vi "TLB main task ver 1.00 (incomplete).vi"() -> ()   [LabVIEW 2018]
uses:
  TLB Type Definitions/Intruction Type Definitions.ctl
  TLB Type Definitions/State Type Definitions, for 0.26g versions and later 3.ctl
  <vilib>/Studica/Studica Toolkit/NavX/TypeDefs/Flags/Z900_navX_Flags_OpStatusTypeDef.ctl
  <vilib>/Studica/Studica Toolkit/NavX/TypeDefs/Flags/Z900_navX_Flags_CalibrationStatusTypeDef.ctl
  TLB Type Definitions/Vision cluster.ctl
  TLB Type Definitions/PING CLUSTER.ctl
  TLB Type Definitions/Encoder cluster.ctl
  TLB Type Definitions/Stepper cluster.ctl
  TLB Type Definitions/Yaw Cluster.ctl
  TLB Type Definitions/IR Sensor Type Def.ctl
  TLB Type Definitions/Line Sensor Cluster.ctl
  TLB Type Definitions/Time cluster.ctl
  TLB Type Definitions/Box Colour Detection Cluster (0.26d and above).ctl
  Underlying VI's/FGV's/Box FGV/Box Colour FGV Colours.ctl
  <vilib>/Studica/Studica Toolkit/Background/DIO Channel.ctl
  TLB Type Definitions/Y Stepper cluster.ctl
  TLB Type Definitions/Motor Speed Cluster.ctl
  Labview Training Phase 2/Enum Controls/States for Action Engine.ctl
  Underlying VI's/NavX VI/navX type def.ctl
  <vilib>/Studica/Studica Toolkit/Background/I2C Channel.ctl
  Underlying VI's/I2C Master VI/Arduino_Interfacing.ctl
  Underlying VI's/Motor Control VI with PID/MOTOR CONTROL WITH PID AE DATA MODE TYPE DEF.ctl
  Underlying VI's/Motor Control VI with PID/MOTOR CONTROL WITH PID AE DIRECTION TYPE DEF.ctl
  Experimental VI's/Archived VI's/MOTOR CONTROL NO PID Type Def.ctl
  <vilib>/myRIO/Common/Instrument Driver Framework/myRIO v1.0/AI/typedefs/AI Channels List.ctl
  <vilib>/myRIO/Common/Instrument Driver Framework/myRIO v1.0/AI/typedefs/AI Channels Enum.ctl
  Underlying VI's/Line Sensor AE/Line Sensor AE Type Def.ctl
  Underlying VI's/I2C Master VI/I2C MASTER Type Def.ctl
  Underlying VI's/Elasped Timer/Elapsed timer control.ctl
  Underlying VI's/IMAQ Create Reference AE/IMAQ Reference AE.ctl
  Underlying VI's/FGV's/Box FGV/Box Colour FGV States.ctl
  Underlying VI's/I2C Master VI/I2C_MASTER_WRITE_NEW Type Def.ctl
  Underlying VI's/Modified webcam FGV/Webcam AE.ctl
  <vilib>/userdefined/High Color/IMAQdx.ctl
  <vilib>/Studica/Studica Toolkit/NavX/NavX.lvlib
  <vilib>/NI_Real-Time Target Support.lvlib
panel:
  out "Distance to move":dbl
  out "Same colour?":bool
  out "Box Colour Detection":T1
  out "Errors detected":bool
  out "Robot ready":bool
  out "Time cluster":T3
  out "Table IR obstruct":bool
  out "Front IR obstruct":bool
  out "CPU 1 Usage":dbl
  out "CPU 0 Usage":dbl
  out "Line sensors":T4
  out "IR Sensors":T5
  out "NAVX Values":T6
  out "Stepper position values":T7
  out "Encoder values":T8
  out "Ultrasonic sensors":T9
  out "Selected Task":T10=enum."Start Task 9"
  out "Object recognition mode":enum16{"Ball", "Soap", "Gel", "Pipe", "None"}(ring)
  out "Image Processing Error":errorcluster
  out "Object Detection":T11
  out "Status":T14 {"OP Status" items=["INITIALIZING", "SELFTEST_IN_PROGRESS", "ERROR", "IMU_AUTOCAL_IN_PROGRESS", "NORMAL"]; "Calibration Status" items=["IMU_CAL_STATE_MASK"=3, "IMU_CAL_STATE_INPROGRESS"=0, "IMU_CAL_STATE_ACCUMULATE"=1, "IMU_CAL_STATE_COMPLETE"=2]}
  out "General Errors":errorcluster
  in  "Red LED":bool
  out "Front Ultrasonic obstruct":bool
  out "Speed & distance":T15
  out "Task selection":u8
  out "NavX Readings":T16
  out "Arduino Data":T17
  out "TASK ENABLE":bool
  out "Rising Edge":bool
  in  "Green LED":bool
  out "State Logic":T18=enum."Startup"
  out "elements":T10[](array[typedef])
  in  "STOP TASK":bool
  in  "OK Button":bool
  in  "STOP":bool
  out "Queue Errors":errorcluster
  out "Action Queue Items":i32
  out "State Logic Queue Items":i32
  out "Action Queues items":string[](array[string])=["Hardware reset", "Software reset", ""]
  out "Action State":string
  # "VISION"
  # "TLB FRAMEWORK STATUS"
  # "System Health Status Update"
  # "Test Programme written by Calvin Loke    Dated: 28 Aug 2019\nTest Programme revised by Dr Alex See   Dated 30 Aug 2019\n\nRevision date: 20/03/2020\nProgramme version:   TLB Native Dynamic Events ver 0.19a"
  # "0: Task 1\n1: Task 2\n2: Task 3\n3: Task 4\n4: Task 5\n5: Task 6\n6: Task 7\n7: Task 8 Ball\n8: Task 8 Soap\n9: Task 8 Gel\n10: Task 8 Pipe\n11: Task 9 Blue\n12: Task 9 Black\n13: Task 9 Green\n14: Task 9 Red\n15: Task 9 Yellow"
  # "Ball: Right\nSoap: Left\nGel: Reverse\nPipe: Forward"
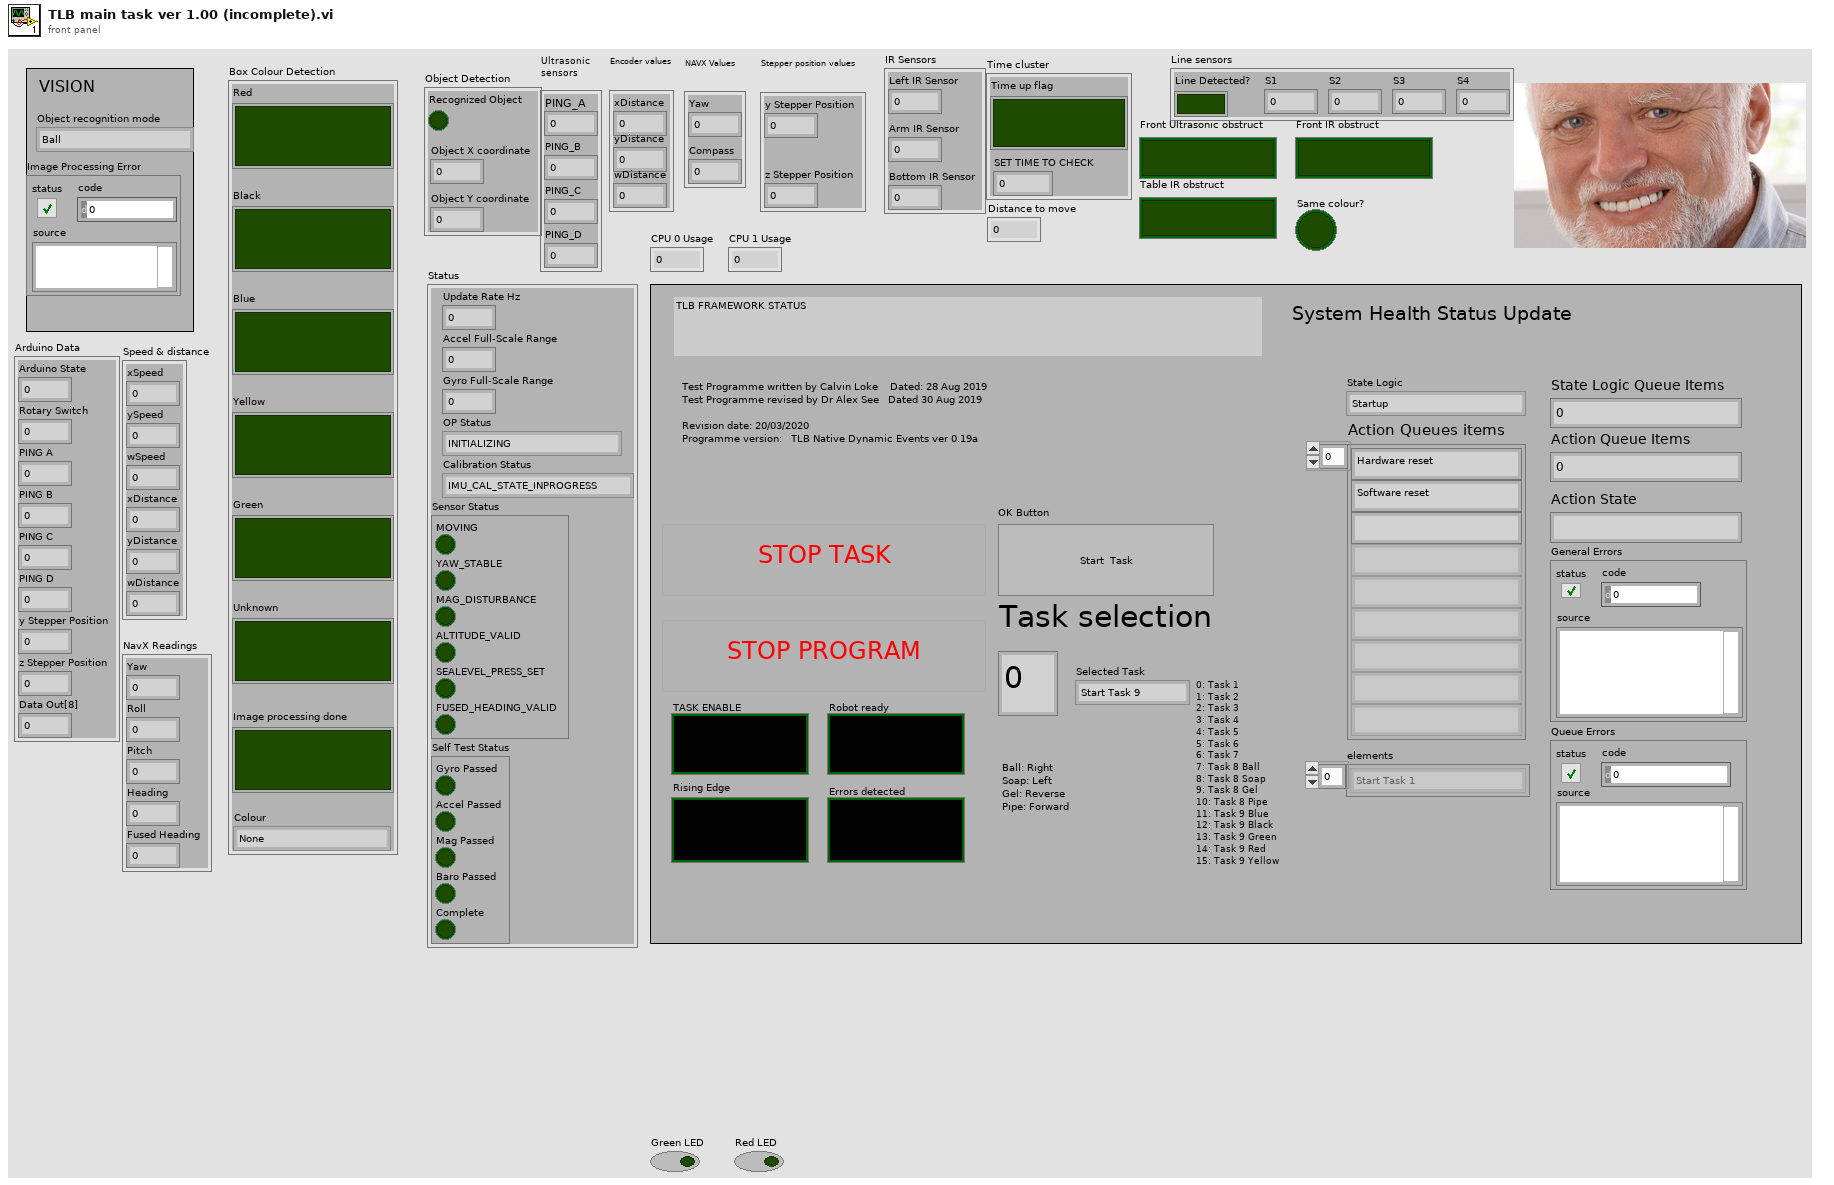
[diagram p1: front panel]
types:
  T1 = typedef "Box Colour Detection Cluster (0.26d and above).ctl" = cluster{"Red":bool, "Black":bool, "Blue":bool, "Yellow":bool, "Green":bool, "Unknown":bool, "Image processing done":bool, "Colour":T2}
  T2 = typedef "Box Colour FGV Colours.ctl" = enum16{"None", "Black", "Blue", "Green", "Red", "Yellow"}
  T3 = typedef "Time cluster.ctl" = cluster{"Time up flag":bool, "SET TIME TO CHECK":dbl}
  T4 = typedef "Line Sensor Cluster.ctl" = cluster{"Line Detected?":bool, "S1":dbl, "S2":dbl, "S3":dbl, "S4":dbl}
  T5 = typedef "IR Sensor Type Def.ctl" = cluster{"Left IR Sensor":dbl, "Arm IR Sensor":dbl, "Bottom IR Sensor":dbl}
  T6 = typedef "Yaw Cluster.ctl" = cluster{"Yaw":dbl, "Compass":dbl}
  T7 = typedef "Stepper cluster.ctl" = cluster{"y Stepper Position":u8, "z Stepper Position":u8}
  T8 = typedef "Encoder cluster.ctl" = cluster{"xDistance":dbl, "yDistance":dbl, "wDistance":dbl}
  T9 = typedef "PING CLUSTER.ctl" = cluster{"PING_A":u8, "PING_B":u8, "PING_C":u8, "PING_D":u8}
  T10 = typedef "Intruction Type Definitions.ctl" = enum16{"None", "Start Task 1", "Start Task 2", "Start Task 3", "Start Task 4", "Start Task 5", "Start Task 6", "Start Task 7", "Start Task 8 - BALL", "Start Task 8 - Gel", "Start Task 8 - Pipe", "Start Task 8 - Soap", "Start Task 9", "Start Task A", "Start Task B", "Exit"}
  T11 = typedef "Vision cluster.ctl" = cluster{"Recognized Object":bool, "Object X coordinate":dbl, "Object Y coordinate":dbl}
  T12 = typedef "NavX.lvlib/Z900_navX_Flags_OpStatusTypeDef.ctl" = u8
  T13 = typedef "NavX.lvlib/Z900_navX_Flags_CalibrationStatusTypeDef.ctl" = u8
  T14 = cluster{"Update Rate Hz":u8, "Accel Full-Scale Range":u8, "Gyro Full-Scale Range":u16, "OP Status":T12, "Calibration Status":T13, "Sensor Status":cluster{"MOVING":bool, "YAW_STABLE":bool, "MAG_DISTURBANCE":bool, "ALTITUDE_VALID":bool, "SEALEVEL_PRESS_SET":bool, "FUSED_HEADING_VALID":bool}, "Self Test Status":cluster{"Gyro Passed":bool, "Accel Passed":bool, "Mag Passed":bool, "Baro Passed":bool, "Complete":bool}}
  T15 = cluster{"xSpeed":dbl, "ySpeed":dbl, "wSpeed":dbl, "xDistance":dbl, "yDistance":dbl, "wDistance":dbl}
  T16 = cluster{"Yaw":dbl, "Roll":dbl, "Pitch":dbl, "Heading":dbl, "Fused Heading":dbl}
  T17 = cluster{"Arduino State":u8, "Rotary Switch":u8, "PING A":u8, "PING B":u8, "PING C":u8, "PING D":u8, "y Stepper Position":u8, "z Stepper Position":u8, "Data Out[8]":u8}
  T18 = typedef "State Type Definitions, for 0.26g versions and later 3.ctl" = enum16{"None", "Startup", "Move to Angle", "True Stop", "Idle", "Shutdown", "Task 1A", "Task 1B", "Task 2:Raise Arm", "Task 2:Sensor Mode", "Task 2:Reverse Mode", "Task 3", "Task 4_A", "Task 4_B", "Task 4_C", "Task 4_D", "Task 5A: RAISING ARM", "Task 5B: STILL WAITING", "Task 5C: GOING DOWN", "Task 5D: GRAB", "Task 5E: GOING UP", "Task 5F: ARM GRAB HEIGHT", "Task 5G: CLOSE CLAW", "Task 5H: RAISE ARM", "Task 6A: RAISE ARM", "Task 6B: CAM BURST", "Task 6C: PROCESS IMAGE", "Task 6D: BALL BUSTER", "Task 6E: STILL WAITING", "Task 6F: CAM BURST 2", "Task 6G: PROCESS IMAGE 2", "Task 6H: SKADI SOAPS", "Task 6I: STILL WAITING 2", "Task 6J: CAM BURST 3", "Task 6K: PROCESS IMAGE 3", "Task 6L: JAM IT IN", "Task 6M: STILL WAITING 3", "Task 6N: CAM BURST 4", "Task 6O: PROCESS IMAGE 4", "Task 6P: PIPE BOMB", "Task 7", "Task 8A: RAISE ARM", "Task 8B: MOVE TO BOX", "Task 8C: CAM BURST", "Task 8D: PROCESS IMAGE", "Task 8E: ROBOT ADJUST", "Task 8F: CAM BURST 2", "Task 8G: PROCESS IMAGE 2", "Task 8H: ARM ADJUST", "Task 8I: ARM GRAB HEIGHT", "Task 8J: CLOSE CLAW", "Task 8K: RAISE MY SWORD", "Task 9A: Raise Arm", "Task 9B: Rotate to Angle", "Task 9C: Detect Box", "Task 9D: MOVE FORWARD", "Task 9E: MOVE LEFT", "Task 9E2: MOVE RIGHT", "Task 9F: SCAN BOX", "Task 9G: MOVE RIGHT", "Task 9H: SCAN BOX 2", "Task 9I: ROTATE 90 CW", "Task 9J: FORWARD", "Task 9K: RAM WALL", "Task 9L: MOVE RIGHT", "Task 9M: SCAN BOX 3", "Task 9N: MOVE RIGHT", "Task 9O: SCAN BOX 4", "Task A1: RAISE ARM", "Task A2: ROTATE TO ANGLE", "Task A3: MOVE TO BL BOX", "Task A4: MOVE FORWARD", "Task A5: ROTATE CW 90"}
  T19 = typedef "Motor Speed Cluster.ctl" = cluster{"ySpeed":dbl, "xSpeed":dbl, "wSpeed":dbl}
  T20 = typedef "Y Stepper cluster.ctl" = cluster{"yStepper desired":u8}
  T21 = typedef "DIO Channel.ctl" = enum16{"Not Connected", "A/DIO1", "A/DIO2", "A/DIO3", "A/DIO4", "A/DIO5", "A/DIO6", "A/DIO7", "A/DIO13", "B/DIO1", "B/DIO2", "B/DIO3", "B/DIO4", "B/DIO5", "B/DIO6", "B/DIO7", "B/DIO13", "C/DIO0", "C/DIO1", "C/DIO2", "C/DIO3", "C/DIO4", "C/DIO5", "C/DIO6", "C/DIO7"}
  T22 = cluster{"DIO Channel":T21, "FPGA VI Reference Out":refnum<k20>}
  T23 = typedef "States for Action Engine.ctl" = enum16{"Initialize", "Write", "Read"}
  T24 = typedef "NI_Real-Time Target Support.lvlib/RT CPU Load.ctl" = cluster{"Total (%)":dbl, "Time Critical (%)":dbl, "Timed Structures (%)":dbl, "High (%)":dbl, "Above Normal (%)":dbl, "Normal (%)":dbl, "Background (%)":dbl, "Idle (%)":dbl, "ISR (%)":dbl}
  T25 = cluster{"CPU loads[0]":T24, "CPU loads[1]":T24, "CPU loads[2]":T24, "CPU loads[3]":T24, "CPU loads[4]":T24, "CPU loads[5]":T24, "CPU loads[6]":T24, "CPU loads[7]":T24, "CPU loads[8]":T24}
  T26 = typedef "navX type def.ctl" = enum16{"Get i2C reference", "Read Values", "Zero Yaw"}
  T27 = typedef "Arduino_Interfacing.ctl" = enum16{"Initialize", "Write to Arduino", "Read From Arduino"}
  T28 = typedef "I2C Channel.ctl" = enum16{"Not Connected", "A", "B"}
  T29 = cluster{"I2C Ref Out":cluster{"I2C Channel":T28, "FPGA VI Reference Out":refnum<k20>}, "Connected":bool, "Slave Address (7-bit)":u8, "Registry":u8[]}
  T30 = typedef "Box Colour FGV States.ctl" = enum16{"Initialize", "Read", "Write"}
  T31 = typedef "MOTOR CONTROL WITH PID AE DIRECTION TYPE DEF.ctl" = enum16{"y-axis movement", "x-axis movement", "rotation", "stop", "reset encoders"}
  T32 = typedef "MOTOR CONTROL WITH PID AE DATA MODE TYPE DEF.ctl" = enum16{"Init AE", "Write to AE", "Read from AE"}
  T33 = typedef "Line Sensor AE Type Def.ctl" = enum16{"INIT AE", "READ FROM LINE SENSORS"}
  T34 = typedef "IMAQ Reference AE.ctl" = enum16{"Initialize AE", "Get IMAQ Reference", "Dispose Processing Buffer"}
  T35 = typedef "Elapsed timer control.ctl" = enum16{"Start", "Pause", "Initialize"}
  T36 = typedef "I2C_MASTER_WRITE_NEW Type Def.ctl" = enum16{"Ultrasonic sensors", "Stepper origin", "zStepper 13.3k", "zStepper 13k", "zStepper 12k", "zStepper 11k", "zStepper 10k", "zStepper 9k", "zStepper 8k", "zStepper 7k", "zStepper 6k", "zStepper 5k", "zStepper 4k", "zStepper 3k", "zStepper 2k", "zStepper 1k", "zStepper 900", "zStepper 800", "zStepper 700", "zStepper 600", "zStepper 500", "zStepper 400", "zStepper 300", "zStepper 200", "zStepper 100", "zStepper 0", "yStepper control", "Open Claw", "Close Claw", "Soft Reset"}
  T37 = typedef "Webcam AE.ctl" = enum16{"Initialize Camera", "Open Camera", "Continuous Acquisition", "Close Camera", "Retrieve Image", "Dispose Camera Image Buffer"}
  T38 = typedef "IMAQdx.ctl" = refnum<k21>
  T39 = typedef "MOTOR CONTROL NO PID Type Def.ctl" = enum16{"Init", "Front Back", "Left Right", "Rotate", "Stop", "Latch"}
  T40 = typedef "AI Channels List.ctl" = T41[]
  T41 = typedef "AI Channels Enum.ctl" = enum16{"Not Connected", "AudioIn/Left", "AudioIn/Right", "C/AI0", "C/AI1", "A/AI0", "A/AI1", "A/AI2", "A/AI3", "A/AI4", "A/AI5", "A/AI6", "A/AI7", "B/AI0", "B/AI1", "B/AI2", "B/AI3", "B/AI4", "B/AI5", "B/AI6", "B/AI7", "AI/AI0", "AI/AI1", "AI/AI2", "AI/AI3", "A/AI0 (DIFF)", "A/AI1 (DIFF)", "A/AI2 (DIFF)", "A/AI3 (DIFF)", "B/AI0 (DIFF)", "B/AI1 (DIFF)", "B/AI2 (DIFF)", "B/AI3 (DIFF)"}
  T42 = cluster{"S1":dbl, "S2":dbl, "S3":dbl, "S4":dbl, "Array[4]":dbl, "Array[5]":dbl, "Array[6]":dbl, "Array[7]":dbl, "Array[8]":dbl}
  T43 = typedef "I2C MASTER Type Def.ctl" = enum16{"Last State", "Mode 0", "Mode 1", "Mode 2", "Mode 3", "Mode 4", "Mode 5", "Mode 6", "Mode 7", "Mode 8", "Mode 9", "Mode 10"}
  T44 = typedef "IMAQ Image.ctl" = refnum<image>
  T45 = cluster{"Number of Matches":i32, "Object detected?":bool}
  T46 = cluster{"Red":bool, "Black":bool, "Blue":bool, "Yellow":bool, "Green":bool, "No recognizable coolour":bool}
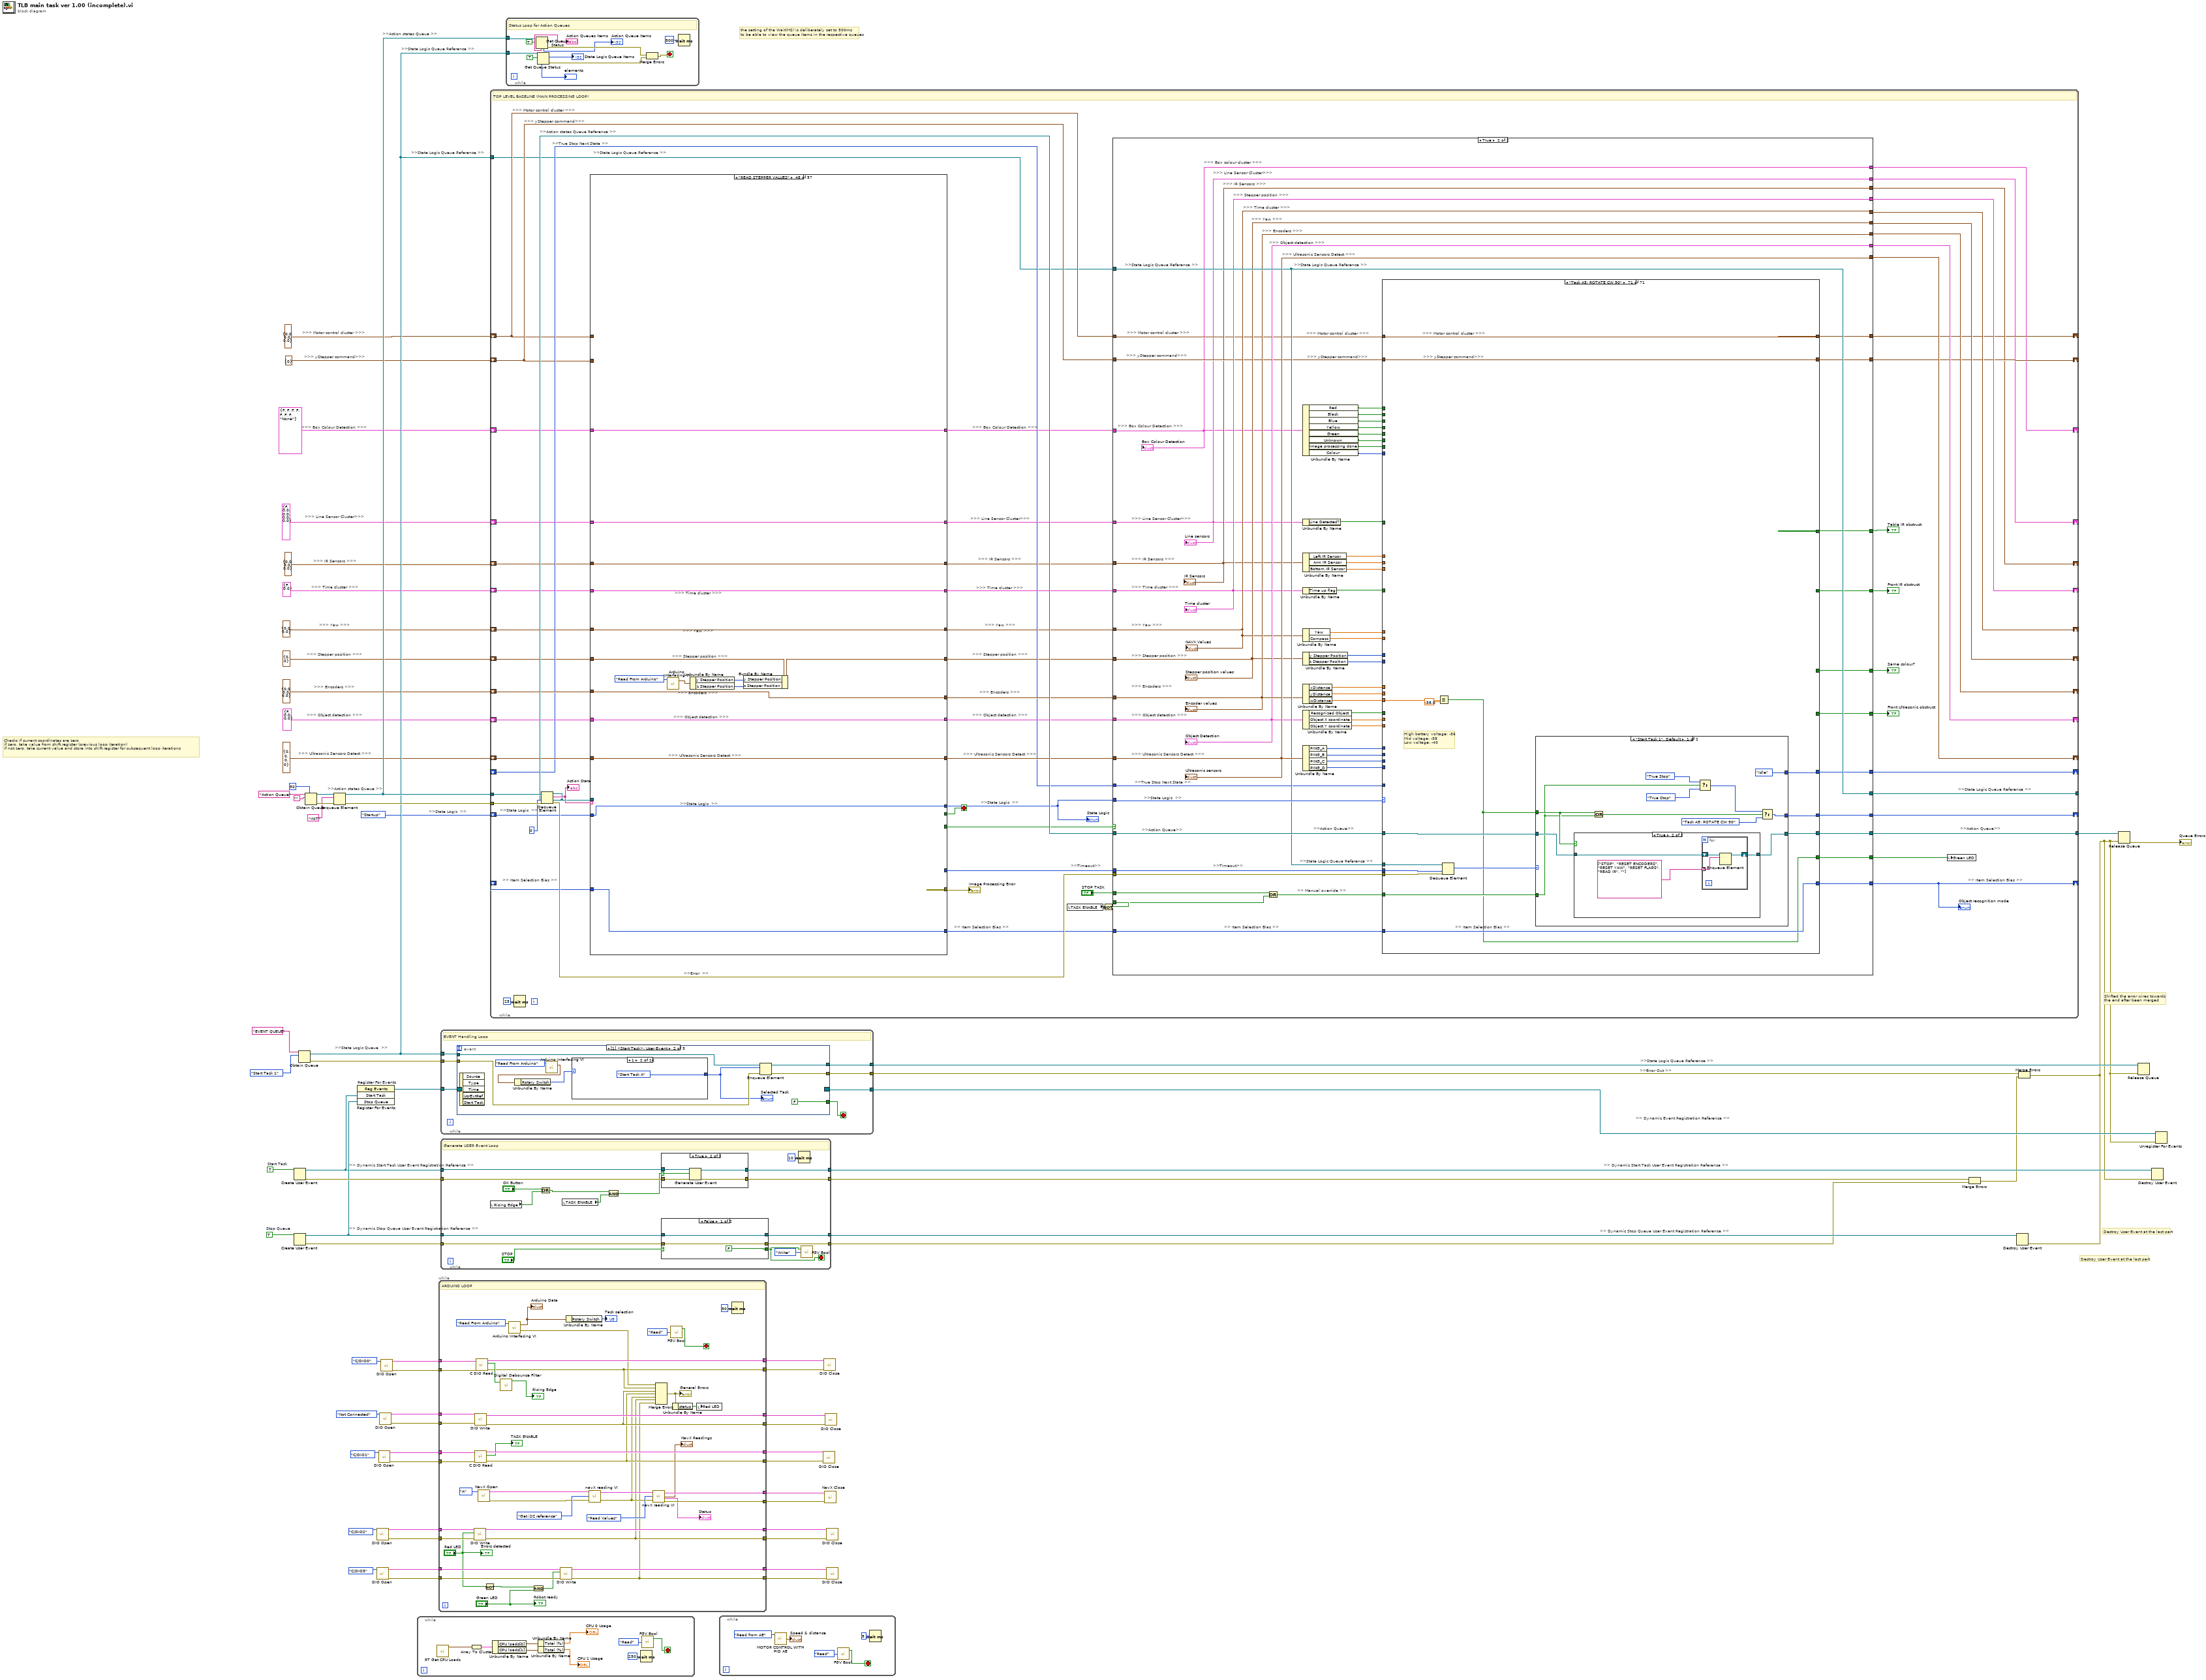
[diagram p0: block diagram]
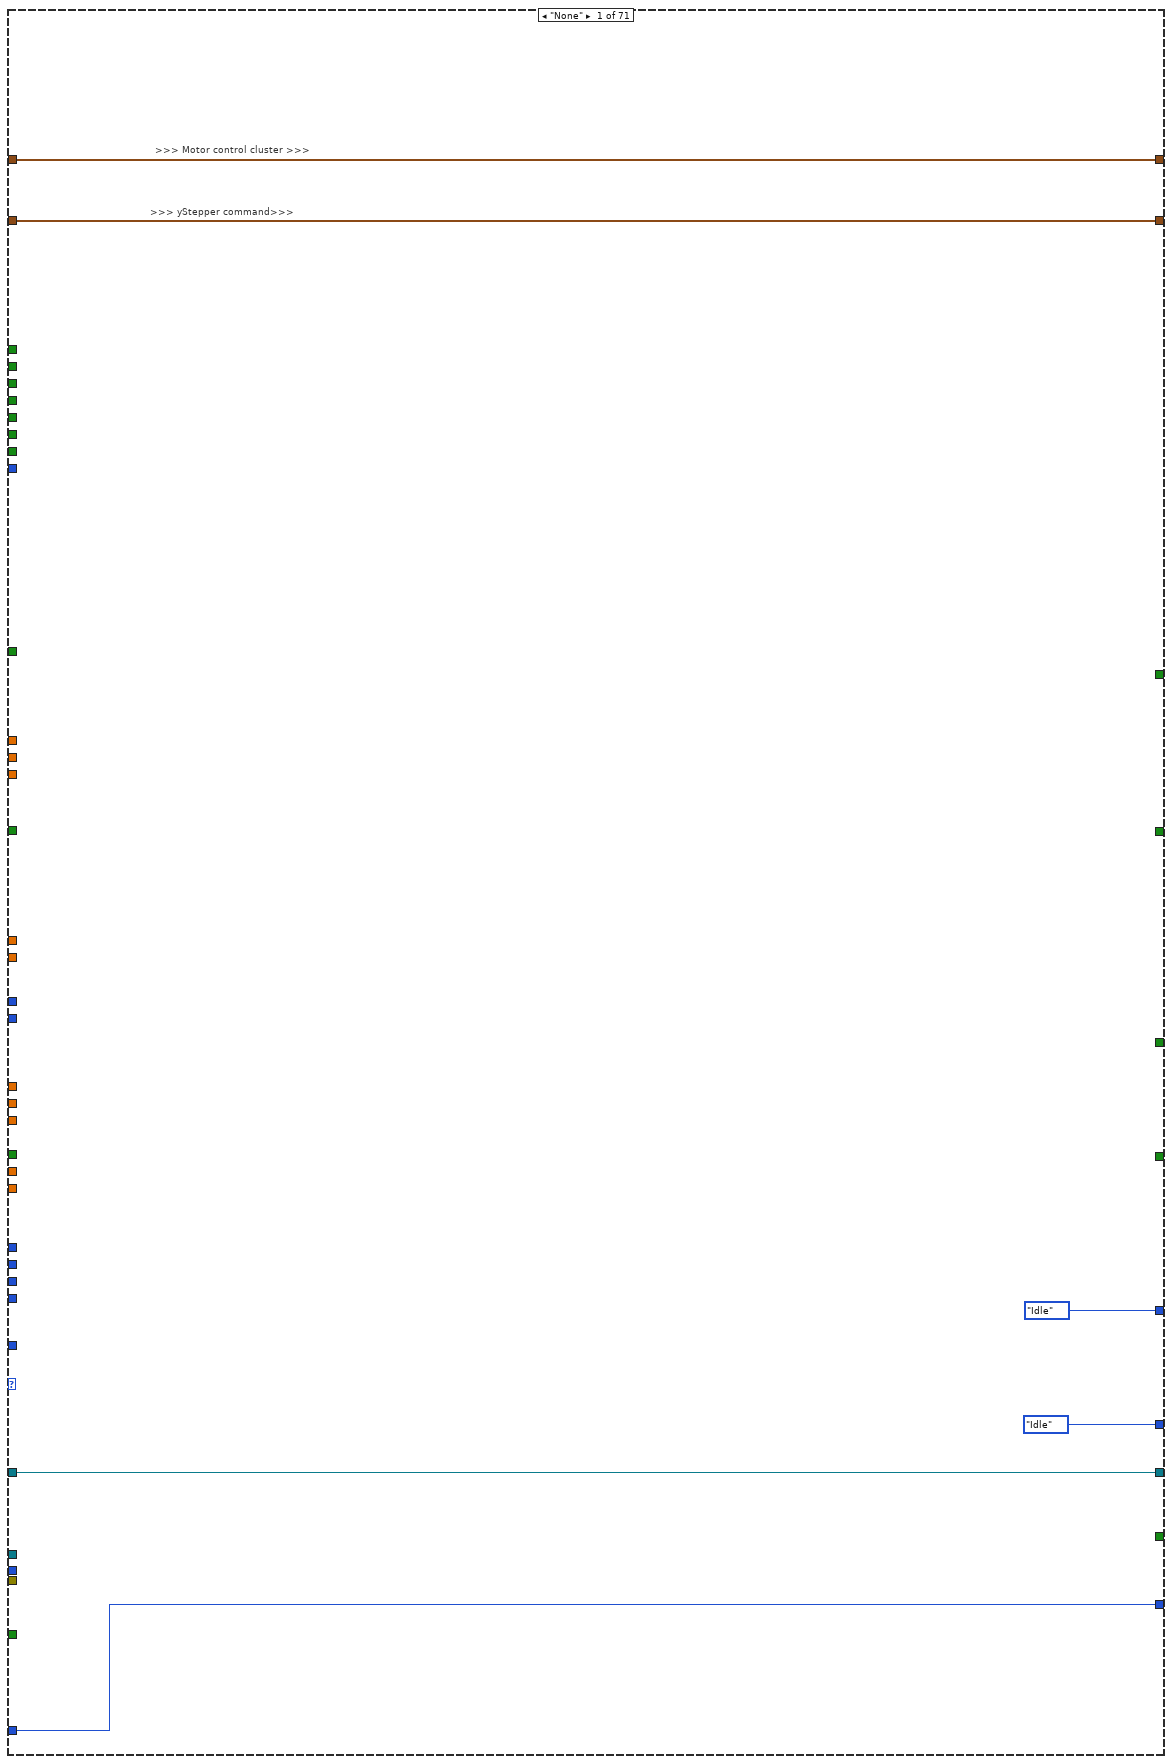
[diagram p3: hidden frame]
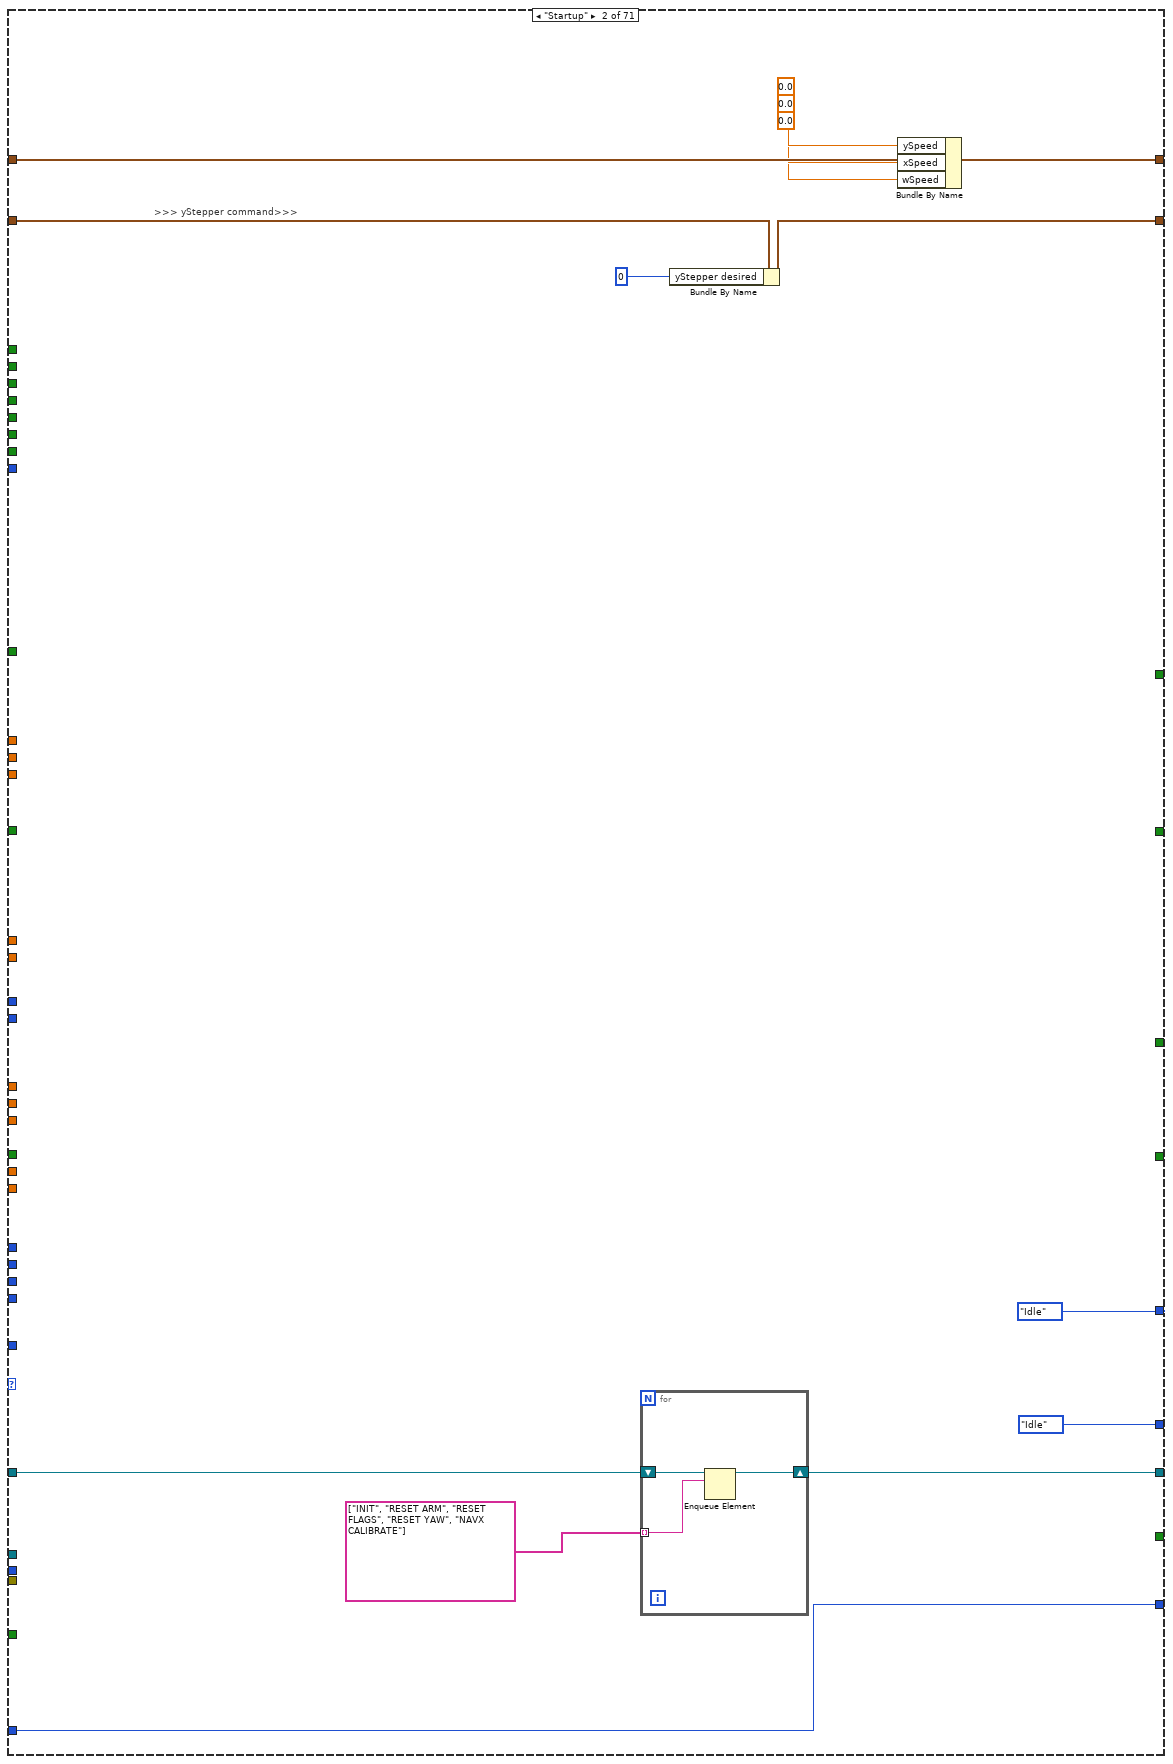
[diagram p4: hidden frame]
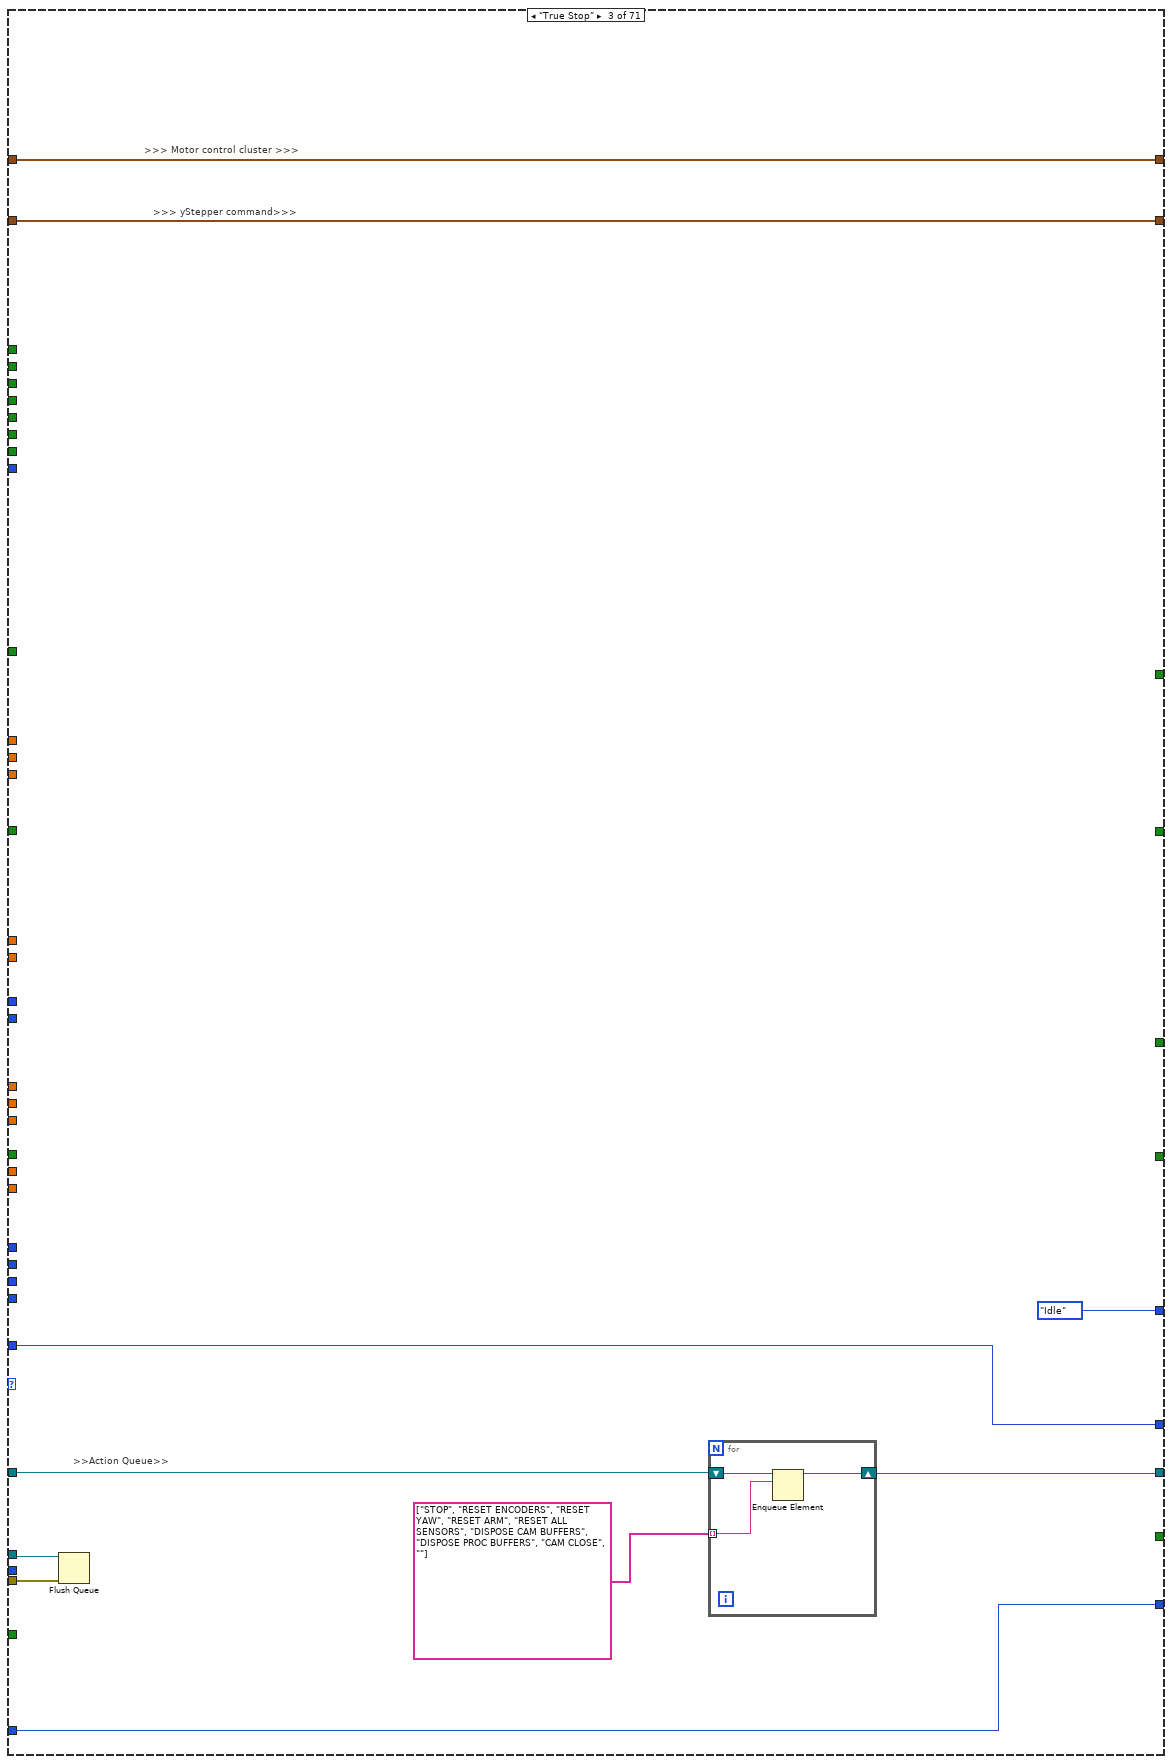
[diagram p5: hidden frame]
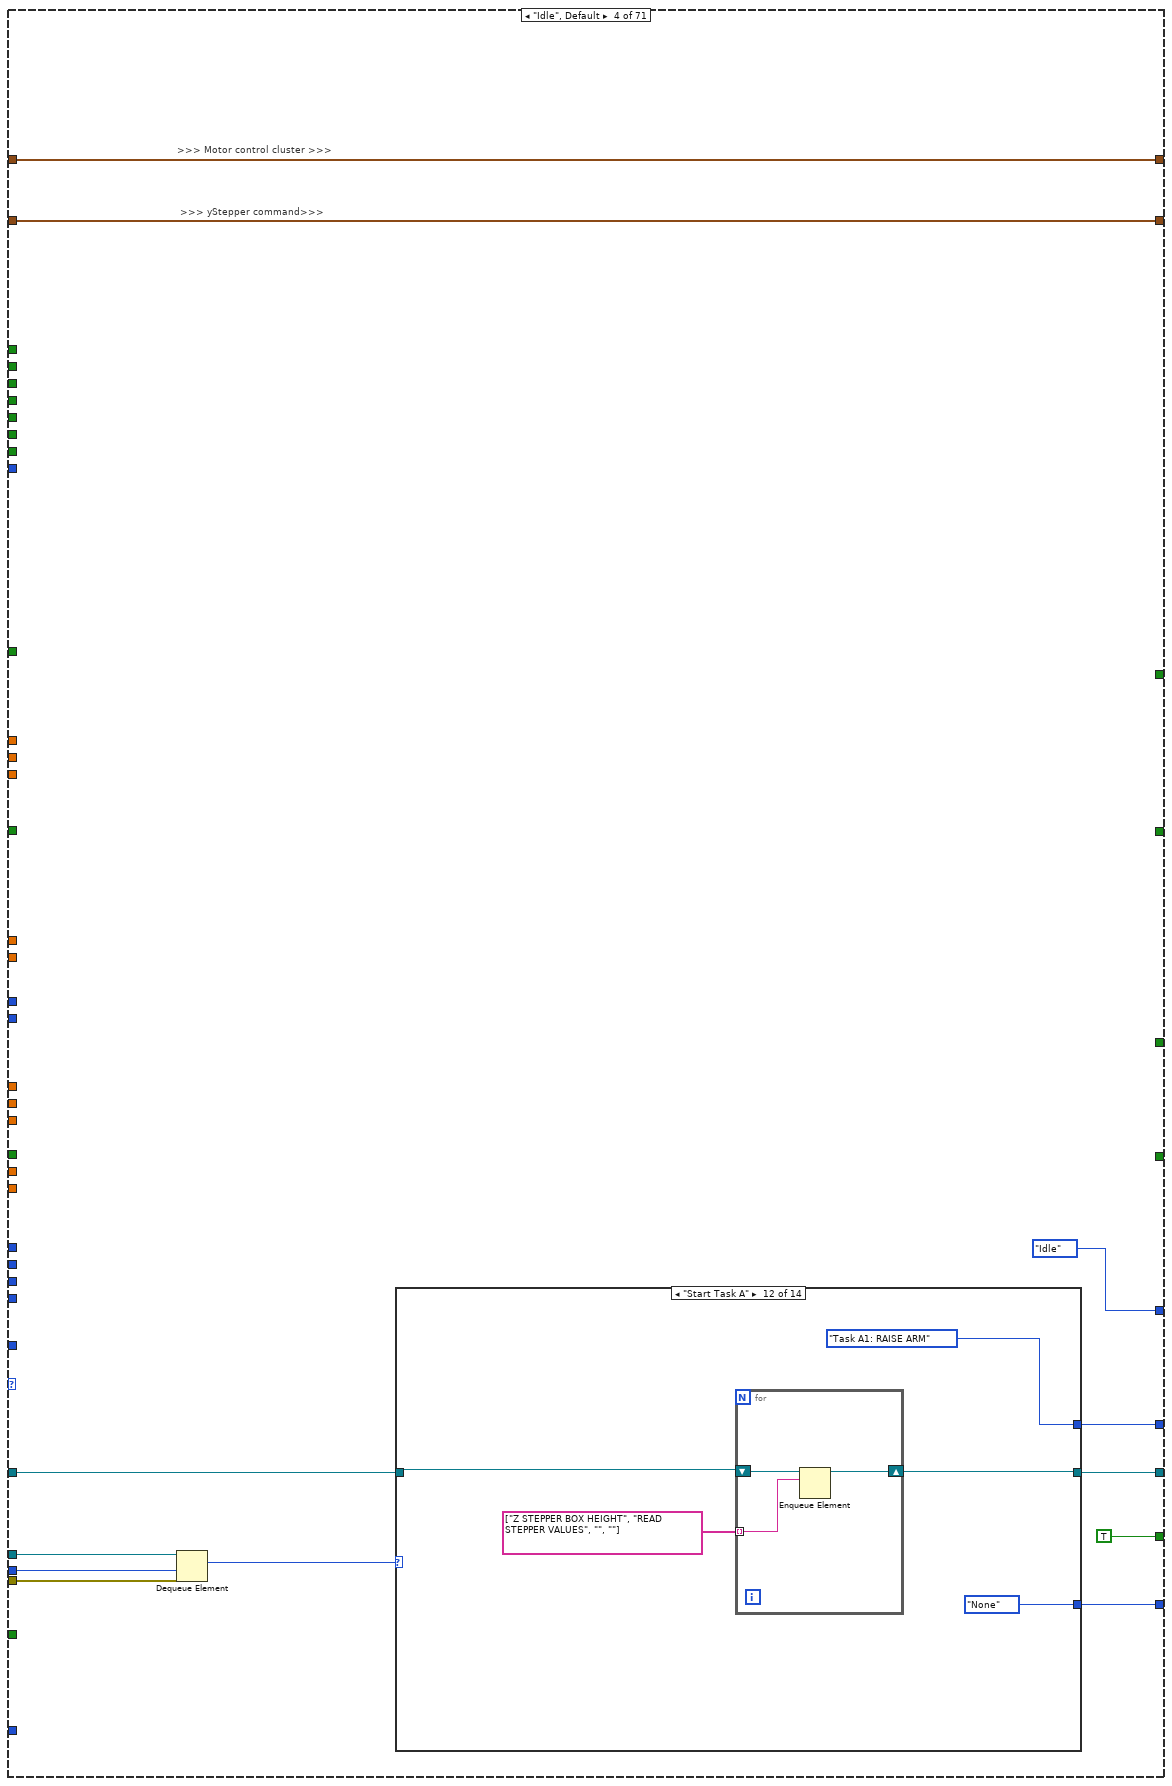
[diagram p6: hidden frame]
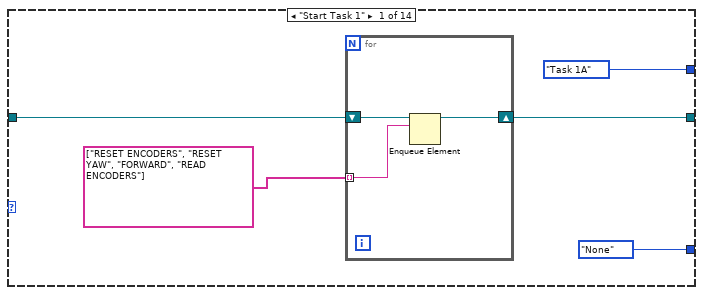
[diagram p7: hidden frame]
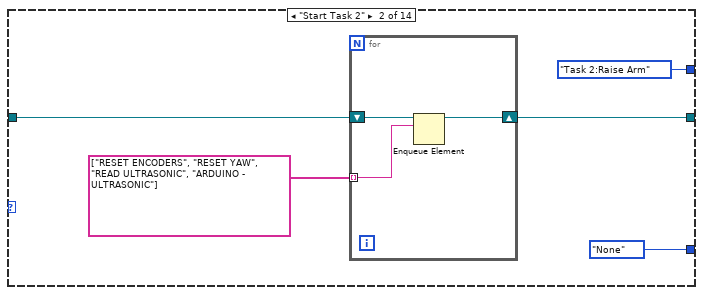
[diagram p8: hidden frame]
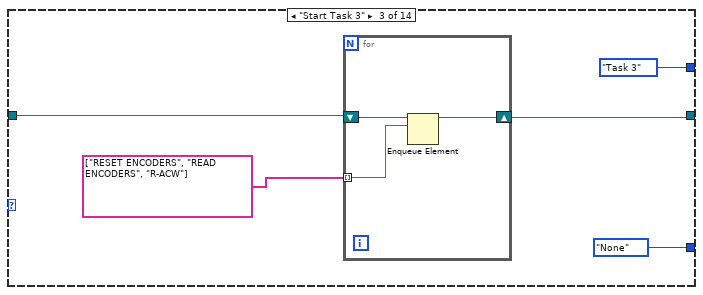
[diagram p9: hidden frame]
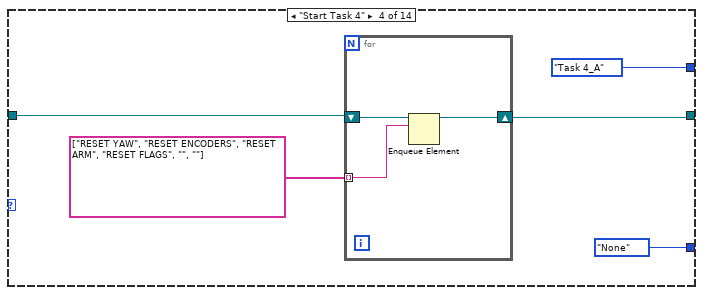
[diagram p10: hidden frame]
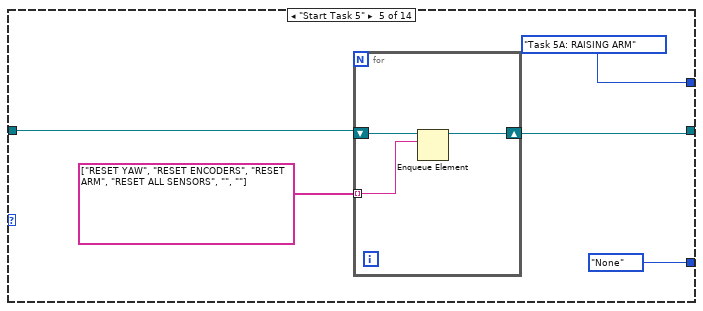
[diagram p11: hidden frame]
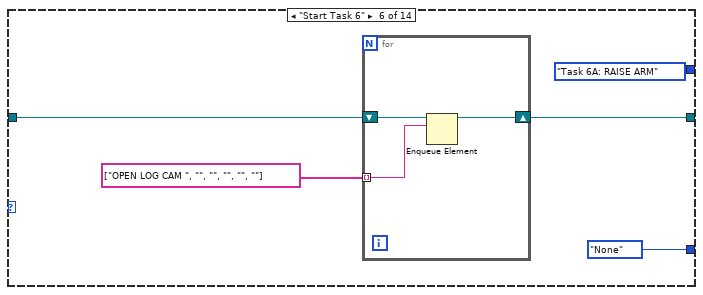
[diagram p12: hidden frame]
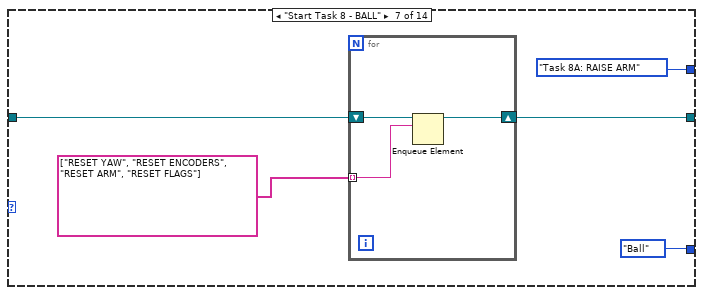
[diagram p13: hidden frame]
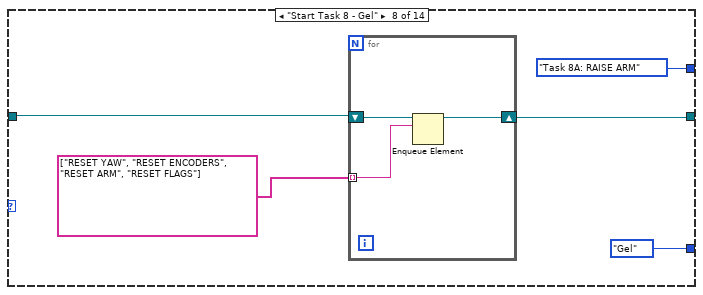
[diagram p14: hidden frame]
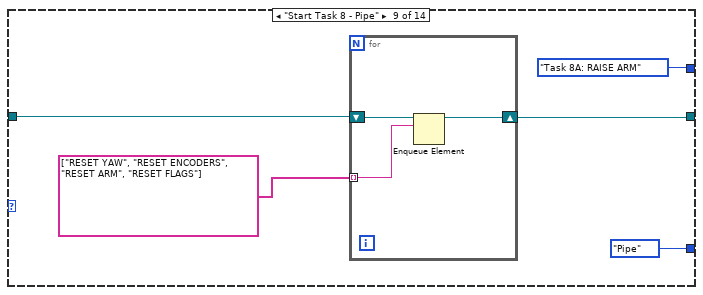
[diagram p15: hidden frame]
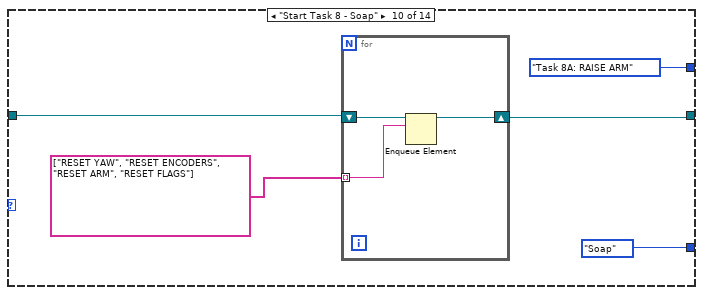
[diagram p16: hidden frame]
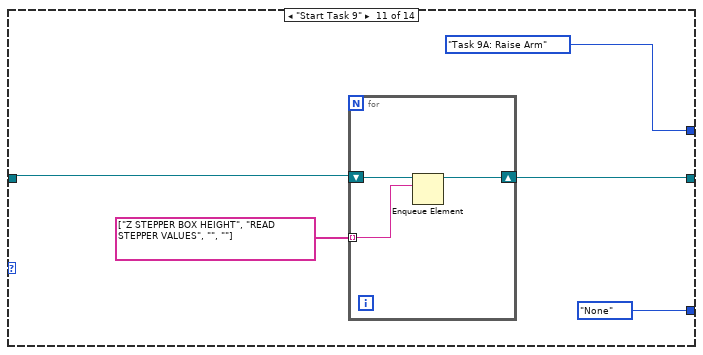
[diagram p17: hidden frame]
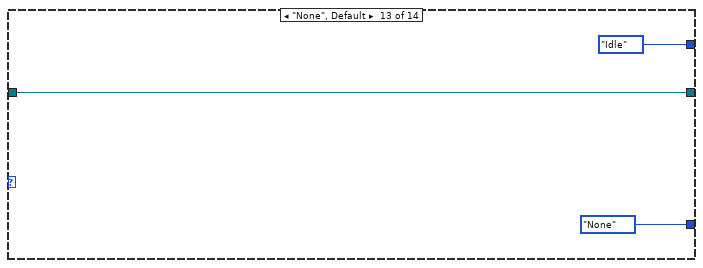
[diagram p18: hidden frame]
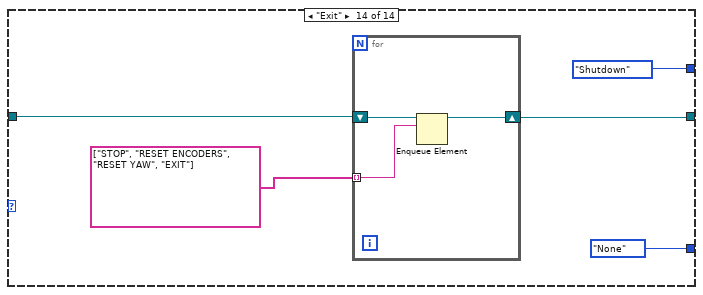
[diagram p19: hidden frame]
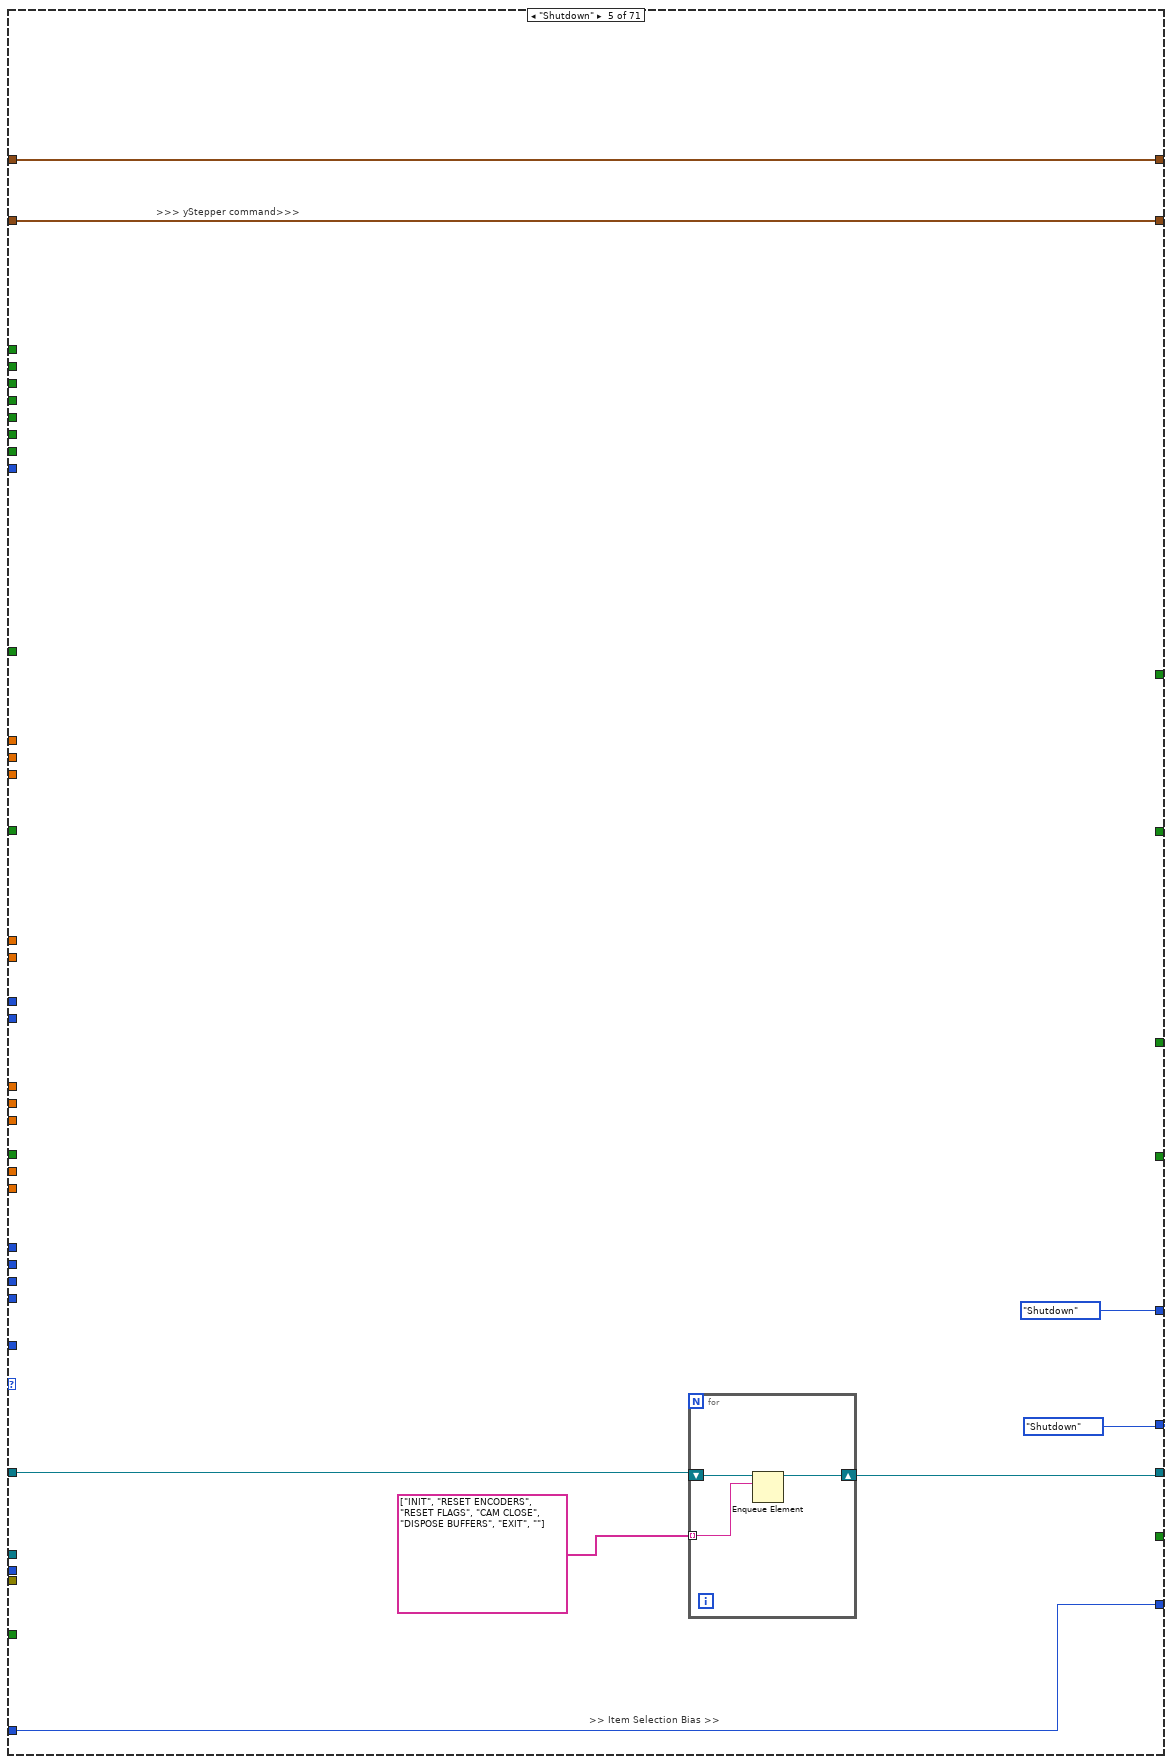
[diagram p20: hidden frame]
diagram:
  w69 = TRUE  # Stop Queue
  w68 = TRUE  # Start Task
  # ">>State Logic Queue Reference >>"
  # ">>Action states Queue >>"
  # ">>> Box Colour Detection >>>"
  # ">>State Logic Queue Reference >>"
  # ">>State Logic  >>"
  # ">>> Line Sensor Cluster>>>"
  # ">>> Motor control cluster >>>"
  # ">>> IR Sensors >>>"
  # "Checks if current coordinates are zero\nif zero, take value from shift register (previous loop iteration)\nif not zero, take current value and store into shift register for subsequent loop iterations"
  # ">>> yStepper command>>>"
  # ">>> Time cluster >>>"
  # ">>> Yaw >>>"
  # ">>> Stepper position >>>"
  # ">>> Encoders >>>"
  # ">>> Object detection >>>"
  # ">>> Ultrasonic Sensors Detect >>>"
  # "the setting of the Wait(MS) is deliberately set to 500ms\nto be able to view the queue items in the respective queues"
  # ">>Error Out >>"
  # ">> Dynamic Stop Queue User Event Registration Reference >>"
  # ">> Dynamic Start Task User Event Registration Reference >>"
  # ">> Dynamic Stop Queue User Event Registration Reference >>"
  # ">> Dynamic Start Task User Event Registration Reference >>"
  # ">> Dynamic Event Registration Reference >>"
  # ">>Action states Queue >>"
  # ">>State Logic Queue  >>"
  # ">>State Logic Queue Reference >>"
  # "Destroy User Event at the last part"
  # "Destroy User Event at the last part"
  # "Shifted the error wires towards\nthe end after been merged"
  n1 = Create User Event(user event datatype=w68) -> (user event=w60:refnum<user-event>, error out=w65:errorcluster)  [unwired: 1 in]
  n2 = Create User Event(user event datatype=w69) -> (user event=w61:refnum<user-event>, error out=w64:errorcluster)  [unwired: 1 in]
  n3 = Obtain Queue(name (unnamed)="EVENT QUEUE", element data type=Intruction_Type_Definitions."Start Task 1" ("Enum")) -> (queue out=w46:refnum<queue>, error out=w52:errorcluster)  [unwired: 3 in, 1 out]
  n4 = Obtain Queue(max queue size (-1, unlimited)=50, name (unnamed)="Action Queue", element data type="") -> (queue out=w55:refnum<queue>, error out=w51:errorcluster)  [unwired: 2 in, 1 out]
  n5 = Enqueue Element(queue=w55, element="INIT", error in (no error)=w51) -> (queue out=w47:refnum<queue>, error out=w50:errorcluster)  [unwired: 1 in, 1 out]
  n6 = register-events "Register For Events"(w60, w61) -> (reference out=w59:refnum<event-registration>)  [unwired: 2 in, 1 out]
  n7 = call <vilib>:"DIO Open.vi"("DIO Channel"=DIO_Channel."C/DIO2") -> ("error out"=w19:errorcluster, "DIO Info Out"=w20:T22)  [unwired: 9 in]
  n8 = call <vilib>:"DIO Open.vi"("DIO Channel"=DIO_Channel."C/DIO3") -> ("error out"=w14:errorcluster, "DIO Info Out"=w15:T22)  [unwired: 9 in]
  n9 = call <vilib>:"DIO Open.vi"("DIO Channel"=DIO_Channel."C/DIO1") -> ("error out"=w24:errorcluster, "DIO Info Out"=w25:T22)  [unwired: 9 in]
  n10 = call <vilib>:"DIO Open.vi"("DIO Channel"=DIO_Channel."Not Connected") -> ("error out"=w29:errorcluster, "DIO Info Out"=w31:T22)  [unwired: 9 in]
  n11 = call <vilib>:"DIO Open.vi"("DIO Channel"=DIO_Channel."C/DIO0") -> ("error out"=w34:errorcluster, "DIO Info Out"=w37:T22)  [unwired: 9 in]
  n12 = while {
    stop <- w76 stop-if-true
    n13 = call <vilib>:"RT Get CPU Loads.vi"() -> ("CPU loads"=w75:T24[])  [unwired: 10 in, 1 out]
    n14 = Array To Cluster(array=w75) -> (cluster=w74:T25)
    n15 = Unbundle By Name(w74) -> ("CPU loads[0]"=w73:T24, "CPU loads[1]"=w72:T24)
    n16 = Unbundle By Name(w73) -> ("Total (%)"=→"CPU 0 Usage":dbl)
    n17 = Unbundle By Name(w72) -> ("Total (%)"=→"CPU 1 Usage":dbl)
    n18 = Wait (ms)(milliseconds to wait=u32 250) -> ()  [unwired: 1 out]
    n19 = call "FGV Bool.vi"("Init/Read/Write State"=States_for_Action_Engine."Read") -> ("Output node"=w76:bool)  [unwired: 2 in, 1 out]
  }
  n20 = while {
    tunnel: w37 -> [w122]
    tunnel: [w121] -> w35
    tunnel: w34 -> [w120]
    tunnel: [w91] -> w33
    tunnel: w31 -> [w117]
    tunnel: [w116] -> w30
    tunnel: w29 -> [w115]
    tunnel: [w90] -> w28
    tunnel: [w114] -> w26
    tunnel: w25 -> [w113]
    tunnel: w24 -> [w112]
    tunnel: [w89] -> w23
    tunnel: w20 -> [w106]
    tunnel: w19 -> [w105]
    tunnel: [w104] -> w18
    tunnel: [w87] -> w17
    tunnel: w15 -> [w103]
    tunnel: w14 -> [w102]
    tunnel: [w101] -> w13
    tunnel: [w86] -> w12
    tunnel: [w98] -> w9
    tunnel: [w97] -> w10
    stop <- w124 stop-if-true
    # "ARDUINO LOOP"
    n21 = call <vilib>:"DIO Write.vi"("error in (no error)"=w105, "Input"="Red LED", "DIO Info In"=w106) -> ("error out"=w87:errorcluster, "DIO Info Out"=w104:T22)  [unwired: 7 in]
    n22 = call <vilib>:"DIO Write.vi"("error in (no error)"=w115, "DIO Info In"=w117) -> ("error out"=w90:errorcluster, "DIO Info Out"=w116:T22)  [unwired: 8 in]
    n23 = call <vilib>:"C DIO Read.vi"("error in (no error)"=w112, "DIO Info In in"=w113) -> ("error out"=w89:errorcluster, "IN"=→"TASK ENABLE":bool, "DIO Info In out"=w114:T22)  [unwired: 7 in]
    n24 = call <vilib>:"C DIO Read.vi"("error in (no error)"=w120, "DIO Info In in"=w122) -> ("error out"=w91:errorcluster, "IN"=w119:bool, "DIO Info In out"=w121:T22)  [unwired: 7 in]
    n25 = call <vilib>:"NavX Open.vi"("I2C Channel"=I2C_Channel."A") -> ("error out"=w108:errorcluster, "NavX Info"=w110:T29)  [unwired: 9 in]
    n26 = Not(x="Red LED") -> (.not. x?=w81:bool)
    n27 = call "Digital Debounce Filter.vi"("Boolean input"=w119) -> ("Rising Edge"=→"Rising Edge":bool)  [unwired: 1 in, 2 out]
    n28 = call "Arduino Interfacing VI.vi"("AE Mode"=Arduino_Interfacing."Read From Arduino") -> ("error out"=w92:errorcluster, "Arduino Data"=w94:T17)  [unwired: 3 in]
    "Arduino Data" <- w94
    n29 = And(x=w81, y="Green LED") -> (x .and. y?=w83:bool)
    n30 = call <vilib>:"DIO Write.vi"("error in (no error)"=w102, "Input"=w83, "DIO Info In"=w103) -> ("error out"=w86:errorcluster, "DIO Info Out"=w101:T22)  [unwired: 7 in]
    n31 = Unbundle By Name(w94) -> ("Rotary Switch"=→"Task selection":u8)
    n32 = call "navX reading VI.vi"("NavX Info In"=w110, "Mode"=navX_type_def."Get i2C reference", "error in (no error)"=w108) -> ("NavX Info Out"=w99:T29, "Error Out"=w88:errorcluster)  [unwired: 2 out]
    n33 = call "navX reading VI.vi"("NavX Info In"=w99, "Mode"=navX_type_def."Read Values", "error in (no error)"=w88) -> ("NavX Info Out"=w98:T29, "NavX Readings"=→"NavX Readings":T16, "Status"=→"Status":T14, "Error Out"=w97:errorcluster)
    n34 = Merge Errors(w92, w91, w90, w89, w88, w87, w86) -> (w84:errorcluster)
    "General Errors" <- w84
    n35 = call "FGV Bool.vi"("Init/Read/Write State"=States_for_Action_Engine."Read") -> ("Output node"=w124:bool)  [unwired: 2 in, 1 out]
    n36 = Unbundle By Name(w84) -> ("status"=w82:bool)
    n37 = local write "Red LED"(w82) -> ()
    n38 = Wait (ms)(milliseconds to wait=u32 50) -> ()  [unwired: 1 out]
    "Robot ready" <- "Green LED"
    "Errors detected" <- "Red LED"
  }
  n39 = while {
    tunnel: w60 -> [w142]
    tunnel: w61 -> [w141]
    tunnel: [w140] -> w67
    tunnel: [w139] -> w66
    tunnel: w65 -> [w138]
    tunnel: [w137] -> w63
    tunnel: w64 -> [w136]
    tunnel: [w135] -> w62
    stop <- w133 stop-if-true
    # "Generate USER Event Loop"
    n40 = local read "Rising Edge"() -> (w130:bool)
    n41 = Or(x="OK Button", y=w130) -> (x .or. y?=w129:bool)
    n42 = local read "TASK ENABLE"() -> (w128:bool)
    n43 = And(x=w129, y=w128) -> (x .and. y?=w127:bool)
    n44 = case shown="True" w127 {
      selector: w127 -> [_ w153]
      tunnel: w142 -> [w152 w157]
      tunnel: [w152 w156] -> w139
      tunnel: w138 -> [w151 w155]
      tunnel: [w151 w154] -> w137
      frame False {
      }
      frame True {
        n45 = Generate User Event(user event=w157, event data cluster=w153, error in=w155) -> (user event out=w156:refnum<user-event>, error out=w154:errorcluster)  [unwired: 1 in]
      }
    }
    n46 = case shown="False" "STOP" {
      selector: "STOP" -> [_ w146]
      tunnel: w141 -> [w145 w150]
      tunnel: [w145 w149] -> w140
      tunnel: w136 -> [w144 w148]
      tunnel: [w144 w147] -> w135
      tunnel: [FALSE w146] -> w133
      frame False {
      }
      frame True {
        n47 = Generate User Event(user event=w150, event data cluster=w146, error in=w148) -> (user event out=w149:refnum<user-event>, error out=w147:errorcluster)  [unwired: 1 in]
      }
    }
    n48 = Wait (ms)(milliseconds to wait=u32 10) -> ()  [unwired: 1 out]
    n49 = call "FGV Bool.vi"("Init/Read/Write State"=States_for_Action_Engine."Write", "Input Node"=w133) -> ()  [unwired: 1 in, 2 out]
  }
  n50 = while {
    tunnel: w59 -> [w164]
    tunnel: [w163] -> w58
    tunnel: w46 -> [w161]
    tunnel: [w160] -> w57
    tunnel: w52 -> [w159]
    tunnel: [w158] -> w49
    stop <- w162 stop-if-true
    # "EVENT Handling Loop"
    n51 = event shown="[1] <Start Task>: User Event" {
      selector: w164 -> [_ _ _]
      dyn-events: [_ _ _] -> w163
      timeout: _ -> [_ _ _]
      tunnel: [FALSE FALSE w211] -> w162
      tunnel: w161 -> [w169 w178 w209]
      tunnel: [w168 w177 w210] -> w160
      tunnel: w159 -> [w167 w176 w208]
      tunnel: [w166 w175 w207] -> w158
      event Timeout {
        n52 = event-data() -> ()  [unwired: 1 in, 3 out]
        n53 = Enqueue Element(queue=w169, element=Intruction_Type_Definitions."Start Task 1" ("Enum"), error in (no error)=w167) -> (queue out=w168:refnum<queue>, error out=w166:errorcluster)  [unwired: 1 in, 1 out]
      }
      event User Event {
        n54 = event-data() -> ()  [unwired: 1 in, 5 out]
        n55 = call "Arduino Interfacing VI.vi"("AE Mode"=Arduino_Interfacing."Read From Arduino") -> ("Arduino Data"=w172:T17)  [unwired: 3 in, 1 out]
        n56 = Unbundle By Name(w172) -> ("Rotary Switch"=w171:u8)
        n57 = case shown="1" w171 {
          tunnel: [Intruction_Type_Definitions."None" ("Enum") Intruction_Type_Definitions."Start Task A" ("Enum") Intruction_Type_Definitions."Start Task 3" ("Enum") Intruction_Type_Definitions."Start Task 4" ("Enum") Intruction_Type_Definitions."Start Task 5" ("Enum") Intruction_Type_Definitions."Start Task 6" ("Enum") Intruction_Type_Definitions."Start Task 7" ("Enum") Intruction_Type_Definitions."Start Task 8 - BALL" ("Enum") Intruction_Type_Definitions."Start Task 8 - Soap" ("Enum") Intruction_Type_Definitions."Start Task 8 - Gel" ("Enum") Intruction_Type_Definitions."Start Task 8 - Pipe" ("Enum") Intruction_Type_Definitions."Start Task 9" ("Enum") Intruction_Type_Definitions."Start Task 9" ("Enum") Intruction_Type_Definitions."Start Task 9" ("Enum") Intruction_Type_Definitions."Start Task 9" ("Enum") Intruction_Type_Definitions."Start Task 9" ("Enum")] -> w174
          frame 0, Default {
          }
          frame 1 {
          }
          frame 2 {
          }
          frame 3 {
          }
          frame 4 {
          }
          frame 5 {
          }
          frame 6 {
          }
          frame 7 {
          }
          frame 8 {
          }
          frame 9 {
          }
          frame 10 {
          }
          frame 11 {
            # "Task 9: Red Detection"
            n58 = call "Box Colour FGV.vi"("Colour to detect"=Box_Colour_FGV_Colours."Blue", "Init/R/W State"=Box_Colour_FGV_States."Write") -> ()  [unwired: 8 in, 2 out]
          }
          frame 12 {
            # "Task 9: Black Detection"
            n59 = call "Box Colour FGV.vi"("Colour to detect"=Box_Colour_FGV_Colours."Black", "Init/R/W State"=Box_Colour_FGV_States."Write") -> ()  [unwired: 8 in, 2 out]
          }
          frame 13 {
            # "Task 9: Blue Detection"
            n60 = call "Box Colour FGV.vi"("Colour to detect"=Box_Colour_FGV_Colours."Green", "Init/R/W State"=Box_Colour_FGV_States."Write") -> ()  [unwired: 8 in, 2 out]
          }
          frame 14 {
            # "Task 9: Yellow Detection"
            n61 = call "Box Colour FGV.vi"("Colour to detect"=Box_Colour_FGV_Colours."Red", "Init/R/W State"=Box_Colour_FGV_States."Write") -> ()  [unwired: 8 in, 2 out]
          }
          frame 15 {
            # "Task 9: Green Detection"
            n62 = call "Box Colour FGV.vi"("Colour to detect"=Box_Colour_FGV_Colours."Yellow", "Init/R/W State"=Box_Colour_FGV_States."Write") -> ()  [unwired: 8 in, 2 out]
          }
        }
        "Selected Task" <- w174
        n63 = Enqueue Element(queue=w178, element=w174, error in (no error)=w176) -> (queue out=w177:refnum<queue>, error out=w175:errorcluster)  [unwired: 1 in, 1 out]
      }
      event User Event {
        n64 = event-data() -> ("Stop Queue"=w211:bool)  [unwired: 1 in, 4 out]
        n65 = Enqueue Element At Opposite End(queue=w209, element=Intruction_Type_Definitions."Exit" ("Enum"), error in (no error)=w208) -> (queue out=w210:refnum<queue>, error out=w207:errorcluster)  [unwired: 1 in, 1 out]
      }
    }
  }
  n66 = while {
    tunnel: w46 -> [w214]
    tunnel: w47 -> [w272]
    tunnel: w50 -> [w270]
    tunnel: [w269] -> _
    tunnel: [w268] -> w40
    shift-right: [w261] -> _
    shift-left: T9 {"PING_A"=0, "PING_B"=0, "PING_C"=0, "PING_D"=0} -> [w263]
    shift-right: [w255] -> _
    shift-left: State_Type_Definitions,_for_0.26g_versions_and_later_3."Startup" ("Enum") -> [w258]
    shift-right: [w251] -> _
    shift-left: T8 {"xDistance"=0.0, "yDistance"=0.0, "wDistance"=0.0} -> [w253]
    shift-right: [w248] -> _
    shift-left: _ -> [w247]
    shift-right: [w244] -> _
    shift-left: T11 {"Recognized Object"=FALSE, "Object X coordinate"=0.0, "Object Y coordinate"=0.0} -> [w246]
    shift-right: [w241] -> _
    shift-left: T7 {"y Stepper Position"=0, "z Stepper Position"=0} -> [w243]
    shift-right: [w238] -> _
    shift-left: T6 {"Yaw"=0.0, "Compass"=0.0} -> [w240]
    shift-right: [w235] -> _
    shift-left: T3 {"Time up flag"=FALSE, "SET TIME TO CHECK"=0.0} -> [w237]
    shift-right: [w233] -> _
    shift-left: T20 {"yStepper desired"=0} -> [w234]
    shift-right: [w229] -> _
    shift-left: T5 {"Left IR Sensor"=0.0, "Arm IR Sensor"=0.0, "Bottom IR Sensor"=0.0} -> [w231]
    shift-right: [w227] -> _
    shift-left: T19 {"ySpeed"=0.0, "xSpeed"=0.0, "wSpeed"=0.0} -> [w228]
    shift-right: [w224] -> _
    shift-left: T4 {"Line Detected?"=FALSE, "S1"=0.0, "S2"=0.0, "S3"=0.0, "S4"=0.0} -> [w226]
    shift-right: [w222] -> _
    shift-left: _ -> [w221]
    shift-right: [w213] -> _
    shift-left: T1 {"Red"=FALSE, "Black"=FALSE, "Blue"=FALSE, "Yellow"=FALSE, "Green"=FALSE, "Unknown"=FALSE, "Image processing done"=FALSE, "Colour"=enum."None"} -> [w216]
    stop <- w260 stop-if-true
    # ">>> Box Colour Detection >>>"
    # ">>State Logic Queue Reference >>"
    # ">>Action Queue>>"
    # ">>State Logic Queue Reference >>"
    # ">>> Line Sensor Cluster>>>"
    # ">>> IR Sensors >>>"
    # ">>> Time cluster >>>"
    # ">>> Object detection >>>"
    # ">>> Yaw >>>"
    # ">>> Ultrasonic Sensors Detect >>>"
    # ">>> Encoders >>>"
    # ">>> Stepper position >>>"
    # ">>State Logic  >>"
    # ">> Item Selection Bias >>"
    # ">> Item Selection Bias >>"
    # ">> Item Selection Bias >>"
    # ">>State Logic  >>"
    # ">>> Motor control cluster >>>"
    # ">>> yStepper command>>>"
    # ">>True Stop Next State >>"
    # ">>Error  >>"
    # ">>Timeout>>"
    # ">>Action states Queue Reference >>"
    # "TOP LEVEL BASELINE (MAIN PROCESSING LOOP)"
    n67 = Wait (ms)(milliseconds to wait=u32 25) -> ()  [unwired: 1 out]
    n68 = Dequeue Element(queue=w272, timeout in ms (-1)=0, error in (no error)=w270) -> (queue out=w264:refnum<queue>, element=w271:string, error out=w265:errorcluster)  [unwired: 1 out]
    "Action State" <- w271
    n69 = case shown="\"READ STEPPER VALUES\"" w271 {
      tunnel: [_ _ _ _ _ _ _ _ _ _ _ _ _ _ _ _ _ _ _ _ 0 w3877 _ _ _ _ _ _ _ _ _ _ _ _ _ _ _ _ _ _ _ _ _ _ _ _ _ _ _ _ _ _ _ _ _ _ _] -> w267
      tunnel: w264 -> [_ _ _ _ _ _ _ _ _ _ _ _ _ _ _ _ _ _ _ _ _ _ _ _ _ _ _ _ _ _ _ _ _ _ _ _ _ _ _ _ _ _ _ _ _ _ _ _ _ _ _ _ _ _ _ _ _]
      tunnel: w263 -> [w3549 w3561 w3576 w3590 w3610 w3625 w3639 w3653 w3669 w3684 w3698 w3708 w3726 w3743 w3758 w3773 w3797 w3807 w3838 w3851 w3865 w3878 w3890 w3903 w3923 w3958 w3995 w4009 w4020 w4032 w4045 w4060 w4076 w4088 w4100 w4120 w4143 w4154 w4170 w4201 w4211 w4224 w4237 w4250 w4260 w4278 w4288 w4307 w4316 w4332 w4348 w4364 w4380 w4396 w4410 w4425 w4445]
      tunnel: [w3549 w3561 w3576 w3590 w3610 w3625 w3639 w3653 w3669 w3684 w3698 w3708 w3726 w3744 w3758 w3773 w3797 w3807 w3839 w3851 w3865 w3878 w3890 w3903 w3923 w3957 w3994 w4009 w4020 w4032 w4045 w4060 w4076 w4088 w4100 w4120 w4143 w4154 w4170 w4201 w4211 w4224 w4237 w4250 w4260 w4278 w4288 w4307 w4316 w4332 w4348 w4364 w4380 w4396 w4410 w4425 w4445] -> w262
      tunnel: [TRUE TRUE _ _ _ _ _ _ _ _ _ _ _ _ _ _ _ _ _ _ _ _ _ _ _ _ _ _ _ _ _ _ _ _ _ _ _ _ _ _ _ _ _ _ _ _ _ _ _ _ _ _ _ _ _ _ _] -> w260
      tunnel: w258 -> [w3547 w3559 w3575 w3589 w3609 w3624 w3638 w3652 w3668 w3683 w3697 w3707 w3725 w3742 w3757 w3771 w3790 w3806 w3837 w3850 w3862 w3875 w3889 w3902 w3922 w3956 w3993 w4008 w4019 w4031 w4037 w4059 w4075 w4087 w4099 w4119 w4142 w4153 w4164 w4195 w4210 w4223 w4236 w4249 w4259 w4269 w4287 w4306 w4315 w4331 w4347 w4363 w4379 w4395 w4409 w4415 w4433]
      tunnel: [_ _ _ _ _ _ _ _ _ _ _ _ _ _ _ _ _ _ _ _ _ TRUE _ _ _ _ _ _ _ _ _ _ _ _ _ _ _ _ _ _ _ _ _ _ _ _ _ _ _ _ _ _ _ _ _ _ _] -> w257
      tunnel: [w3547 w3559 w3575 w3589 w3609 w3624 w3638 w3652 w3668 w3683 w3697 w3707 w3725 w3742 w3757 w3771 w3790 w3806 w3837 w3850 w3862 w3875 w3889 w3902 w3922 w3956 w3993 w4008 w4019 w4031 w4037 w4059 w4075 w4087 w4099 w4119 w4142 w4153 w4164 w4195 w4210 w4223 w4236 w4249 w4259 w4269 w4287 w4306 w4315 w4331 w4347 w4363 w4379 w4395 w4409 w4415 w4433] -> w256
      tunnel: w253 -> [w3546 w3558 w3574 w3592 w3608 w3623 w3637 w3651 w3667 w3682 w3696 w3709 w3724 w3741 w3759 w3775 w3792 w3808 w3836 w3852 w3861 w3874 w3891 w3904 w3918 w3947 w3983 w4007 w4022 w4033 w4042 w4061 w4077 w4089 w4101 w4121 w4144 w4156 w4168 w4199 w4213 w4226 w4239 w4252 w4262 w4273 w4290 w4309 w4318 w4334 w4350 w4366 w4382 w4398 w4412 w4417 w4438]
      tunnel: [w3546 w3558 w3574 w3592 w3608 w3623 w3637 w3651 w3667 w3682 w3696 w3709 w3723 w3741 w3759 w3775 w3792 w3808 w3835 w3852 w3861 w3874 w3891 w3904 w3918 w3946 w3982 w4007 w4022 w4033 w4042 w4061 w4077 w4089 w4101 w4121 w4144 w4156 w4168 w4199 w4213 w4226 w4239 w4252 w4262 w4273 w4290 w4309 w4318 w4334 w4350 w4366 w4382 w4398 w4412 w4417 w4438] -> w252
      tunnel: w246 -> [w3545 w3557 w3573 w3591 w3607 w3622 w3636 w3650 w3666 w3681 w3694 w3706 w3722 w3740 w3752 w3774 w3791 w3805 w3827 w3849 w3860 w3873 w3888 w3901 w3921 w3951 w3988 w4005 w4021 w4030 w4043 w4058 w4074 w4083 w4098 w4117 w4137 w4155 w4169 w4200 w4212 w4225 w4238 w4251 w4261 w4272 w4289 w4308 w4317 w4333 w4349 w4365 w4381 w4397 w4411 w4416 w4437]
      tunnel: [w3545 w3557 w3573 w3591 w3607 w3622 w3636 w3650 w3666 w3681 w3694 w3706 w3722 w3740 w3752 w3774 w3791 w3805 w3826 w3849 w3860 w3873 w3888 w3901 w3920 w3950 w3987 w4005 w4021 w4030 w4043 w4058 w4074 w4083 w4098 w4116 w4137 w4155 w4169 w4200 w4212 w4225 w4238 w4251 w4261 w4272 w4289 w4308 w4317 w4333 w4349 w4365 w4381 w4397 w4411 w4416 w4437] -> w245
      tunnel: w243 -> [w3544 w3556 w3572 w3593 w3606 w3621 w3635 w3649 w3665 w3680 w3693 w3705 w3721 w3739 w3760 w3776 w3793 w3804 w3832 w3848 w3859 w3872 w3887 w3900 w3917 w3942 w3978 w4004 w4018 w4029 w4041 w4057 w4073 w4086 w4097 w4122 w4145 w4157 w4167 w4198 w4209 w4222 w4235 w4248 w4263 w4274 w4291 w4305 w4319 w4335 w4351 w4367 w4383 w4399 w4413 w4418 w4439]
      tunnel: [w3544 w3556 w3572 w3593 w3606 w3621 w3635 w3649 w3665 w3680 w3693 w3705 w3721 w3739 w3760 w3776 w3793 w3804 w3831 w3848 w3859 w3872 w3887 w3900 w3917 w3941 w3977 w4004 w4018 w4029 w4041 w4057 w4073 w4086 w4097 w4122 w4145 w4157 w4167 w4198 w4209 w4222 w4235 w4248 w4263 w4274 w4291 w4304 w4319 w4335 w4351 w4367 w4383 w4399 w4413 w4418 w4439] -> w242
      tunnel: w240 -> [w3543 w3555 w3570 w3594 w3604 w3619 w3633 w3648 w3663 w3678 w3692 w3704 w3720 w3732 w3755 w3777 w3794 w3803 w3822 w3847 w3858 w3871 w3886 w3899 w3916 w3938 w3974 w4003 w4015 w4028 w4040 w4056 w4072 w4085 w4096 w4123 w4146 w4158 w4166 w4197 w4208 w4219 w4232 w4245 w4264 w4275 w4292 w4299 w4320 w4336 w4352 w4368 w4384 w4400 w4414 w4419 w4440]
      tunnel: [w3543 w3555 w3570 w3594 w3604 w3619 w3633 w3648 w3663 w3678 w3692 w3704 w3720 w3732 w3754 w3777 w3794 w3803 w3821 w3847 w3858 w3871 w3886 w3899 w3916 w3937 w3973 w4003 w4015 w4028 w4040 w4056 w4072 w4085 w4096 w4123 w4146 w4158 w4166 w4197 w4208 w4219 w4232 w4245 w4264 w4275 w4292 w4299 w4320 w4336 w4352 w4368 w4384 w4400 w4414 w4419 w4440] -> w239
      tunnel: w237 -> [w3541 w3554 w3571 w3595 w3605 w3620 w3634 w3647 w3664 w3679 w3691 w3703 w3719 w3731 w3751 w3778 w3795 w3802 w3818 w3844 w3857 w3870 w3885 w3898 w3915 w3935 w3971 w4001 w4014 w4027 w4039 w4055 w4071 w4084 w4095 w4124 w4147 w4159 w4165 w4196 w4207 w4218 w4231 w4244 w4265 w4276 w4293 w4298 w4314 w4330 w4346 w4362 w4378 w4394 w4408 w4420 w4441]
      tunnel: [w3541 w3554 w3571 w3595 w3605 w3620 w3634 w3647 w3664 w3679 w3691 w3703 w3719 w3731 w3751 w3778 w3795 w3802 w3818 w3844 w3857 w3870 w3885 w3898 w3914 w3934 w3970 w4001 w4014 w4027 w4039 w4055 w4071 w4084 w4095 w4124 w4147 w4159 w4165 w4196 w4207 w4218 w4231 w4244 w4265 w4276 w4293 w4298 w4314 w4328 w4344 w4360 w4376 w4393 w4407 w4420 w4441] -> w236
      tunnel: w234 -> [_ _ _ _ _ _ _ _ _ _ _ _ _ _ _ _ _ _ _ _ _ _ _ _ _ _ _ _ _ _ _ _ _ _ _ _ _ _ _ _ _ _ _ _ _ _ w4284 _ _ _ _ _ _ _ _ _ _]
      tunnel: [w3540 w3553 w3565 w3585 w3599 w3614 w3629 w3643 w3659 w3673 w3688 w3702 w3713 w3730 w3748 w3769 w3796 w3801 w3815 w3843 w3856 w3869 w3884 w3895 w3908 w3928 w3962 w4000 w4013 w4026 w4044 w4049 w4065 w4081 w4093 w4112 w4140 w4151 w4171 w4202 w4206 w4217 w4230 w4243 w4256 w4277 w4282 w4297 w4313 w4326 w4342 w4358 w4374 w4391 w4404 w4424 w4444] -> w230
      tunnel: w231 -> [w3540 w3553 w3565 w3585 w3599 w3614 w3629 w3643 w3659 w3673 w3688 w3702 w3713 w3730 w3748 w3770 w3796 w3801 w3815 w3843 w3856 w3869 w3884 w3895 w3908 w3929 w3963 w4000 w4013 w4026 w4044 w4049 w4065 w4081 w4093 w4112 w4140 w4151 w4171 w4202 w4206 w4217 w4230 w4243 w4256 w4277 w4282 w4297 w4313 w4326 w4342 w4358 w4374 w4391 w4404 w4424 w4444]
      tunnel: w228 -> [_ _ _ _ _ _ _ _ w3658 _ _ _ _ _ _ _ _ _ _ _ _ _ _ _ _ _ _ _ _ _ _ _ _ _ _ _ _ _ _ _ _ _ _ _ _ _ _ _ _ _ _ _ _ _ _ _ _]
      tunnel: w226 -> [w3539 w3552 w3564 w3579 w3598 w3613 w3628 w3642 w3656 w3672 w3687 w3701 w3712 w3729 w3747 w3765 w3789 w3800 w3813 w3842 w3855 w3868 w3883 w3894 w3911 w3931 w3966 w3999 w4012 w4025 w4036 w4048 w4064 w4080 w4092 w4110 w4139 w4150 w4162 w4194 w4205 w4216 w4229 w4242 w4255 w4268 w4281 w4296 w4312 w4325 w4341 w4357 w4373 w4390 w4403 w4423 w4443]
      tunnel: [w3539 w3552 w3564 w3579 w3598 w3613 w3628 w3642 w3656 w3672 w3687 w3701 w3712 w3729 w3747 w3765 w3788 w3800 w3813 w3842 w3855 w3868 w3883 w3894 w3910 w3930 w3965 w3999 w4012 w4025 w4036 w4048 w4064 w4080 w4092 w4110 w4139 w4150 w4162 w4194 w4205 w4216 w4229 w4242 w4255 w4268 w4281 w4296 w4312 w4325 w4341 w4357 w4373 w4390 w4403 w4423 w4443] -> w225
      tunnel: [_ _ _ _ _ _ _ _ _ _ _ _ _ _ _ _ _ _ _ _ _ _ _ _ _ _ _ _ _ _ _ _ _ _ _ w4104 w4134 _ _ _ _ _ _ _ _ _ _ _ _ _ _ _ _ _ _ _ _] -> w223
      tunnel: w221 -> [w3538 w3551 w3563 w3578 w3597 w3612 w3627 w3641 w3655 w3671 w3686 w3700 w3711 w3728 w3746 w3764 w3780 w3799 w3811 w3841 w3854 w3867 w3882 w3893 w3912 w3932 w3967 w3998 w4011 w4024 w4035 w4047 w4063 w4079 w4091 w4106 w4138 w4149 w4161 w4193 w4204 w4215 w4228 w4241 w4254 w4267 w4280 w4295 w4311 w4324 w4340 w4356 w4372 w4389 w4402 w4422 w4442]
      tunnel: [w3538 w3551 w3563 w3578 w3597 w3612 w3627 w3641 w3655 w3671 w3686 w3700 w3711 w3728 w3746 w3764 w3780 w3799 w3811 w3841 w3854 w3867 w3882 w3893 w3912 w3932 w3967 w3998 w4011 w4024 w4035 w4047 w4063 w4079 w4091 w4106 w4138 w4149 w4161 w4193 w4204 w4215 w4228 w4241 w4254 w4267 w4280 w4295 w4311 w4324 w4340 w4356 w4372 w4389 w4402 w4422 w4442] -> w220
      tunnel: w216 -> [w3537 w3550 w3562 w3577 w3596 w3611 w3626 w3640 w3654 w3670 w3685 w3699 w3710 w3727 w3745 w3761 w3779 w3798 w3810 w3840 w3853 w3866 w3881 w3892 w3907 w3925 w3961 w3997 w4010 w4023 w4034 w4046 w4062 w4078 w4090 w4109 w4132 w4148 w4160 w4192 w4203 w4214 w4227 w4240 w4253 w4266 w4279 w4294 w4310 w4323 w4339 w4355 w4371 w4388 w4401 w4421 w4436]
      tunnel: [w3537 w3550 w3562 w3577 w3596 w3611 w3626 w3640 w3654 w3670 w3685 w3699 w3710 w3727 w3745 w3761 w3779 w3798 w3810 w3840 w3853 w3866 w3881 w3892 w3906 w3925 w3961 w3997 w4010 w4023 w4034 w4046 w4062 w4078 w4090 w4109 w4125 w4148 w4160 w4191 w4203 w4214 w4227 w4240 w4253 w4266 w4279 w4294 w4310 w4323 w4339 w4355 w4371 w4388 w4401 w4421 w4435] -> w215
      frame "Exit" {
        # ">>State Logic  >>"
        # ">>> Time cluster >>>"
        # ">>> Yaw >>>"
        # ">>> Stepper position >>>"
        # ">>> Encoders >>>"
        # ">>> Object detection >>>"
        # ">>> Ultrasonic Sensors Detect >>>"
        n70 = call "Imaq Dispose"("All Images? (No)"=TRUE) -> ()  [unwired: 5 in, 1 out]
      }
      frame "----Movement States----" {
        # ">>State Logic  >>"
        # ">>> Time cluster >>>"
        # ">>> Yaw >>>"
        # ">>> Stepper position >>>"
        # ">>> Encoders >>>"
        # ">>> Object detection >>>"
        # ">>> Ultrasonic Sensors Detect >>>"
      }
      frame "FORWARD" {
        # "High voltage values: 30\nMid voltage values: 40\nLow voltage values: 50"
        # ">>State Logic  >>"
        # ">>> Time cluster >>>"
        # ">>> Yaw >>>"
        # ">>> Stepper position >>>"
        # ">>> Encoders >>>"
        # ">>> Object detection >>>"
        # ">>> Ultrasonic Sensors Detect >>>"
        n71 = Unbundle By Name(w3570) -> ("Yaw"=w3566:dbl)
        n72 = call "MOTOR CONTROL WITH PID AE.vi"("Yaw"=w3566, "Speed"=30.0, "Direction"=MOTOR_CONTROL_WITH_PID_AE_DIRECTION_TYPE_DEF."y-axis movement", "AE Mode"=MOTOR_CONTROL_WITH_PID_AE_DATA_MODE_TYPE_DEF."Write to AE") -> ()  [unwired: 1 out]
      }
      frame "FORWARD - IR ASSIST" {
        # "Algorithm sensitivity"
        # "Distance to maintain from wall"
        # ">>State Logic  >>"
        # ">>> Time cluster >>>"
        # ">>> Yaw >>>"
        # ">>> Stepper position >>>"
        # ">>> Encoders >>>"
        # ">>> Object detection >>>"
        # ">>> Ultrasonic Sensors Detect >>>"
        n73 = Unbundle By Name(w3585) -> ("Left IR Sensor"=w3584:dbl)
        n74 = Subtract(x=w3584, y=20.0) -> (x-y=w3582:dbl)
        n75 = Multiply(x=w3582, y=0.2) -> (x*y=w3580:dbl)
        n76 = call "MOTOR CONTROL WITH PID AE.vi"("Yaw"=w3580, "Speed"=35.0, "Direction"=MOTOR_CONTROL_WITH_PID_AE_DIRECTION_TYPE_DEF."y-axis movement", "AE Mode"=MOTOR_CONTROL_WITH_PID_AE_DATA_MODE_TYPE_DEF."Write to AE") -> ()  [unwired: 1 out]
      }
      frame "LEFT" {
        # ">>State Logic  >>"
        # ">>> Time cluster >>>"
        # ">>> Yaw >>>"
        # ">>> Stepper position >>>"
        # ">>> Encoders >>>"
        # ">>> Object detection >>>"
        # ">>> Ultrasonic Sensors Detect >>>"
        n77 = Unbundle By Name(w3604) -> ("Yaw"=w3601:dbl)
        n78 = call "MOTOR CONTROL WITH PID AE.vi"("Yaw"=w3601, "Speed"=-25.0, "Direction"=MOTOR_CONTROL_WITH_PID_AE_DIRECTION_TYPE_DEF."x-axis movement", "AE Mode"=MOTOR_CONTROL_WITH_PID_AE_DATA_MODE_TYPE_DEF."Write to AE") -> ()  [unwired: 1 out]
      }
      frame "RIGHT" {
        # ">>> Time cluster >>>"
        # ">>> Yaw >>>"
        # ">>> Stepper position >>>"
        # ">>> Encoders >>>"
        # ">>> Object detection >>>"
        # ">>> Ultrasonic Sensors Detect >>>"
        n79 = Unbundle By Name(w3619) -> ("Yaw"=w3615:dbl)
        n80 = call "MOTOR CONTROL WITH PID AE.vi"("Yaw"=w3615, "Speed"=25.0, "Direction"=MOTOR_CONTROL_WITH_PID_AE_DIRECTION_TYPE_DEF."x-axis movement", "AE Mode"=MOTOR_CONTROL_WITH_PID_AE_DATA_MODE_TYPE_DEF."Write to AE") -> ()  [unwired: 1 out]
      }
      frame "R-ACW" {
        # ">>> IR Sensors >>>"
        # ">>> Time cluster >>>"
        # ">>> Yaw >>>"
        # ">>> Stepper position >>>"
        # ">>> Encoders >>>"
        # ">>> Object detection >>>"
        # ">>> Ultrasonic Sensors Detect >>>"
        n81 = call "MOTOR CONTROL WITH PID AE.vi"("Speed"=10.0, "Direction"=MOTOR_CONTROL_WITH_PID_AE_DIRECTION_TYPE_DEF."rotation", "AE Mode"=MOTOR_CONTROL_WITH_PID_AE_DATA_MODE_TYPE_DEF."Write to AE") -> ()  [unwired: 1 in, 1 out]
      }
      frame "R-CW" {
        (unwired) -0.2 ("Speed")
        # ">>> Time cluster >>>"
        # ">>> Yaw >>>"
        # ">>> Stepper position >>>"
        # ">>> Encoders >>>"
        # ">>> Object detection >>>"
        # ">>> Ultrasonic Sensors Detect >>>"
        n82 = call "MOTOR CONTROL WITH PID AE.vi"("Speed"=-10.0, "Direction"=MOTOR_CONTROL_WITH_PID_AE_DIRECTION_TYPE_DEF."rotation", "AE Mode"=MOTOR_CONTROL_WITH_PID_AE_DATA_MODE_TYPE_DEF."Write to AE") -> ()  [unwired: 1 in, 1 out]
      }
      frame "X AXIS - SLOW" {
        # ">>> Line Sensor Cluster>>>"
        # ">>> IR Sensors >>>"
        # ">>> Time cluster >>>"
        # ">>> Yaw >>>"
        # ">>> Stepper position >>>"
        # ">>> Encoders >>>"
        # ">>> Object detection >>>"
        # ">>> Ultrasonic Sensors Detect >>>"
        n83 = Unbundle By Name(w3658) -> ("xSpeed"=w3657:dbl)
        n84 = Unbundle By Name(w3663) -> ("Yaw"=w3660:dbl)
        n85 = call "MOTOR CONTROL WITH PID AE.vi"("Yaw"=w3660, "Speed"=w3657, "Direction"=MOTOR_CONTROL_WITH_PID_AE_DIRECTION_TYPE_DEF."x-axis movement", "AE Mode"=MOTOR_CONTROL_WITH_PID_AE_DATA_MODE_TYPE_DEF."Write to AE") -> ()  [unwired: 1 out]
      }
      frame "REVERSE" {
        # ">>> Time cluster >>>"
        # ">>> Yaw >>>"
        # ">>> Stepper position >>>"
        # ">>> Encoders >>>"
        # ">>> Object detection >>>"
        # ">>> Ultrasonic Sensors Detect >>>"
        n86 = Unbundle By Name(w3678) -> ("Yaw"=w3674:dbl)
        n87 = call "MOTOR CONTROL WITH PID AE.vi"("Yaw"=w3674, "Speed"=-40.0, "Direction"=MOTOR_CONTROL_WITH_PID_AE_DIRECTION_TYPE_DEF."y-axis movement", "AE Mode"=MOTOR_CONTROL_WITH_PID_AE_DATA_MODE_TYPE_DEF."Write to AE") -> ()  [unwired: 1 out]
      }
      frame "STOP" {
        n88 = Wait (ms)(milliseconds to wait=u32 100) -> ()  [unwired: 1 out]
        n89 = call "MOTOR CONTROL WITH PID AE.vi"("Direction"=MOTOR_CONTROL_WITH_PID_AE_DIRECTION_TYPE_DEF."stop", "AE Mode"=MOTOR_CONTROL_WITH_PID_AE_DATA_MODE_TYPE_DEF."Write to AE") -> ()  [unwired: 2 in, 1 out]
      }
      frame "----SENSOR READING---- " {
      }
      frame "READ ENCODERS" {
        # ">>> Time cluster >>>"
        # ">>> Yaw >>>"
        # ">>> Stepper position >>>"
        # ">>> Object detection >>>"
        # ">>> Current encoder distance >>>"
        # ">>> Ultrasonic Sensors Detect >>>"
        n90 = call "MOTOR CONTROL WITH PID AE.vi"("AE Mode"=MOTOR_CONTROL_WITH_PID_AE_DATA_MODE_TYPE_DEF."Read from AE") -> ("Speed & distance"=w3717:T15)  [unwired: 3 in]
        n91 = Unbundle By Name(w3717) -> ("xDistance"=w3716:dbl, "yDistance"=w3715:dbl, "wDistance"=w3714:dbl)
        n92 = Bundle By Name(cluster=w3724, "xDistance"=w3716, "yDistance"=w3715, "wDistance"=w3714) -> (w3723:T8)
      }
      frame "READ ULTRASONIC" {
        (unwired) navX_type_def."Read Values" ("Mode")
        (unwired) MOTOR_CONTROL_NO_PID_Type_Def."Latch" ("Direction")
        # ">>> Line Sensor Cluster>>>"
        # ">>> IR Sensors >>>"
        # ">>State Logic  >>"
        # ">>> Time cluster >>>"
        # ">>> Ultrasonic Sensors Detect >>>"
        # ">>> Object detection >>>"
        # ">>> Encoders >>>"
        # ">>> Stepper position >>>"
        # ">>> Yaw >>>"
        n93 = call "Arduino Interfacing VI.vi"("AE Mode"=Arduino_Interfacing."Read From Arduino") -> ("Arduino Data"=w3737:T17)  [unwired: 3 in, 1 out]
        n94 = Unbundle By Name(w3737) -> ("PING A"=w3736:u8, "PING B"=w3735:u8, "PING C"=w3734:u8, "PING D"=w3733:u8)
        n95 = Bundle By Name(cluster=w3743, "PING_A"=w3736, "PING_B"=w3735, "PING_C"=w3734, "PING_D"=w3733) -> (w3744:T9)
      }
      frame "READ NAVX" {
        # ">> Item Selection Bias >>"
        # ">>State Logic  >>"
        # ">>> Line Sensor Cluster>>>"
        # ">>> IR Sensors >>>"
        # ">>> Time cluster >>>"
        # ">>> Yaw >>>"
        # ">>> Ultrasonic Sensors Detect >>>"
        # ">>> Object detection >>>"
        # ">>> Encoders >>>"
        # ">>> Stepper position >>>"
        n96 = call "navX reading VI.vi"("Mode"=navX_type_def."Read Values") -> ("NavX Readings"=w3750:T16)  [unwired: 2 in, 3 out]
        n97 = Unbundle By Name(w3750) -> ("Heading"=w3749:dbl)
        n98 = Unbundle By Name(w3750) -> ("Yaw"=w3753:dbl)
        n99 = Bundle By Name(cluster=w3755, "Yaw"=w3753, "Compass"=w3749) -> (w3754:T6)
      }
      frame "READ IR" {
        w3763 = T40 [enum."B/AI2"] items=["Not Connected", "AudioIn/Left", "AudioIn/Right", "C/AI0", "C/AI1", "A/AI0", "A/AI1", "A/AI2", "A/AI3", "A/AI4", "A/AI5", "A/AI6", "A/AI7", "B/AI0", "B/AI1", "B/AI2", "B/AI3", "B/AI4", "B/AI5", "B/AI6", "B/AI7", "AI/AI0", "AI/AI1", "AI/AI2", "AI/AI3", "A/AI0 (DIFF)", "A/AI1 (DIFF)", "A/AI2 (DIFF)", "A/AI3 (DIFF)", "B/AI0 (DIFF)", "B/AI1 (DIFF)", "B/AI2 (DIFF)", "B/AI3 (DIFF)"] ("AI Channel")
        w3767 = T40 [enum."B/AI1"] items=["Not Connected", "AudioIn/Left", "AudioIn/Right", "C/AI0", "C/AI1", "A/AI0", "A/AI1", "A/AI2", "A/AI3", "A/AI4", "A/AI5", "A/AI6", "A/AI7", "B/AI0", "B/AI1", "B/AI2", "B/AI3", "B/AI4", "B/AI5", "B/AI6", "B/AI7", "AI/AI0", "AI/AI1", "AI/AI2", "AI/AI3", "A/AI0 (DIFF)", "A/AI1 (DIFF)", "A/AI2 (DIFF)", "A/AI3 (DIFF)", "B/AI0 (DIFF)", "B/AI1 (DIFF)", "B/AI2 (DIFF)", "B/AI3 (DIFF)"] ("AI Channel")
        w3772 = T40 [enum."B/AI0"] items=["Not Connected", "AudioIn/Left", "AudioIn/Right", "C/AI0", "C/AI1", "A/AI0", "A/AI1", "A/AI2", "A/AI3", "A/AI4", "A/AI5", "A/AI6", "A/AI7", "B/AI0", "B/AI1", "B/AI2", "B/AI3", "B/AI4", "B/AI5", "B/AI6", "B/AI7", "AI/AI0", "AI/AI1", "AI/AI2", "AI/AI3", "A/AI0 (DIFF)", "A/AI1 (DIFF)", "A/AI2 (DIFF)", "A/AI3 (DIFF)", "B/AI0 (DIFF)", "B/AI1 (DIFF)", "B/AI2 (DIFF)", "B/AI3 (DIFF)"] ("AI Channel")
        # ">>> Line Sensor Cluster>>>"
        # ">>> IR Sensors >>>"
        # ">>State Logic  >>"
        # ">>> Time cluster >>>"
        # ">>> Ultrasonic Sensors Detect >>>"
        # ">>> Object detection >>>"
        # ">>> Encoders >>>"
        # ">>> Stepper position >>>"
        # ">>> Yaw >>>"
        n100 = call <vilib>:"Sharp IR.vi"("AI Channel"=w3772) -> ("Sharp IR Distance"=w3768:dbl)  [unwired: 8 in, 2 out]
        n101 = call <vilib>:"Sharp IR.vi"("AI Channel"=w3767) -> ("Sharp IR Distance"=w3766:dbl)  [unwired: 8 in, 2 out]
        n102 = call <vilib>:"Sharp IR.vi"("AI Channel"=w3763) -> ("Sharp IR Distance"=w3762:dbl)  [unwired: 8 in, 2 out]
        n103 = Bundle By Name(cluster=w3770, "Left IR Sensor"=w3768, "Arm IR Sensor"=w3766, "Bottom IR Sensor"=w3762) -> (w3769:T5)
      }
      frame "READ LINE SENSOR" {
        # ">>> IR Sensors >>>"
        # ">>> Line Sensor Cluster>>>"
        # ">>State Logic  >>"
        # ">>> Time cluster >>>"
        # ">>> Object detection >>>"
        # ">>> Yaw >>>"
        # ">>> Ultrasonic Sensors Detect >>>"
        # ">>> Encoders >>>"
        # ">>> Stepper position >>>"
        n104 = call "Line Sensor AE.vi"("AE State"=Line_Sensor_AE_Type_Def."READ FROM LINE SENSORS") -> ("Line Detected?"=w3786:bool, "Line Sensor Raw Values"=w3785:T42)
        n105 = Unbundle By Name(w3785) -> ("S1"=w3784:dbl, "S2"=w3783:dbl, "S3"=w3782:dbl, "S4"=w3781:dbl)
        n106 = Bundle By Name(cluster=w3789, "Line Detected?"=w3786, "S1"=w3784, "S2"=w3783, "S3"=w3782, "S4"=w3781) -> (w3788:T4)
      }
      frame "----SYSTEM MODES----" {
        (unwired) I2C_MASTER_Type_Def."Last State" ("Arduino Mode")
        # ">>> Object detection >>>"
        # ">>> Yaw >>>"
        # ">>> Ultrasonic Sensors Detect >>>"
        # ">>> Encoders >>>"
        # ">>> Stepper position >>>"
      }
      frame "INIT" {
        w3833 = u8 0
        w3834 = 0.0
        # ">>> IR Sensors >>>"
        # ">>> IR Sensors >>>"
        # ">>> Line Sensor Cluster>>>"
        # ">>> Time cluster >>>"
        # ">>> Object detection >>>"
        # ">>> Yaw >>>"
        # ">>> Ultrasonic Sensors Detect >>>"
        # ">>> Encoders >>>"
        # ">>> Stepper position >>>"
        # ">>State Logic  >>"
        n107 = call "Arduino Interfacing VI.vi"("AE Mode"=Arduino_Interfacing."Initialize") -> ()  [unwired: 3 in, 2 out]
        n108 = call "FGV Bool.vi"("Init/Read/Write State"=States_for_Action_Engine."Initialize") -> ()  [unwired: 2 in, 2 out]
        n109 = call "Elasped Timer.vi"("Action"=Elapsed_timer_control."Initialize") -> ()  [unwired: 7 in, 4 out]
        n110 = call "MOTOR CONTROL WITH PID AE.vi"("AE Mode"=MOTOR_CONTROL_WITH_PID_AE_DATA_MODE_TYPE_DEF."Init AE") -> ()  [unwired: 3 in, 1 out]
        n111 = call "IMAQ Reference AE.vi"("IMAQ AE States"=IMAQ_Reference_AE."Initialize AE") -> ()  [unwired: 1 in, 2 out]
        n112 = call "Line Sensor AE.vi"("AE State"=Line_Sensor_AE_Type_Def."INIT AE") -> ()  [unwired: 2 out]
        n113 = Bundle By Name(cluster=w3827, "Recognized Object"=FALSE, "Object X coordinate"=0.0, "Object Y coordinate"=0.0) -> (w3826:T11)
        n114 = Bundle By Name(cluster=w3832, "y Stepper Position"=u8 0, "z Stepper Position"=u8 0) -> (w3831:T7)
        n115 = Bundle By Name(cluster=w3836, "xDistance"=w3834, "yDistance"=w3834, "wDistance"=w3834) -> (w3835:T8)
        n116 = Bundle By Name(cluster=w3838, "PING_A"=w3833, "PING_B"=w3833, "PING_C"=w3833, "PING_D"=w3833) -> (w3839:T9)
        n117 = invoke class="VI" method="Default Vals.Reinit All"() -> ()  [unwired: 3 in, 3 out]
        n118 = Bundle By Name(cluster=w3822, "Yaw"=0.0) -> (w3821:T6)
        n119 = call "Box Colour FGV.vi"("Init/R/W State"=Box_Colour_FGV_States."Initialize") -> ()  [unwired: 9 in, 2 out]
      }
      frame "ARDUINO - ULTRASONIC" {
        # ">>> Time cluster >>>"
        # ">>> Line Sensor Cluster>>>"
        # ">>> Object detection >>>"
        # ">>> Yaw >>>"
        # ">>> Ultrasonic Sensors Detect >>>"
        # ">>> Encoders >>>"
        # ">>> Stepper position >>>"
        # ">>State Logic  >>"
        n120 = call "Arduino Interfacing VI.vi"("Data to Write"=I2C_MASTER_WRITE_NEW_Type_Def."Ultrasonic sensors", "AE Mode"=Arduino_Interfacing."Write to Arduino") -> ()  [unwired: 2 in, 2 out]
      }
      frame "NAVX CALIBRATE" {
        # ">>> Object detection >>>"
        # ">>> Yaw >>>"
        # ">>> Ultrasonic Sensors Detect >>>"
        # ">>> Encoders >>>"
        # ">>> Stepper position >>>"
        # ">>State Logic  >>"
        # "Adds a 15 second delay to the startup process \nfor the NavX to calibrate"
        n121 = Wait (ms)(milliseconds to wait=u32 1000) -> ()  [unwired: 1 out]
      }
      frame "NO ACTION", Default {
        (unwired) u8 0 ("y Stepper value")
        (unwired) TRUE ("Latch")
        (unwired) navX_type_def."Read Values" ("Mode")
        (unwired) MOTOR_CONTROL_NO_PID_Type_Def."Latch" ("Direction")
        # ">>> Object detection >>>"
        # ">>> Yaw >>>"
        # ">>> Ultrasonic Sensors Detect >>>"
        # ">>> Encoders >>>"
        # ">>> Stepper position >>>"
        # ">>State Logic  >>"
        n122 = case shown="\"Idle\"" w3875 {
          tunnel: [0 100] -> w3877
          frame "Startup", Default {
          }
          frame "Idle" {
          }
        }
      }
      frame "----RESET CASES----" {
        (unwired) I2C_MASTER_Type_Def."Last State" ("Arduino Mode")
        # ">>> Object detection >>>"
        # ">>> Yaw >>>"
        # ">>> Ultrasonic Sensors Detect >>>"
        # ">>> Encoders >>>"
        # ">>> Stepper position >>>"
        # ">>State Logic  >>"
      }
      frame "RESET ENCODERS" {
        # ">>> Object detection >>>"
        # ">>> Yaw >>>"
        # ">>> Ultrasonic Sensors Detect >>>"
        # ">>> Encoders >>>"
        # ">>> Stepper position >>>"
        # ">>State Logic  >>"
        n123 = call "MOTOR CONTROL WITH PID AE.vi"("Direction"=MOTOR_CONTROL_WITH_PID_AE_DIRECTION_TYPE_DEF."reset encoders", "AE Mode"=MOTOR_CONTROL_WITH_PID_AE_DATA_MODE_TYPE_DEF."Write to AE") -> ()  [unwired: 2 in, 1 out]
      }
      frame "RESET FLAGS" {
        w3905 = FALSE ("Line Detected?")
        # ">>> Line Sensor Cluster>>>"
        # ">>> IR Sensors >>>"
        # ">>> Time cluster >>>"
        # ">>> Object detection >>>"
        # ">>> Yaw >>>"
        # ">>> Ultrasonic Sensors Detect >>>"
        # ">>> Encoders >>>"
        # ">>> Stepper position >>>"
        # ">>> Line Sensor Cluster>>>"
        # ">>> IR Sensors >>>"
        # ">>> Time cluster >>>"
        # ">>> Object detection >>>"
        # ">>> Yaw >>>"
        # ">>> Ultrasonic Sensors Detect >>>"
        # ">>> Encoders >>>"
        # ">>> Stepper position >>>"
        # "Resets BOOLEAN FLAGS only"
        n124 = Wait (ms)(milliseconds to wait=u32 20) -> ()  [unwired: 1 out]
        n125 = Bundle By Name(cluster=w3921, "Recognized Object"=FALSE) -> (w3920:T11)
        n126 = Bundle By Name(cluster=w3911, "Line Detected?"=FALSE) -> (w3910:T4)
        n127 = Bundle By Name(cluster=w3915, "Time up flag"=FALSE) -> (w3914:T3)
        n128 = Bundle By Name(cluster=w3907, "Red"=w3905, "Black"=w3905, "Blue"=w3905, "Yellow"=w3905, "Green"=w3905, "Unknown"=w3905, "Image processing done"=w3905) -> (w3906:T1)
      }
      frame "RESET SENSOR VALUES" {
        w3926 = 0.0 ("S4")
        w3927 = 0.0 ("S4")
        # "Resets SENSOR VALUES only"
        # ">>> Line Sensor Cluster>>>"
        # ">>> IR Sensors >>>"
        # ">>> Time cluster >>>"
        # ">>> Object detection >>>"
        # ">>> Yaw >>>"
        # ">>> Ultrasonic Sensors Detect >>>"
        # ">>> Encoders >>>"
        # ">>> Stepper position >>>"
        # ">>> Line Sensor Cluster>>>"
        # ">>> IR Sensors >>>"
        # ">>> Time cluster >>>"
        # ">>> Object detection >>>"
        # ">>> Yaw >>>"
        # ">>> Ultrasonic Sensors Detect >>>"
        # ">>> Encoders >>>"
        # ">>> Stepper position >>>"
        # "Resets any software variables\nand/or non-critical states"
        n129 = Wait (ms)(milliseconds to wait=u32 20) -> ()  [unwired: 1 out]
        n130 = Bundle By Name(cluster=w3935, "SET TIME TO CHECK"=0.0) -> (w3934:T3)
        n131 = Bundle By Name(cluster=w3951, "Object X coordinate"=0.0, "Object Y coordinate"=0.0) -> (w3950:T11)
        n132 = Bundle By Name(cluster=w3942, "y Stepper Position"=u8 0, "z Stepper Position"=u8 0) -> (w3941:T7)
        n133 = Bundle By Name(cluster=w3929, "Left IR Sensor"=w3926, "Arm IR Sensor"=w3926) -> (w3928:T5)
        n134 = Bundle By Name(cluster=w3947, "xDistance"=0.0, "yDistance"=0.0, "wDistance"=0.0) -> (w3946:T8)
        n135 = Bundle By Name(cluster=w3958, "PING_A"=u8 0, "PING_B"=u8 0, "PING_C"=u8 0, "PING_D"=u8 0) -> (w3957:T9)
        n136 = Bundle By Name(cluster=w3938, "Yaw"=0.0) -> (w3937:T6)
        n137 = Bundle By Name(cluster=w3931, "S1"=w3927, "S2"=w3927, "S3"=w3927, "S4"=w3927) -> (w3930:T4)
      }
      frame "RESET ALL SENSORS" {
        w3960 = 0.0 ("SET TIME TO CHECK")
        # ">>> Line Sensor Cluster>>>"
        # ">>> IR Sensors >>>"
        # ">>> Time cluster >>>"
        # ">>> Object detection >>>"
        # ">>> Yaw >>>"
        # ">>> Ultrasonic Sensors Detect >>>"
        # ">>> Encoders >>>"
        # ">>> Stepper position >>>"
        # ">>> Line Sensor Cluster>>>"
        # ">>> IR Sensors >>>"
        # ">>> Time cluster >>>"
        # ">>> Object detection >>>"
        # ">>> Yaw >>>"
        # ">>> Ultrasonic Sensors Detect >>>"
        # ">>> Encoders >>>"
        # ">>> Stepper position >>>"
        # "Resets ALL SENSOR PARAMTERS"
        n138 = Wait (ms)(milliseconds to wait=u32 20) -> ()  [unwired: 1 out]
        n139 = Bundle By Name(cluster=w3971, "Time up flag"=FALSE, "SET TIME TO CHECK"=0.0) -> (w3970:T3)
        n140 = Bundle By Name(cluster=w3988, "Recognized Object"=FALSE, "Object X coordinate"=0.0, "Object Y coordinate"=0.0) -> (w3987:T11)
        n141 = Bundle By Name(cluster=w3978, "y Stepper Position"=u8 0, "z Stepper Position"=u8 0) -> (w3977:T7)
        n142 = Bundle By Name(cluster=w3963, "Left IR Sensor"=w3960, "Arm IR Sensor"=w3960, "Bottom IR Sensor"=w3960) -> (w3962:T5)
        n143 = Bundle By Name(cluster=w3966, "Line Detected?"=FALSE) -> (w3965:T4)
        n144 = Bundle By Name(cluster=w3983, "xDistance"=0.0, "yDistance"=0.0, "wDistance"=0.0) -> (w3982:T8)
        n145 = Bundle By Name(cluster=w3995, "PING_A"=u8 0, "PING_B"=u8 0, "PING_C"=u8 0, "PING_D"=u8 0) -> (w3994:T9)
        n146 = Bundle By Name(cluster=w3974, "Yaw"=0.0) -> (w3973:T6)
      }
      frame "RESET YAW" {
        n147 = Wait (ms)(milliseconds to wait=u32 100) -> ()  [unwired: 1 out]
        n148 = call "navX reading VI.vi"("Mode"=navX_type_def."Zero Yaw") -> ()  [unwired: 2 in, 4 out]
      }
      frame "RESET ARM" {
        n149 = call "Arduino Interfacing VI.vi"("Data to Write"=I2C_MASTER_WRITE_NEW_Type_Def."Soft Reset", "AE Mode"=Arduino_Interfacing."Write to Arduino") -> ()  [unwired: 2 in, 2 out]
      }
      frame "--------CAM STATES-------" {
      }
      frame "OPEN IMAQ REF" {
        # ">>> Line Sensor Cluster>>>"
        # ">>State Logic  >>"
        # ">>> Time cluster >>>"
        # ">>> Object detection >>>"
        # ">>> Yaw >>>"
        # ">>> Ultrasonic Sensors Detect >>>"
        # ">>> Encoders >>>"
        # ">>> Stepper position >>>"
        # ">>> IR Sensors >>>"
        n150 = call "IMAQ Reference AE.vi"("IMAQ AE States"=IMAQ_Reference_AE."Initialize AE") -> ()  [unwired: 1 in, 2 out]
      }
      frame "OPEN LOG CAM" {
        n151 = call "Webcam AE.vi"("Session In"=T38 "cam0", "Camera states"=Webcam_AE."Initialize Camera") -> ("error out"=w4052:errorcluster, "Session Out"=w4051:T38)  [unwired: 1 in, 1 out]
        n152 = call "Webcam AE.vi"("error in (no error)"=w4052, "Session In"=w4051, "Camera states"=Webcam_AE."Open Camera") -> ()  [unwired: 3 out]
      }
      frame "OPEN LIFE CAM" {
        n153 = call "Webcam AE.vi"("Session In"=T38 "cam1", "Camera states"=Webcam_AE."Initialize Camera") -> ("error out"=w4068:errorcluster, "Session Out"=w4067:T38)  [unwired: 1 in, 1 out]
        n154 = call "Webcam AE.vi"("error in (no error)"=w4068, "Session In"=w4067, "Camera states"=Webcam_AE."Open Camera") -> ()  [unwired: 3 out]
      }
      frame "CAM ACQ" {
        # ">>State Logic  >>"
        # ">>> Time cluster >>>"
        # ">>> Yaw >>>"
        # ">>> Stepper position >>>"
        # ">>> Encoders >>>"
        # ">>> Object detection >>>"
        # ">>> Ultrasonic Sensors Detect >>>"
        n155 = call "Webcam AE.vi"("Camera states"=Webcam_AE."Continuous Acquisition") -> ()  [unwired: 2 in, 3 out]
      }
      frame "CAM CLOSE" {
        # ">>> Box Colour Detection >>>"
        # ">>> Line Sensor Cluster>>>"
        # ">>> IR Sensors >>>"
        # ">>State Logic  >>"
        # ">>> Time cluster >>>"
        # ">>> Yaw >>>"
        # ">>> Stepper position >>>"
        # ">>> Encoders >>>"
        # ">>> Object detection >>>"
        # ">>> Ultrasonic Sensors Detect >>>"
        n156 = call "Webcam AE.vi"("Camera states"=Webcam_AE."Close Camera") -> ()  [unwired: 2 in, 3 out]
      }
      frame "PROCESS IMAGE" {
        # ">>> Line Sensor Cluster>>>"
        # ">>> IR Sensors >>>"
        # ">> Item Selection Bias >>"
        # ">> Item Selection Bias >>"
        # ">>State Logic  >>"
        # ">>> Time cluster >>>"
        # ">>> Yaw >>>"
        # ">>> Stepper position >>>"
        # ">>> Encoders >>>"
        # ">>> Object detection >>>"
        # ">>> Ultrasonic Sensors Detect >>>"
        n157 = call "Webcam AE.vi"("Camera states"=Webcam_AE."Retrieve Image") -> ("error out"=w4105:errorcluster, "Image Out"=w4108:T44)  [unwired: 2 in, 1 out]
        n158 = call "IMAQ Reference AE.vi"("IMAQ AE States"=IMAQ_Reference_AE."Get IMAQ Reference") -> ("Image Out"=w4107:T44)  [unwired: 1 in, 1 out]
        n159 = call "Object Detection SubVI v2.vi"("Error In"=w4105, "Mode"=w4106, "Image Dest"=w4107, "Image in"=w4108) -> ("Error out"=w4104:errorcluster, "Object Center Coordinates"=w4103:cluster{"x":sgl, "y":sgl}, "Object detection cluster"=w4102:T45)  [unwired: 1 out]
        n160 = Unbundle By Name(w4102) -> ("Object detected?"=w4113:bool)
        n161 = Unbundle By Name(w4103) -> ("x"=w4115:sgl, "y"=w4114:sgl)
        n162 = Bundle By Name(cluster=w4117, "Recognized Object"=w4113, "Object X coordinate"=w4115, "Object Y coordinate"=w4114) -> (w4116:T11)
      }
      frame "COLOUR PROCESSING" {
        # ">>> Box Colour Detection >>>"
        # ">>> Box Colour Detection >>>"
        # ">>> Line Sensor Cluster>>>"
        # ">>> IR Sensors >>>"
        # ">> Item Selection Bias >>"
        # ">> Item Selection Bias >>"
        # ">>State Logic  >>"
        # ">>> Time cluster >>>"
        # ">>> Yaw >>>"
        # ">>> Stepper position >>>"
        # ">>> Encoders >>>"
        # ">>> Object detection >>>"
        # ">>> Ultrasonic Sensors Detect >>>"
        n163 = call "Webcam AE.vi"("Camera states"=Webcam_AE."Retrieve Image") -> ("error out"=w4135:errorcluster, "Image Out"=w4136:T44)  [unwired: 2 in, 1 out]
        n164 = call "Box Colour Detection SubVI.vi"("Image In"=w4136, "Error In"=w4135) -> ("Colour output boolean cluster"=w4133:T46, "Error out"=w4134:errorcluster)  [unwired: 1 out]
        n165 = Unbundle By Name(w4133) -> ("Red"=w4131:bool, "Black"=w4130:bool, "Blue"=w4129:bool, "Yellow"=w4128:bool, "Green"=w4127:bool, "No recognizable coolour"=w4126:bool)
        n166 = Bundle By Name(cluster=w4132, "Red"=w4131, "Black"=w4130, "Blue"=w4129, "Yellow"=w4128, "Green"=w4127, "Unknown"=w4126) -> (w4125:T1)
      }
      frame "DISPOSE CAM BUFFERS" {
        # ">> Item Selection Bias >>"
        # ">>> Line Sensor Cluster>>>"
        # ">>> IR Sensors >>>"
        # ">>State Logic  >>"
        # ">>> Time cluster >>>"
        # ">>> Yaw >>>"
        # ">>> Stepper position >>>"
        # ">>> Encoders >>>"
        # ">>> Object detection >>>"
        # ">>> Ultrasonic Sensors Detect >>>"
        n167 = call "Webcam AE.vi"("Camera states"=Webcam_AE."Dispose Camera Image Buffer") -> ()  [unwired: 2 in, 3 out]
      }
      frame "DISPOSE PROC BUFFERS" {
        # ">>> Box Colour Detection >>>"
        # ">>> Line Sensor Cluster>>>"
        # ">>State Logic  >>"
        # ">>> IR Sensors >>>"
        # ">>> Time cluster >>>"
        # ">>> Object detection >>>"
        # ">>> Yaw >>>"
        # ">>> Ultrasonic Sensors Detect >>>"
        # ">>> Encoders >>>"
        # ">>> Stepper position >>>"
        n168 = call "IMAQ Reference AE.vi"("IMAQ AE States"=IMAQ_Reference_AE."Dispose Processing Buffer") -> ()  [unwired: 1 in, 2 out]
      }
      frame "BOX COLOUR" {
        # ">>> Box Colour Detection >>>"
        # ">>> Line Sensor Cluster>>>"
        # ">>State Logic  >>"
        # ">>> IR Sensors >>>"
        # ">>> Time cluster >>>"
        # ">>> Object detection >>>"
        # ">>> Yaw >>>"
        # ">>> Ultrasonic Sensors Detect >>>"
        # ">>> Encoders >>>"
        # ">>> Stepper position >>>"
        n169 = call "Box Colour Detection Sequence.vi"() -> ("Colour scan time out?"=w4188:bool, "Colour output boolean cluster"=w4190:T46)  [unwired: 9 in, 1 out]
        n170 = Unbundle By Name(w4190) -> ("Red"=w4187:bool, "Black"=w4183:bool, "Blue"=w4180:bool, "Yellow"=w4179:bool, "Green"=w4176:bool, "No recognizable coolour"=w4189:bool)
        n171 = Select(t=Box_Colour_FGV_Colours."Green" ("Colour"), s=w4176, f=Box_Colour_FGV_Colours."None" ("Colour")) -> (s? t:f=w4174:T2)
        n172 = Select(t=Box_Colour_FGV_Colours."Yellow" ("Colour"), s=w4179, f=w4174) -> (s? t:f=w4173:T2)
        n173 = Select(t=Box_Colour_FGV_Colours."Blue" ("Colour"), s=w4180, f=w4173) -> (s? t:f=w4182:T2)
        n174 = Select(t=Box_Colour_FGV_Colours."Black" ("Colour"), s=w4183, f=w4182) -> (s? t:f=w4185:T2)
        n175 = Select(t=Box_Colour_FGV_Colours."Red" ("Colour"), s=w4187, f=w4185) -> (s? t:f=w4172:T2)
        n176 = Bundle By Name(cluster=w4192, "Red"=w4187, "Black"=w4183, "Blue"=w4180, "Yellow"=w4179, "Green"=w4176, "Unknown"=w4189, "Image processing done"=w4188, "Colour"=w4172) -> (w4191:T1)
      }
      frame "-----ARM ACTIONS-----" {
      }
      frame "CLOSE CLAW" {
        n177 = call "Arduino Interfacing VI.vi"("Data to Write"=I2C_MASTER_WRITE_NEW_Type_Def."Close Claw", "AE Mode"=Arduino_Interfacing."Write to Arduino") -> ()  [unwired: 2 in, 2 out]
      }
      frame "OPEN CLAW" {
        n178 = call "Arduino Interfacing VI.vi"("Data to Write"=I2C_MASTER_WRITE_NEW_Type_Def."Open Claw", "AE Mode"=Arduino_Interfacing."Write to Arduino") -> ()  [unwired: 2 in, 2 out]
      }
      frame "Z STEPPER CAM HEIGHT" {
        n179 = call "Arduino Interfacing VI.vi"("Data to Write"=I2C_MASTER_WRITE_NEW_Type_Def."zStepper 6k", "AE Mode"=Arduino_Interfacing."Write to Arduino") -> ()  [unwired: 2 in, 2 out]
      }
      frame "Z STEPPER GRAB HEIGHT" {
        # ">>State Logic  >>"
        # ">>> Time cluster >>>"
        # ">>> Yaw >>>"
        # ">>> Stepper position >>>"
        # ">>> Encoders >>>"
        # ">>> Object detection >>>"
        # ">>> Ultrasonic Sensors Detect >>>"
        n180 = call "Arduino Interfacing VI.vi"("Data to Write"=I2C_MASTER_WRITE_NEW_Type_Def."zStepper 100", "AE Mode"=Arduino_Interfacing."Write to Arduino") -> ()  [unwired: 2 in, 2 out]
      }
      frame "Z STEPPER BOX HEIGHT" {
        # ">>> IR Sensors >>>"
        # ">>> Time cluster >>>"
        # ">>> Yaw >>>"
        # ">>> Stepper position >>>"
        # ">>> Encoders >>>"
        # ">>> Object detection >>>"
        # ">>> Ultrasonic Sensors Detect >>>"
        n181 = call "Arduino Interfacing VI.vi"("Data to Write"=I2C_MASTER_WRITE_NEW_Type_Def."zStepper 5k", "AE Mode"=Arduino_Interfacing."Write to Arduino") -> ()  [unwired: 2 in, 2 out]
      }
      frame "Y STEPPER CONTROL" {
        # ">>State Logic  >>"
        # ">>> yStepper command>>>"
        # ">>> Time cluster >>>"
        # ">>> Yaw >>>"
        # ">>> Stepper position >>>"
        # ">>> Encoders >>>"
        # ">>> Object detection >>>"
        # ">>> Ultrasonic Sensors Detect >>>"
        n182 = Unbundle By Name(w4284) -> ("yStepper desired"=w4283:u8)
        n183 = call "Arduino Interfacing VI.vi"("y Stepper value"=w4283, "Data to Write"=I2C_MASTER_WRITE_NEW_Type_Def."yStepper control", "AE Mode"=Arduino_Interfacing."Write to Arduino") -> ()  [unwired: 1 in, 2 out]
      }
      frame "READ STEPPER VALUES" {
        # ">>State Logic  >>"
        # ">>> Time cluster >>>"
        # ">>> Yaw >>>"
        # ">>> Stepper position >>>"
        # ">>> Encoders >>>"
        # ">>> Object detection >>>"
        # ">>> Ultrasonic Sensors Detect >>>"
        n184 = call "Arduino Interfacing VI.vi"("AE Mode"=Arduino_Interfacing."Read From Arduino") -> ("Arduino Data"=w4302:T17)  [unwired: 3 in, 1 out]
        n185 = Unbundle By Name(w4302) -> ("y Stepper Position"=w4301:u8, "z Stepper Position"=w4300:u8)
        n186 = Bundle By Name(cluster=w4305, "y Stepper Position"=w4301, "z Stepper Position"=w4300) -> (w4304:T7)
      }
      frame " -----TIMING-----" {
        # ">>State Logic  >>"
        # ">>> Time cluster >>>"
        # ">>> Yaw >>>"
        # ">>> Stepper position >>>"
        # ">>> Encoders >>>"
        # ">>> Object detection >>>"
        # ">>> Ultrasonic Sensors Detect >>>"
      }
      frame "SET TIMER 1" {
        w4321 = 1.0 ("Time Setting")
        # ">>State Logic  >>"
        # ">>> Time cluster >>>"
        # ">>> Yaw >>>"
        # ">>> Stepper position >>>"
        # ">>> Encoders >>>"
        # ">>> Object detection >>>"
        # ">>> Ultrasonic Sensors Detect >>>"
        n187 = Wait (ms)(milliseconds to wait=u32 250) -> ()  [unwired: 1 out]
        n188 = call "Elasped Timer.vi"("Time Setting"=w4321, "Action"=Elapsed_timer_control."Initialize") -> ()  [unwired: 6 in, 4 out]
        n189 = Bundle By Name(cluster=w4330, "Time up flag"=FALSE, "SET TIME TO CHECK"=w4321) -> (w4328:T3)
      }
      frame "SET TIMER 2" {
        w4337 = 2.0 ("Time Setting")
        # ">>State Logic  >>"
        # ">>> Time cluster >>>"
        # ">>> Yaw >>>"
        # ">>> Stepper position >>>"
        # ">>> Encoders >>>"
        # ">>> Object detection >>>"
        # ">>> Ultrasonic Sensors Detect >>>"
        n190 = Wait (ms)(milliseconds to wait=u32 250) -> ()  [unwired: 1 out]
        n191 = call "Elasped Timer.vi"("Time Setting"=w4337, "Action"=Elapsed_timer_control."Initialize") -> ()  [unwired: 6 in, 4 out]
        n192 = Bundle By Name(cluster=w4346, "Time up flag"=FALSE, "SET TIME TO CHECK"=w4337) -> (w4344:T3)
      }
      frame "SET TIMER 3" {
        w4353 = 3.0 ("Time Setting")
        # ">>State Logic  >>"
        # ">>> Time cluster >>>"
        # ">>> Yaw >>>"
        # ">>> Stepper position >>>"
        # ">>> Encoders >>>"
        # ">>> Object detection >>>"
        # ">>> Ultrasonic Sensors Detect >>>"
        n193 = Wait (ms)(milliseconds to wait=u32 250) -> ()  [unwired: 1 out]
        n194 = call "Elasped Timer.vi"("Time Setting"=w4353, "Action"=Elapsed_timer_control."Initialize") -> ()  [unwired: 6 in, 4 out]
        n195 = Bundle By Name(cluster=w4362, "Time up flag"=FALSE, "SET TIME TO CHECK"=w4353) -> (w4360:T3)
      }
      frame "SET TIMER 4" {
        w4369 = 4.0 ("Time Setting")
        # ">>State Logic  >>"
        # ">>> Time cluster >>>"
        # ">>> Yaw >>>"
        # ">>> Stepper position >>>"
        # ">>> Encoders >>>"
        # ">>> Object detection >>>"
        # ">>> Ultrasonic Sensors Detect >>>"
        n196 = call "Elasped Timer.vi"("Time Setting"=w4369, "Action"=Elapsed_timer_control."Initialize") -> ()  [unwired: 6 in, 4 out]
        n197 = Wait (ms)(milliseconds to wait=u32 250) -> ()  [unwired: 1 out]
        n198 = Bundle By Name(cluster=w4378, "Time up flag"=FALSE, "SET TIME TO CHECK"=w4369) -> (w4376:T3)
      }
      frame "SET TIMER 5" {
        w4386 = 5.0 ("Time Setting")
        # ">>State Logic  >>"
        # ">>> Time cluster >>>"
        # ">>> Yaw >>>"
        # ">>> Stepper position >>>"
        # ">>> Encoders >>>"
        # ">>> Object detection >>>"
        # ">>> Ultrasonic Sensors Detect >>>"
        n199 = call "Elasped Timer.vi"("Time Setting"=w4386, "Action"=Elapsed_timer_control."Initialize") -> ("Time Out?!"=w4385:bool)  [unwired: 6 in, 3 out]
        n200 = Wait (ms)(milliseconds to wait=u32 250) -> ()  [unwired: 1 out]
        n201 = Bundle By Name(cluster=w4394, "Time up flag"=w4385, "SET TIME TO CHECK"=w4386) -> (w4393:T3)
      }
      frame "START TIMER" {
        # ">>State Logic  >>"
        # ">>> Time cluster >>>"
        # ">>> Yaw >>>"
        # ">>> Stepper position >>>"
        # ">>> Encoders >>>"
        # ">>> Object detection >>>"
        # ">>> Ultrasonic Sensors Detect >>>"
        n202 = call "Elasped Timer.vi"("Action"=Elapsed_timer_control."Start") -> ("Time Out?!"=w4405:bool)  [unwired: 7 in, 3 out]
        n203 = Bundle By Name(cluster=w4408, "Time up flag"=w4405) -> (w4407:T3)
      }
      frame "-----MISC-----" {
        # ">>> Box Colour Detection >>>"
        # ">>> Line Sensor Cluster>>>"
        # ">>> IR Sensors >>>"
        # ">>> Time cluster >>>"
        # ">>> Object detection >>>"
        # ">>> Yaw >>>"
        # ">>> Ultrasonic Sensors Detect >>>"
        # ">>> Encoders >>>"
        # ">>> Stepper position >>>"
      }
      frame "Task 9" {
        # ">>> Box Colour Detection >>>"
        # ">>> Line Sensor Cluster>>>"
        # ">>> IR Sensors >>>"
        # ">>> Time cluster >>>"
        # ">>> Object detection >>>"
        # ">>> Yaw >>>"
        # ">>> Ultrasonic Sensors Detect >>>"
        # ">>> Encoders >>>"
        # ">>> Stepper position >>>"
        n204 = call "Colour Processing Test Env.vi"() -> ("Colour scan time out?"=w4434:bool, "Colour output boolean cluster"=w4432:T46)  [unwired: 10 in]
        n205 = Unbundle By Name(w4432) -> ("Red"=w4426:bool, "Black"=w4427:bool, "Blue"=w4428:bool, "Yellow"=w4429:bool, "Green"=w4430:bool, "No recognizable coolour"=w4431:bool)
        n206 = Bundle By Name(cluster=w4436, "Red"=w4426, "Black"=w4427, "Blue"=w4428, "Yellow"=w4429, "Green"=w4430, "Unknown"=w4431, "Image processing done"=w4434) -> (w4435:T1)
      }
    }
    "State Logic" <- w256
    "Image Processing Error" <- w223
    n207 = local read "TASK ENABLE"() -> (w250:bool)
    n208 = Not(x=w250) -> (.not. x?=w249:bool)
    n209 = case shown="True" w257 {
      tunnel: w214 -> [w288 w342]
      tunnel: w264 -> [w284 w344]
      tunnel: [w288 w342] -> w269
      tunnel: [w284 w345] -> w268
      tunnel: w265 -> [_ w340]
      tunnel: w267 -> [_ w341]
      tunnel: w262 -> [w287 w347]
      tunnel: [w287 w347] -> w261
      tunnel: "STOP TASK" -> [_ w330]
      tunnel: w256 -> [w286 w346]
      tunnel: [w286 w343] -> w255
      tunnel: w252 -> [w285 w336]
      tunnel: [w285 w336] -> w251
      tunnel: w249 -> [_ w331]
      tunnel: [w283 w328] -> w248
      tunnel: w247 -> [w283 w327]
      tunnel: w245 -> [w282 w324]
      tunnel: [w282 w324] -> w244
      tunnel: w242 -> [w281 w320]
      tunnel: [w281 w320] -> w241
      tunnel: w239 -> [w280 w318]
      tunnel: [w280 w318] -> w238
      tunnel: w236 -> [w279 w316]
      tunnel: [w279 w316] -> w235
      tunnel: w234 -> [w278 w315]
      tunnel: [w278 w314] -> w233
      tunnel: [_ w312] -> w232
      tunnel: w230 -> [w277 w310]
      tunnel: [w277 w310] -> w229
      tunnel: w228 -> [w276 w309]
      tunnel: [w276 w308] -> w227
      tunnel: w225 -> [w275 w305]
      tunnel: [w275 w305] -> w224
      tunnel: [w274 w304] -> w222
      tunnel: w220 -> [w274 w303]
      tunnel: [_ w301] -> w219
      tunnel: [_ w300] -> w218
      tunnel: [_ w299] -> w217
      tunnel: w215 -> [w273 w298]
      tunnel: [w273 w298] -> w213
      tunnel: [_ w289] -> w212
      frame False {
        # ">>> Box Colour Detection >>>"
        # ">>> Line Sensor Cluster>>>"
        # ">> Item Selection Bias >>"
        # ">>State Logic Queue Reference >>"
        # ">>Action states Queue Reference >>"
        # ">>True Stop Next State >>"
        # ">>State Logic  >>"
        # ">>> IR Sensors >>>"
        # ">>> Line Sensor Cluster>>>"
        # ">>> Line Sensor Cluster>>>"
        # ">>> Motor control cluster >>>"
        # ">>> yStepper command>>>"
        # ">>> Motor control cluster >>>"
        # ">>> yStepper command>>>"
        # ">>> Motor control cluster >>>"
        # ">>> IR Sensors >>>"
        # ">>> IR Sensors >>>"
        # ">>> yStepper command>>>"
        # ">>> Time cluster >>>"
        # ">>> Yaw >>>"
        # ">>> Stepper position >>>"
        # ">>> Encoders >>>"
        # ">>> Object detection >>>"
        # ">>> Ultrasonic Sensors Detect >>>"
        # ">>> Time cluster >>>"
        # ">>> Yaw >>>"
        # ">>> Stepper position >>>"
        # ">>> Encoders >>>"
        # ">>> Object detection >>>"
        # ">>> Ultrasonic Sensors Detect >>>"
      }
      frame True {
        # ">>> Box colour cluster >>>"
        # ">>State Logic Queue Reference >>"
        # ">>> Box Colour Detection >>>"
        # ">> Item Selection Bias >>"
        # ">>> IR Sensors >>>"
        # ">>> Line Sensor Cluster>>>"
        # ">>> Line Sensor Cluster>>>"
        # ">>> Motor control cluster >>>"
        # ">>> yStepper command>>>"
        # ">>> IR Sensors >>>"
        # ">>> Motor control cluster >>>"
        # ">>State Logic Queue Reference >>"
        # ">>Timeout>>"
        # ">>> yStepper command>>>"
        # ">>> Time cluster >>>"
        # ">>> Object detection >>>"
        # ">>> Yaw >>>"
        # ">>> Ultrasonic Sensors Detect >>>"
        # ">>> Encoders >>>"
        # ">>> Stepper position >>>"
        # ">>State Logic  >>"
        # ">>True Stop Next State >>"
        # ">>Action Queue>>"
        # ">> Manual override >>"
        # ">>> Time cluster >>>"
        # ">>> Yaw >>>"
        # ">>> Stepper position >>>"
        # ">>> Encoders >>>"
        # ">>> Object detection >>>"
        # ">>> Ultrasonic Sensors Detect >>>"
        # ">>Action Queue>>"
        # ">>State Logic Queue Reference >>"
        n210 = Or(x=w330, y=w331) -> (x .or. y?=w329:bool)
        n211 = Unbundle By Name(w298) -> ("Red"=w297:bool, "Black"=w296:bool, "Blue"=w295:bool, "Yellow"=w294:bool, "Green"=w293:bool, "Unknown"=w292:bool, "Image processing done"=w291:bool, "Colour"=w290:T2)
        n212 = Unbundle By Name(w305) -> ("Line Detected?"=w306:bool)
        n213 = Unbundle By Name(w310) -> ("Left IR Sensor"=w311:dbl, "Arm IR Sensor"=w307:dbl, "Bottom IR Sensor"=w302:dbl)
        n214 = Unbundle By Name(w316) -> ("Time up flag"=w317:bool)
        n215 = Unbundle By Name(w318) -> ("Yaw"=w319:dbl, "Compass"=w313:dbl)
        n216 = Unbundle By Name(w320) -> ("y Stepper Position"=w322:u8, "z Stepper Position"=w321:u8)
        n217 = Unbundle By Name(w336) -> ("xDistance"=w333:dbl, "yDistance"=w334:dbl, "wDistance"=w335:dbl)
        n218 = Unbundle By Name(w324) -> ("Recognized Object"=w323:bool, "Object X coordinate"=w326:dbl, "Object Y coordinate"=w325:dbl)
        n219 = Unbundle By Name(w347) -> ("PING_A"=w339:u8, "PING_B"=w338:u8, "PING_C"=w337:u8, "PING_D"=w332:u8)
        n220 = case shown="\"Task A5: ROTATE CW 90\"" w346 {
          tunnel: [w352 w364 w378 w389 w507 w524 w570 w608 w662 w704 w753 w796 w851 w899 w943 w1003 w1044 w1087 w1136 w1179 w1232 w1270 w1322 w1368 w1414 w1455 w1504 w1548 w1594 w1635 w1684 w1728 w1774 w1815 w1864 w1908 w1954 w1995 w2044 w2079 w2097 w2145 w2186 w2236 w2292 w2331 w2380 w2423 w2476 w2514 w2566 w2603 w2651 w2694 w2744 w2788 w2836 w2892 w2933 w2985 w3033 w3078 w3122 w3170 w3221 w3264 w3313 w3361 w3404 w3450 w3500] -> w345
          tunnel: w344 -> [w352 w367 w379 w392 w509 w525 w571 w617 w660 w708 w754 w802 w844 w902 w950 w993 w1047 w1093 w1135 w1182 w1222 w1276 w1312 w1363 w1406 w1454 w1503 w1547 w1586 w1634 w1683 w1727 w1766 w1814 w1863 w1907 w1946 w1994 w2043 w2079 w2087 w2148 w2192 w2235 w2291 w2337 w2379 w2426 w2466 w2520 w2556 w2607 w2658 w2699 w2749 w2793 w2837 w2890 w2934 w2986 w3035 w3084 w3129 w3175 w3220 w3260 w3317 w3368 w3409 w3455 w3501]
          tunnel: [State_Type_Definitions,_for_0.26g_versions_and_later_3."Idle" ("Enum") State_Type_Definitions,_for_0.26g_versions_and_later_3."Idle" ("Enum") w374 w391 State_Type_Definitions,_for_0.26g_versions_and_later_3."Shutdown" ("Enum") w526 w572 w615 w663 w705 w752 w797 w850 w900 w945 w1002 w1045 w1094 w1137 w1181 w1231 w1277 w1321 w1369 w1407 w1456 w1505 w1549 w1587 w1636 w1685 w1729 w1767 w1816 w1865 w1909 w1947 w1996 w2045 State_Type_Definitions,_for_0.26g_versions_and_later_3."Idle" ("Enum") w2096 w2146 w2193 w2237 w2293 w2338 w2381 w2425 w2475 w2521 w2565 w2604 w2652 w2695 w2745 w2789 w2835 w2893 w2932 w2984 w3034 w3077 w3124 w3176 w3222 w3263 w3314 w3362 w3405 w3451 w3499] -> w343
          tunnel: w342 -> [_ _ w377 w395 _ w530 w577 w611 w659 w709 w760 w801 w848 w903 w949 w1000 w1042 w1092 w1133 w1183 w1229 w1275 w1319 w1366 w1413 w1452 w1501 w1545 w1593 w1632 w1681 w1725 w1773 w1812 w1861 w1905 w1953 w1992 w2041 _ w2094 w2143 w2191 w2233 w2289 w2336 w2377 w2427 w2473 w2519 w2563 w2611 w2657 w2702 w2752 w2796 w2845 w2889 w2935 w2979 w3036 w3083 w3128 w3174 w3219 w3269 w3321 w3367 w3412 w3458 w3494]
          tunnel: w341 -> [_ _ _ w394 _ w529 w576 w610 w658 w710 w759 w800 w847 w896 w948 w999 w1041 w1091 w1132 w1184 w1228 w1274 w1318 w1365 w1411 w1451 w1500 w1544 w1591 w1631 w1680 w1724 w1771 w1811 w1860 w1904 w1951 w1991 w2040 _ w2093 w2142 w2190 w2232 w2288 w2335 w2376 w2428 w2472 w2518 w2562 w2606 w2656 w2701 w2751 w2795 w2843 w2888 w2936 w2980 w3037 w3082 w3127 w3173 w3218 w3268 w3316 w3366 w3411 w3457 w3495]
          tunnel: w340 -> [_ _ w376 w390 _ w528 w575 w609 w657 w711 w758 w799 w846 w895 w947 w1001 w1043 w1090 w1131 w1185 w1230 w1273 w1320 w1364 w1412 w1450 w1499 w1543 w1592 w1630 w1679 w1723 w1772 w1810 w1859 w1903 w1952 w1990 w2039 _ w2095 w2144 w2189 w2231 w2287 w2334 w2375 w2429 w2474 w2517 w2564 w2610 w2655 w2700 w2750 w2794 w2844 w2887 w2937 w2981 w3038 w3081 w3126 w3172 w3217 w3267 w3320 w3365 w3410 w3456 w3496]
          tunnel: w329 -> [_ _ _ _ _ w515 w569 w616 w656 w712 w755 w795 w849 w901 w951 w994 w1048 w1088 w1134 w1186 w1223 w1271 w1313 w1367 w1409 w1453 w1502 w1546 w1589 w1633 w1682 w1726 w1769 w1813 w1862 w1906 w1949 w1993 w2042 _ w2088 w2149 w2187 w2234 w2290 w2332 w2378 w2430 w2467 w2515 w2557 w2609 w2650 w2698 w2748 w2792 w2839 w2886 w2938 w2982 w3039 w3080 w3125 w3171 w3216 w3266 w3319 w3360 w3408 w3454 w3497]
          tunnel: w339 -> [_ _ _ _ _ _ _ _ _ _ _ _ _ _ _ _ _ _ _ _ _ _ _ _ _ _ _ _ _ _ _ _ _ _ _ _ _ _ _ _ _ _ _ _ _ _ _ _ _ _ _ _ _ _ _ _ _ _ _ _ _ _ _ _ _ _ _ _ _ _ _]
          tunnel: w338 -> [_ _ _ _ _ _ _ _ w655 _ _ _ w840 w884 w941 _ _ _ _ _ _ _ _ _ _ _ _ _ _ _ _ _ _ _ _ _ _ _ _ _ _ w2135 _ _ _ _ _ _ _ _ _ _ _ _ _ _ _ _ _ _ _ _ _ _ _ _ _ _ _ _ _]
          tunnel: w337 -> [_ _ _ _ _ _ _ _ w654 _ _ _ w841 w885 w942 _ _ _ _ _ _ _ _ _ _ _ _ _ _ _ _ _ _ _ _ _ _ _ _ _ _ w2136 _ _ _ _ _ _ _ _ _ _ _ _ _ _ _ _ _ _ _ _ _ _ _ _ _ _ _ _ _]
          tunnel: w335 -> [_ _ _ _ _ _ _ _ _ _ w757 _ _ _ _ _ _ _ _ _ _ _ _ _ _ _ _ _ _ _ _ _ _ _ _ _ _ _ _ _ _ _ _ _ _ _ _ _ _ _ _ _ _ _ _ _ _ _ _ w2978 _ _ _ _ _ _ _ _ _ _ w3493]
          tunnel: w334 -> [_ _ _ _ _ w523 w568 _ _ w703 _ _ _ _ w946 _ _ _ _ _ _ _ _ _ _ _ _ _ _ _ _ _ _ _ w1852 _ _ _ w2032 _ _ _ _ _ _ _ _ _ _ _ _ _ _ _ _ _ _ _ _ _ _ _ _ _ _ _ _ _ _ w3447 _]
          tunnel: w333 -> [_ _ _ _ _ _ _ _ _ _ _ _ _ w890 _ _ _ _ _ _ _ _ _ _ _ _ w1492 _ _ _ w1672 _ _ _ _ _ _ _ _ _ _ _ _ _ w2278 _ _ _ _ _ _ _ _ _ _ _ _ w2879 _ _ _ _ _ _ _ _ _ _ _ _ _]
          tunnel: w332 -> [_ _ _ _ _ _ _ _ _ _ _ _ _ _ _ _ _ _ _ _ _ _ _ _ _ _ _ _ _ _ _ _ _ _ _ _ _ _ _ _ _ _ _ _ _ _ _ _ _ _ _ _ _ _ _ _ _ _ _ _ _ _ _ _ _ _ _ _ _ _ _]
          tunnel: [State_Type_Definitions,_for_0.26g_versions_and_later_3."Idle" ("Enum") State_Type_Definitions,_for_0.26g_versions_and_later_3."Idle" ("Enum") State_Type_Definitions,_for_0.26g_versions_and_later_3."Idle" ("Enum") State_Type_Definitions,_for_0.26g_versions_and_later_3."Idle" ("Enum") State_Type_Definitions,_for_0.26g_versions_and_later_3."Shutdown" ("Enum") w521 w566 w614 w661 w706 w749 w794 w843 w898 w944 w1004 w1046 w1086 w1138 w1180 w1233 w1269 w1323 w1370 w1408 w1457 w1506 w1550 w1588 w1637 w1686 w1730 w1768 w1817 w1866 w1910 w1948 w1997 w2046 w2081 w2098 w2147 w2185 w2238 w2294 w2330 w2382 w2424 w2477 w2513 w2567 w2605 w2653 w2697 w2747 w2791 w2834 w2891 w2931 w2983 w3032 w3076 w3123 w3177 w3223 w3262 w3315 w3363 w3407 w3453 w3498] -> w328
          tunnel: w327 -> [_ _ w374 _ _ _ _ _ _ _ _ _ _ _ _ _ _ _ _ _ _ _ _ _ _ _ _ _ _ _ _ _ _ _ _ _ _ _ _ w2081 _ _ _ _ _ _ _ _ _ _ _ _ _ _ _ _ _ _ _ _ _ _ _ _ _ _ _ _ _ _ _]
          tunnel: w323 -> [_ _ _ _ _ _ _ _ _ _ _ _ _ _ _ _ _ _ _ _ _ _ _ _ _ w1444 _ _ _ w1624 _ _ _ w1804 _ _ _ w1984 _ _ _ _ _ w2226 _ _ _ _ _ _ _ _ _ _ _ _ _ _ _ _ _ _ _ _ _ _ _ _ _ _ _]
          tunnel: w326 -> [_ _ _ _ _ _ _ _ _ _ _ _ _ _ _ _ _ _ _ _ _ _ _ _ _ _ _ _ _ _ _ _ _ _ _ _ _ _ _ _ _ _ _ _ w2284 _ _ _ _ _ _ _ _ _ _ _ _ _ _ _ _ _ _ _ _ _ _ _ _ _ _]
          tunnel: w325 -> [_ _ _ _ _ _ _ _ _ _ _ _ _ _ _ _ _ _ _ w1175 _ _ _ _ _ _ _ _ _ _ _ _ _ _ _ _ _ _ _ _ _ _ _ _ _ _ _ w2419 _ _ _ _ _ _ _ _ _ _ _ _ _ _ _ _ _ _ _ _ _ _ _]
          tunnel: w322 -> [_ _ _ _ _ _ _ _ _ _ _ _ _ _ _ _ _ _ _ w1174 _ _ _ _ _ _ _ _ _ _ _ _ _ _ _ _ _ _ _ _ _ _ _ _ _ _ _ w2418 _ _ _ _ _ _ _ _ _ _ _ _ _ _ _ _ _ _ _ _ _ _ _]
          tunnel: w321 -> [_ _ _ _ _ _ _ w613 _ _ _ w792 _ _ _ w997 _ w1082 _ _ w1226 _ w1316 w1362 _ _ _ _ _ _ _ _ _ _ _ _ _ _ _ _ w2091 _ _ _ _ _ _ _ w2470 _ w2560 w2608 _ _ _ _ _ _ _ _ _ _ _ _ _ _ w3318 _ _ _ _]
          tunnel: w319 -> [_ _ _ _ _ _ _ _ _ _ _ _ _ _ _ _ _ _ _ _ _ _ _ _ _ _ _ _ _ _ _ _ _ _ _ _ _ _ _ _ _ _ _ _ _ _ _ _ _ _ _ _ _ _ _ _ _ _ _ _ _ _ _ _ _ _ _ _ _ _ _]
          tunnel: w317 -> [_ _ _ _ _ _ _ _ _ _ _ _ _ _ _ _ _ _ w1128 _ _ w1267 _ _ w1402 w1445 _ _ w1582 w1625 _ _ w1762 w1805 _ _ w1942 w1985 _ _ _ _ w2183 w2225 _ w2328 w2372 _ _ w2511 _ _ _ _ _ _ _ _ _ _ _ _ _ _ _ _ _ _ _ _ _]
          tunnel: w315 -> [w350 w362 w373 w387 w505 w520 w565 w612 w653 w707 w748 w793 w842 w894 w940 w992 w1039 w1085 w1129 w1177 w1221 w1268 w1311 w1360 w1405 w1448 w1497 w1541 w1585 w1628 w1677 w1721 w1765 w1808 w1857 w1901 w1945 w1988 w2037 w2082 w2086 w2140 w2184 w2229 w2285 w2329 w2373 w2421 w2465 w2512 w2555 w2602 w2654 w2696 w2746 w2790 w2842 w2885 w2940 w2988 w3041 w3088 w3131 w3179 w3225 w3274 w3312 w3364 w3406 w3452 w3503]
          tunnel: [w350 w361 w373 w387 w505 w520 w565 w612 w653 w707 w748 w793 w842 w894 w940 w992 w1039 w1085 w1129 w1176 w1221 w1268 w1311 w1360 w1405 w1448 w1497 w1541 w1585 w1628 w1677 w1721 w1765 w1808 w1857 w1901 w1945 w1988 w2037 w2082 w2086 w2140 w2184 w2229 w2285 w2329 w2373 w2420 w2465 w2512 w2555 w2602 w2654 w2696 w2746 w2790 w2842 w2885 w2940 w2988 w3041 w3088 w3131 w3179 w3225 w3274 w3312 w3364 w3406 w3452 w3503] -> w314
          tunnel: w313 -> [_ _ _ _ _ _ _ _ _ _ _ _ _ _ _ _ _ _ _ _ _ _ _ _ _ _ _ _ _ _ _ _ _ _ _ _ _ _ _ _ _ _ _ _ _ _ _ _ _ _ _ _ w2649 _ _ _ _ _ _ _ _ _ _ _ _ _ _ w3359 _ _ _]
          tunnel: [_ _ _ TRUE _ w514 w562 w605 w650 w699 w745 w788 _ _ _ _ _ _ _ _ _ _ _ w1356 _ w1445 _ _ _ w1625 _ _ _ w1805 _ _ _ w1985 _ _ _ _ _ w2225 w2273 _ _ _ _ _ _ w2599 w2644 w2691 w2735 w2785 w2829 w2878 w2926 w2976 w3023 _ _ _ w3215 w3259 w3309 w3354 w3401 _ w3491] -> w312
          tunnel: w311 -> [_ _ _ _ _ _ _ _ _ _ _ _ _ _ _ _ _ _ _ _ _ _ _ _ _ _ _ _ _ _ _ _ _ _ _ _ _ _ _ _ _ _ _ _ _ _ _ _ _ _ _ _ _ _ _ _ _ _ _ _ _ w3075 _ _ _ _ _ _ _ _ _]
          tunnel: w309 -> [w349 w359 w372 w385 w504 w519 w564 w607 w652 w701 w747 w790 w835 w883 w939 w991 w1038 w1084 w1127 w1171 w1220 w1266 w1310 w1359 w1404 w1447 w1496 w1540 w1584 w1627 w1676 w1720 w1764 w1807 w1856 w1900 w1944 w1987 w2036 w2083 w2085 w2134 w2182 w2228 w2281 w2327 w2371 w2415 w2464 w2510 w2554 w2601 w2646 w2693 w2743 w2787 w2841 w2884 w2942 w2990 w3043 w3089 w3133 w3181 w3227 w3275 w3311 w3356 w3403 w3449 w3505]
          tunnel: [w349 w358 w372 w385 w504 w519 w564 w607 w652 w701 w747 w790 w835 w883 w939 w991 w1038 w1084 w1127 w1171 w1220 w1266 w1310 w1359 w1404 w1447 w1496 w1540 w1584 w1627 w1676 w1720 w1764 w1807 w1856 w1900 w1944 w1987 w2036 w2083 w2085 w2134 w2182 w2228 w2280 w2327 w2371 w2415 w2464 w2510 w2554 w2601 w2646 w2693 w2743 w2787 w2841 w2884 w2942 w2990 w3043 w3089 w3133 w3181 w3227 w3275 w3311 w3356 w3403 w3449 w3505] -> w308
          tunnel: w307 -> [_ _ _ _ _ _ _ _ _ _ _ _ _ _ _ _ _ _ _ _ _ _ _ _ _ _ _ _ _ _ _ _ _ _ _ _ _ _ _ _ _ _ _ _ _ _ _ _ _ _ _ _ _ _ w2741 _ _ _ _ _ w3030 _ _ _ _ _ _ _ _ _ _]
          tunnel: w306 -> [_ _ _ _ _ w516 _ _ _ _ _ _ _ _ w937 _ _ _ _ _ _ _ _ _ _ _ _ _ _ _ _ _ _ _ _ _ _ _ _ _ _ _ _ _ _ _ _ _ _ _ _ _ _ w2691 _ w2785 _ w2880 _ _ _ _ w3121 _ w3215 _ _ _ w3401 _ _]
          tunnel: [w348 w354 w371 w384 w503 w518 w563 w606 w651 w700 w746 w789 w834 w882 w938 w990 w1037 w1083 w1126 w1170 w1219 w1265 w1309 w1358 enum16{"Ball", "Soap", "Gel", "Pipe", "None"}."Ball" ("Object recognition mode") w1446 w1495 enum16{"Ball", "Soap", "Gel", "Pipe", "None"}."Soap" ("Object recognition mode") enum16{"Ball", "Soap", "Gel", "Pipe", "None"}."Soap" ("Object recognition mode") w1626 w1675 enum16{"Ball", "Soap", "Gel", "Pipe", "None"}."Gel" ("Object recognition mode") enum16{"Ball", "Soap", "Gel", "Pipe", "None"}."Gel" ("Object recognition mode") w1806 w1855 enum16{"Ball", "Soap", "Gel", "Pipe", "None"}."Pipe" ("Object recognition mode") enum16{"Ball", "Soap", "Gel", "Pipe", "None"}."Pipe" ("Object recognition mode") w1986 w2035 w2078 w2084 w2133 w2181 w2227 w2274 w2326 w2370 w2414 w2463 w2509 w2553 w2600 w2645 w2692 w2740 w2786 w2840 w2883 w2941 w2989 w3042 w3079 w3132 w3180 w3226 w3265 w3310 w3355 w3402 w3448 w3504] -> w304
          tunnel: w303 -> [w348 w354 w371 _ w503 w518 w563 w606 w651 w700 w746 w789 w834 w882 w938 w990 w1037 w1083 w1126 w1170 w1219 w1265 w1309 w1358 _ w1446 w1495 _ _ w1626 w1675 _ _ w1806 w1855 _ _ w1986 w2035 w2078 w2084 w2133 w2181 w2227 w2274 w2326 w2370 w2414 w2463 w2509 w2553 w2600 w2645 w2692 w2740 w2786 w2840 w2883 w2941 w2989 w3042 w3079 w3132 w3180 w3226 w3265 w3310 w3355 w3402 w3448 w3504]
          tunnel: w302 -> [_ _ _ _ _ _ _ _ _ _ _ _ _ _ _ _ _ _ _ _ _ _ _ _ _ _ _ _ _ _ _ _ _ _ _ _ _ _ _ _ _ w2132 _ _ _ _ _ _ _ _ _ _ _ _ w2739 _ _ _ _ _ w3024 _ _ _ _ _ _ _ _ _ _]
          tunnel: [_ _ _ _ _ _ _ _ w650 _ _ _ _ _ _ _ _ _ _ _ _ _ _ _ _ _ _ _ _ _ _ _ _ _ _ _ _ _ _ _ _ _ _ _ _ _ _ _ _ _ _ _ _ _ _ _ _ _ _ _ _ _ _ _ _ _ _ _ _ _ _] -> w301
          tunnel: [_ _ _ _ _ _ _ _ _ _ _ _ _ _ _ _ _ _ _ _ _ _ _ _ _ _ _ _ _ _ _ _ _ _ _ _ _ _ _ _ _ _ _ _ _ _ _ _ _ _ _ _ _ _ w2737 _ _ _ _ _ w3022 _ _ _ _ _ _ _ _ _ _] -> w300
          tunnel: [_ _ _ _ _ _ _ _ _ _ _ _ _ _ _ _ _ _ _ _ _ _ _ _ _ _ _ _ _ _ _ _ _ _ _ _ _ _ _ _ _ _ _ _ _ _ _ _ _ _ _ _ _ _ w2736 _ _ _ _ _ w3022 _ _ _ _ _ _ _ _ _ _] -> w299
          tunnel: w297 -> [_ _ _ _ _ _ _ _ _ _ _ _ _ _ _ _ _ _ _ _ _ _ _ _ _ _ _ _ _ _ _ _ _ _ _ _ _ _ _ _ _ _ _ _ _ _ _ _ _ _ _ _ _ _ _ _ _ _ _ _ _ _ _ _ _ _ _ _ _ _ _]
          tunnel: w296 -> [_ _ _ _ _ _ _ _ _ _ _ _ _ _ _ _ _ _ _ _ _ _ _ _ _ _ _ _ _ _ _ _ _ _ _ _ _ _ _ _ _ _ _ _ _ _ _ _ _ _ _ _ _ _ _ _ _ _ _ _ _ _ _ _ _ _ _ _ _ _ _]
          tunnel: w295 -> [_ _ _ _ _ _ _ _ _ _ _ _ _ _ _ _ _ _ _ _ _ _ _ _ _ _ _ _ _ _ _ _ _ _ _ _ _ _ _ _ _ _ _ _ _ _ _ _ _ _ _ _ _ _ _ _ _ _ _ _ _ _ _ _ _ _ _ _ _ _ _]
          tunnel: w294 -> [_ _ _ _ _ _ _ _ _ _ _ _ _ _ _ _ _ _ _ _ _ _ _ _ _ _ _ _ _ _ _ _ _ _ _ _ _ _ _ _ _ _ _ _ _ _ _ _ _ _ _ _ _ _ _ _ _ _ _ _ _ _ _ _ _ _ _ _ _ _ _]
          tunnel: w293 -> [_ _ _ _ _ _ _ _ _ _ _ _ _ _ _ _ _ _ _ _ _ _ _ _ _ _ _ _ _ _ _ _ _ _ _ _ _ _ _ _ _ _ _ _ _ _ _ _ _ _ _ _ _ _ _ _ _ _ _ _ _ _ _ _ _ _ _ _ _ _ _]
          tunnel: w292 -> [_ _ _ _ _ _ _ _ _ _ _ _ _ _ _ _ _ _ _ _ _ _ _ _ _ _ _ _ _ _ _ _ _ _ _ _ _ _ _ _ _ _ _ _ _ _ _ _ _ _ _ _ _ _ _ _ _ _ _ _ _ _ _ _ _ _ _ _ _ _ _]
          tunnel: w291 -> [_ _ _ _ _ _ _ _ _ _ _ _ _ _ _ _ _ _ _ _ _ _ _ _ _ _ _ _ _ _ _ _ _ _ _ _ _ _ _ _ _ _ _ _ _ _ _ _ _ _ _ _ _ _ _ _ w2829 _ w2926 _ _ _ _ w3165 _ w3259 _ _ _ _ _]
          tunnel: w290 -> [_ _ _ _ _ _ _ _ _ _ _ _ _ _ _ _ _ _ _ _ _ _ _ _ _ _ _ _ _ _ _ _ _ _ _ _ _ _ _ _ _ _ _ _ _ _ _ _ _ _ _ _ _ _ _ _ w2832 _ w2928 _ _ _ _ w3167 _ w3261 _ _ _ _ _]
          tunnel: [_ _ _ _ _ _ _ _ _ _ _ _ _ _ _ _ _ _ _ _ _ _ _ _ _ _ _ _ _ _ _ _ _ _ _ _ _ _ _ _ _ _ _ _ _ _ _ _ _ _ _ _ _ _ _ _ w2830 _ w2927 _ _ _ _ _ _ _ _ _ _ _ _] -> w289
          frame "None" {
            # ">>> Motor control cluster >>>"
            # ">>> yStepper command>>>"
          }
          frame "Startup" {
            # ">>> yStepper command>>>"
            n221 = for {
              shift-right: [w370] -> w364
              shift-left: w367 -> [w369]
              tunnel: string[] ["INIT", "RESET ARM", "RESET FLAGS", "RESET YAW", "NAVX CALIBRATE"] -> [w368] mode=indexing
              n222 = Enqueue Element(queue=w369, element=w368) -> (queue out=w370:refnum<queue>)  [unwired: 2 in, 2 out]
            }
            n223 = Bundle By Name(cluster=w362, "yStepper desired"=u8 0) -> (w361:T20)
            n224 = Bundle By Name(cluster=w359, "ySpeed"=0.0, "xSpeed"=0.0, "wSpeed"=0.0) -> (w358:T19)
          }
          frame "True Stop" {
            # ">>Action Queue>>"
            # ">>> Motor control cluster >>>"
            # ">>> yStepper command>>>"
            n225 = Flush Queue(queue=w377, error in (no error)=w376) -> ()  [unwired: 3 out]
            n226 = for {
              shift-right: [w383] -> w378
              shift-left: w379 -> [w382]
              tunnel: string[] ["STOP", "RESET ENCODERS", "RESET YAW", "RESET ARM", "RESET ALL SENSORS", "DISPOSE CAM BUFFERS", "DISPOSE PROC BUFFERS", "CAM CLOSE", ""] -> [w381] mode=indexing
              n227 = Enqueue Element(queue=w382, element=w381) -> (queue out=w383:refnum<queue>)  [unwired: 2 in, 2 out]
            }
          }
          frame "Idle", Default {
            # ">>> Motor control cluster >>>"
            # ">>> yStepper command>>>"
            n228 = Dequeue Element(queue=w395, timeout in ms (-1)=w394, error in (no error)=w390) -> (element=w393:T10)  [unwired: 3 out]
            n229 = case shown="\"Start Task A\"" w393 {
              tunnel: [w398 w406 w414 w422 w430 w438 w446 w454 w462 w469 w479 w487 w494 w497] -> w389
              tunnel: w392 -> [w399 w407 w415 w423 w431 w439 w447 w455 w463 w470 w478 w486 w494 w498]
              tunnel: [State_Type_Definitions,_for_0.26g_versions_and_later_3."Task 1A" ("Enum") State_Type_Definitions,_for_0.26g_versions_and_later_3."Task 2:Raise Arm" ("Enum") State_Type_Definitions,_for_0.26g_versions_and_later_3."Task 3" ("Enum") State_Type_Definitions,_for_0.26g_versions_and_later_3."Task 4_A" ("Enum") State_Type_Definitions,_for_0.26g_versions_and_later_3."Task 5A: RAISING ARM" ("Enum") State_Type_Definitions,_for_0.26g_versions_and_later_3."Task 6A: RAISE ARM" ("Enum") State_Type_Definitions,_for_0.26g_versions_and_later_3."Task 8A: RAISE ARM" ("Enum") State_Type_Definitions,_for_0.26g_versions_and_later_3."Task 8A: RAISE ARM" ("Enum") State_Type_Definitions,_for_0.26g_versions_and_later_3."Task 8A: RAISE ARM" ("Enum") State_Type_Definitions,_for_0.26g_versions_and_later_3."Task 8A: RAISE ARM" ("Enum") State_Type_Definitions,_for_0.26g_versions_and_later_3."Task 9A: Raise Arm" ("Enum") State_Type_Definitions,_for_0.26g_versions_and_later_3."Task A1: RAISE ARM" ("Enum") State_Type_Definitions,_for_0.26g_versions_and_later_3."Idle" ("Enum") State_Type_Definitions,_for_0.26g_versions_and_later_3."Shutdown" ("Enum")] -> w391
              tunnel: [enum16{"Ball", "Soap", "Gel", "Pipe", "None"}."None" ("Object recognition mode") enum16{"Ball", "Soap", "Gel", "Pipe", "None"}."None" ("Object recognition mode") enum16{"Ball", "Soap", "Gel", "Pipe", "None"}."None" ("Object recognition mode") enum16{"Ball", "Soap", "Gel", "Pipe", "None"}."None" ("Object recognition mode") enum16{"Ball", "Soap", "Gel", "Pipe", "None"}."None" ("Object recognition mode") enum16{"Ball", "Soap", "Gel", "Pipe", "None"}."None" ("Object recognition mode") enum16{"Ball", "Soap", "Gel", "Pipe", "None"}."Ball" ("Object recognition mode") enum16{"Ball", "Soap", "Gel", "Pipe", "None"}."Gel" ("Object recognition mode") enum16{"Ball", "Soap", "Gel", "Pipe", "None"}."Pipe" ("Object recognition mode") enum16{"Ball", "Soap", "Gel", "Pipe", "None"}."Soap" ("Object recognition mode") enum16{"Ball", "Soap", "Gel", "Pipe", "None"}."None" ("Object recognition mode") enum16{"Ball", "Soap", "Gel", "Pipe", "None"}."None" ("Object recognition mode") enum16{"Ball", "Soap", "Gel", "Pipe", "None"}."None" ("Object recognition mode") enum16{"Ball", "Soap", "Gel", "Pipe", "None"}."None" ("Object recognition mode")] -> w384
              frame "Start Task 1" {
                n230 = for {
                  shift-right: [w403] -> w398
                  shift-left: w399 -> [w402]
                  tunnel: string[] ["RESET ENCODERS", "RESET YAW", "FORWARD", "READ ENCODERS"] -> [w401] mode=indexing
                  n231 = Enqueue Element(queue=w402, element=w401) -> (queue out=w403:refnum<queue>)  [unwired: 2 in, 2 out]
                }
              }
              frame "Start Task 2" {
                n232 = for {
                  shift-right: [w411] -> w406
                  shift-left: w407 -> [w410]
                  tunnel: string[] ["RESET ENCODERS", "RESET YAW", "READ ULTRASONIC", "ARDUINO - ULTRASONIC"] -> [w409] mode=indexing
                  n233 = Enqueue Element(queue=w410, element=w409) -> (queue out=w411:refnum<queue>)  [unwired: 2 in, 2 out]
                }
              }
              frame "Start Task 3" {
                n234 = for {
                  shift-right: [w419] -> w414
                  shift-left: w415 -> [w418]
                  tunnel: string[] ["RESET ENCODERS", "READ ENCODERS", "R-ACW"] -> [w417] mode=indexing
                  n235 = Enqueue Element(queue=w418, element=w417) -> (queue out=w419:refnum<queue>)  [unwired: 2 in, 2 out]
                }
              }
              frame "Start Task 4" {
                n236 = for {
                  shift-right: [w427] -> w422
                  shift-left: w423 -> [w426]
                  tunnel: string[] ["RESET YAW", "RESET ENCODERS", "RESET ARM", "RESET FLAGS", "", ""] -> [w425] mode=indexing
                  n237 = Enqueue Element(queue=w426, element=w425) -> (queue out=w427:refnum<queue>)  [unwired: 2 in, 2 out]
                }
              }
              frame "Start Task 5" {
                n238 = for {
                  shift-right: [w435] -> w430
                  shift-left: w431 -> [w434]
                  tunnel: string[] ["RESET YAW", "RESET ENCODERS", "RESET ARM", "RESET ALL SENSORS", "", ""] -> [w433] mode=indexing
                  n239 = Enqueue Element(queue=w434, element=w433) -> (queue out=w435:refnum<queue>)  [unwired: 2 in, 2 out]
                }
              }
              frame "Start Task 6" {
                n240 = for {
                  shift-right: [w443] -> w438
                  shift-left: w439 -> [w442]
                  tunnel: string[] ["OPEN LOG CAM ", "", "", "", "", ""] -> [w441] mode=indexing
                  n241 = Enqueue Element(queue=w442, element=w441) -> (queue out=w443:refnum<queue>)  [unwired: 2 in, 2 out]
                }
              }
              frame "Start Task 8 - BALL" {
                n242 = for {
                  shift-right: [w451] -> w446
                  shift-left: w447 -> [w450]
                  tunnel: string[] ["RESET YAW", "RESET ENCODERS", "RESET ARM", "RESET FLAGS"] -> [w449] mode=indexing
                  n243 = Enqueue Element(queue=w450, element=w449) -> (queue out=w451:refnum<queue>)  [unwired: 2 in, 2 out]
                }
              }
              frame "Start Task 8 - Gel" {
                n244 = for {
                  shift-right: [w459] -> w454
                  shift-left: w455 -> [w458]
                  tunnel: string[] ["RESET YAW", "RESET ENCODERS", "RESET ARM", "RESET FLAGS"] -> [w457] mode=indexing
                  n245 = Enqueue Element(queue=w458, element=w457) -> (queue out=w459:refnum<queue>)  [unwired: 2 in, 2 out]
                }
              }
              frame "Start Task 8 - Pipe" {
                n246 = for {
                  shift-right: [w467] -> w462
                  shift-left: w463 -> [w466]
                  tunnel: string[] ["RESET YAW", "RESET ENCODERS", "RESET ARM", "RESET FLAGS"] -> [w465] mode=indexing
                  n247 = Enqueue Element(queue=w466, element=w465) -> (queue out=w467:refnum<queue>)  [unwired: 2 in, 2 out]
                }
              }
              frame "Start Task 8 - Soap" {
                n248 = for {
                  shift-right: [w475] -> w469
                  shift-left: w470 -> [w474]
                  tunnel: string[] ["RESET YAW", "RESET ENCODERS", "RESET ARM", "RESET FLAGS"] -> [w473] mode=indexing
                  n249 = Enqueue Element(queue=w474, element=w473) -> (queue out=w475:refnum<queue>)  [unwired: 2 in, 2 out]
                }
              }
              frame "Start Task 9" {
                n250 = for {
                  shift-right: [w483] -> w479
                  shift-left: w478 -> [w482]
                  tunnel: string[] ["Z STEPPER BOX HEIGHT", "READ STEPPER VALUES", "", ""] -> [w481] mode=indexing
                  n251 = Enqueue Element(queue=w482, element=w481) -> (queue out=w483:refnum<queue>)  [unwired: 2 in, 2 out]
                }
              }
              frame "Start Task A" {
                n252 = for {
                  shift-right: [w491] -> w487
                  shift-left: w486 -> [w490]
                  tunnel: string[] ["Z STEPPER BOX HEIGHT", "READ STEPPER VALUES", "", ""] -> [w489] mode=indexing
                  n253 = Enqueue Element(queue=w490, element=w489) -> (queue out=w491:refnum<queue>)  [unwired: 2 in, 2 out]
                }
              }
              frame "None", Default {
              }
              frame "Exit" {
                n254 = for {
                  shift-right: [w502] -> w497
                  shift-left: w498 -> [w501]
                  tunnel: string[] ["STOP", "RESET ENCODERS", "RESET YAW", "EXIT"] -> [w500] mode=indexing
                  n255 = Enqueue Element(queue=w501, element=w500) -> (queue out=w502:refnum<queue>)  [unwired: 2 in, 2 out]
                }
              }
            }
          }
          frame "Shutdown" {
            # ">> Item Selection Bias >>"
            # ">>> yStepper command>>>"
            n256 = for {
              shift-right: [w513] -> w507
              shift-left: w509 -> [w512]
              tunnel: string[] ["INIT", "RESET ENCODERS", "RESET FLAGS", "CAM CLOSE", "DISPOSE BUFFERS", "EXIT", ""] -> [w511] mode=indexing
              n257 = Enqueue Element(queue=w512, element=w511) -> (queue out=w513:refnum<queue>)  [unwired: 2 in, 2 out]
            }
          }
          frame "Task 1A" {
            # ">>> Motor control cluster >>>"
            # ">> Line detection >>"
            # ">> Checks if 1 metre moved >>"
            # ">>> yStepper command>>>"
            # "Use 250"
            n258 = Greater?(x=w523, y=265.0) -> (0:w517:bool)
            n259 = Dequeue Element(queue=w530, timeout in ms (-1)=w529, error in (no error)=w528) -> (element=w527:T10)  [unwired: 3 out]
            n260 = And(x=w516, y=w517) -> (x .and. y?=w514:bool)
            n261 = case shown="\"Start Task 1\", Default" w527 {
              tunnel: w515 -> [w531 _]
              tunnel: [w541 State_Type_Definitions,_for_0.26g_versions_and_later_3."True Stop" ("Enum")] -> w526
              tunnel: w525 -> [w539 w556]
              tunnel: [w538 w555] -> w524
              tunnel: [State_Type_Definitions,_for_0.26g_versions_and_later_3."Idle" ("Enum") State_Type_Definitions,_for_0.26g_versions_and_later_3."Shutdown" ("Enum")] -> w521
              tunnel: w514 -> [w532 _]
              frame "Start Task 1", Default {
                n262 = Or(x=w532, y=w531) -> (x .or. y?=w533:bool)
                n263 = case shown="True" w533 {
                  tunnel: w539 -> [w544 w550]
                  tunnel: [w543 w548] -> w538
                  frame False {
                    n264 = for {
                      shift-right: [w546] -> w543
                      shift-left: w544 -> [w547]
                      tunnel: string[] ["READ ENCODERS", "READ NAVX", "FORWARD", "READ LINE SENSOR"] ("element") -> [w545] mode=indexing
                      n265 = Enqueue Element(queue=w547, element=w545) -> (queue out=w546:refnum<queue>)  [unwired: 2 in, 2 out]
                    }
                  }
                  frame True {
                    n266 = for {
                      shift-right: [w552] -> w548
                      shift-left: w550 -> [w553]
                      tunnel: string[] ["RESET YAW", "RESET ENCODERS", "STOP", ""] -> [w551] mode=indexing
                      n267 = Enqueue Element(queue=w553, element=w551) -> (queue out=w552:refnum<queue>)  [unwired: 2 in, 2 out]
                    }
                  }
                }
                n268 = Select(t=State_Type_Definitions,_for_0.26g_versions_and_later_3."True Stop" ("Enum"), s=w531, f=State_Type_Definitions,_for_0.26g_versions_and_later_3."Task 1B" ("Enum")) -> (s? t:f=w536:T18)
                n269 = Select(t=w536, s=w532, f=State_Type_Definitions,_for_0.26g_versions_and_later_3."Task 1A" ("Enum")) -> (s? t:f=w541:T18)
              }
              frame "Exit" {
                n270 = for {
                  shift-right: [w560] -> w555
                  shift-left: w556 -> [w561]
                  tunnel: string[] ["STOP", "RESET ENCODERS", "RESET YAW", ""] -> [w559] mode=indexing
                  n271 = Enqueue Element(queue=w561, element=w559) -> (queue out=w560:refnum<queue>)  [unwired: 2 in, 2 out]
                }
              }
            }
          }
          frame "Task 1B" {
            # ">>> Motor control cluster >>>"
            # ">> Line detection >>"
            # ">> Adds small distance overhead after 1M >>"
            # ">>> yStepper command>>>"
            n272 = Greater?(x=w568, y=50.0) -> (0:w562:bool)
            n273 = Dequeue Element(queue=w577, timeout in ms (-1)=w576, error in (no error)=w575) -> (element=w574:T10)  [unwired: 3 out]
            n274 = Or(x=w562, y=w569) -> (x .or. y?=w573:bool)
            n275 = case shown="\"Start Task 1\", Default" w574 {
              tunnel: w573 -> [w580 _]
              tunnel: [w584 State_Type_Definitions,_for_0.26g_versions_and_later_3."True Stop" ("Enum")] -> w572
              tunnel: w571 -> [w581 w599]
              tunnel: [w579 w598] -> w570
              tunnel: [State_Type_Definitions,_for_0.26g_versions_and_later_3."Idle" ("Enum") State_Type_Definitions,_for_0.26g_versions_and_later_3."Shutdown" ("Enum")] -> w566
              frame "Start Task 1", Default {
                n276 = case shown="True" w580 {
                  tunnel: w581 -> [w587 w593]
                  tunnel: [w586 w591] -> w579
                  frame False {
                    n277 = for {
                      shift-right: [w589] -> w586
                      shift-left: w587 -> [w590]
                      tunnel: string[] ["READ ENCODERS", "READ NAVX", "FORWARD", "READ LINE SENSOR"] ("element") -> [w588] mode=indexing
                      n278 = Enqueue Element(queue=w590, element=w588) -> (queue out=w589:refnum<queue>)  [unwired: 2 in, 2 out]
                    }
                  }
                  frame True {
                    n279 = for {
                      shift-right: [w595] -> w591
                      shift-left: w593 -> [w596]
                      tunnel: string[] ["RESET YAW", "RESET ENCODERS", "STOP", ""] -> [w594] mode=indexing
                      n280 = Enqueue Element(queue=w596, element=w594) -> (queue out=w595:refnum<queue>)  [unwired: 2 in, 2 out]
                    }
                  }
                }
                n281 = Select(t=State_Type_Definitions,_for_0.26g_versions_and_later_3."True Stop" ("Enum"), s=w580, f=State_Type_Definitions,_for_0.26g_versions_and_later_3."Task 1B" ("Enum")) -> (s? t:f=w584:T18)
              }
              frame "Exit" {
                n282 = for {
                  shift-right: [w603] -> w598
                  shift-left: w599 -> [w604]
                  tunnel: string[] ["STOP", "RESET ENCODERS", "RESET YAW", ""] -> [w602] mode=indexing
                  n283 = Enqueue Element(queue=w604, element=w602) -> (queue out=w603:refnum<queue>)  [unwired: 2 in, 2 out]
                }
              }
            }
          }
          frame "Task 2:Raise Arm" {
            # ">> Stepper height reeached >>"
            # ">>> yStepper command>>>"
            # ">> Manual override >>"
            n284 = Dequeue Element(queue=w611, timeout in ms (-1)=w610, error in (no error)=w609) -> (element=w619:T10)  [unwired: 3 out]
            n285 = Equal?(x=w613, y=u8 60) -> (x = y?=w605:bool)
            n286 = case shown="\"Start Task 1\", Default" w619 {
              tunnel: [w630 State_Type_Definitions,_for_0.26g_versions_and_later_3."True Stop" ("Enum")] -> w615
              tunnel: [w628 w645] -> w608
              tunnel: w617 -> [w627 _]
              tunnel: w616 -> [w621 _]
              tunnel: [State_Type_Definitions,_for_0.26g_versions_and_later_3."Idle" ("Enum") State_Type_Definitions,_for_0.26g_versions_and_later_3."Shutdown" ("Enum")] -> w614
              tunnel: w605 -> [w620 _]
              frame "Start Task 1", Default {
                # ">> WIill proceed to part ii if not manual override >>"
                # ">>If ENABLE or Trigger is set to true>>"
                n287 = Or(x=w620, y=w621) -> (x .or. y?=w622:bool)
                n288 = case shown="True" w620 {
                  tunnel: [w633 w639] -> w628
                  tunnel: w627 -> [w632 w638]
                  frame False {
                    n289 = for {
                      shift-right: [w635] -> w633
                      shift-left: w632 -> [w636]
                      tunnel: string[] ["Z STEPPER CAM HEIGHT", "READ STEPPER VALUES"] ("element") -> [w634] mode=indexing
                      n290 = Enqueue Element(queue=w636, element=w634) -> (queue out=w635:refnum<queue>)  [unwired: 2 in, 2 out]
                    }
                  }
                  frame True {
                    n291 = for {
                      shift-right: [w641] -> w639
                      shift-left: w638 -> [w642]
                      tunnel: string[] ["ARDUINO - ULTRASONIC", "READ ULTRASONIC", "", "", "", ""] -> [w640] mode=indexing
                      n292 = Enqueue Element(queue=w642, element=w640) -> (queue out=w641:refnum<queue>)  [unwired: 2 in, 2 out]
                    }
                  }
                }
                n293 = Select(t=State_Type_Definitions,_for_0.26g_versions_and_later_3."True Stop" ("Enum"), s=w621, f=State_Type_Definitions,_for_0.26g_versions_and_later_3."Task 2:Sensor Mode" ("Enum")) -> (s? t:f=w624:T18)
                n294 = Select(t=w624, s=w622, f=State_Type_Definitions,_for_0.26g_versions_and_later_3."Task 2:Raise Arm" ("Enum")) -> (s? t:f=w630:T18)
              }
              frame "Exit" {
                n295 = for {
                  shift-right: [w648] -> w645
                  shift-left: _ -> [w649]
                  tunnel: string[] ["STOP", "RESET ENCODERS", "RESET YAW", ""] -> [w647] mode=indexing
                  n296 = Enqueue Element(queue=w649, element=w647) -> (queue out=w648:refnum<queue>)  [unwired: 2 in, 2 out]
                }
              }
            }
          }
          frame "Task 2:Sensor Mode" {
            w666 = u8 20 ("y")
            # ">>> yStepper command>>>"
            # ">>Object detected>>"
            n297 = Dequeue Element(queue=w659, timeout in ms (-1)=w658, error in (no error)=w657) -> (element=w667:T10)  [unwired: 3 out]
            n298 = Less?(x=w655, y=w666) -> (x < y?=w665:bool)
            n299 = Less?(x=w654, y=w666) -> (x < y?=w664:bool)
            n300 = Or(x=w665, y=w664) -> (x .or. y?=w650:bool)
            n301 = case shown="\"Start Task 1\", Default" w667 {
              tunnel: w650 -> [w670 _]
              tunnel: [w677 State_Type_Definitions,_for_0.26g_versions_and_later_3."True Stop" ("Enum")] -> w663
              tunnel: w656 -> [w669 _]
              tunnel: w660 -> [w676 w693]
              tunnel: [w675 w694] -> w662
              tunnel: [State_Type_Definitions,_for_0.26g_versions_and_later_3."Idle" ("Enum") State_Type_Definitions,_for_0.26g_versions_and_later_3."Shutdown" ("Enum")] -> w661
              frame "Start Task 1", Default {
                n302 = case shown="False" w670 {
                  tunnel: w676 -> [w680 w687]
                  tunnel: [w681 w686] -> w675
                  frame False {
                    n303 = for {
                      tunnel: string[] ["READ ULTRASONIC", "STOP"] ("element") -> [w682] mode=indexing
                      shift-right: [w684] -> w681
                      shift-left: w680 -> [w683]
                      n304 = Enqueue Element(queue=w683, element=w682) -> (queue out=w684:refnum<queue>)  [unwired: 2 in, 2 out]
                    }
                  }
                  frame True {
                    n305 = for {
                      shift-right: [w689] -> w686
                      shift-left: w687 -> [w690]
                      tunnel: string[] ["RESET ENCODERS", "READ NAVX", "READ ENCODERS"] -> [w688] mode=indexing
                      n306 = Enqueue Element(queue=w690, element=w688) -> (queue out=w689:refnum<queue>)  [unwired: 2 in, 2 out]
                    }
                  }
                }
                n307 = Or(x=w670, y=w669) -> (x .or. y?=w668:bool)
                n308 = Select(t=State_Type_Definitions,_for_0.26g_versions_and_later_3."True Stop" ("Enum"), s=w669, f=State_Type_Definitions,_for_0.26g_versions_and_later_3."Task 2:Reverse Mode" ("Enum")) -> (s? t:f=w671:T18)
                n309 = Select(t=w671, s=w668, f=State_Type_Definitions,_for_0.26g_versions_and_later_3."Task 2:Sensor Mode" ("Enum")) -> (s? t:f=w677:T18)
              }
              frame "Exit" {
                n310 = for {
                  shift-right: [w697] -> w694
                  shift-left: w693 -> [w698]
                  tunnel: string[] ["STOP", "RESET ENCODERS", "RESET YAW", "ARDUINO MODE 0"] -> [w696] mode=indexing
                  n311 = Enqueue Element(queue=w698, element=w696) -> (queue out=w697:refnum<queue>)  [unwired: 2 in, 2 out]
                }
              }
            }
          }
          frame "Task 2:Reverse Mode" {
            # ">>> yStepper command>>>"
            n312 = Dequeue Element(queue=w709, timeout in ms (-1)=w710, error in (no error)=w711) -> (element=w713:T10)  [unwired: 3 out]
            n313 = Less?(x=w703, y=-30.0) -> (x < y?=w699:bool)
            n314 = case shown="\"Start Task 1\", Default" w713 {
              tunnel: [w723 State_Type_Definitions,_for_0.26g_versions_and_later_3."True Stop" ("Enum")] -> w705
              tunnel: w712 -> [w716 _]
              tunnel: w708 -> [w722 w739]
              tunnel: [w721 w740] -> w704
              tunnel: [State_Type_Definitions,_for_0.26g_versions_and_later_3."Idle" ("Enum") State_Type_Definitions,_for_0.26g_versions_and_later_3."Shutdown" ("Enum")] -> w706
              tunnel: w699 -> [w714 _]
              frame "Start Task 1", Default {
                n315 = case shown="True" w714 {
                  tunnel: w722 -> [w726 w733]
                  tunnel: [w727 w732] -> w721
                  frame False {
                    n316 = for {
                      tunnel: string[] ["READ ENCODERS", "REVERSE", "READ NAVX"] ("element") -> [w728] mode=indexing
                      shift-right: [w730] -> w727
                      shift-left: w726 -> [w729]
                      n317 = Enqueue Element(queue=w729, element=w728) -> (queue out=w730:refnum<queue>)  [unwired: 2 in, 2 out]
                    }
                  }
                  frame True {
                    n318 = for {
                      shift-right: [w735] -> w732
                      shift-left: w733 -> [w736]
                      tunnel: string[] ["STOP", "ARDUINO - ULTRASONIC", "READ ULTRASONIC", "RESET ENCODERS"] -> [w734] mode=indexing
                      n319 = Enqueue Element(queue=w736, element=w734) -> (queue out=w735:refnum<queue>)  [unwired: 2 in, 2 out]
                    }
                  }
                }
                n320 = Or(x=w714, y=w716) -> (x .or. y?=w715:bool)
                n321 = Select(t=State_Type_Definitions,_for_0.26g_versions_and_later_3."True Stop" ("Enum"), s=w716, f=State_Type_Definitions,_for_0.26g_versions_and_later_3."Task 2:Sensor Mode" ("Enum")) -> (s? t:f=w717:T18)
                n322 = Select(t=w717, s=w715, f=State_Type_Definitions,_for_0.26g_versions_and_later_3."Task 2:Reverse Mode" ("Enum")) -> (s? t:f=w723:T18)
              }
              frame "Exit" {
                n323 = for {
                  shift-right: [w743] -> w740
                  shift-left: w739 -> [w744]
                  tunnel: string[] ["STOP", "RESET ENCODERS", "RESET YAW", "ARDUINO MODE 0"] -> [w742] mode=indexing
                  n324 = Enqueue Element(queue=w744, element=w742) -> (queue out=w743:refnum<queue>)  [unwired: 2 in, 2 out]
                }
              }
            }
          }
          frame "Task 3" {
            # ">>> Motor control cluster >>>"
            # ">>> yStepper command>>>"
            n325 = Dequeue Element(queue=w760, timeout in ms (-1)=w759, error in (no error)=w758) -> (element=w750:T10)  [unwired: 3 out]
            n326 = Less?(x=w757, y=-160.0) -> (x < y?=w745:bool)
            n327 = Or(x=w745, y=w755) -> (x .or. y?=w751:bool)
            n328 = case shown="\"Start Task 1\", Default" w750 {
              tunnel: w751 -> [w763 _]
              tunnel: [w767 State_Type_Definitions,_for_0.26g_versions_and_later_3."True Stop" ("Enum")] -> w752
              tunnel: w754 -> [w764 w783]
              tunnel: [w762 w782] -> w753
              tunnel: [State_Type_Definitions,_for_0.26g_versions_and_later_3."Idle" ("Enum") State_Type_Definitions,_for_0.26g_versions_and_later_3."Shutdown" ("Enum")] -> w749
              frame "Start Task 1", Default {
                n329 = case shown="False" w763 {
                  tunnel: w764 -> [w770 w776]
                  tunnel: [w769 w774] -> w762
                  frame False {
                    n330 = for {
                      shift-right: [w772] -> w769
                      shift-left: w770 -> [w773]
                      tunnel: string[] ["READ ENCODERS", "R-CW"] ("element") -> [w771] mode=indexing
                      n331 = Enqueue Element(queue=w773, element=w771) -> (queue out=w772:refnum<queue>)  [unwired: 2 in, 2 out]
                    }
                  }
                  frame True {
                    n332 = for {
                      shift-right: [w778] -> w774
                      shift-left: w776 -> [w779]
                      tunnel: string[] ["RESET YAW", "RESET ENCODERS", "STOP", "ARDUINO MODE 0"] -> [w777] mode=indexing
                      n333 = Enqueue Element(queue=w779, element=w777) -> (queue out=w778:refnum<queue>)  [unwired: 2 in, 2 out]
                    }
                  }
                }
                n334 = Select(t=State_Type_Definitions,_for_0.26g_versions_and_later_3."True Stop" ("Enum"), s=w763, f=State_Type_Definitions,_for_0.26g_versions_and_later_3."Task 3" ("Enum")) -> (s? t:f=w767:T18)
              }
              frame "Exit" {
                n335 = for {
                  shift-right: [w786] -> w782
                  shift-left: w783 -> [w787]
                  tunnel: string[] ["STOP", "RESET ENCODERS", "RESET YAW", ""] -> [w785] mode=indexing
                  n336 = Enqueue Element(queue=w787, element=w785) -> (queue out=w786:refnum<queue>)  [unwired: 2 in, 2 out]
                }
              }
            }
          }
          frame "Task 4_A" {
            # ">> Stepper height reeached >>"
            # ">>> yStepper command>>>"
            # ">> Manual override >>"
            n337 = Dequeue Element(queue=w801, timeout in ms (-1)=w800, error in (no error)=w799) -> (element=w798:T10)  [unwired: 3 out]
            n338 = Equal?(x=w792, y=u8 60) -> (x = y?=w788:bool)
            n339 = case shown="\"Start Task 1\", Default" w798 {
              tunnel: [w813 State_Type_Definitions,_for_0.26g_versions_and_later_3."True Stop" ("Enum")] -> w797
              tunnel: [w811 w829] -> w796
              tunnel: w802 -> [w810 w826]
              tunnel: w795 -> [w804 _]
              tunnel: [State_Type_Definitions,_for_0.26g_versions_and_later_3."Idle" ("Enum") State_Type_Definitions,_for_0.26g_versions_and_later_3."Shutdown" ("Enum")] -> w794
              tunnel: w788 -> [w803 _]
              frame "Start Task 1", Default {
                # ">> WIill proceed to part ii if not manual override >>"
                # ">>If ENABLE or Trigger is set to true>>"
                n340 = Or(x=w803, y=w804) -> (x .or. y?=w805:bool)
                n341 = case shown="False" w803 {
                  tunnel: [w816 w822] -> w811
                  tunnel: w810 -> [w815 w821]
                  frame False {
                    n342 = for {
                      shift-right: [w818] -> w816
                      shift-left: w815 -> [w819]
                      tunnel: string[] ["Z STEPPER CAM HEIGHT", "READ STEPPER VALUES"] ("element") -> [w817] mode=indexing
                      n343 = Enqueue Element(queue=w819, element=w817) -> (queue out=w818:refnum<queue>)  [unwired: 2 in, 2 out]
                    }
                  }
                  frame True {
                    n344 = for {
                      shift-right: [w824] -> w822
                      shift-left: w821 -> [w825]
                      tunnel: string[] ["ARDUINO - ULTRASONIC", "READ ULTRASONIC", "FORWARD", "", "", ""] -> [w823] mode=indexing
                      n345 = Enqueue Element(queue=w825, element=w823) -> (queue out=w824:refnum<queue>)  [unwired: 2 in, 2 out]
                    }
                  }
                }
                n346 = Select(t=State_Type_Definitions,_for_0.26g_versions_and_later_3."True Stop" ("Enum"), s=w804, f=State_Type_Definitions,_for_0.26g_versions_and_later_3."Task 4_B" ("Enum")) -> (s? t:f=w807:T18)
                n347 = Select(t=w807, s=w805, f=State_Type_Definitions,_for_0.26g_versions_and_later_3."Task 4_A" ("Enum")) -> (s? t:f=w813:T18)
              }
              frame "Exit" {
                n348 = for {
                  shift-right: [w832] -> w829
                  shift-left: w826 -> [w833]
                  tunnel: string[] ["STOP", "RESET ENCODERS", "RESET YAW", ""] -> [w831] mode=indexing
                  n349 = Enqueue Element(queue=w833, element=w831) -> (queue out=w832:refnum<queue>)  [unwired: 2 in, 2 out]
                }
              }
            }
          }
          frame "Task 4_B" {
            w839 = u8 20
            # ">> Path blocked >>"
            # ">>> yStepper command>>>"
            # ">> Manual override >>"
            n350 = Dequeue Element(queue=w848, timeout in ms (-1)=w847, error in (no error)=w846) -> (element=w845:T10)  [unwired: 3 out]
            n351 = Less?(x=w841, y=w839) -> (x < y?=w836:bool)
            n352 = Less?(x=w840, y=w839) -> (x < y?=w837:bool)
            n353 = And(x=w837, y=w836) -> (x .and. y?=w838:bool)
            n354 = case shown="\"Start Task 1\", Default" w845 {
              tunnel: [w862 State_Type_Definitions,_for_0.26g_versions_and_later_3."True Stop" ("Enum")] -> w850
              tunnel: [w860 w877] -> w851
              tunnel: w844 -> [w859 _]
              tunnel: w849 -> [w853 _]
              tunnel: [State_Type_Definitions,_for_0.26g_versions_and_later_3."Idle" ("Enum") State_Type_Definitions,_for_0.26g_versions_and_later_3."Shutdown" ("Enum")] -> w843
              tunnel: w838 -> [w852 _]
              frame "Start Task 1", Default {
                # ">> Manual override forces program to true stop >>"
                # ">>If ENABLE or Trigger is set to true>>"
                n355 = Or(x=w852, y=w853) -> (x .or. y?=w858:bool)
                n356 = case shown="False" w852 {
                  tunnel: [w865 w870] -> w860
                  tunnel: w859 -> [w864 w869]
                  frame False {
                    n357 = for {
                      shift-right: [w867] -> w865
                      shift-left: w864 -> [w868]
                      tunnel: string[] ["FORWARD", "READ ULTRASONIC", "READ NAVX"] ("element") -> [w866] mode=indexing
                      n358 = Enqueue Element(queue=w868, element=w866) -> (queue out=w867:refnum<queue>)  [unwired: 2 in, 2 out]
                    }
                  }
                  frame True {
                    n359 = for {
                      shift-right: [w873] -> w870
                      shift-left: w869 -> [w874]
                      tunnel: string[] ["STOP", "RESET YAW", "RESET ENCODERS", "RESET FLAGS"] -> [w872] mode=indexing
                      n360 = Enqueue Element(queue=w874, element=w872) -> (queue out=w873:refnum<queue>)  [unwired: 2 in, 2 out]
                    }
                  }
                }
                n361 = Select(t=State_Type_Definitions,_for_0.26g_versions_and_later_3."True Stop" ("Enum"), s=w853, f=State_Type_Definitions,_for_0.26g_versions_and_later_3."Task 4_C" ("Enum")) -> (s? t:f=w855:T18)
                n362 = Select(t=w855, s=w858, f=State_Type_Definitions,_for_0.26g_versions_and_later_3."Task 4_B" ("Enum")) -> (s? t:f=w862:T18)
              }
              frame "Exit" {
                n363 = for {
                  shift-right: [w880] -> w877
                  shift-left: _ -> [w881]
                  tunnel: string[] ["STOP", "RESET ENCODERS", "RESET YAW", ""] -> [w879] mode=indexing
                  n364 = Enqueue Element(queue=w881, element=w879) -> (queue out=w880:refnum<queue>)  [unwired: 2 in, 2 out]
                }
              }
            }
          }
          frame "Task 4_C" {
            w893 = u8 20
            # ">> xDistance travelled>>"
            # ">> Path NOT blocked >>"
            # ">>> yStepper command>>>"
            # ">> Manual override >>"
            n365 = Dequeue Element(queue=w903, timeout in ms (-1)=w896, error in (no error)=w895) -> (element=w897:T10)  [unwired: 3 out]
            n366 = Greater?(x=w885, y=w893) -> (0:w891:bool)
            n367 = Greater?(x=w890, y=80.0) -> (0:w888:bool)
            n368 = Greater?(x=w884, y=w893) -> (0:w892:bool)
            n369 = And(x=w892, y=w891) -> (x .and. y?=w887:bool)
            n370 = And(x=w888, y=w887) -> (x .and. y?=w886:bool)
            n371 = case shown="\"Start Task 1\", Default" w897 {
              tunnel: [w914 State_Type_Definitions,_for_0.26g_versions_and_later_3."True Stop" ("Enum")] -> w900
              tunnel: [w912 w930] -> w899
              tunnel: w902 -> [w911 w927]
              tunnel: w901 -> [w905 _]
              tunnel: [State_Type_Definitions,_for_0.26g_versions_and_later_3."Idle" ("t") State_Type_Definitions,_for_0.26g_versions_and_later_3."Shutdown" ("Enum")] -> w898
              tunnel: w886 -> [w904 _]
              frame "Start Task 1", Default {
                # ">> Manual override forces program to true stop >>"
                # ">>If ENABLE or Trigger is set to true>>"
                n372 = Or(x=w904, y=w905) -> (x .or. y?=w910:bool)
                n373 = case shown="False" w904 {
                  tunnel: [w917 w922] -> w912
                  tunnel: w911 -> [w915 w921]
                  frame False {
                    n374 = for {
                      shift-right: [w919] -> w917
                      shift-left: w915 -> [w920]
                      tunnel: string[] ["RIGHT", "READ NAVX", "READ ENCODERS", "READ ULTRASONIC"] ("element") -> [w918] mode=indexing
                      n375 = Enqueue Element(queue=w920, element=w918) -> (queue out=w919:refnum<queue>)  [unwired: 2 in, 2 out]
                    }
                  }
                  frame True {
                    n376 = for {
                      shift-right: [w925] -> w922
                      shift-left: w921 -> [w926]
                      tunnel: string[] ["STOP", "RESET YAW", "RESET ENCODERS", "ARDUINO - ULTRASONIC"] -> [w924] mode=indexing
                      n377 = Enqueue Element(queue=w926, element=w924) -> (queue out=w925:refnum<queue>)  [unwired: 2 in, 2 out]
                    }
                  }
                }
                n378 = Select(t=State_Type_Definitions,_for_0.26g_versions_and_later_3."True Stop" ("Enum"), s=w905, f=State_Type_Definitions,_for_0.26g_versions_and_later_3."Task 4_D" ("Enum")) -> (s? t:f=w906:T18)
                n379 = Select(t=w906, s=w910, f=State_Type_Definitions,_for_0.26g_versions_and_later_3."Task 4_C" ("Enum")) -> (s? t:f=w914:T18)
              }
              frame "Exit" {
                n380 = for {
                  shift-right: [w933] -> w930
                  shift-left: w927 -> [w934]
                  tunnel: string[] ["STOP", "RESET ENCODERS", "RESET YAW", ""] -> [w932] mode=indexing
                  n381 = Enqueue Element(queue=w934, element=w932) -> (queue out=w933:refnum<queue>)  [unwired: 2 in, 2 out]
                }
              }
            }
          }
          frame "Task 4_D" {
            w957 = u8 20
            # ">>> Motor control cluster >>>"
            # ">> Line detected >>"
            # ">> yDistance travelled>>"
            # ">> Path blocked >>"
            # ">>> yStepper command>>>"
            # ">> Manual override >>"
            n382 = Less?(x=w942, y=w957) -> (x < y?=w955:bool)
            n383 = Greater?(x=w946, y=200.0) -> (0:w953:bool)
            n384 = Less?(x=w941, y=w957) -> (x < y?=w956:bool)
            n385 = And(x=w956, y=w955) -> (x .and. y?=w952:bool)
            n386 = Dequeue Element(queue=w949, timeout in ms (-1)=w948, error in (no error)=w947) -> (element=w958:T10)  [unwired: 3 out]
            n387 = Or(x=w953, y=w952) -> (x .or. y?=w936:bool)
            n388 = And(x=w937, y=w936) -> (x .and. y?=w935:bool)
            n389 = case shown="\"Start Task 1\", Default" w958 {
              tunnel: [w969 State_Type_Definitions,_for_0.26g_versions_and_later_3."True Stop" ("Enum")] -> w945
              tunnel: [w967 w985] -> w943
              tunnel: w950 -> [w966 w982]
              tunnel: w951 -> [w960 _]
              tunnel: [State_Type_Definitions,_for_0.26g_versions_and_later_3."Idle" ("t") State_Type_Definitions,_for_0.26g_versions_and_later_3."Shutdown" ("Enum")] -> w944
              tunnel: w935 -> [w959 _]
              frame "Start Task 1", Default {
                # ">> Manual override forces program to true stop >>"
                # ">>If ENABLE or Trigger is set to true>>"
                n390 = Or(x=w959, y=w960) -> (x .or. y?=w965:bool)
                n391 = case shown="False" w959 {
                  tunnel: [w972 w977] -> w967
                  tunnel: w966 -> [w970 w976]
                  frame False {
                    n392 = for {
                      shift-right: [w974] -> w972
                      shift-left: w970 -> [w975]
                      tunnel: string[] ["FORWARD", "READ NAVX", "READ ENCODERS", "READ ULTRASONIC", "READ LINE SENSOR"] ("element") -> [w973] mode=indexing
                      n393 = Enqueue Element(queue=w975, element=w973) -> (queue out=w974:refnum<queue>)  [unwired: 2 in, 2 out]
                    }
                  }
                  frame True {
                    n394 = for {
                      shift-right: [w980] -> w977
                      shift-left: w976 -> [w981]
                      tunnel: string[] ["STOP", "RESET YAW", "RESET ENCODERS", "RESET FLAGS"] -> [w979] mode=indexing
                      n395 = Enqueue Element(queue=w981, element=w979) -> (queue out=w980:refnum<queue>)  [unwired: 2 in, 2 out]
                    }
                  }
                }
                n396 = Select(t=State_Type_Definitions,_for_0.26g_versions_and_later_3."True Stop" ("Enum"), s=w960, f=State_Type_Definitions,_for_0.26g_versions_and_later_3."True Stop" ("Enum")) -> (s? t:f=w961:T18)
                n397 = Select(t=w961, s=w965, f=State_Type_Definitions,_for_0.26g_versions_and_later_3."Task 4_D" ("Enum")) -> (s? t:f=w969:T18)
              }
              frame "Exit" {
                n398 = for {
                  shift-right: [w988] -> w985
                  shift-left: w982 -> [w989]
                  tunnel: string[] ["STOP", "RESET ENCODERS", "RESET YAW", ""] -> [w987] mode=indexing
                  n399 = Enqueue Element(queue=w989, element=w987) -> (queue out=w988:refnum<queue>)  [unwired: 2 in, 2 out]
                }
              }
            }
          }
          frame "Task 5A: RAISING ARM" {
            # "Stays in Task 5_A until stepper reaches desired \nheight"
            # ">>> Motor control cluster >>>"
            # ">>> yStepper command>>>"
            # ">> Manual override >>"
            n400 = Dequeue Element(queue=w1000, timeout in ms (-1)=w999, error in (no error)=w1001) -> (element=w998:T10)  [unwired: 3 out]
            n401 = Equal?(x=w997, y=u8 60) -> (x = y?=w995:bool)
            n402 = case shown="\"Start Task 1\", Default" w998 {
              tunnel: [w1011 State_Type_Definitions,_for_0.26g_versions_and_later_3."True Stop" ("Enum")] -> w1002
              tunnel: [w1014 w1031] -> w1003
              tunnel: [State_Type_Definitions,_for_0.26g_versions_and_later_3."Idle" ("Enum") State_Type_Definitions,_for_0.26g_versions_and_later_3."Shutdown" ("Enum")] -> w1004
              tunnel: w995 -> [w1010 _]
              tunnel: w994 -> [w1009 _]
              tunnel: w993 -> [w1005 w1028]
              frame "Start Task 1", Default {
                # "T: Go back to idle, F: Continue with task\""
                # ">> Manual override >>"
                n403 = case shown="True" w1010 {
                  tunnel: [w1018 w1024] -> w1014
                  tunnel: w1005 -> [w1016 w1022]
                  frame False {
                    n404 = for {
                      tunnel: string[] ["Z STEPPER GRAB HEIGHT", "READ STEPPER VALUES"] ("element") -> [w1019] mode=indexing
                      shift-right: [w1021] -> w1018
                      shift-left: w1016 -> [w1020]
                      n405 = Enqueue Element(queue=w1020, element=w1019) -> (queue out=w1021:refnum<queue>)  [unwired: 2 in, 2 out]
                    }
                  }
                  frame True {
                    n406 = for {
                      shift-right: [w1026] -> w1024
                      shift-left: w1022 -> [w1027]
                      tunnel: string[] ["", "", ""] -> [w1025] mode=indexing
                      n407 = Enqueue Element(queue=w1027, element=w1025) -> (queue out=w1026:refnum<queue>)  [unwired: 2 in, 2 out]
                    }
                  }
                }
                n408 = Or(x=w1010, y=w1009) -> (x .or. y?=w1012:bool)
                n409 = Select(t=State_Type_Definitions,_for_0.26g_versions_and_later_3."True Stop" ("Enum"), s=w1009, f=State_Type_Definitions,_for_0.26g_versions_and_later_3."Task 5B: STILL WAITING" ("Enum")) -> (s? t:f=w1006:T18)
                n410 = Select(t=w1006, s=w1012, f=State_Type_Definitions,_for_0.26g_versions_and_later_3."Task 5A: RAISING ARM" ("Enum")) -> (s? t:f=w1011:T18)
              }
              frame "Exit" {
                n411 = for {
                  shift-right: [w1034] -> w1031
                  shift-left: w1028 -> [w1035]
                  tunnel: string[] ["STOP", "RESET ENCODERS", "RESET YAW", "ARDUINO MODE 0"] -> [w1033] mode=indexing
                  n412 = Enqueue Element(queue=w1035, element=w1033) -> (queue out=w1034:refnum<queue>)  [unwired: 2 in, 2 out]
                }
              }
            }
          }
          frame "Task 5B: STILL WAITING" {
            # ">>> yStepper command>>>"
            n413 = Dequeue Element(queue=w1042, timeout in ms (-1)=w1041, error in (no error)=w1043) -> (element=w1040:T10)  [unwired: 3 out]
            n414 = local read "Rising Edge"() -> (w1036:bool)
            n415 = case shown="\"Start Task 1\", Default" w1040 {
              tunnel: [w1055 State_Type_Definitions,_for_0.26g_versions_and_later_3."True Stop" ("Enum")] -> w1045
              tunnel: [w1058 w1075] -> w1044
              tunnel: [State_Type_Definitions,_for_0.26g_versions_and_later_3."Idle" ("Enum") State_Type_Definitions,_for_0.26g_versions_and_later_3."Shutdown" ("Enum")] -> w1046
              tunnel: w1048 -> [w1054 _]
              tunnel: w1047 -> [w1050 w1072]
              tunnel: w1036 -> [w1049 _]
              frame "Start Task 1", Default {
                # "T: Go back to idle, F: Continue with task\""
                # ">> Manual override >>"
                n416 = case shown="True" w1049 {
                  tunnel: [w1062 w1068] -> w1058
                  tunnel: w1050 -> [w1060 w1066]
                  frame False {
                    n417 = for {
                      tunnel: string[] ["CLOSE CLAW", "START TIMER", ""] ("element") -> [w1063] mode=indexing
                      shift-right: [w1065] -> w1062
                      shift-left: w1060 -> [w1064]
                      n418 = Enqueue Element(queue=w1064, element=w1063) -> (queue out=w1065:refnum<queue>)  [unwired: 2 in, 2 out]
                    }
                  }
                  frame True {
                    n419 = for {
                      shift-right: [w1070] -> w1068
                      shift-left: w1066 -> [w1071]
                      tunnel: string[] ["STOP", "", "", ""] -> [w1069] mode=indexing
                      n420 = Enqueue Element(queue=w1071, element=w1069) -> (queue out=w1070:refnum<queue>)  [unwired: 2 in, 2 out]
                    }
                  }
                }
                n421 = Or(x=w1049, y=w1054) -> (x .or. y?=w1056:bool)
                n422 = Select(t=State_Type_Definitions,_for_0.26g_versions_and_later_3."True Stop" ("Enum"), s=w1054, f=State_Type_Definitions,_for_0.26g_versions_and_later_3."Task 5C: GOING DOWN" ("Enum")) -> (s? t:f=w1051:T18)
                n423 = Select(t=w1051, s=w1056, f=State_Type_Definitions,_for_0.26g_versions_and_later_3."Task 5B: STILL WAITING" ("Enum")) -> (s? t:f=w1055:T18)
              }
              frame "Exit" {
                n424 = for {
                  shift-right: [w1078] -> w1075
                  shift-left: w1072 -> [w1079]
                  tunnel: string[] ["STOP", "RESET ENCODERS", "RESET YAW", "ARDUINO MODE 0"] -> [w1077] mode=indexing
                  n425 = Enqueue Element(queue=w1079, element=w1077) -> (queue out=w1078:refnum<queue>)  [unwired: 2 in, 2 out]
                }
              }
            }
          }
          frame "Task 5C: GOING DOWN" {
            # ">>> Motor control cluster >>>"
            # ">>> yStepper command>>>"
            # ">> Manual override >>"
            n426 = Equal?(x=w1082, y=u8 1) -> (x = y?=w1080:bool)
            n427 = Dequeue Element(queue=w1092, timeout in ms (-1)=w1091, error in (no error)=w1090) -> (element=w1089:T10)  [unwired: 3 out]
            n428 = case shown="\"Start Task 1\", Default" w1089 {
              tunnel: [w1101 State_Type_Definitions,_for_0.26g_versions_and_later_3."True Stop" ("Enum")] -> w1094
              tunnel: [w1104 w1121] -> w1087
              tunnel: [State_Type_Definitions,_for_0.26g_versions_and_later_3."Idle" ("Enum") State_Type_Definitions,_for_0.26g_versions_and_later_3."Shutdown" ("Enum")] -> w1086
              tunnel: w1088 -> [w1095 _]
              tunnel: w1093 -> [w1100 w1118]
              tunnel: w1080 -> [w1099 _]
              frame "Start Task 1", Default {
                # ">> Is time up? >>"
                # "Determines if object is in range to pick up"
                # ">> Manual override >>"
                n429 = case shown="False" w1099 {
                  tunnel: [w1108 w1114] -> w1104
                  tunnel: w1100 -> [w1107 w1112]
                  frame False {
                    n430 = for {
                      tunnel: string[] ["Z STEPPER GRAB HEIGHT", "READ STEPPER VALUES", "", ""] -> [w1109] mode=indexing
                      shift-right: [w1111] -> w1108
                      shift-left: w1107 -> [w1110]
                      n431 = Enqueue Element(queue=w1110, element=w1109) -> (queue out=w1111:refnum<queue>)  [unwired: 2 in, 2 out]
                    }
                  }
                  frame True {
                    n432 = for {
                      shift-right: [w1116] -> w1114
                      shift-left: w1112 -> [w1117]
                      tunnel: string[] ["SET TIMER 5", "", ""] -> [w1115] mode=indexing
                      n433 = Enqueue Element(queue=w1117, element=w1115) -> (queue out=w1116:refnum<queue>)  [unwired: 2 in, 2 out]
                    }
                  }
                }
                n434 = Or(x=w1099, y=w1095) -> (x .or. y?=w1102:bool)
                n435 = Select(t=State_Type_Definitions,_for_0.26g_versions_and_later_3."True Stop" ("Enum"), s=w1095, f=State_Type_Definitions,_for_0.26g_versions_and_later_3."Task 5D: GRAB" ("Enum")) -> (s? t:f=w1097:T18)
                n436 = Select(t=w1097, s=w1102, f=State_Type_Definitions,_for_0.26g_versions_and_later_3."Task 5C: GOING DOWN" ("Enum")) -> (s? t:f=w1101:T18)
              }
              frame "Exit" {
                n437 = for {
                  shift-right: [w1124] -> w1121
                  shift-left: w1118 -> [w1125]
                  tunnel: string[] ["STOP", "RESET ENCODERS", "RESET YAW", "ARDUINO MODE 0"] -> [w1123] mode=indexing
                  n438 = Enqueue Element(queue=w1125, element=w1123) -> (queue out=w1124:refnum<queue>)  [unwired: 2 in, 2 out]
                }
              }
            }
          }
          frame "Task 5D: GRAB" {
            # ">>> Motor control cluster >>>"
            # ">>> yStepper command>>>"
            n439 = Dequeue Element(queue=w1133, timeout in ms (-1)=w1132, error in (no error)=w1131) -> (element=w1130:T10)  [unwired: 3 out]
            n440 = case shown="\"Start Task 1\", Default" w1130 {
              tunnel: [w1145 State_Type_Definitions,_for_0.26g_versions_and_later_3."True Stop" ("Enum")] -> w1137
              tunnel: [w1148 w1165] -> w1136
              tunnel: [State_Type_Definitions,_for_0.26g_versions_and_later_3."Idle" ("Enum") State_Type_Definitions,_for_0.26g_versions_and_later_3."Shutdown" ("Enum")] -> w1138
              tunnel: w1134 -> [w1144 _]
              tunnel: w1135 -> [w1140 w1162]
              tunnel: w1128 -> [w1139 _]
              frame "Start Task 1", Default {
                # ">> T: Breaks out of state loop; F: Stays in loop>>"
                # ">> Manual override >>"
                # ">> Checks if time is up>>"
                # "Stays in Task 5D until the object is detected"
                # "T: Go back to idle, F: Continue with task\""
                # ">> Manual override >>"
                n441 = case shown="False" w1139 {
                  tunnel: [w1152 w1158] -> w1148
                  tunnel: w1140 -> [w1150 w1156]
                  frame False {
                    n442 = for {
                      tunnel: string[] ["START TIMER", "OPEN CLAW", ""] ("element") -> [w1153] mode=indexing
                      shift-right: [w1155] -> w1152
                      shift-left: w1150 -> [w1154]
                      n443 = Enqueue Element(queue=w1154, element=w1153) -> (queue out=w1155:refnum<queue>)  [unwired: 2 in, 2 out]
                    }
                  }
                  frame True {
                    n444 = for {
                      shift-right: [w1160] -> w1158
                      shift-left: w1156 -> [w1161]
                      tunnel: string[] ["CAM CLOSE", "", ""] -> [w1159] mode=indexing
                      n445 = Enqueue Element(queue=w1161, element=w1159) -> (queue out=w1160:refnum<queue>)  [unwired: 2 in, 2 out]
                    }
                  }
                }
                n446 = Or(x=w1139, y=w1144) -> (x .or. y?=w1146:bool)
                n447 = Select(t=State_Type_Definitions,_for_0.26g_versions_and_later_3."True Stop" ("Enum"), s=w1144, f=State_Type_Definitions,_for_0.26g_versions_and_later_3."Task 5E: GOING UP" ("Enum")) -> (s? t:f=w1141:T18)
                n448 = Select(t=w1141, s=w1146, f=State_Type_Definitions,_for_0.26g_versions_and_later_3."Task 5D: GRAB" ("Enum")) -> (s? t:f=w1145:T18)
              }
              frame "Exit" {
                n449 = for {
                  shift-right: [w1168] -> w1165
                  shift-left: w1162 -> [w1169]
                  tunnel: string[] ["STOP", "RESET ENCODERS", "RESET YAW", "ARDUINO MODE 0"] -> [w1167] mode=indexing
                  n450 = Enqueue Element(queue=w1169, element=w1167) -> (queue out=w1168:refnum<queue>)  [unwired: 2 in, 2 out]
                }
              }
            }
          }
          frame "Task 5E: GOING UP" {
            # ">>> yStepper command>>>"
            n451 = Dequeue Element(queue=w1183, timeout in ms (-1)=w1184, error in (no error)=w1185) -> (element=w1187:T10)  [unwired: 3 out]
            n452 = formula code="if (pos < 100)\ny = 41;\n\nelse if (pos >= 100 && pos <= 140)\ny = 30;\n\nelse if (pos >= 141 && pos <= 170)\ny = 25;\n\nelse if (pos >= 171 &&pos <= 180) \ny = 20;\n\nelse if (pos >= 181&& pos <= 200)\ny = 15;\n\nelse if (pos >= 201 && pos <= 230)\ny = 10;\n\nelse if (pos >= 231 && pos <= 320)\ny = 8;\n\nelse if (pos > 320)\ny = 0;"("pos"=w1175) -> ("y"=w1178:dbl)
            n453 = To Unsigned Byte Integer(number=w1178) -> (unsigned 8bit integer=w1173:u8)
            n454 = Equal?(x=w1174, y=w1173) -> (x = y?=w1172:bool)
            n455 = case shown="\"Start Task 1\", Default" w1187 {
              tunnel: [w1194 State_Type_Definitions,_for_0.26g_versions_and_later_3."True Stop" ("Enum")] -> w1181
              tunnel: [w1197 w1214] -> w1179
              tunnel: [State_Type_Definitions,_for_0.26g_versions_and_later_3."Idle" ("Enum") State_Type_Definitions,_for_0.26g_versions_and_later_3."Shutdown" ("Enum")] -> w1180
              tunnel: w1186 -> [w1193 _]
              tunnel: w1182 -> [w1189 w1211]
              tunnel: w1172 -> [w1188 _]
              frame "Start Task 1", Default {
                # ">> T: Breaks out of state loop; F: Stays in loop>>"
                # ">> Manual override >>"
                # ">> Checks if time is up>>"
                # "Stays in Task 5D until the object is detected"
                # "T: Go back to idle, F: Continue with task\""
                # ">> Manual override >>"
                n456 = case shown="False" w1188 {
                  tunnel: [w1201 w1207] -> w1197
                  tunnel: w1189 -> [w1199 w1205]
                  frame False {
                    n457 = for {
                      tunnel: string[] ["READ STEPPER VALUES", "Y STEPPER CONTROL", ""] ("element") -> [w1202] mode=indexing
                      shift-right: [w1204] -> w1201
                      shift-left: w1199 -> [w1203]
                      n458 = Enqueue Element(queue=w1203, element=w1202) -> (queue out=w1204:refnum<queue>)  [unwired: 2 in, 2 out]
                    }
                  }
                  frame True {
                    n459 = for {
                      shift-right: [w1209] -> w1207
                      shift-left: w1205 -> [w1210]
                      tunnel: string[] ["CAM CLOSE", "DISPOSE BUFFERS", ""] -> [w1208] mode=indexing
                      n460 = Enqueue Element(queue=w1210, element=w1208) -> (queue out=w1209:refnum<queue>)  [unwired: 2 in, 2 out]
                    }
                  }
                }
                n461 = Or(x=w1188, y=w1193) -> (x .or. y?=w1195:bool)
                n462 = Select(t=State_Type_Definitions,_for_0.26g_versions_and_later_3."True Stop" ("Enum"), s=w1193, f=State_Type_Definitions,_for_0.26g_versions_and_later_3."Task 5F: ARM GRAB HEIGHT" ("Enum")) -> (s? t:f=w1190:T18)
                n463 = Select(t=w1190, s=w1195, f=State_Type_Definitions,_for_0.26g_versions_and_later_3."Task 5E: GOING UP" ("Enum")) -> (s? t:f=w1194:T18)
              }
              frame "Exit" {
                n464 = for {
                  shift-right: [w1217] -> w1214
                  shift-left: w1211 -> [w1218]
                  tunnel: string[] ["STOP", "RESET ENCODERS", "RESET YAW", "ARDUINO MODE 0"] -> [w1216] mode=indexing
                  n465 = Enqueue Element(queue=w1218, element=w1216) -> (queue out=w1217:refnum<queue>)  [unwired: 2 in, 2 out]
                }
              }
            }
            n466 = Bundle By Name(cluster=w1177, "yStepper desired"=w1173) -> (w1176:T20)
          }
          frame "Task 5F: ARM GRAB HEIGHT" {
            # ">>> Motor control cluster >>>"
            # ">>> yStepper command>>>"
            # ">> Manual override >>"
            n467 = Dequeue Element(queue=w1229, timeout in ms (-1)=w1228, error in (no error)=w1230) -> (element=w1227:T10)  [unwired: 3 out]
            n468 = Equal?(x=w1226, y=u8 1) -> (x = y?=w1224:bool)
            n469 = case shown="\"Start Task 1\", Default" w1227 {
              tunnel: [w1240 State_Type_Definitions,_for_0.26g_versions_and_later_3."True Stop" ("Enum")] -> w1231
              tunnel: [w1243 w1260] -> w1232
              tunnel: [State_Type_Definitions,_for_0.26g_versions_and_later_3."Idle" ("Enum") State_Type_Definitions,_for_0.26g_versions_and_later_3."Shutdown" ("Enum")] -> w1233
              tunnel: w1224 -> [w1239 _]
              tunnel: w1223 -> [w1238 _]
              tunnel: w1222 -> [w1234 w1257]
              frame "Start Task 1", Default {
                # "Stays in Task 5F until stepper reaches desired \nheight"
                # "T: Go back to idle, F: Continue with task\""
                # ">> Manual override >>"
                n470 = case shown="True" w1239 {
                  tunnel: [w1247 w1253] -> w1243
                  tunnel: w1234 -> [w1245 w1251]
                  frame False {
                    n471 = for {
                      tunnel: string[] ["Z STEPPER GRAB HEIGHT", "READ STEPPER VALUES"] ("element") -> [w1248] mode=indexing
                      shift-right: [w1250] -> w1247
                      shift-left: w1245 -> [w1249]
                      n472 = Enqueue Element(queue=w1249, element=w1248) -> (queue out=w1250:refnum<queue>)  [unwired: 2 in, 2 out]
                    }
                  }
                  frame True {
                    n473 = for {
                      shift-right: [w1255] -> w1253
                      shift-left: w1251 -> [w1256]
                      tunnel: string[] ["SET TIMER 5", "CLOSE CLAW", ""] -> [w1254] mode=indexing
                      n474 = Enqueue Element(queue=w1256, element=w1254) -> (queue out=w1255:refnum<queue>)  [unwired: 2 in, 2 out]
                    }
                  }
                }
                n475 = Or(x=w1239, y=w1238) -> (x .or. y?=w1241:bool)
                n476 = Select(t=State_Type_Definitions,_for_0.26g_versions_and_later_3."True Stop" ("Enum"), s=w1238, f=State_Type_Definitions,_for_0.26g_versions_and_later_3."Task 5G: CLOSE CLAW" ("Enum")) -> (s? t:f=w1235:T18)
                n477 = Select(t=w1235, s=w1241, f=State_Type_Definitions,_for_0.26g_versions_and_later_3."Task 5F: ARM GRAB HEIGHT" ("Enum")) -> (s? t:f=w1240:T18)
              }
              frame "Exit" {
                n478 = for {
                  shift-right: [w1263] -> w1260
                  shift-left: w1257 -> [w1264]
                  tunnel: string[] ["STOP", "RESET ENCODERS", "RESET YAW", "ARDUINO MODE 0"] -> [w1262] mode=indexing
                  n479 = Enqueue Element(queue=w1264, element=w1262) -> (queue out=w1263:refnum<queue>)  [unwired: 2 in, 2 out]
                }
              }
            }
          }
          frame "Task 5G: CLOSE CLAW" {
            # ">>> yStepper command>>>"
            # ">> Manual override >>"
            n480 = Dequeue Element(queue=w1275, timeout in ms (-1)=w1274, error in (no error)=w1273) -> (element=w1272:T10)  [unwired: 3 out]
            n481 = case shown="\"Start Task 1\", Default" w1272 {
              tunnel: [w1284 State_Type_Definitions,_for_0.26g_versions_and_later_3."True Stop" ("Enum")] -> w1277
              tunnel: [w1287 w1304] -> w1270
              tunnel: [State_Type_Definitions,_for_0.26g_versions_and_later_3."Idle" ("Enum") State_Type_Definitions,_for_0.26g_versions_and_later_3."Shutdown" ("Enum")] -> w1269
              tunnel: w1271 -> [w1278 _]
              tunnel: w1276 -> [w1283 w1301]
              tunnel: w1267 -> [w1282 _]
              frame "Start Task 1", Default {
                # ">> Is time up? >>"
                # "Determines if object is in range to pick up"
                # ">> Manual override >>"
                n482 = case shown="True" w1282 {
                  tunnel: [w1291 w1297] -> w1287
                  tunnel: w1283 -> [w1289 w1295]
                  frame False {
                    n483 = for {
                      tunnel: string[] ["CLOSE CLAW", "START TIMER"] ("element") -> [w1292] mode=indexing
                      shift-right: [w1294] -> w1291
                      shift-left: w1289 -> [w1293]
                      n484 = Enqueue Element(queue=w1293, element=w1292) -> (queue out=w1294:refnum<queue>)  [unwired: 2 in, 2 out]
                    }
                  }
                  frame True {
                    n485 = for {
                      shift-right: [w1299] -> w1297
                      shift-left: w1295 -> [w1300]
                      tunnel: string[] ["READ STEPPER VALUES", "", ""] -> [w1298] mode=indexing
                      n486 = Enqueue Element(queue=w1300, element=w1298) -> (queue out=w1299:refnum<queue>)  [unwired: 2 in, 2 out]
                    }
                  }
                }
                n487 = Or(x=w1282, y=w1278) -> (x .or. y?=w1285:bool)
                n488 = Select(t=State_Type_Definitions,_for_0.26g_versions_and_later_3."True Stop" ("Enum"), s=w1278, f=State_Type_Definitions,_for_0.26g_versions_and_later_3."Task 5H: RAISE ARM" ("Enum")) -> (s? t:f=w1280:T18)
                n489 = Select(t=w1280, s=w1285, f=State_Type_Definitions,_for_0.26g_versions_and_later_3."Task 5G: CLOSE CLAW" ("Enum")) -> (s? t:f=w1284:T18)
              }
              frame "Exit" {
                n490 = for {
                  shift-right: [w1307] -> w1304
                  shift-left: w1301 -> [w1308]
                  tunnel: string[] ["STOP", "RESET ENCODERS", "RESET YAW", "ARDUINO MODE 0"] -> [w1306] mode=indexing
                  n491 = Enqueue Element(queue=w1308, element=w1306) -> (queue out=w1307:refnum<queue>)  [unwired: 2 in, 2 out]
                }
              }
            }
          }
          frame "Task 5H: RAISE ARM" {
            # ">>> yStepper command>>>"
            # ">> Manual override >>"
            n492 = Dequeue Element(queue=w1319, timeout in ms (-1)=w1318, error in (no error)=w1320) -> (element=w1317:T10)  [unwired: 3 out]
            n493 = Equal?(x=w1316, y=u8 60) -> (x = y?=w1314:bool)
            n494 = case shown="\"Start Task 1\", Default" w1317 {
              tunnel: [w1330 State_Type_Definitions,_for_0.26g_versions_and_later_3."True Stop" ("Enum")] -> w1321
              tunnel: [w1333 w1350] -> w1322
              tunnel: [State_Type_Definitions,_for_0.26g_versions_and_later_3."Idle" ("Enum") State_Type_Definitions,_for_0.26g_versions_and_later_3."Shutdown" ("Enum")] -> w1323
              tunnel: w1314 -> [w1329 _]
              tunnel: w1313 -> [w1328 _]
              tunnel: w1312 -> [w1324 w1347]
              frame "Start Task 1", Default {
                # "Stays in Task 5_A until stepper reaches desired \nheight"
                # "T: Go back to idle, F: Continue with task\""
                # ">> Manual override >>"
                n495 = case shown="False" w1329 {
                  tunnel: [w1337 w1343] -> w1333
                  tunnel: w1324 -> [w1335 w1341]
                  frame False {
                    n496 = for {
                      tunnel: string[] ["Z STEPPER CAM HEIGHT", "READ STEPPER VALUES"] ("element") -> [w1338] mode=indexing
                      shift-right: [w1340] -> w1337
                      shift-left: w1335 -> [w1339]
                      n497 = Enqueue Element(queue=w1339, element=w1338) -> (queue out=w1340:refnum<queue>)  [unwired: 2 in, 2 out]
                    }
                  }
                  frame True {
                    n498 = for {
                      shift-right: [w1345] -> w1343
                      shift-left: w1341 -> [w1346]
                      tunnel: string[] ["ARDUINO - ULTRASONIC", "READ ULTRASONIC", ""] -> [w1344] mode=indexing
                      n499 = Enqueue Element(queue=w1346, element=w1344) -> (queue out=w1345:refnum<queue>)  [unwired: 2 in, 2 out]
                    }
                  }
                }
                n500 = Or(x=w1329, y=w1328) -> (x .or. y?=w1331:bool)
                n501 = Select(t=State_Type_Definitions,_for_0.26g_versions_and_later_3."True Stop" ("Enum"), s=w1328, f=State_Type_Definitions,_for_0.26g_versions_and_later_3."True Stop" ("Enum")) -> (s? t:f=w1325:T18)
                n502 = Select(t=w1325, s=w1331, f=State_Type_Definitions,_for_0.26g_versions_and_later_3."Task 5H: RAISE ARM" ("Enum")) -> (s? t:f=w1330:T18)
              }
              frame "Exit" {
                n503 = for {
                  shift-right: [w1353] -> w1350
                  shift-left: w1347 -> [w1354]
                  tunnel: string[] ["STOP", "RESET ENCODERS", "RESET YAW", "ARDUINO MODE 0"] -> [w1352] mode=indexing
                  n504 = Enqueue Element(queue=w1354, element=w1352) -> (queue out=w1353:refnum<queue>)  [unwired: 2 in, 2 out]
                }
              }
            }
          }
          frame "Task 6A: RAISE ARM" {
            # ">>> Motor control cluster >>>"
            # ">>> yStepper command>>>"
            n505 = Equal?(x=w1362, y=u8 60) -> (x = y?=w1356:bool)
            n506 = Dequeue Element(queue=w1366, timeout in ms (-1)=w1365, error in (no error)=w1364) -> (element=w1371:T10)  [unwired: 3 out]
            n507 = local read "Rising Edge"() -> (w1357:bool)
            n508 = And(x=w1357, y=w1356) -> (x .and. y?=w1355:bool)
            n509 = case shown="\"Start Task 1\", Default" w1371 {
              tunnel: [w1381 State_Type_Definitions,_for_0.26g_versions_and_later_3."True Stop" ("Enum")] -> w1369
              tunnel: [w1380 w1397] -> w1368
              tunnel: [State_Type_Definitions,_for_0.26g_versions_and_later_3."Idle" ("Enum") State_Type_Definitions,_for_0.26g_versions_and_later_3."Shutdown" ("Enum")] -> w1370
              tunnel: w1367 -> [w1377 _]
              tunnel: w1363 -> [w1378 _]
              tunnel: w1355 -> [w1375 _]
              frame "Start Task 1", Default {
                n510 = Or(x=w1375, y=w1377) -> (x .or. y?=w1372:bool)
                n511 = case shown="False" w1372 {
                  tunnel: [w1385 w1391] -> w1380
                  tunnel: w1378 -> [w1383 w1390]
                  frame False {
                    n512 = for {
                      tunnel: string[] ["Z STEPPER CAM HEIGHT", "READ STEPPER VALUES"] ("element") -> [w1386] mode=indexing
                      shift-right: [w1388] -> w1385
                      shift-left: w1383 -> [w1387]
                      n513 = Enqueue Element(queue=w1387, element=w1386) -> (queue out=w1388:refnum<queue>)  [unwired: 2 in, 2 out]
                    }
                  }
                  frame True {
                    n514 = for {
                      shift-right: [w1393] -> w1391
                      shift-left: w1390 -> [w1394]
                      tunnel: string[] ["OPEN LOG CAM", "SET TIMER 2", "OPEN IMAQ REF", "", ""] -> [w1392] mode=indexing
                      n515 = Enqueue Element(queue=w1394, element=w1392) -> (queue out=w1393:refnum<queue>)  [unwired: 2 in, 2 out]
                    }
                  }
                }
                n516 = Select(t=State_Type_Definitions,_for_0.26g_versions_and_later_3."Task 6B: CAM BURST" ("Enum"), s=w1375, f=State_Type_Definitions,_for_0.26g_versions_and_later_3."True Stop" ("Enum")) -> (s? t:f=w1373:T18)
                n517 = Select(t=w1373, s=w1372, f=State_Type_Definitions,_for_0.26g_versions_and_later_3."Task 6A: RAISE ARM" ("Enum")) -> (s? t:f=w1381:T18)
              }
              frame "Exit" {
                n518 = for {
                  shift-right: [w1400] -> w1397
                  shift-left: _ -> [w1401]
                  tunnel: string[] ["STOP", "RESET ENCODERS", "RESET YAW", "ARDUINO MODE 0"] -> [w1399] mode=indexing
                  n519 = Enqueue Element(queue=w1401, element=w1399) -> (queue out=w1400:refnum<queue>)  [unwired: 2 in, 2 out]
                }
              }
            }
          }
          frame "Task 6B: CAM BURST" {
            # ">> Manual override >>"
            # ">>> Motor control cluster >>>"
            # ">>> yStepper command>>>"
            n520 = Dequeue Element(queue=w1413, timeout in ms (-1)=w1411, error in (no error)=w1412) -> (element=w1410:T10)  [unwired: 3 out]
            n521 = case shown="\"Start Task 1\", Default" w1410 {
              tunnel: [w1421 State_Type_Definitions,_for_0.26g_versions_and_later_3."True Stop" ("Enum")] -> w1407
              tunnel: [w1419 w1439] -> w1414
              tunnel: [State_Type_Definitions,_for_0.26g_versions_and_later_3."Idle" ("Enum") State_Type_Definitions,_for_0.26g_versions_and_later_3."Shutdown" ("Enum")] -> w1408
              tunnel: w1409 -> [w1417 _]
              tunnel: w1406 -> [w1418 w1436]
              tunnel: w1402 -> [w1415 _]
              frame "Start Task 1", Default {
                n522 = Or(x=w1415, y=w1417) -> (x .or. y?=w1416:bool)
                n523 = case shown="True" w1416 {
                  tunnel: [w1426 w1432] -> w1419
                  tunnel: w1418 -> [w1424 w1430]
                  frame False {
                    n524 = for {
                      tunnel: string[] ["CAM ACQ", "START TIMER"] ("element") -> [w1427] mode=indexing
                      shift-right: [w1429] -> w1426
                      shift-left: w1424 -> [w1428]
                      n525 = Enqueue Element(queue=w1428, element=w1427) -> (queue out=w1429:refnum<queue>)  [unwired: 2 in, 2 out]
                    }
                  }
                  frame True {
                    n526 = for {
                      shift-right: [w1434] -> w1432
                      shift-left: w1430 -> [w1435]
                      tunnel: string[] ["CAM CLOSE", "PROCESS IMAGE", "SET TIMER 2", "RESET ENCODERS"] -> [w1433] mode=indexing
                      n527 = Enqueue Element(queue=w1435, element=w1433) -> (queue out=w1434:refnum<queue>)  [unwired: 2 in, 2 out]
                    }
                  }
                }
                n528 = Select(t=State_Type_Definitions,_for_0.26g_versions_and_later_3."Task 6C: PROCESS IMAGE" ("Enum"), s=w1416, f=State_Type_Definitions,_for_0.26g_versions_and_later_3."Task 6B: CAM BURST" ("Enum")) -> (s? t:f=w1421:T18)
              }
              frame "Exit" {
                # ">> State after true stop >>"
                # ">> Goes to true stop >>"
                n529 = for {
                  shift-right: [w1442] -> w1439
                  shift-left: w1436 -> [w1443]
                  tunnel: string[] ["STOP", "RESET ENCODERS", "RESET YAW", ""] -> [w1441] mode=indexing
                  n530 = Enqueue Element(queue=w1443, element=w1441) -> (queue out=w1442:refnum<queue>)  [unwired: 2 in, 2 out]
                }
              }
            }
          }
          frame "Task 6C: PROCESS IMAGE" {
            # "Ball > Soap > Gel > Pipe"
            # ">>> Motor control cluster >>>"
            # ">>> yStepper command>>>"
            n531 = Dequeue Element(queue=w1452, timeout in ms (-1)=w1451, error in (no error)=w1450) -> (element=w1449:T10)  [unwired: 3 out]
            n532 = case shown="\"Start Task 1\", Default" w1449 {
              tunnel: [w1468 State_Type_Definitions,_for_0.26g_versions_and_later_3."True Stop" ("Enum")] -> w1456
              tunnel: [w1470 w1487] -> w1455
              tunnel: [State_Type_Definitions,_for_0.26g_versions_and_later_3."Idle" ("Enum") State_Type_Definitions,_for_0.26g_versions_and_later_3."Shutdown" ("Enum")] -> w1457
              tunnel: w1453 -> [w1459 _]
              tunnel: w1454 -> [w1465 w1484]
              tunnel: w1445 -> [w1463 _]
              tunnel: w1444 -> [w1464 _]
              frame "Start Task 1", Default {
                # "Stays in Task 5D until the object is detected"
                n533 = Or(x=w1463, y=w1459) -> (x .or. y?=w1462:bool)
                n534 = case shown="True" w1462 {
                  tunnel: [w1474 w1480] -> w1470
                  tunnel: w1465 -> [w1472 w1478]
                  frame False {
                    n535 = for {
                      tunnel: string[] ["START TIMER", "PROCESS IMAGE", ""] ("element") -> [w1475] mode=indexing
                      shift-right: [w1477] -> w1474
                      shift-left: w1472 -> [w1476]
                      n536 = Enqueue Element(queue=w1476, element=w1475) -> (queue out=w1477:refnum<queue>)  [unwired: 2 in, 2 out]
                    }
                  }
                  frame True {
                    n537 = for {
                      shift-right: [w1482] -> w1480
                      shift-left: w1478 -> [w1483]
                      tunnel: string[] ["RESET ENCODERS", "RESET YAW", ""] -> [w1481] mode=indexing
                      n538 = Enqueue Element(queue=w1483, element=w1481) -> (queue out=w1482:refnum<queue>)  [unwired: 2 in, 2 out]
                    }
                  }
                }
                n539 = Select(t=State_Type_Definitions,_for_0.26g_versions_and_later_3."Task 6D: BALL BUSTER" ("Enum"), s=w1464, f=State_Type_Definitions,_for_0.26g_versions_and_later_3."Task 6F: CAM BURST 2" ("Enum")) -> (s? t:f=w1460:T18)
                n540 = Select(t=State_Type_Definitions,_for_0.26g_versions_and_later_3."True Stop" ("Enum"), s=w1459, f=w1460) -> (s? t:f=w1466:T18)
                n541 = Select(t=w1466, s=w1462, f=State_Type_Definitions,_for_0.26g_versions_and_later_3."Task 6C: PROCESS IMAGE" ("Enum")) -> (s? t:f=w1468:T18)
              }
              frame "Exit" {
                n542 = for {
                  shift-right: [w1490] -> w1487
                  shift-left: w1484 -> [w1491]
                  tunnel: string[] ["STOP", "RESET ENCODERS", "RESET YAW", "ARDUINO MODE 0"] -> [w1489] mode=indexing
                  n543 = Enqueue Element(queue=w1491, element=w1489) -> (queue out=w1490:refnum<queue>)  [unwired: 2 in, 2 out]
                }
              }
            }
          }
          frame "Task 6D: BALL BUSTER" {
            # "Ball > Soap > Gel > Pipe"
            # ">>> Motor control cluster >>>"
            # ">>> yStepper command>>>"
            n544 = Greater Or Equal?(x=w1492, y=20.0) -> (x >= y?=w1493:bool)
            n545 = Dequeue Element(queue=w1501, timeout in ms (-1)=w1500, error in (no error)=w1499) -> (element=w1498:T10)  [unwired: 3 out]
            n546 = case shown="\"Start Task 1\", Default" w1498 {
              tunnel: [w1514 State_Type_Definitions,_for_0.26g_versions_and_later_3."True Stop" ("Enum")] -> w1505
              tunnel: [w1516 w1533] -> w1504
              tunnel: [State_Type_Definitions,_for_0.26g_versions_and_later_3."Idle" ("Enum") State_Type_Definitions,_for_0.26g_versions_and_later_3."Shutdown" ("Enum")] -> w1506
              tunnel: w1502 -> [w1509 _]
              tunnel: w1503 -> [w1511 w1530]
              tunnel: w1493 -> [w1508 _]
              frame "Start Task 1", Default {
                # "Stays in Task 5D until the object is detected"
                n547 = Or(x=w1508, y=w1509) -> (x .or. y?=w1510:bool)
                n548 = case shown="False" w1510 {
                  tunnel: [w1520 w1526] -> w1516
                  tunnel: w1511 -> [w1518 w1524]
                  frame False {
                    n549 = for {
                      tunnel: string[] ["RIGHT", "READ NAVX", "READ ENCODERS"] ("element") -> [w1521] mode=indexing
                      shift-right: [w1523] -> w1520
                      shift-left: w1518 -> [w1522]
                      n550 = Enqueue Element(queue=w1522, element=w1521) -> (queue out=w1523:refnum<queue>)  [unwired: 2 in, 2 out]
                    }
                  }
                  frame True {
                    n551 = for {
                      shift-right: [w1528] -> w1526
                      shift-left: w1524 -> [w1529]
                      tunnel: string[] ["RESET ENCODERS", "RESET YAW", "RESET FLAGS"] -> [w1527] mode=indexing
                      n552 = Enqueue Element(queue=w1529, element=w1527) -> (queue out=w1528:refnum<queue>)  [unwired: 2 in, 2 out]
                    }
                  }
                }
                n553 = Select(t=State_Type_Definitions,_for_0.26g_versions_and_later_3."True Stop" ("Enum"), s=w1509, f=State_Type_Definitions,_for_0.26g_versions_and_later_3."Task 6E: STILL WAITING" ("Enum")) -> (s? t:f=w1512:T18)
                n554 = Select(t=w1512, s=w1510, f=State_Type_Definitions,_for_0.26g_versions_and_later_3."Task 6D: BALL BUSTER" ("Enum")) -> (s? t:f=w1514:T18)
              }
              frame "Exit" {
                n555 = for {
                  shift-right: [w1536] -> w1533
                  shift-left: w1530 -> [w1537]
                  tunnel: string[] ["STOP", "RESET ENCODERS", "RESET YAW", "ARDUINO MODE 0"] -> [w1535] mode=indexing
                  n556 = Enqueue Element(queue=w1537, element=w1535) -> (queue out=w1536:refnum<queue>)  [unwired: 2 in, 2 out]
                }
              }
            }
          }
          frame "Task 6E: STILL WAITING" {
            # "Ball > Soap > Gel > Pipe"
            # ">>> Motor control cluster >>>"
            # ">>> yStepper command>>>"
            n557 = local read "Rising Edge"() -> (w1539:bool)
            n558 = Dequeue Element(queue=w1545, timeout in ms (-1)=w1544, error in (no error)=w1543) -> (element=w1542:T10)  [unwired: 3 out]
            n559 = case shown="\"Start Task 1\", Default" w1542 {
              tunnel: [w1559 State_Type_Definitions,_for_0.26g_versions_and_later_3."True Stop" ("Enum")] -> w1549
              tunnel: [w1552 w1577] -> w1548
              tunnel: [State_Type_Definitions,_for_0.26g_versions_and_later_3."Idle" ("Enum") State_Type_Definitions,_for_0.26g_versions_and_later_3."Shutdown" ("Enum")] -> w1550
              tunnel: w1546 -> [w1556 _]
              tunnel: w1547 -> [w1553 w1574]
              tunnel: w1539 -> [w1554 _]
              frame "Start Task 1", Default {
                # "Stays in Task 5D until the object is detected"
                n560 = Or(x=w1554, y=w1556) -> (x .or. y?=w1551:bool)
                n561 = case shown="False" w1551 {
                  tunnel: [w1564 w1570] -> w1552
                  tunnel: w1553 -> [w1562 w1569]
                  frame False {
                    n562 = for {
                      tunnel: string[] ["Z STEPPER CAM HEIGHT", "READ STEPPER VALUES"] ("element") -> [w1565] mode=indexing
                      shift-right: [w1567] -> w1564
                      shift-left: w1562 -> [w1566]
                      n563 = Enqueue Element(queue=w1566, element=w1565) -> (queue out=w1567:refnum<queue>)  [unwired: 2 in, 2 out]
                    }
                  }
                  frame True {
                    n564 = for {
                      shift-right: [w1572] -> w1570
                      shift-left: w1569 -> [w1573]
                      tunnel: string[] ["OPEN LOG CAM", "SET TIMER 2", "OPEN IMAQ REF", "", ""] -> [w1571] mode=indexing
                      n565 = Enqueue Element(queue=w1573, element=w1571) -> (queue out=w1572:refnum<queue>)  [unwired: 2 in, 2 out]
                    }
                  }
                }
                n566 = Select(t=State_Type_Definitions,_for_0.26g_versions_and_later_3."True Stop" ("Enum"), s=w1556, f=State_Type_Definitions,_for_0.26g_versions_and_later_3."Task 6F: CAM BURST 2" ("Enum")) -> (s? t:f=w1557:T18)
                n567 = Select(t=w1557, s=w1551, f=State_Type_Definitions,_for_0.26g_versions_and_later_3."Task 6E: STILL WAITING" ("Enum")) -> (s? t:f=w1559:T18)
              }
              frame "Exit" {
                n568 = for {
                  shift-right: [w1580] -> w1577
                  shift-left: w1574 -> [w1581]
                  tunnel: string[] ["STOP", "RESET ENCODERS", "RESET YAW", "ARDUINO MODE 0"] -> [w1579] mode=indexing
                  n569 = Enqueue Element(queue=w1581, element=w1579) -> (queue out=w1580:refnum<queue>)  [unwired: 2 in, 2 out]
                }
              }
            }
          }
          frame "Task 6F: CAM BURST 2" {
            # ">> Manual override >>"
            # ">>> Motor control cluster >>>"
            # ">>> yStepper command>>>"
            n570 = Dequeue Element(queue=w1593, timeout in ms (-1)=w1591, error in (no error)=w1592) -> (element=w1590:T10)  [unwired: 3 out]
            n571 = case shown="\"Start Task 1\", Default" w1590 {
              tunnel: [w1601 State_Type_Definitions,_for_0.26g_versions_and_later_3."True Stop" ("Enum")] -> w1587
              tunnel: [w1599 w1619] -> w1594
              tunnel: [State_Type_Definitions,_for_0.26g_versions_and_later_3."Idle" ("Enum") State_Type_Definitions,_for_0.26g_versions_and_later_3."Shutdown" ("Enum")] -> w1588
              tunnel: w1589 -> [w1597 _]
              tunnel: w1586 -> [w1598 w1616]
              tunnel: w1582 -> [w1595 _]
              frame "Start Task 1", Default {
                n572 = Or(x=w1595, y=w1597) -> (x .or. y?=w1596:bool)
                n573 = case shown="True" w1596 {
                  tunnel: [w1606 w1612] -> w1599
                  tunnel: w1598 -> [w1604 w1610]
                  frame False {
                    n574 = for {
                      tunnel: string[] ["CAM ACQ", "START TIMER"] ("element") -> [w1607] mode=indexing
                      shift-right: [w1609] -> w1606
                      shift-left: w1604 -> [w1608]
                      n575 = Enqueue Element(queue=w1608, element=w1607) -> (queue out=w1609:refnum<queue>)  [unwired: 2 in, 2 out]
                    }
                  }
                  frame True {
                    n576 = for {
                      shift-right: [w1614] -> w1612
                      shift-left: w1610 -> [w1615]
                      tunnel: string[] ["CAM CLOSE", "PROCESS IMAGE", "SET TIMER 2", "RESET ENCODERS"] -> [w1613] mode=indexing
                      n577 = Enqueue Element(queue=w1615, element=w1613) -> (queue out=w1614:refnum<queue>)  [unwired: 2 in, 2 out]
                    }
                  }
                }
                n578 = Select(t=State_Type_Definitions,_for_0.26g_versions_and_later_3."Task 6G: PROCESS IMAGE 2" ("Enum"), s=w1596, f=State_Type_Definitions,_for_0.26g_versions_and_later_3."Task 6F: CAM BURST 2" ("Enum")) -> (s? t:f=w1601:T18)
              }
              frame "Exit" {
                # ">> State after true stop >>"
                # ">> Goes to true stop >>"
                n579 = for {
                  shift-right: [w1622] -> w1619
                  shift-left: w1616 -> [w1623]
                  tunnel: string[] ["STOP", "RESET ENCODERS", "RESET YAW", ""] -> [w1621] mode=indexing
                  n580 = Enqueue Element(queue=w1623, element=w1621) -> (queue out=w1622:refnum<queue>)  [unwired: 2 in, 2 out]
                }
              }
            }
          }
          frame "Task 6G: PROCESS IMAGE 2" {
            # "Ball > Soap > Gel > Pipe"
            # ">>> Motor control cluster >>>"
            # ">>> yStepper command>>>"
            n581 = Dequeue Element(queue=w1632, timeout in ms (-1)=w1631, error in (no error)=w1630) -> (element=w1629:T10)  [unwired: 3 out]
            n582 = case shown="\"Start Task 1\", Default" w1629 {
              tunnel: [w1648 State_Type_Definitions,_for_0.26g_versions_and_later_3."True Stop" ("Enum")] -> w1636
              tunnel: [w1650 w1667] -> w1635
              tunnel: [State_Type_Definitions,_for_0.26g_versions_and_later_3."Idle" ("Enum") State_Type_Definitions,_for_0.26g_versions_and_later_3."Shutdown" ("Enum")] -> w1637
              tunnel: w1633 -> [w1639 _]
              tunnel: w1634 -> [w1645 w1664]
              tunnel: w1625 -> [w1643 _]
              tunnel: w1624 -> [w1644 _]
              frame "Start Task 1", Default {
                # "Stays in Task 5D until the object is detected"
                n583 = Or(x=w1643, y=w1639) -> (x .or. y?=w1642:bool)
                n584 = case shown="True" w1642 {
                  tunnel: [w1654 w1660] -> w1650
                  tunnel: w1645 -> [w1652 w1658]
                  frame False {
                    n585 = for {
                      tunnel: string[] ["START TIMER", "PROCESS IMAGE", ""] ("element") -> [w1655] mode=indexing
                      shift-right: [w1657] -> w1654
                      shift-left: w1652 -> [w1656]
                      n586 = Enqueue Element(queue=w1656, element=w1655) -> (queue out=w1657:refnum<queue>)  [unwired: 2 in, 2 out]
                    }
                  }
                  frame True {
                    n587 = for {
                      shift-right: [w1662] -> w1660
                      shift-left: w1658 -> [w1663]
                      tunnel: string[] ["RESET ENCODERS", "RESET YAW", ""] -> [w1661] mode=indexing
                      n588 = Enqueue Element(queue=w1663, element=w1661) -> (queue out=w1662:refnum<queue>)  [unwired: 2 in, 2 out]
                    }
                  }
                }
                n589 = Select(t=State_Type_Definitions,_for_0.26g_versions_and_later_3."Task 6H: SKADI SOAPS" ("Enum"), s=w1644, f=State_Type_Definitions,_for_0.26g_versions_and_later_3."Task 6J: CAM BURST 3" ("Enum")) -> (s? t:f=w1640:T18)
                n590 = Select(t=State_Type_Definitions,_for_0.26g_versions_and_later_3."True Stop" ("Enum"), s=w1639, f=w1640) -> (s? t:f=w1646:T18)
                n591 = Select(t=w1646, s=w1642, f=State_Type_Definitions,_for_0.26g_versions_and_later_3."Task 6G: PROCESS IMAGE 2" ("Enum")) -> (s? t:f=w1648:T18)
              }
              frame "Exit" {
                n592 = for {
                  shift-right: [w1670] -> w1667
                  shift-left: w1664 -> [w1671]
                  tunnel: string[] ["STOP", "RESET ENCODERS", "RESET YAW", "ARDUINO MODE 0"] -> [w1669] mode=indexing
                  n593 = Enqueue Element(queue=w1671, element=w1669) -> (queue out=w1670:refnum<queue>)  [unwired: 2 in, 2 out]
                }
              }
            }
          }
          frame "Task 6H: SKADI SOAPS" {
            # "Ball > Soap > Gel > Pipe"
            # ">>> Motor control cluster >>>"
            # ">>> yStepper command>>>"
            n594 = Less Or Equal?(x=w1672, y=-20.0) -> (x <= y?=w1673:bool)
            n595 = Dequeue Element(queue=w1681, timeout in ms (-1)=w1680, error in (no error)=w1679) -> (element=w1678:T10)  [unwired: 3 out]
            n596 = case shown="\"Start Task 1\", Default" w1678 {
              tunnel: [w1694 State_Type_Definitions,_for_0.26g_versions_and_later_3."True Stop" ("Enum")] -> w1685
              tunnel: [w1696 w1713] -> w1684
              tunnel: [State_Type_Definitions,_for_0.26g_versions_and_later_3."Idle" ("Enum") State_Type_Definitions,_for_0.26g_versions_and_later_3."Shutdown" ("Enum")] -> w1686
              tunnel: w1682 -> [w1689 _]
              tunnel: w1683 -> [w1691 w1710]
              tunnel: w1673 -> [w1688 _]
              frame "Start Task 1", Default {
                # "Stays in Task 5D until the object is detected"
                n597 = Or(x=w1688, y=w1689) -> (x .or. y?=w1690:bool)
                n598 = case shown="False" w1690 {
                  tunnel: [w1700 w1706] -> w1696
                  tunnel: w1691 -> [w1698 w1704]
                  frame False {
                    n599 = for {
                      tunnel: string[] ["LEFT", "READ NAVX", "READ ENCODERS"] ("element") -> [w1701] mode=indexing
                      shift-right: [w1703] -> w1700
                      shift-left: w1698 -> [w1702]
                      n600 = Enqueue Element(queue=w1702, element=w1701) -> (queue out=w1703:refnum<queue>)  [unwired: 2 in, 2 out]
                    }
                  }
                  frame True {
                    n601 = for {
                      shift-right: [w1708] -> w1706
                      shift-left: w1704 -> [w1709]
                      tunnel: string[] ["RESET ENCODERS", "RESET YAW", "RESET FLAGS"] -> [w1707] mode=indexing
                      n602 = Enqueue Element(queue=w1709, element=w1707) -> (queue out=w1708:refnum<queue>)  [unwired: 2 in, 2 out]
                    }
                  }
                }
                n603 = Select(t=State_Type_Definitions,_for_0.26g_versions_and_later_3."True Stop" ("Enum"), s=w1689, f=State_Type_Definitions,_for_0.26g_versions_and_later_3."Task 6I: STILL WAITING 2" ("Enum")) -> (s? t:f=w1692:T18)
                n604 = Select(t=w1692, s=w1690, f=State_Type_Definitions,_for_0.26g_versions_and_later_3."Task 6H: SKADI SOAPS" ("Enum")) -> (s? t:f=w1694:T18)
              }
              frame "Exit" {
                n605 = for {
                  shift-right: [w1716] -> w1713
                  shift-left: w1710 -> [w1717]
                  tunnel: string[] ["STOP", "RESET ENCODERS", "RESET YAW", "ARDUINO MODE 0"] -> [w1715] mode=indexing
                  n606 = Enqueue Element(queue=w1717, element=w1715) -> (queue out=w1716:refnum<queue>)  [unwired: 2 in, 2 out]
                }
              }
            }
          }
          frame "Task 6I: STILL WAITING 2" {
            # "Ball > Soap > Gel > Pipe"
            # ">>> Motor control cluster >>>"
            # ">>> yStepper command>>>"
            n607 = local read "Rising Edge"() -> (w1719:bool)
            n608 = Dequeue Element(queue=w1725, timeout in ms (-1)=w1724, error in (no error)=w1723) -> (element=w1722:T10)  [unwired: 3 out]
            n609 = case shown="\"Start Task 1\", Default" w1722 {
              tunnel: [w1739 State_Type_Definitions,_for_0.26g_versions_and_later_3."True Stop" ("Enum")] -> w1729
              tunnel: [w1732 w1757] -> w1728
              tunnel: [State_Type_Definitions,_for_0.26g_versions_and_later_3."Idle" ("Enum") State_Type_Definitions,_for_0.26g_versions_and_later_3."Shutdown" ("Enum")] -> w1730
              tunnel: w1726 -> [w1736 _]
              tunnel: w1727 -> [w1733 w1754]
              tunnel: w1719 -> [w1734 _]
              frame "Start Task 1", Default {
                # "Stays in Task 5D until the object is detected"
                n610 = Or(x=w1734, y=w1736) -> (x .or. y?=w1731:bool)
                n611 = case shown="False" w1731 {
                  tunnel: [w1744 w1750] -> w1732
                  tunnel: w1733 -> [w1742 w1749]
                  frame False {
                    n612 = for {
                      tunnel: string[] ["Z STEPPER CAM HEIGHT", "READ STEPPER VALUES"] ("element") -> [w1745] mode=indexing
                      shift-right: [w1747] -> w1744
                      shift-left: w1742 -> [w1746]
                      n613 = Enqueue Element(queue=w1746, element=w1745) -> (queue out=w1747:refnum<queue>)  [unwired: 2 in, 2 out]
                    }
                  }
                  frame True {
                    n614 = for {
                      shift-right: [w1752] -> w1750
                      shift-left: w1749 -> [w1753]
                      tunnel: string[] ["OPEN LOG CAM", "SET TIMER 2", "OPEN IMAQ REF", "", ""] -> [w1751] mode=indexing
                      n615 = Enqueue Element(queue=w1753, element=w1751) -> (queue out=w1752:refnum<queue>)  [unwired: 2 in, 2 out]
                    }
                  }
                }
                n616 = Select(t=State_Type_Definitions,_for_0.26g_versions_and_later_3."True Stop" ("Enum"), s=w1736, f=State_Type_Definitions,_for_0.26g_versions_and_later_3."Task 6J: CAM BURST 3" ("Enum")) -> (s? t:f=w1737:T18)
                n617 = Select(t=w1737, s=w1731, f=State_Type_Definitions,_for_0.26g_versions_and_later_3."Task 6I: STILL WAITING 2" ("Enum")) -> (s? t:f=w1739:T18)
              }
              frame "Exit" {
                n618 = for {
                  shift-right: [w1760] -> w1757
                  shift-left: w1754 -> [w1761]
                  tunnel: string[] ["STOP", "RESET ENCODERS", "RESET YAW", "ARDUINO MODE 0"] -> [w1759] mode=indexing
                  n619 = Enqueue Element(queue=w1761, element=w1759) -> (queue out=w1760:refnum<queue>)  [unwired: 2 in, 2 out]
                }
              }
            }
          }
          frame "Task 6J: CAM BURST 3" {
            # ">> Manual override >>"
            # ">>> Motor control cluster >>>"
            # ">>> yStepper command>>>"
            n620 = Dequeue Element(queue=w1773, timeout in ms (-1)=w1771, error in (no error)=w1772) -> (element=w1770:T10)  [unwired: 3 out]
            n621 = case shown="\"Start Task 1\", Default" w1770 {
              tunnel: [w1781 State_Type_Definitions,_for_0.26g_versions_and_later_3."True Stop" ("Enum")] -> w1767
              tunnel: [w1779 w1799] -> w1774
              tunnel: [State_Type_Definitions,_for_0.26g_versions_and_later_3."Idle" ("Enum") State_Type_Definitions,_for_0.26g_versions_and_later_3."Shutdown" ("Enum")] -> w1768
              tunnel: w1769 -> [w1777 _]
              tunnel: w1766 -> [w1778 w1796]
              tunnel: w1762 -> [w1775 _]
              frame "Start Task 1", Default {
                n622 = Or(x=w1775, y=w1777) -> (x .or. y?=w1776:bool)
                n623 = case shown="True" w1776 {
                  tunnel: [w1786 w1792] -> w1779
                  tunnel: w1778 -> [w1784 w1790]
                  frame False {
                    n624 = for {
                      tunnel: string[] ["CAM ACQ", "START TIMER"] ("element") -> [w1787] mode=indexing
                      shift-right: [w1789] -> w1786
                      shift-left: w1784 -> [w1788]
                      n625 = Enqueue Element(queue=w1788, element=w1787) -> (queue out=w1789:refnum<queue>)  [unwired: 2 in, 2 out]
                    }
                  }
                  frame True {
                    n626 = for {
                      shift-right: [w1794] -> w1792
                      shift-left: w1790 -> [w1795]
                      tunnel: string[] ["CAM CLOSE", "PROCESS IMAGE", "SET TIMER 2", "RESET ENCODERS"] -> [w1793] mode=indexing
                      n627 = Enqueue Element(queue=w1795, element=w1793) -> (queue out=w1794:refnum<queue>)  [unwired: 2 in, 2 out]
                    }
                  }
                }
                n628 = Select(t=State_Type_Definitions,_for_0.26g_versions_and_later_3."Task 6K: PROCESS IMAGE 3" ("Enum"), s=w1776, f=State_Type_Definitions,_for_0.26g_versions_and_later_3."Task 6J: CAM BURST 3" ("Enum")) -> (s? t:f=w1781:T18)
              }
              frame "Exit" {
                # ">> State after true stop >>"
                # ">> Goes to true stop >>"
                n629 = for {
                  shift-right: [w1802] -> w1799
                  shift-left: w1796 -> [w1803]
                  tunnel: string[] ["STOP", "RESET ENCODERS", "RESET YAW", ""] -> [w1801] mode=indexing
                  n630 = Enqueue Element(queue=w1803, element=w1801) -> (queue out=w1802:refnum<queue>)  [unwired: 2 in, 2 out]
                }
              }
            }
          }
          frame "Task 6K: PROCESS IMAGE 3" {
            # "Ball > Soap > Gel > Pipe"
            # ">>> Motor control cluster >>>"
            # ">>> yStepper command>>>"
            n631 = Dequeue Element(queue=w1812, timeout in ms (-1)=w1811, error in (no error)=w1810) -> (element=w1809:T10)  [unwired: 3 out]
            n632 = case shown="\"Start Task 1\", Default" w1809 {
              tunnel: [w1828 State_Type_Definitions,_for_0.26g_versions_and_later_3."True Stop" ("Enum")] -> w1816
              tunnel: [w1830 w1847] -> w1815
              tunnel: [State_Type_Definitions,_for_0.26g_versions_and_later_3."Idle" ("Enum") State_Type_Definitions,_for_0.26g_versions_and_later_3."Shutdown" ("Enum")] -> w1817
              tunnel: w1813 -> [w1819 _]
              tunnel: w1814 -> [w1825 w1844]
              tunnel: w1805 -> [w1823 _]
              tunnel: w1804 -> [w1824 _]
              frame "Start Task 1", Default {
                # "Stays in Task 5D until the object is detected"
                n633 = Or(x=w1823, y=w1819) -> (x .or. y?=w1822:bool)
                n634 = case shown="True" w1822 {
                  tunnel: [w1834 w1840] -> w1830
                  tunnel: w1825 -> [w1832 w1838]
                  frame False {
                    n635 = for {
                      tunnel: string[] ["START TIMER", "PROCESS IMAGE", ""] ("element") -> [w1835] mode=indexing
                      shift-right: [w1837] -> w1834
                      shift-left: w1832 -> [w1836]
                      n636 = Enqueue Element(queue=w1836, element=w1835) -> (queue out=w1837:refnum<queue>)  [unwired: 2 in, 2 out]
                    }
                  }
                  frame True {
                    n637 = for {
                      shift-right: [w1842] -> w1840
                      shift-left: w1838 -> [w1843]
                      tunnel: string[] ["RESET ENCODERS", "RESET YAW", ""] -> [w1841] mode=indexing
                      n638 = Enqueue Element(queue=w1843, element=w1841) -> (queue out=w1842:refnum<queue>)  [unwired: 2 in, 2 out]
                    }
                  }
                }
                n639 = Select(t=State_Type_Definitions,_for_0.26g_versions_and_later_3."Task 6L: JAM IT IN" ("Enum"), s=w1824, f=State_Type_Definitions,_for_0.26g_versions_and_later_3."Task 6N: CAM BURST 4" ("Enum")) -> (s? t:f=w1820:T18)
                n640 = Select(t=State_Type_Definitions,_for_0.26g_versions_and_later_3."True Stop" ("Enum"), s=w1819, f=w1820) -> (s? t:f=w1826:T18)
                n641 = Select(t=w1826, s=w1822, f=State_Type_Definitions,_for_0.26g_versions_and_later_3."Task 6K: PROCESS IMAGE 3" ("Enum")) -> (s? t:f=w1828:T18)
              }
              frame "Exit" {
                n642 = for {
                  shift-right: [w1850] -> w1847
                  shift-left: w1844 -> [w1851]
                  tunnel: string[] ["STOP", "RESET ENCODERS", "RESET YAW", "ARDUINO MODE 0"] -> [w1849] mode=indexing
                  n643 = Enqueue Element(queue=w1851, element=w1849) -> (queue out=w1850:refnum<queue>)  [unwired: 2 in, 2 out]
                }
              }
            }
          }
          frame "Task 6L: JAM IT IN" {
            # "Ball > Soap > Gel > Pipe"
            # ">>> Motor control cluster >>>"
            # ">>> yStepper command>>>"
            n644 = Less Or Equal?(x=w1852, y=-20.0) -> (x <= y?=w1853:bool)
            n645 = Dequeue Element(queue=w1861, timeout in ms (-1)=w1860, error in (no error)=w1859) -> (element=w1858:T10)  [unwired: 3 out]
            n646 = case shown="\"Start Task 1\", Default" w1858 {
              tunnel: [w1874 State_Type_Definitions,_for_0.26g_versions_and_later_3."True Stop" ("Enum")] -> w1865
              tunnel: [w1876 w1893] -> w1864
              tunnel: [State_Type_Definitions,_for_0.26g_versions_and_later_3."Idle" ("Enum") State_Type_Definitions,_for_0.26g_versions_and_later_3."Shutdown" ("Enum")] -> w1866
              tunnel: w1862 -> [w1869 _]
              tunnel: w1863 -> [w1871 w1890]
              tunnel: w1853 -> [w1868 _]
              frame "Start Task 1", Default {
                # "Stays in Task 5D until the object is detected"
                n647 = Or(x=w1868, y=w1869) -> (x .or. y?=w1870:bool)
                n648 = case shown="False" w1870 {
                  tunnel: [w1880 w1886] -> w1876
                  tunnel: w1871 -> [w1878 w1884]
                  frame False {
                    n649 = for {
                      tunnel: string[] ["REVERSE", "READ NAVX", "READ ENCODERS"] ("element") -> [w1881] mode=indexing
                      shift-right: [w1883] -> w1880
                      shift-left: w1878 -> [w1882]
                      n650 = Enqueue Element(queue=w1882, element=w1881) -> (queue out=w1883:refnum<queue>)  [unwired: 2 in, 2 out]
                    }
                  }
                  frame True {
                    n651 = for {
                      shift-right: [w1888] -> w1886
                      shift-left: w1884 -> [w1889]
                      tunnel: string[] ["RESET ENCODERS", "RESET YAW", "RESET FLAGS"] -> [w1887] mode=indexing
                      n652 = Enqueue Element(queue=w1889, element=w1887) -> (queue out=w1888:refnum<queue>)  [unwired: 2 in, 2 out]
                    }
                  }
                }
                n653 = Select(t=State_Type_Definitions,_for_0.26g_versions_and_later_3."True Stop" ("Enum"), s=w1869, f=State_Type_Definitions,_for_0.26g_versions_and_later_3."Task 6M: STILL WAITING 3" ("Enum")) -> (s? t:f=w1872:T18)
                n654 = Select(t=w1872, s=w1870, f=State_Type_Definitions,_for_0.26g_versions_and_later_3."Task 6L: JAM IT IN" ("Enum")) -> (s? t:f=w1874:T18)
              }
              frame "Exit" {
                n655 = for {
                  shift-right: [w1896] -> w1893
                  shift-left: w1890 -> [w1897]
                  tunnel: string[] ["STOP", "RESET ENCODERS", "RESET YAW", "ARDUINO MODE 0"] -> [w1895] mode=indexing
                  n656 = Enqueue Element(queue=w1897, element=w1895) -> (queue out=w1896:refnum<queue>)  [unwired: 2 in, 2 out]
                }
              }
            }
          }
          frame "Task 6M: STILL WAITING 3" {
            # "Ball > Soap > Gel > Pipe"
            # ">>> Motor control cluster >>>"
            # ">>> yStepper command>>>"
            n657 = local read "Rising Edge"() -> (w1899:bool)
            n658 = Dequeue Element(queue=w1905, timeout in ms (-1)=w1904, error in (no error)=w1903) -> (element=w1902:T10)  [unwired: 3 out]
            n659 = case shown="\"Start Task 1\", Default" w1902 {
              tunnel: [w1919 State_Type_Definitions,_for_0.26g_versions_and_later_3."True Stop" ("Enum")] -> w1909
              tunnel: [w1912 w1937] -> w1908
              tunnel: [State_Type_Definitions,_for_0.26g_versions_and_later_3."Idle" ("Enum") State_Type_Definitions,_for_0.26g_versions_and_later_3."Shutdown" ("Enum")] -> w1910
              tunnel: w1906 -> [w1916 _]
              tunnel: w1907 -> [w1913 w1934]
              tunnel: w1899 -> [w1914 _]
              frame "Start Task 1", Default {
                # "Stays in Task 5D until the object is detected"
                n660 = Or(x=w1914, y=w1916) -> (x .or. y?=w1911:bool)
                n661 = case shown="False" w1911 {
                  tunnel: [w1924 w1930] -> w1912
                  tunnel: w1913 -> [w1922 w1929]
                  frame False {
                    n662 = for {
                      tunnel: string[] ["Z STEPPER CAM HEIGHT", "READ STEPPER VALUES"] ("element") -> [w1925] mode=indexing
                      shift-right: [w1927] -> w1924
                      shift-left: w1922 -> [w1926]
                      n663 = Enqueue Element(queue=w1926, element=w1925) -> (queue out=w1927:refnum<queue>)  [unwired: 2 in, 2 out]
                    }
                  }
                  frame True {
                    n664 = for {
                      shift-right: [w1932] -> w1930
                      shift-left: w1929 -> [w1933]
                      tunnel: string[] ["OPEN LOG CAM", "SET TIMER 2", "OPEN IMAQ REF", "", ""] -> [w1931] mode=indexing
                      n665 = Enqueue Element(queue=w1933, element=w1931) -> (queue out=w1932:refnum<queue>)  [unwired: 2 in, 2 out]
                    }
                  }
                }
                n666 = Select(t=State_Type_Definitions,_for_0.26g_versions_and_later_3."True Stop" ("Enum"), s=w1916, f=State_Type_Definitions,_for_0.26g_versions_and_later_3."Task 6N: CAM BURST 4" ("Enum")) -> (s? t:f=w1917:T18)
                n667 = Select(t=w1917, s=w1911, f=State_Type_Definitions,_for_0.26g_versions_and_later_3."Task 6M: STILL WAITING 3" ("Enum")) -> (s? t:f=w1919:T18)
              }
              frame "Exit" {
                n668 = for {
                  shift-right: [w1940] -> w1937
                  shift-left: w1934 -> [w1941]
                  tunnel: string[] ["STOP", "RESET ENCODERS", "RESET YAW", "ARDUINO MODE 0"] -> [w1939] mode=indexing
                  n669 = Enqueue Element(queue=w1941, element=w1939) -> (queue out=w1940:refnum<queue>)  [unwired: 2 in, 2 out]
                }
              }
            }
          }
          frame "Task 6N: CAM BURST 4" {
            # ">> Manual override >>"
            # ">>> Motor control cluster >>>"
            # ">>> yStepper command>>>"
            n670 = Dequeue Element(queue=w1953, timeout in ms (-1)=w1951, error in (no error)=w1952) -> (element=w1950:T10)  [unwired: 3 out]
            n671 = case shown="\"Start Task 1\", Default" w1950 {
              tunnel: [w1961 State_Type_Definitions,_for_0.26g_versions_and_later_3."True Stop" ("Enum")] -> w1947
              tunnel: [w1959 w1979] -> w1954
              tunnel: [State_Type_Definitions,_for_0.26g_versions_and_later_3."Idle" ("Enum") State_Type_Definitions,_for_0.26g_versions_and_later_3."Shutdown" ("Enum")] -> w1948
              tunnel: w1949 -> [w1957 _]
              tunnel: w1946 -> [w1958 w1976]
              tunnel: w1942 -> [w1955 _]
              frame "Start Task 1", Default {
                n672 = Or(x=w1955, y=w1957) -> (x .or. y?=w1956:bool)
                n673 = case shown="True" w1956 {
                  tunnel: [w1966 w1972] -> w1959
                  tunnel: w1958 -> [w1964 w1970]
                  frame False {
                    n674 = for {
                      tunnel: string[] ["CAM ACQ", "START TIMER"] ("element") -> [w1967] mode=indexing
                      shift-right: [w1969] -> w1966
                      shift-left: w1964 -> [w1968]
                      n675 = Enqueue Element(queue=w1968, element=w1967) -> (queue out=w1969:refnum<queue>)  [unwired: 2 in, 2 out]
                    }
                  }
                  frame True {
                    n676 = for {
                      shift-right: [w1974] -> w1972
                      shift-left: w1970 -> [w1975]
                      tunnel: string[] ["CAM CLOSE", "PROCESS IMAGE", "SET TIMER 2", "RESET ENCODERS"] -> [w1973] mode=indexing
                      n677 = Enqueue Element(queue=w1975, element=w1973) -> (queue out=w1974:refnum<queue>)  [unwired: 2 in, 2 out]
                    }
                  }
                }
                n678 = Select(t=State_Type_Definitions,_for_0.26g_versions_and_later_3."Task 6O: PROCESS IMAGE 4" ("Enum"), s=w1956, f=State_Type_Definitions,_for_0.26g_versions_and_later_3."Task 6N: CAM BURST 4" ("Enum")) -> (s? t:f=w1961:T18)
              }
              frame "Exit" {
                # ">> State after true stop >>"
                # ">> Goes to true stop >>"
                n679 = for {
                  shift-right: [w1982] -> w1979
                  shift-left: w1976 -> [w1983]
                  tunnel: string[] ["STOP", "RESET ENCODERS", "RESET YAW", ""] -> [w1981] mode=indexing
                  n680 = Enqueue Element(queue=w1983, element=w1981) -> (queue out=w1982:refnum<queue>)  [unwired: 2 in, 2 out]
                }
              }
            }
          }
          frame "Task 6O: PROCESS IMAGE 4" {
            # "Ball > Soap > Gel > Pipe"
            # ">>> Motor control cluster >>>"
            # ">>> yStepper command>>>"
            n681 = Dequeue Element(queue=w1992, timeout in ms (-1)=w1991, error in (no error)=w1990) -> (element=w1989:T10)  [unwired: 3 out]
            n682 = case shown="\"Start Task 1\", Default" w1989 {
              tunnel: [w2008 State_Type_Definitions,_for_0.26g_versions_and_later_3."True Stop" ("Enum")] -> w1996
              tunnel: [w2010 w2027] -> w1995
              tunnel: [State_Type_Definitions,_for_0.26g_versions_and_later_3."Idle" ("Enum") State_Type_Definitions,_for_0.26g_versions_and_later_3."Shutdown" ("Enum")] -> w1997
              tunnel: w1993 -> [w1999 _]
              tunnel: w1994 -> [w2005 w2024]
              tunnel: w1985 -> [w2003 _]
              tunnel: w1984 -> [w2004 _]
              frame "Start Task 1", Default {
                # "Stays in Task 5D until the object is detected"
                n683 = Or(x=w2003, y=w1999) -> (x .or. y?=w2002:bool)
                n684 = case shown="True" w2002 {
                  tunnel: [w2014 w2020] -> w2010
                  tunnel: w2005 -> [w2012 w2018]
                  frame False {
                    n685 = for {
                      tunnel: string[] ["START TIMER", "PROCESS IMAGE", ""] ("element") -> [w2015] mode=indexing
                      shift-right: [w2017] -> w2014
                      shift-left: w2012 -> [w2016]
                      n686 = Enqueue Element(queue=w2016, element=w2015) -> (queue out=w2017:refnum<queue>)  [unwired: 2 in, 2 out]
                    }
                  }
                  frame True {
                    n687 = for {
                      shift-right: [w2022] -> w2020
                      shift-left: w2018 -> [w2023]
                      tunnel: string[] ["RESET ENCODERS", "RESET YAW", ""] -> [w2021] mode=indexing
                      n688 = Enqueue Element(queue=w2023, element=w2021) -> (queue out=w2022:refnum<queue>)  [unwired: 2 in, 2 out]
                    }
                  }
                }
                n689 = Select(t=State_Type_Definitions,_for_0.26g_versions_and_later_3."Task 6P: PIPE BOMB" ("Enum"), s=w2004, f=State_Type_Definitions,_for_0.26g_versions_and_later_3."Task 6B: CAM BURST" ("Enum")) -> (s? t:f=w2000:T18)
                n690 = Select(t=State_Type_Definitions,_for_0.26g_versions_and_later_3."True Stop" ("Enum"), s=w1999, f=w2000) -> (s? t:f=w2006:T18)
                n691 = Select(t=w2006, s=w2002, f=State_Type_Definitions,_for_0.26g_versions_and_later_3."Task 6O: PROCESS IMAGE 4" ("Enum")) -> (s? t:f=w2008:T18)
              }
              frame "Exit" {
                n692 = for {
                  shift-right: [w2030] -> w2027
                  shift-left: w2024 -> [w2031]
                  tunnel: string[] ["STOP", "RESET ENCODERS", "RESET YAW", "ARDUINO MODE 0"] -> [w2029] mode=indexing
                  n693 = Enqueue Element(queue=w2031, element=w2029) -> (queue out=w2030:refnum<queue>)  [unwired: 2 in, 2 out]
                }
              }
            }
          }
          frame "Task 6P: PIPE BOMB" {
            # "Ball > Soap > Gel > Pipe"
            # ">>> Motor control cluster >>>"
            # ">>> yStepper command>>>"
            n694 = Greater Or Equal?(x=w2032, y=20.0) -> (x >= y?=w2033:bool)
            n695 = Dequeue Element(queue=w2041, timeout in ms (-1)=w2040, error in (no error)=w2039) -> (element=w2038:T10)  [unwired: 3 out]
            n696 = case shown="\"Start Task 1\", Default" w2038 {
              tunnel: [w2054 State_Type_Definitions,_for_0.26g_versions_and_later_3."True Stop" ("Enum")] -> w2045
              tunnel: [w2056 w2073] -> w2044
              tunnel: [State_Type_Definitions,_for_0.26g_versions_and_later_3."Idle" ("Enum") State_Type_Definitions,_for_0.26g_versions_and_later_3."Shutdown" ("Enum")] -> w2046
              tunnel: w2042 -> [w2049 _]
              tunnel: w2043 -> [w2051 w2070]
              tunnel: w2033 -> [w2048 _]
              frame "Start Task 1", Default {
                # "Stays in Task 5D until the object is detected"
                n697 = Or(x=w2048, y=w2049) -> (x .or. y?=w2050:bool)
                n698 = case shown="False" w2050 {
                  tunnel: [w2060 w2066] -> w2056
                  tunnel: w2051 -> [w2058 w2064]
                  frame False {
                    n699 = for {
                      tunnel: string[] ["FORWARD", "READ NAVX", "READ ENCODERS"] ("element") -> [w2061] mode=indexing
                      shift-right: [w2063] -> w2060
                      shift-left: w2058 -> [w2062]
                      n700 = Enqueue Element(queue=w2062, element=w2061) -> (queue out=w2063:refnum<queue>)  [unwired: 2 in, 2 out]
                    }
                  }
                  frame True {
                    n701 = for {
                      shift-right: [w2068] -> w2066
                      shift-left: w2064 -> [w2069]
                      tunnel: string[] ["RESET ENCODERS", "RESET YAW", "RESET FLAGS"] -> [w2067] mode=indexing
                      n702 = Enqueue Element(queue=w2069, element=w2067) -> (queue out=w2068:refnum<queue>)  [unwired: 2 in, 2 out]
                    }
                  }
                }
                n703 = Select(t=State_Type_Definitions,_for_0.26g_versions_and_later_3."True Stop" ("Enum"), s=w2049, f=State_Type_Definitions,_for_0.26g_versions_and_later_3."Task 5F: ARM GRAB HEIGHT" ("Enum")) -> (s? t:f=w2052:T18)
                n704 = Select(t=w2052, s=w2050, f=State_Type_Definitions,_for_0.26g_versions_and_later_3."Task 6P: PIPE BOMB" ("Enum")) -> (s? t:f=w2054:T18)
              }
              frame "Exit" {
                n705 = for {
                  shift-right: [w2076] -> w2073
                  shift-left: w2070 -> [w2077]
                  tunnel: string[] ["STOP", "RESET ENCODERS", "RESET YAW", "ARDUINO MODE 0"] -> [w2075] mode=indexing
                  n706 = Enqueue Element(queue=w2077, element=w2075) -> (queue out=w2076:refnum<queue>)  [unwired: 2 in, 2 out]
                }
              }
            }
          }
          frame "Task 7" {
          }
          frame "Task 8A: RAISE ARM" {
            # ">>> Motor control cluster >>>"
            # ">>> yStepper command>>>"
            # ">> Manual override >>"
            n707 = Dequeue Element(queue=w2094, timeout in ms (-1)=w2093, error in (no error)=w2095) -> (element=w2092:T10)  [unwired: 3 out]
            n708 = Equal?(x=w2091, y=u8 60) -> (x = y?=w2089:bool)
            n709 = case shown="\"Start Task 1\", Default" w2092 {
              tunnel: [w2105 State_Type_Definitions,_for_0.26g_versions_and_later_3."True Stop" ("Enum")] -> w2096
              tunnel: [w2108 w2125] -> w2097
              tunnel: [State_Type_Definitions,_for_0.26g_versions_and_later_3."Idle" ("Enum") State_Type_Definitions,_for_0.26g_versions_and_later_3."Shutdown" ("Enum")] -> w2098
              tunnel: w2089 -> [w2104 _]
              tunnel: w2088 -> [w2103 _]
              tunnel: w2087 -> [w2099 w2122]
              frame "Start Task 1", Default {
                # "Stays in Task 5_A until stepper reaches desired \nheight"
                # "T: Go back to idle, F: Continue with task\""
                # ">> Manual override >>"
                n710 = case shown="False" w2104 {
                  tunnel: [w2112 w2118] -> w2108
                  tunnel: w2099 -> [w2110 w2116]
                  frame False {
                    n711 = for {
                      tunnel: string[] ["Z STEPPER CAM HEIGHT", "READ STEPPER VALUES", "READ IR"] ("element") -> [w2113] mode=indexing
                      shift-right: [w2115] -> w2112
                      shift-left: w2110 -> [w2114]
                      n712 = Enqueue Element(queue=w2114, element=w2113) -> (queue out=w2115:refnum<queue>)  [unwired: 2 in, 2 out]
                    }
                  }
                  frame True {
                    n713 = for {
                      shift-right: [w2120] -> w2118
                      shift-left: w2116 -> [w2121]
                      tunnel: string[] ["RESET YAW", "RESET ENCODERS", "READ IR"] -> [w2119] mode=indexing
                      n714 = Enqueue Element(queue=w2121, element=w2119) -> (queue out=w2120:refnum<queue>)  [unwired: 2 in, 2 out]
                    }
                  }
                }
                n715 = Or(x=w2104, y=w2103) -> (x .or. y?=w2106:bool)
                n716 = Select(t=State_Type_Definitions,_for_0.26g_versions_and_later_3."True Stop" ("Enum"), s=w2103, f=State_Type_Definitions,_for_0.26g_versions_and_later_3."Task 8B: MOVE TO BOX" ("Enum")) -> (s? t:f=w2100:T18)
                n717 = Select(t=w2100, s=w2106, f=State_Type_Definitions,_for_0.26g_versions_and_later_3."Task 8A: RAISE ARM" ("Enum")) -> (s? t:f=w2105:T18)
              }
              frame "Exit" {
                n718 = for {
                  shift-right: [w2128] -> w2125
                  shift-left: w2122 -> [w2129]
                  tunnel: string[] ["STOP", "RESET ENCODERS", "RESET YAW", "ARDUINO MODE 0"] -> [w2127] mode=indexing
                  n719 = Enqueue Element(queue=w2129, element=w2127) -> (queue out=w2128:refnum<queue>)  [unwired: 2 in, 2 out]
                }
              }
            }
          }
          frame "Task 8B: MOVE TO BOX" {
            w2139 = u8 15 ("y")
            # "High voltage: 70"
            # ">>> yStepper command>>>"
            n720 = Less?(x=w2136, y=w2139) -> (x < y?=w2137:bool)
            n721 = Less?(x=w2135, y=w2139) -> (x < y?=w2138:bool)
            n722 = And(x=w2138, y=w2137) -> ()  [unwired: 1 out]
            n723 = Dequeue Element(queue=w2143, timeout in ms (-1)=w2142, error in (no error)=w2144) -> (element=w2141:T10)  [unwired: 3 out]
            n724 = Less?(x=w2132, y=40.0) -> (x < y?=w2130:bool)
            n725 = case shown="\"Start Task 1\", Default" w2141 {
              tunnel: [w2156 State_Type_Definitions,_for_0.26g_versions_and_later_3."True Stop" ("Enum")] -> w2146
              tunnel: [w2159 w2176] -> w2145
              tunnel: [State_Type_Definitions,_for_0.26g_versions_and_later_3."Idle" ("Enum") State_Type_Definitions,_for_0.26g_versions_and_later_3."Shutdown" ("Enum")] -> w2147
              tunnel: w2149 -> [w2155 _]
              tunnel: w2148 -> [w2151 w2173]
              tunnel: w2130 -> [w2150 _]
              frame "Start Task 1", Default {
                # "Stays in Task 5_B to capture image over 5 seconds"
                # "T: Go back to idle, F: Continue with task\""
                # ">> Manual override >>"
                n726 = case shown="True" w2150 {
                  tunnel: [w2163 w2169] -> w2159
                  tunnel: w2151 -> [w2161 w2167]
                  frame False {
                    n727 = for {
                      tunnel: string[] ["FORWARD", "READ IR", "READ NAVX"] ("element") -> [w2164] mode=indexing
                      shift-right: [w2166] -> w2163
                      shift-left: w2161 -> [w2165]
                      n728 = Enqueue Element(queue=w2165, element=w2164) -> (queue out=w2166:refnum<queue>)  [unwired: 2 in, 2 out]
                    }
                  }
                  frame True {
                    n729 = for {
                      shift-right: [w2171] -> w2169
                      shift-left: w2167 -> [w2172]
                      tunnel: string[] ["STOP", "RESET ENCODERS", "OPEN LOG CAM", "SET TIMER 2", "OPEN IMAQ REF"] -> [w2170] mode=indexing
                      n730 = Enqueue Element(queue=w2172, element=w2170) -> (queue out=w2171:refnum<queue>)  [unwired: 2 in, 2 out]
                    }
                  }
                }
                n731 = Or(x=w2150, y=w2155) -> (x .or. y?=w2157:bool)
                n732 = Select(t=State_Type_Definitions,_for_0.26g_versions_and_later_3."True Stop" ("Enum"), s=w2155, f=State_Type_Definitions,_for_0.26g_versions_and_later_3."Task 8C: CAM BURST" ("Enum")) -> (s? t:f=w2152:T18)
                n733 = Select(t=w2152, s=w2157, f=State_Type_Definitions,_for_0.26g_versions_and_later_3."Task 8B: MOVE TO BOX" ("Enum")) -> (s? t:f=w2156:T18)
              }
              frame "Exit" {
                n734 = for {
                  shift-right: [w2179] -> w2176
                  shift-left: w2173 -> [w2180]
                  tunnel: string[] ["STOP", "RESET ENCODERS", "RESET YAW", "ARDUINO MODE 0"] -> [w2178] mode=indexing
                  n735 = Enqueue Element(queue=w2180, element=w2178) -> (queue out=w2179:refnum<queue>)  [unwired: 2 in, 2 out]
                }
              }
            }
          }
          frame "Task 8C: CAM BURST" {
            # ">>> Motor control cluster >>>"
            # ">>> yStepper command>>>"
            # ">> Manual override >>"
            n736 = Dequeue Element(queue=w2191, timeout in ms (-1)=w2190, error in (no error)=w2189) -> (element=w2188:T10)  [unwired: 3 out]
            n737 = case shown="\"Start Task 1\", Default" w2188 {
              tunnel: [w2200 State_Type_Definitions,_for_0.26g_versions_and_later_3."True Stop" ("Enum")] -> w2193
              tunnel: [w2203 w2220] -> w2186
              tunnel: [State_Type_Definitions,_for_0.26g_versions_and_later_3."Idle" ("Enum") State_Type_Definitions,_for_0.26g_versions_and_later_3."Shutdown" ("Enum")] -> w2185
              tunnel: w2187 -> [w2194 _]
              tunnel: w2192 -> [w2199 w2217]
              tunnel: w2183 -> [w2198 _]
              frame "Start Task 1", Default {
                # ">> Is time up? >>"
                # "Determines if object is in range to pick up"
                # ">> Manual override >>"
                n738 = case shown="True" w2198 {
                  tunnel: [w2207 w2213] -> w2203
                  tunnel: w2199 -> [w2205 w2211]
                  frame False {
                    n739 = for {
                      tunnel: string[] ["CAM ACQ", "START TIMER"] ("element") -> [w2208] mode=indexing
                      shift-right: [w2210] -> w2207
                      shift-left: w2205 -> [w2209]
                      n740 = Enqueue Element(queue=w2209, element=w2208) -> (queue out=w2210:refnum<queue>)  [unwired: 2 in, 2 out]
                    }
                  }
                  frame True {
                    n741 = for {
                      shift-right: [w2215] -> w2213
                      shift-left: w2211 -> [w2216]
                      tunnel: string[] ["CAM CLOSE", "PROCESS IMAGE", "SET TIMER 2"] -> [w2214] mode=indexing
                      n742 = Enqueue Element(queue=w2216, element=w2214) -> (queue out=w2215:refnum<queue>)  [unwired: 2 in, 2 out]
                    }
                  }
                }
                n743 = Or(x=w2198, y=w2194) -> (x .or. y?=w2201:bool)
                n744 = Select(t=State_Type_Definitions,_for_0.26g_versions_and_later_3."True Stop" ("Enum"), s=w2194, f=State_Type_Definitions,_for_0.26g_versions_and_later_3."Task 8D: PROCESS IMAGE" ("Enum")) -> (s? t:f=w2196:T18)
                n745 = Select(t=w2196, s=w2201, f=State_Type_Definitions,_for_0.26g_versions_and_later_3."Task 8C: CAM BURST" ("Enum")) -> (s? t:f=w2200:T18)
              }
              frame "Exit" {
                n746 = for {
                  shift-right: [w2223] -> w2220
                  shift-left: w2217 -> [w2224]
                  tunnel: string[] ["STOP", "RESET ENCODERS", "RESET YAW", "ARDUINO MODE 0"] -> [w2222] mode=indexing
                  n747 = Enqueue Element(queue=w2224, element=w2222) -> (queue out=w2223:refnum<queue>)  [unwired: 2 in, 2 out]
                }
              }
            }
          }
          frame "Task 8D: PROCESS IMAGE" {
            # ">>> Motor control cluster >>>"
            # ">>> yStepper command>>>"
            n748 = Dequeue Element(queue=w2233, timeout in ms (-1)=w2232, error in (no error)=w2231) -> (element=w2230:T10)  [unwired: 3 out]
            n749 = case shown="\"Start Task 1\", Default" w2230 {
              tunnel: [w2248 State_Type_Definitions,_for_0.26g_versions_and_later_3."True Stop" ("Enum")] -> w2237
              tunnel: [w2251 w2268] -> w2236
              tunnel: [State_Type_Definitions,_for_0.26g_versions_and_later_3."Idle" ("Enum") State_Type_Definitions,_for_0.26g_versions_and_later_3."Shutdown" ("Enum")] -> w2238
              tunnel: w2234 -> [w2247 _]
              tunnel: w2235 -> [w2244 w2265]
              tunnel: w2225 -> [w2243 _]
              tunnel: w2226 -> [w2242 _]
              frame "Start Task 1", Default {
                # ">> T: Breaks out of state loop; F: Stays in loop>>"
                # ">> Manual override >>"
                # ">> Checks if time is up>>"
                # "Stays in Task 5D until the object is detected"
                # "T: Go back to idle, F: Continue with task\""
                # ">> Manual override >>"
                n750 = case shown="False" w2243 {
                  tunnel: [w2255 w2261] -> w2251
                  tunnel: w2244 -> [w2253 w2259]
                  frame False {
                    n751 = for {
                      tunnel: string[] ["START TIMER", "PROCESS IMAGE", ""] ("element") -> [w2256] mode=indexing
                      shift-right: [w2258] -> w2255
                      shift-left: w2253 -> [w2257]
                      n752 = Enqueue Element(queue=w2257, element=w2256) -> (queue out=w2258:refnum<queue>)  [unwired: 2 in, 2 out]
                    }
                  }
                  frame True {
                    n753 = for {
                      shift-right: [w2263] -> w2261
                      shift-left: w2259 -> [w2264]
                      tunnel: string[] ["RESET ENCODERS", "", ""] -> [w2262] mode=indexing
                      n754 = Enqueue Element(queue=w2264, element=w2262) -> (queue out=w2263:refnum<queue>)  [unwired: 2 in, 2 out]
                    }
                  }
                }
                n755 = Or(x=w2243, y=w2247) -> (x .or. y?=w2249:bool)
                n756 = Select(t=State_Type_Definitions,_for_0.26g_versions_and_later_3."Task 8E: ROBOT ADJUST" ("Enum"), s=w2242, f=State_Type_Definitions,_for_0.26g_versions_and_later_3."True Stop" ("Enum")) -> (s? t:f=w2239:T18)
                n757 = Select(t=State_Type_Definitions,_for_0.26g_versions_and_later_3."True Stop" ("Enum"), s=w2247, f=w2239) -> (s? t:f=w2245:T18)
                n758 = Select(t=w2245, s=w2249, f=State_Type_Definitions,_for_0.26g_versions_and_later_3."Task 8D: PROCESS IMAGE" ("Enum")) -> (s? t:f=w2248:T18)
              }
              frame "Exit" {
                n759 = for {
                  shift-right: [w2271] -> w2268
                  shift-left: w2265 -> [w2272]
                  tunnel: string[] ["STOP", "RESET ENCODERS", "RESET YAW", "ARDUINO MODE 0"] -> [w2270] mode=indexing
                  n760 = Enqueue Element(queue=w2272, element=w2270) -> (queue out=w2271:refnum<queue>)  [unwired: 2 in, 2 out]
                }
              }
            }
          }
          frame "Task 8E: ROBOT ADJUST" {
            # ">>> Motor control cluster >>>"
            # ">>> yStepper command>>>"
            n761 = Dequeue Element(queue=w2289, timeout in ms (-1)=w2288, error in (no error)=w2287) -> (element=w2286:T10)  [unwired: 3 out]
            n762 = Subtract(x=w2284, y=150.0) -> (x-y=w2282:dbl)
            n763 = formula code="if (error >= -100 && error < -80){\n    distance = -25;\n    xSpeed = -30;\n}\n\nelse if (error >= -80 && error < -60){\n    distance = -20;\n    xSpeed = -30;\n}\n\nelse if (error >= -60 && error < -40){\n    distance = -15;\n    xSpeed = -30;\n}\n\nelse if (error >= -40 && error < -20){\n    distance = -10;\n    xSpeed = -30;\n}\n\nelse if (error >= -20 && error < -10){\n    distance = 5;\n    xSpeed = -30;\n}\n\nelse if (error >= -10 && error <= 10){\n    distance = 0;\n    xSpeed = 0;\n}\n\nelse if (error >= 20 && error < 40){\n    distance = 5;\n    xSpeed = 30;\n}\n\nelse if (error >= 40 && error < 60){\n    distance = 10;\n    xSpeed = 30;\n}\n\nelse if (error >= 60 && error < 80){\n    distance = 15;\n    xSpeed = 30;\n}\n\nelse if (error >= 80 && error < 100){\n    distance = 20;\n    xSpeed = 30;\n}\n\nelse if (error >= 100){\n    distance = 25;\n    xSpeed = 30;\n}\n\nelse {\n    distance = 0;\n    xSpeed = 0;\n}"("error"=w2282) -> ("distance"=w2277:dbl, "xSpeed"=w2279:dbl)
            "Distance to move" <- w2277
            n764 = formula code="if (target > 0){\nif (current  >= target)\noutput = 1;\n\nelse if (current != target)\noutput = 0;\n}\n\nelse if (target == 0){\nif (current == target)\noutput = 1;\n\nelse if (current != target)\noutput = 0;\n}\n\nelse if (target < 0){\nif (current <= target)\noutput = 1;\n\nelse if (current != target)\noutput = 0;\n}\n\nelse if (current != target)\noutput = 0;"("target"=w2277, "current"=w2278) -> ("output"=w2276:dbl)
            n765 = Bundle By Name(cluster=w2281, "xSpeed"=w2279) -> (w2280:T19)
            n766 = Equal?(x=w2276, y=1.0) -> (x = y?=w2273:bool)
            n767 = case shown="\"Start Task 1\", Default" w2286 {
              tunnel: [w2301 State_Type_Definitions,_for_0.26g_versions_and_later_3."True Stop" ("Enum")] -> w2293
              tunnel: [w2304 w2321] -> w2292
              tunnel: [State_Type_Definitions,_for_0.26g_versions_and_later_3."Idle" ("Enum") State_Type_Definitions,_for_0.26g_versions_and_later_3."Shutdown" ("Enum")] -> w2294
              tunnel: w2290 -> [w2300 _]
              tunnel: w2291 -> [w2296 w2318]
              tunnel: w2273 -> [w2295 _]
              frame "Start Task 1", Default {
                # ">> T: Breaks out of state loop; F: Stays in loop>>"
                # ">> Manual override >>"
                # ">> Checks if time is up>>"
                # "Stays in Task 5D until the object is detected"
                # "T: Go back to idle, F: Continue with task\""
                # ">> Manual override >>"
                n768 = case shown="True" w2295 {
                  tunnel: [w2308 w2314] -> w2304
                  tunnel: w2296 -> [w2306 w2312]
                  frame False {
                    n769 = for {
                      tunnel: string[] ["X AXIS - SLOW", "READ ENCODERS", "READ NAVX"] ("element") -> [w2309] mode=indexing
                      shift-right: [w2311] -> w2308
                      shift-left: w2306 -> [w2310]
                      n770 = Enqueue Element(queue=w2310, element=w2309) -> (queue out=w2311:refnum<queue>)  [unwired: 2 in, 2 out]
                    }
                  }
                  frame True {
                    n771 = for {
                      shift-right: [w2316] -> w2314
                      shift-left: w2312 -> [w2317]
                      tunnel: string[] ["SET TIMER 2", "STOP", "READ STEPPER VALUES", ""] -> [w2315] mode=indexing
                      n772 = Enqueue Element(queue=w2317, element=w2315) -> (queue out=w2316:refnum<queue>)  [unwired: 2 in, 2 out]
                    }
                  }
                }
                n773 = Or(x=w2295, y=w2300) -> (x .or. y?=w2302:bool)
                n774 = Select(t=State_Type_Definitions,_for_0.26g_versions_and_later_3."True Stop" ("Enum"), s=w2300, f=State_Type_Definitions,_for_0.26g_versions_and_later_3."Task 8H: ARM ADJUST" ("Enum")) -> (s? t:f=w2297:T18)
                n775 = Select(t=w2297, s=w2302, f=State_Type_Definitions,_for_0.26g_versions_and_later_3."Task 8E: ROBOT ADJUST" ("Enum")) -> (s? t:f=w2301:T18)
              }
              frame "Exit" {
                n776 = for {
                  shift-right: [w2324] -> w2321
                  shift-left: w2318 -> [w2325]
                  tunnel: string[] ["STOP", "RESET ENCODERS", "RESET YAW", "ARDUINO MODE 0"] -> [w2323] mode=indexing
                  n777 = Enqueue Element(queue=w2325, element=w2323) -> (queue out=w2324:refnum<queue>)  [unwired: 2 in, 2 out]
                }
              }
            }
          }
          frame "Task 8F: CAM BURST 2" {
            # ">>> Motor control cluster >>>"
            # ">>> yStepper command>>>"
            # ">> Manual override >>"
            n778 = Dequeue Element(queue=w2336, timeout in ms (-1)=w2335, error in (no error)=w2334) -> (element=w2333:T10)  [unwired: 3 out]
            n779 = case shown="\"Start Task 1\", Default" w2333 {
              tunnel: [w2345 State_Type_Definitions,_for_0.26g_versions_and_later_3."True Stop" ("Enum")] -> w2338
              tunnel: [w2348 w2365] -> w2331
              tunnel: [State_Type_Definitions,_for_0.26g_versions_and_later_3."Idle" ("Enum") State_Type_Definitions,_for_0.26g_versions_and_later_3."Shutdown" ("Enum")] -> w2330
              tunnel: w2332 -> [w2339 _]
              tunnel: w2337 -> [w2344 w2362]
              tunnel: w2328 -> [w2343 _]
              frame "Start Task 1", Default {
                # ">> Is time up? >>"
                # "Determines if object is in range to pick up"
                # ">> Manual override >>"
                n780 = case shown="False" w2343 {
                  tunnel: [w2352 w2358] -> w2348
                  tunnel: w2344 -> [w2350 w2356]
                  frame False {
                    n781 = for {
                      tunnel: string[] ["CAM ACQ", "START TIMER"] ("element") -> [w2353] mode=indexing
                      shift-right: [w2355] -> w2352
                      shift-left: w2350 -> [w2354]
                      n782 = Enqueue Element(queue=w2354, element=w2353) -> (queue out=w2355:refnum<queue>)  [unwired: 2 in, 2 out]
                    }
                  }
                  frame True {
                    n783 = for {
                      shift-right: [w2360] -> w2358
                      shift-left: w2356 -> [w2361]
                      tunnel: string[] ["CAM CLOSE", "PROCESS IMAGE", "SET TIMER 3"] -> [w2359] mode=indexing
                      n784 = Enqueue Element(queue=w2361, element=w2359) -> (queue out=w2360:refnum<queue>)  [unwired: 2 in, 2 out]
                    }
                  }
                }
                n785 = Or(x=w2343, y=w2339) -> (x .or. y?=w2346:bool)
                n786 = Select(t=State_Type_Definitions,_for_0.26g_versions_and_later_3."True Stop" ("Enum"), s=w2339, f=State_Type_Definitions,_for_0.26g_versions_and_later_3."Task 8G: PROCESS IMAGE 2" ("Enum")) -> (s? t:f=w2341:T18)
                n787 = Select(t=w2341, s=w2346, f=State_Type_Definitions,_for_0.26g_versions_and_later_3."Task 8F: CAM BURST 2" ("Enum")) -> (s? t:f=w2345:T18)
              }
              frame "Exit" {
                n788 = for {
                  shift-right: [w2368] -> w2365
                  shift-left: w2362 -> [w2369]
                  tunnel: string[] ["STOP", "RESET ENCODERS", "RESET YAW", "ARDUINO MODE 0"] -> [w2367] mode=indexing
                  n789 = Enqueue Element(queue=w2369, element=w2367) -> (queue out=w2368:refnum<queue>)  [unwired: 2 in, 2 out]
                }
              }
            }
          }
          frame "Task 8G: PROCESS IMAGE 2" {
            # ">>> yStepper command>>>"
            n790 = Dequeue Element(queue=w2377, timeout in ms (-1)=w2376, error in (no error)=w2375) -> (element=w2374:T10)  [unwired: 3 out]
            n791 = case shown="\"Start Task 1\", Default" w2374 {
              tunnel: [w2389 State_Type_Definitions,_for_0.26g_versions_and_later_3."True Stop" ("Enum")] -> w2381
              tunnel: [w2392 w2409] -> w2380
              tunnel: [State_Type_Definitions,_for_0.26g_versions_and_later_3."Idle" ("Enum") State_Type_Definitions,_for_0.26g_versions_and_later_3."Shutdown" ("Enum")] -> w2382
              tunnel: w2378 -> [w2388 _]
              tunnel: w2379 -> [w2384 w2406]
              tunnel: w2372 -> [w2383 _]
              frame "Start Task 1", Default {
                # ">> T: Breaks out of state loop; F: Stays in loop>>"
                # ">> Manual override >>"
                # ">> Checks if time is up>>"
                # "Stays in Task 5D until the object is detected"
                # "T: Go back to idle, F: Continue with task\""
                # ">> Manual override >>"
                n792 = case shown="False" w2383 {
                  tunnel: [w2396 w2402] -> w2392
                  tunnel: w2384 -> [w2394 w2400]
                  frame False {
                    n793 = for {
                      tunnel: string[] ["START TIMER", "PROCESS IMAGE", ""] ("element") -> [w2397] mode=indexing
                      shift-right: [w2399] -> w2396
                      shift-left: w2394 -> [w2398]
                      n794 = Enqueue Element(queue=w2398, element=w2397) -> (queue out=w2399:refnum<queue>)  [unwired: 2 in, 2 out]
                    }
                  }
                  frame True {
                    n795 = for {
                      shift-right: [w2404] -> w2402
                      shift-left: w2400 -> [w2405]
                      tunnel: string[] ["READ STEPPER VALUES", "Y STEPPER CONTROL", ""] -> [w2403] mode=indexing
                      n796 = Enqueue Element(queue=w2405, element=w2403) -> (queue out=w2404:refnum<queue>)  [unwired: 2 in, 2 out]
                    }
                  }
                }
                n797 = Or(x=w2383, y=w2388) -> (x .or. y?=w2390:bool)
                n798 = Select(t=State_Type_Definitions,_for_0.26g_versions_and_later_3."True Stop" ("Enum"), s=w2388, f=State_Type_Definitions,_for_0.26g_versions_and_later_3."Task 8H: ARM ADJUST" ("Enum")) -> (s? t:f=w2385:T18)
                n799 = Select(t=w2385, s=w2390, f=State_Type_Definitions,_for_0.26g_versions_and_later_3."Task 8G: PROCESS IMAGE 2" ("Enum")) -> (s? t:f=w2389:T18)
              }
              frame "Exit" {
                n800 = for {
                  shift-right: [w2412] -> w2409
                  shift-left: w2406 -> [w2413]
                  tunnel: string[] ["STOP", "RESET ENCODERS", "RESET YAW", "ARDUINO MODE 0"] -> [w2411] mode=indexing
                  n801 = Enqueue Element(queue=w2413, element=w2411) -> (queue out=w2412:refnum<queue>)  [unwired: 2 in, 2 out]
                }
              }
            }
          }
          frame "Task 8H: ARM ADJUST" {
            # ">>> yStepper command>>>"
            n802 = Dequeue Element(queue=w2427, timeout in ms (-1)=w2428, error in (no error)=w2429) -> (element=w2431:T10)  [unwired: 3 out]
            n803 = formula code="if (pos >= 50 && pos < 80)\ny = 40;\n\nelse if (pos >= 80 && pos < 100)\ny = 35;\n\nelse if (pos >= 100 && pos < 120)\ny = 20;\n\nelse if (pos >= 120 && pos < 140)\ny = 15;\n\nelse if (pos >= 140 && pos < 150)\ny = 10;\n\nelse if (pos >= 150 && 170)\ny = 5;\n\nelse \ny = 0;"("pos"=w2419) -> ("y"=w2422:dbl)
            n804 = To Unsigned Byte Integer(number=w2422) -> (unsigned 8bit integer=w2417:u8)
            n805 = Equal?(x=w2418, y=w2417) -> (x = y?=w2416:bool)
            n806 = case shown="\"Start Task 1\", Default" w2431 {
              tunnel: [w2438 State_Type_Definitions,_for_0.26g_versions_and_later_3."True Stop" ("Enum")] -> w2425
              tunnel: [w2441 w2458] -> w2423
              tunnel: [State_Type_Definitions,_for_0.26g_versions_and_later_3."Idle" ("Enum") State_Type_Definitions,_for_0.26g_versions_and_later_3."Shutdown" ("Enum")] -> w2424
              tunnel: w2430 -> [w2437 _]
              tunnel: w2426 -> [w2433 w2455]
              tunnel: w2416 -> [w2432 _]
              frame "Start Task 1", Default {
                # ">> T: Breaks out of state loop; F: Stays in loop>>"
                # ">> Manual override >>"
                # ">> Checks if time is up>>"
                # "Stays in Task 5D until the object is detected"
                # "T: Go back to idle, F: Continue with task\""
                # ">> Manual override >>"
                n807 = case shown="False" w2432 {
                  tunnel: [w2445 w2451] -> w2441
                  tunnel: w2433 -> [w2443 w2449]
                  frame False {
                    n808 = for {
                      tunnel: string[] ["READ STEPPER VALUES", "Y STEPPER CONTROL", ""] ("element") -> [w2446] mode=indexing
                      shift-right: [w2448] -> w2445
                      shift-left: w2443 -> [w2447]
                      n809 = Enqueue Element(queue=w2447, element=w2446) -> (queue out=w2448:refnum<queue>)  [unwired: 2 in, 2 out]
                    }
                  }
                  frame True {
                    n810 = for {
                      shift-right: [w2453] -> w2451
                      shift-left: w2449 -> [w2454]
                      tunnel: string[] ["DISPOSE BUFFERS", "READ STEPPER VALUES", ""] -> [w2452] mode=indexing
                      n811 = Enqueue Element(queue=w2454, element=w2452) -> (queue out=w2453:refnum<queue>)  [unwired: 2 in, 2 out]
                    }
                  }
                }
                n812 = Or(x=w2432, y=w2437) -> (x .or. y?=w2439:bool)
                n813 = Select(t=State_Type_Definitions,_for_0.26g_versions_and_later_3."True Stop" ("Enum"), s=w2437, f=State_Type_Definitions,_for_0.26g_versions_and_later_3."Task 8I: ARM GRAB HEIGHT" ("Enum")) -> (s? t:f=w2434:T18)
                n814 = Select(t=w2434, s=w2439, f=State_Type_Definitions,_for_0.26g_versions_and_later_3."Task 8H: ARM ADJUST" ("Enum")) -> (s? t:f=w2438:T18)
              }
              frame "Exit" {
                n815 = for {
                  shift-right: [w2461] -> w2458
                  shift-left: w2455 -> [w2462]
                  tunnel: string[] ["STOP", "RESET ENCODERS", "RESET YAW", "ARDUINO MODE 0"] -> [w2460] mode=indexing
                  n816 = Enqueue Element(queue=w2462, element=w2460) -> (queue out=w2461:refnum<queue>)  [unwired: 2 in, 2 out]
                }
              }
            }
            n817 = Bundle By Name(cluster=w2421, "yStepper desired"=w2417) -> (w2420:T20)
          }
          frame "Task 8I: ARM GRAB HEIGHT" {
            # ">>> Motor control cluster >>>"
            # ">>> yStepper command>>>"
            # ">> Manual override >>"
            n818 = Dequeue Element(queue=w2473, timeout in ms (-1)=w2472, error in (no error)=w2474) -> (element=w2471:T10)  [unwired: 3 out]
            n819 = Equal?(x=w2470, y=u8 1) -> (x = y?=w2468:bool)
            n820 = case shown="\"Start Task 1\", Default" w2471 {
              tunnel: [w2484 State_Type_Definitions,_for_0.26g_versions_and_later_3."True Stop" ("Enum")] -> w2475
              tunnel: [w2487 w2504] -> w2476
              tunnel: [State_Type_Definitions,_for_0.26g_versions_and_later_3."Idle" ("Enum") State_Type_Definitions,_for_0.26g_versions_and_later_3."Shutdown" ("Enum")] -> w2477
              tunnel: w2468 -> [w2483 _]
              tunnel: w2467 -> [w2482 _]
              tunnel: w2466 -> [w2478 w2501]
              frame "Start Task 1", Default {
                # "Stays in Task 5F until stepper reaches desired \nheight"
                # "T: Go back to idle, F: Continue with task\""
                # ">> Manual override >>"
                n821 = case shown="True" w2483 {
                  tunnel: [w2491 w2497] -> w2487
                  tunnel: w2478 -> [w2489 w2495]
                  frame False {
                    n822 = for {
                      tunnel: string[] ["Z STEPPER GRAB HEIGHT", "READ STEPPER VALUES"] ("element") -> [w2492] mode=indexing
                      shift-right: [w2494] -> w2491
                      shift-left: w2489 -> [w2493]
                      n823 = Enqueue Element(queue=w2493, element=w2492) -> (queue out=w2494:refnum<queue>)  [unwired: 2 in, 2 out]
                    }
                  }
                  frame True {
                    n824 = for {
                      shift-right: [w2499] -> w2497
                      shift-left: w2495 -> [w2500]
                      tunnel: string[] ["SET TIMER 2", "CLOSE CLAW", ""] -> [w2498] mode=indexing
                      n825 = Enqueue Element(queue=w2500, element=w2498) -> (queue out=w2499:refnum<queue>)  [unwired: 2 in, 2 out]
                    }
                  }
                }
                n826 = Or(x=w2483, y=w2482) -> (x .or. y?=w2485:bool)
                n827 = Select(t=State_Type_Definitions,_for_0.26g_versions_and_later_3."True Stop" ("Enum"), s=w2482, f=State_Type_Definitions,_for_0.26g_versions_and_later_3."Task 8J: CLOSE CLAW" ("Enum")) -> (s? t:f=w2479:T18)
                n828 = Select(t=w2479, s=w2485, f=State_Type_Definitions,_for_0.26g_versions_and_later_3."Task 8I: ARM GRAB HEIGHT" ("Enum")) -> (s? t:f=w2484:T18)
              }
              frame "Exit" {
                n829 = for {
                  shift-right: [w2507] -> w2504
                  shift-left: w2501 -> [w2508]
                  tunnel: string[] ["STOP", "RESET ENCODERS", "RESET YAW", "ARDUINO MODE 0"] -> [w2506] mode=indexing
                  n830 = Enqueue Element(queue=w2508, element=w2506) -> (queue out=w2507:refnum<queue>)  [unwired: 2 in, 2 out]
                }
              }
            }
          }
          frame "Task 8J: CLOSE CLAW" {
            # ">>> yStepper command>>>"
            # ">> Manual override >>"
            n831 = Dequeue Element(queue=w2519, timeout in ms (-1)=w2518, error in (no error)=w2517) -> (element=w2516:T10)  [unwired: 3 out]
            n832 = case shown="\"Start Task 1\", Default" w2516 {
              tunnel: [w2528 State_Type_Definitions,_for_0.26g_versions_and_later_3."True Stop" ("Enum")] -> w2521
              tunnel: [w2531 w2548] -> w2514
              tunnel: [State_Type_Definitions,_for_0.26g_versions_and_later_3."Idle" ("Enum") State_Type_Definitions,_for_0.26g_versions_and_later_3."Shutdown" ("Enum")] -> w2513
              tunnel: w2515 -> [w2522 _]
              tunnel: w2520 -> [w2527 w2545]
              tunnel: w2511 -> [w2526 _]
              frame "Start Task 1", Default {
                # ">> Is time up? >>"
                # "Determines if object is in range to pick up"
                # ">> Manual override >>"
                n833 = case shown="True" w2526 {
                  tunnel: [w2535 w2541] -> w2531
                  tunnel: w2527 -> [w2533 w2539]
                  frame False {
                    n834 = for {
                      tunnel: string[] ["CLOSE CLAW", "START TIMER"] ("element") -> [w2536] mode=indexing
                      shift-right: [w2538] -> w2535
                      shift-left: w2533 -> [w2537]
                      n835 = Enqueue Element(queue=w2537, element=w2536) -> (queue out=w2538:refnum<queue>)  [unwired: 2 in, 2 out]
                    }
                  }
                  frame True {
                    n836 = for {
                      shift-right: [w2543] -> w2541
                      shift-left: w2539 -> [w2544]
                      tunnel: string[] ["READ STEPPER VALUES", "", ""] -> [w2542] mode=indexing
                      n837 = Enqueue Element(queue=w2544, element=w2542) -> (queue out=w2543:refnum<queue>)  [unwired: 2 in, 2 out]
                    }
                  }
                }
                n838 = Or(x=w2526, y=w2522) -> (x .or. y?=w2529:bool)
                n839 = Select(t=State_Type_Definitions,_for_0.26g_versions_and_later_3."True Stop" ("Enum"), s=w2522, f=State_Type_Definitions,_for_0.26g_versions_and_later_3."Task 8K: RAISE MY SWORD" ("Enum")) -> (s? t:f=w2524:T18)
                n840 = Select(t=w2524, s=w2529, f=State_Type_Definitions,_for_0.26g_versions_and_later_3."Task 8J: CLOSE CLAW" ("Enum")) -> (s? t:f=w2528:T18)
              }
              frame "Exit" {
                n841 = for {
                  shift-right: [w2551] -> w2548
                  shift-left: w2545 -> [w2552]
                  tunnel: string[] ["STOP", "RESET ENCODERS", "RESET YAW", "ARDUINO MODE 0"] -> [w2550] mode=indexing
                  n842 = Enqueue Element(queue=w2552, element=w2550) -> (queue out=w2551:refnum<queue>)  [unwired: 2 in, 2 out]
                }
              }
            }
          }
          frame "Task 8K: RAISE MY SWORD" {
            # ">>> yStepper command>>>"
            # ">> Manual override >>"
            n843 = Dequeue Element(queue=w2563, timeout in ms (-1)=w2562, error in (no error)=w2564) -> (element=w2561:T10)  [unwired: 3 out]
            n844 = Equal?(x=w2560, y=u8 60) -> (x = y?=w2558:bool)
            n845 = case shown="\"Start Task 1\", Default" w2561 {
              tunnel: [w2574 State_Type_Definitions,_for_0.26g_versions_and_later_3."True Stop" ("Enum")] -> w2565
              tunnel: [w2577 w2594] -> w2566
              tunnel: [State_Type_Definitions,_for_0.26g_versions_and_later_3."Idle" ("Enum") State_Type_Definitions,_for_0.26g_versions_and_later_3."Shutdown" ("Enum")] -> w2567
              tunnel: w2558 -> [w2573 _]
              tunnel: w2557 -> [w2572 _]
              tunnel: w2556 -> [w2568 w2591]
              frame "Start Task 1", Default {
                # "Stays in Task 5_A until stepper reaches desired \nheight"
                # "T: Go back to idle, F: Continue with task\""
                # ">> Manual override >>"
                n846 = case shown="True" w2573 {
                  tunnel: [w2581 w2587] -> w2577
                  tunnel: w2568 -> [w2579 w2585]
                  frame False {
                    n847 = for {
                      tunnel: string[] ["Z STEPPER CAM HEIGHT", "READ STEPPER VALUES"] ("element") -> [w2582] mode=indexing
                      shift-right: [w2584] -> w2581
                      shift-left: w2579 -> [w2583]
                      n848 = Enqueue Element(queue=w2583, element=w2582) -> (queue out=w2584:refnum<queue>)  [unwired: 2 in, 2 out]
                    }
                  }
                  frame True {
                    n849 = for {
                      shift-right: [w2589] -> w2587
                      shift-left: w2585 -> [w2590]
                      tunnel: string[] ["CAM CLOSE", "DISPOSE CAM BUFFERS", "DISPOSE PROC BUFFERS", "RESET ENCODERS"] -> [w2588] mode=indexing
                      n850 = Enqueue Element(queue=w2590, element=w2588) -> (queue out=w2589:refnum<queue>)  [unwired: 2 in, 2 out]
                    }
                  }
                }
                n851 = Or(x=w2573, y=w2572) -> (x .or. y?=w2575:bool)
                n852 = Select(t=State_Type_Definitions,_for_0.26g_versions_and_later_3."True Stop" ("Enum"), s=w2572, f=State_Type_Definitions,_for_0.26g_versions_and_later_3."True Stop" ("Enum")) -> (s? t:f=w2569:T18)
                n853 = Select(t=w2569, s=w2575, f=State_Type_Definitions,_for_0.26g_versions_and_later_3."Task 8K: RAISE MY SWORD" ("Enum")) -> (s? t:f=w2574:T18)
              }
              frame "Exit" {
                n854 = for {
                  shift-right: [w2597] -> w2594
                  shift-left: w2591 -> [w2598]
                  tunnel: string[] ["STOP", "RESET ENCODERS", "RESET YAW", "ARDUINO MODE 0"] -> [w2596] mode=indexing
                  n855 = Enqueue Element(queue=w2598, element=w2596) -> (queue out=w2597:refnum<queue>)  [unwired: 2 in, 2 out]
                }
              }
            }
          }
          frame "Task 9A: Raise Arm" {
            # ">>> Motor control cluster >>>"
            # ">> Stepper height reeached >>"
            # ">>> yStepper command>>>"
            # ">> Manual override >>"
            n856 = Dequeue Element(queue=w2611, timeout in ms (-1)=w2606, error in (no error)=w2610) -> (element=w2613:T10)  [unwired: 3 out]
            n857 = Equal?(x=w2608, y=u8 50) -> (x = y?=w2599:bool)
            n858 = case shown="\"Start Task 1\", Default" w2613 {
              tunnel: [w2624 State_Type_Definitions,_for_0.26g_versions_and_later_3."True Stop" ("Enum")] -> w2604
              tunnel: [w2622 w2639] -> w2603
              tunnel: w2607 -> [w2621 _]
              tunnel: w2609 -> [w2615 _]
              tunnel: [State_Type_Definitions,_for_0.26g_versions_and_later_3."Idle" ("Enum") State_Type_Definitions,_for_0.26g_versions_and_later_3."Shutdown" ("Enum")] -> w2605
              tunnel: w2599 -> [w2614 _]
              frame "Start Task 1", Default {
                # ">> WIill proceed to part ii if not manual override >>"
                # ">>If ENABLE or Trigger is set to true>>"
                n859 = Or(x=w2614, y=w2615) -> (x .or. y?=w2616:bool)
                n860 = case shown="False" w2614 {
                  tunnel: [w2627 w2633] -> w2622
                  tunnel: w2621 -> [w2626 w2632]
                  frame False {
                    n861 = for {
                      shift-right: [w2629] -> w2627
                      shift-left: w2626 -> [w2630]
                      tunnel: string[] ["Z STEPPER BOX HEIGHT", "READ STEPPER VALUES"] ("element") -> [w2628] mode=indexing
                      n862 = Enqueue Element(queue=w2630, element=w2628) -> (queue out=w2629:refnum<queue>)  [unwired: 2 in, 2 out]
                    }
                  }
                  frame True {
                    n863 = for {
                      shift-right: [w2635] -> w2633
                      shift-left: w2632 -> [w2636]
                      tunnel: string[] ["READ NAVX", "RESET FLAGS", "RESET YAW", "", "", ""] -> [w2634] mode=indexing
                      n864 = Enqueue Element(queue=w2636, element=w2634) -> (queue out=w2635:refnum<queue>)  [unwired: 2 in, 2 out]
                    }
                  }
                }
                n865 = Select(t=State_Type_Definitions,_for_0.26g_versions_and_later_3."True Stop" ("Enum"), s=w2615, f=State_Type_Definitions,_for_0.26g_versions_and_later_3."Task 9B: Rotate to Angle" ("Enum")) -> (s? t:f=w2618:T18)
                n866 = Select(t=w2618, s=w2616, f=State_Type_Definitions,_for_0.26g_versions_and_later_3."Task 9A: Raise Arm" ("Enum")) -> (s? t:f=w2624:T18)
              }
              frame "Exit" {
                n867 = for {
                  shift-right: [w2642] -> w2639
                  shift-left: _ -> [w2643]
                  tunnel: string[] ["STOP", "RESET ENCODERS", "RESET YAW", ""] -> [w2641] mode=indexing
                  n868 = Enqueue Element(queue=w2643, element=w2641) -> (queue out=w2642:refnum<queue>)  [unwired: 2 in, 2 out]
                }
              }
            }
          }
          frame "Task 9B: Rotate to Angle" {
            # ">>> Motor control cluster >>>"
            # ">>> yStepper command>>>"
            n869 = Dequeue Element(queue=w2657, timeout in ms (-1)=w2656, error in (no error)=w2655) -> (element=w2659:T10)  [unwired: 3 out]
            n870 = In Range and Coerce(upper limit=65.0, x=w2649, lower limit=58.0) -> (In Range?=w2644:bool)  [unwired: 1 out]
            n871 = case shown="\"Start Task 1\", Default" w2659 {
              tunnel: w2650 -> [w2662 _]
              tunnel: [w2670 State_Type_Definitions,_for_0.26g_versions_and_later_3."True Stop" ("Enum")] -> w2652
              tunnel: w2658 -> [w2668 w2686]
              tunnel: [w2667 w2685] -> w2651
              tunnel: [State_Type_Definitions,_for_0.26g_versions_and_later_3."Idle" ("Enum") State_Type_Definitions,_for_0.26g_versions_and_later_3."Shutdown" ("Enum")] -> w2653
              tunnel: w2644 -> [w2660 _]
              frame "Start Task 1", Default {
                n872 = Or(x=w2660, y=w2662) -> (x .or. y?=w2661:bool)
                n873 = case shown="False" w2660 {
                  tunnel: w2668 -> [w2673 w2679]
                  tunnel: [w2672 w2677] -> w2667
                  frame False {
                    n874 = for {
                      shift-right: [w2675] -> w2672
                      shift-left: w2673 -> [w2676]
                      tunnel: string[] ["READ NAVX", "R-CW", ""] ("element") -> [w2674] mode=indexing
                      n875 = Enqueue Element(queue=w2676, element=w2674) -> (queue out=w2675:refnum<queue>)  [unwired: 2 in, 2 out]
                    }
                  }
                  frame True {
                    n876 = for {
                      shift-right: [w2681] -> w2677
                      shift-left: w2679 -> [w2682]
                      tunnel: string[] ["STOP", "RESET ENCODERS", "RESET YAW", "", ""] -> [w2680] mode=indexing
                      n877 = Enqueue Element(queue=w2682, element=w2680) -> (queue out=w2681:refnum<queue>)  [unwired: 2 in, 2 out]
                    }
                  }
                }
                n878 = Select(t=State_Type_Definitions,_for_0.26g_versions_and_later_3."True Stop" ("Enum"), s=w2662, f=State_Type_Definitions,_for_0.26g_versions_and_later_3."Task 9C: Detect Box") -> (s? t:f=w2664:T18)
                n879 = Select(t=w2664, s=w2661, f=State_Type_Definitions,_for_0.26g_versions_and_later_3."Task 9B: Rotate to Angle" ("Enum")) -> (s? t:f=w2670:T18)
              }
              frame "Exit" {
                n880 = for {
                  shift-right: [w2689] -> w2685
                  shift-left: w2686 -> [w2690]
                  tunnel: string[] ["STOP", "RESET ENCODERS", "RESET YAW", ""] -> [w2688] mode=indexing
                  n881 = Enqueue Element(queue=w2690, element=w2688) -> (queue out=w2689:refnum<queue>)  [unwired: 2 in, 2 out]
                }
              }
            }
          }
          frame "Task 9C: Detect Box" {
            # ">>> Motor control cluster >>>"
            # ">>Line Detected>>"
            # ">>Action Queue>>"
            # ">>> yStepper command>>>"
            n882 = Dequeue Element(queue=w2702, timeout in ms (-1)=w2701, error in (no error)=w2700) -> (element=w2703:T10)  [unwired: 3 out]
            n883 = case shown="\"Start Task 1\", Default" w2703 {
              tunnel: w2698 -> [w2704 _]
              tunnel: [w2714 State_Type_Definitions,_for_0.26g_versions_and_later_3."True Stop" ("Enum")] -> w2695
              tunnel: w2699 -> [w2712 w2730]
              tunnel: [w2711 w2729] -> w2694
              tunnel: [State_Type_Definitions,_for_0.26g_versions_and_later_3."Idle" ("Enum") State_Type_Definitions,_for_0.26g_versions_and_later_3."Shutdown" ("Enum")] -> w2697
              tunnel: w2691 -> [w2705 _]
              frame "Start Task 1", Default {
                n884 = Or(x=w2704, y=w2705) -> (x .or. y?=w2706:bool)
                n885 = case shown="False" w2705 {
                  tunnel: w2712 -> [w2717 w2723]
                  tunnel: [w2716 w2721] -> w2711
                  frame False {
                    n886 = for {
                      shift-right: [w2719] -> w2716
                      shift-left: w2717 -> [w2720]
                      tunnel: string[] ["READ IR", "READ LINE SENSOR", "FORWARD - IR ASSIST"] ("element") -> [w2718] mode=indexing
                      n887 = Enqueue Element(queue=w2720, element=w2718) -> (queue out=w2719:refnum<queue>)  [unwired: 2 in, 2 out]
                    }
                  }
                  frame True {
                    n888 = for {
                      shift-right: [w2725] -> w2721
                      shift-left: w2723 -> [w2726]
                      tunnel: string[] ["STOP", "RESET ENCODERS", "RESET YAW", "RESET FLAGS"] -> [w2724] mode=indexing
                      n889 = Enqueue Element(queue=w2726, element=w2724) -> (queue out=w2725:refnum<queue>)  [unwired: 2 in, 2 out]
                    }
                  }
                }
                n890 = Select(t=State_Type_Definitions,_for_0.26g_versions_and_later_3."True Stop" ("Enum"), s=w2704, f=State_Type_Definitions,_for_0.26g_versions_and_later_3."Task 9D: MOVE FORWARD") -> (s? t:f=w2708:T18)
                n891 = Select(t=w2708, s=w2706, f=State_Type_Definitions,_for_0.26g_versions_and_later_3."Task 9C: Detect Box" ("Enum")) -> (s? t:f=w2714:T18)
              }
              frame "Exit" {
                n892 = for {
                  shift-right: [w2733] -> w2729
                  shift-left: w2730 -> [w2734]
                  tunnel: string[] ["STOP", "RESET ENCODERS", "RESET YAW", ""] -> [w2732] mode=indexing
                  n893 = Enqueue Element(queue=w2734, element=w2732) -> (queue out=w2733:refnum<queue>)  [unwired: 2 in, 2 out]
                }
              }
            }
          }
          frame "Task 9D: MOVE FORWARD" {
            (unwired) 50.0 ("y")
            # ">> Item Selection Bias >>"
            # ">> Wall detected >>"
            # ">> Manual override >>"
            # ">>Table Detected>>"
            # ">>> Motor control cluster >>>"
            # ">>Table or wall detectected>>"
            # ">>Action Queue>>"
            # ">>> yStepper command>>>"
            n894 = Dequeue Element(queue=w2752, timeout in ms (-1)=w2751, error in (no error)=w2750) -> (element=w2753:T10)  [unwired: 3 out]
            n895 = Less Or Equal?(x=w2741, y=20.0) -> (x <= y?=w2736:bool)
            n896 = Less?(x=w2739, y=20.0) -> (x < y?=w2737:bool)
            n897 = Or(x=w2736, y=w2737) -> (x .or. y?=w2735:bool)
            n898 = case shown="\"Start Task 1\", Default" w2753 {
              tunnel: w2748 -> [w2754 _]
              tunnel: [w2764 State_Type_Definitions,_for_0.26g_versions_and_later_3."True Stop" ("Enum")] -> w2745
              tunnel: w2749 -> [w2762 w2780]
              tunnel: [w2761 w2779] -> w2744
              tunnel: [State_Type_Definitions,_for_0.26g_versions_and_later_3."Idle" ("Enum") State_Type_Definitions,_for_0.26g_versions_and_later_3."Shutdown" ("Enum")] -> w2747
              tunnel: w2735 -> [w2755 _]
              frame "Start Task 1", Default {
                n899 = Or(x=w2754, y=w2755) -> (x .or. y?=w2756:bool)
                n900 = case shown="True" w2755 {
                  tunnel: w2762 -> [w2767 w2773]
                  tunnel: [w2766 w2771] -> w2761
                  frame False {
                    n901 = for {
                      shift-right: [w2769] -> w2766
                      shift-left: w2767 -> [w2770]
                      tunnel: string[] ["READ IR", "FORWARD - IR ASSIST", ""] ("element") -> [w2768] mode=indexing
                      n902 = Enqueue Element(queue=w2770, element=w2768) -> (queue out=w2769:refnum<queue>)  [unwired: 2 in, 2 out]
                    }
                  }
                  frame True {
                    n903 = for {
                      shift-right: [w2775] -> w2771
                      shift-left: w2773 -> [w2776]
                      tunnel: string[] ["STOP", "RESET ENCODERS", "RESET YAW", "RESET FLAGS"] -> [w2774] mode=indexing
                      n904 = Enqueue Element(queue=w2776, element=w2774) -> (queue out=w2775:refnum<queue>)  [unwired: 2 in, 2 out]
                    }
                  }
                }
                n905 = Select(t=State_Type_Definitions,_for_0.26g_versions_and_later_3."True Stop" ("Enum"), s=w2754, f=State_Type_Definitions,_for_0.26g_versions_and_later_3."Task 9E: MOVE LEFT") -> (s? t:f=w2758:T18)
                n906 = Select(t=w2758, s=w2756, f=State_Type_Definitions,_for_0.26g_versions_and_later_3."Task 9D: MOVE FORWARD" ("Enum")) -> (s? t:f=w2764:T18)
              }
              frame "Exit" {
                n907 = for {
                  shift-right: [w2783] -> w2779
                  shift-left: w2780 -> [w2784]
                  tunnel: string[] ["STOP", "RESET ENCODERS", "RESET YAW", ""] -> [w2782] mode=indexing
                  n908 = Enqueue Element(queue=w2784, element=w2782) -> (queue out=w2783:refnum<queue>)  [unwired: 2 in, 2 out]
                }
              }
            }
          }
          frame "Task 9E: MOVE LEFT" {
            # ">> Item Selection Bias >>"
            # ">> Line detected? >>"
            # ">> Manual override >>"
            # ">>> Motor control cluster >>>"
            # ">>Action Queue>>"
            # ">>> yStepper command>>>"
            n909 = Dequeue Element(queue=w2796, timeout in ms (-1)=w2795, error in (no error)=w2794) -> (element=w2797:T10)  [unwired: 3 out]
            n910 = case shown="\"Start Task 1\", Default" w2797 {
              tunnel: w2792 -> [w2798 _]
              tunnel: [w2808 State_Type_Definitions,_for_0.26g_versions_and_later_3."True Stop" ("Enum")] -> w2789
              tunnel: w2793 -> [w2806 w2824]
              tunnel: [w2805 w2823] -> w2788
              tunnel: [State_Type_Definitions,_for_0.26g_versions_and_later_3."Idle" ("Enum") State_Type_Definitions,_for_0.26g_versions_and_later_3."Shutdown" ("Enum")] -> w2791
              tunnel: w2785 -> [w2799 _]
              frame "Start Task 1", Default {
                n911 = Or(x=w2798, y=w2799) -> (x .or. y?=w2800:bool)
                n912 = case shown="True" w2799 {
                  tunnel: w2806 -> [w2811 w2817]
                  tunnel: [w2810 w2815] -> w2805
                  frame False {
                    n913 = for {
                      shift-right: [w2813] -> w2810
                      shift-left: w2811 -> [w2814]
                      tunnel: string[] ["LEFT", "READ NAVX", "READ LINE SENSOR", ""] ("element") -> [w2812] mode=indexing
                      n914 = Enqueue Element(queue=w2814, element=w2812) -> (queue out=w2813:refnum<queue>)  [unwired: 2 in, 2 out]
                    }
                  }
                  frame True {
                    n915 = for {
                      shift-right: [w2819] -> w2815
                      shift-left: w2817 -> [w2820]
                      tunnel: string[] ["STOP", "RESET ENCODERS", "RESET YAW", "BOX COLOUR", "", ""] -> [w2818] mode=indexing
                      n916 = Enqueue Element(queue=w2820, element=w2818) -> (queue out=w2819:refnum<queue>)  [unwired: 2 in, 2 out]
                    }
                  }
                }
                n917 = Select(t=State_Type_Definitions,_for_0.26g_versions_and_later_3."True Stop" ("Enum"), s=w2798, f=State_Type_Definitions,_for_0.26g_versions_and_later_3."Task 9F: SCAN BOX") -> (s? t:f=w2802:T18)
                n918 = Select(t=w2802, s=w2800, f=State_Type_Definitions,_for_0.26g_versions_and_later_3."Task 9E: MOVE LEFT" ("Enum")) -> (s? t:f=w2808:T18)
              }
              frame "Exit" {
                n919 = for {
                  shift-right: [w2827] -> w2823
                  shift-left: w2824 -> [w2828]
                  tunnel: string[] ["STOP", "RESET ENCODERS", "RESET YAW", ""] -> [w2826] mode=indexing
                  n920 = Enqueue Element(queue=w2828, element=w2826) -> (queue out=w2827:refnum<queue>)  [unwired: 2 in, 2 out]
                }
              }
            }
          }
          frame "Task 9F: SCAN BOX" {
            # ">>> Motor control cluster >>>"
            # ">>Colour detection >>"
            # ">>> yStepper command>>>"
            # ">> Manual override >>"
            n921 = Dequeue Element(queue=w2845, timeout in ms (-1)=w2843, error in (no error)=w2844) -> (element=w2838:T10)  [unwired: 3 out]
            n922 = call "Box Colour FGV.vi"("Init/R/W State"=Box_Colour_FGV_States."Read") -> ("Colour to detect (output)"=w2831:T2)  [unwired: 9 in, 1 out]
            n923 = Equal?(x=w2832, y=w2831) -> (x = y?=w2830:bool)
            n924 = case shown="\"Start Task 1\", Default" w2838 {
              tunnel: [w2858 State_Type_Definitions,_for_0.26g_versions_and_later_3."True Stop" ("Enum")] -> w2835
              tunnel: [w2856 w2873] -> w2836
              tunnel: w2837 -> [w2855 _]
              tunnel: w2839 -> [w2848 _]
              tunnel: [State_Type_Definitions,_for_0.26g_versions_and_later_3."Idle" ("Enum") State_Type_Definitions,_for_0.26g_versions_and_later_3."Shutdown" ("Enum")] -> w2834
              tunnel: w2829 -> [w2849 _]
              tunnel: w2830 -> [w2847 _]
              frame "Start Task 1", Default {
                # ">> Will stop either due to manual override or is same box colour >>"
                # ">> WIill proceed to part ii if not manual override >>"
                # ">>If ENABLE or Trigger is set to true>>"
                n925 = Or(x=w2849, y=w2848) -> (x .or. y?=w2850:bool)
                n926 = case shown="True" w2849 {
                  tunnel: [w2861 w2867] -> w2856
                  tunnel: w2855 -> [w2860 w2866]
                  frame False {
                    n927 = for {
                      shift-right: [w2863] -> w2861
                      shift-left: w2860 -> [w2864]
                      tunnel: string[] ["", ""] ("element") -> [w2862] mode=indexing
                      n928 = Enqueue Element(queue=w2864, element=w2862) -> (queue out=w2863:refnum<queue>)  [unwired: 2 in, 2 out]
                    }
                  }
                  frame True {
                    n929 = for {
                      shift-right: [w2869] -> w2867
                      shift-left: w2866 -> [w2870]
                      tunnel: string[] ["RESET ENCODER", "RESET FLAGS", "RESET YAW", "", "", ""] -> [w2868] mode=indexing
                      n930 = Enqueue Element(queue=w2870, element=w2868) -> (queue out=w2869:refnum<queue>)  [unwired: 2 in, 2 out]
                    }
                  }
                }
                n931 = Or(x=w2848, y=w2847) -> (x .or. y?=w2846:bool)
                n932 = Select(t=State_Type_Definitions,_for_0.26g_versions_and_later_3."True Stop" ("Enum"), s=w2846, f=State_Type_Definitions,_for_0.26g_versions_and_later_3."Task 9G: MOVE RIGHT" ("Enum")) -> (s? t:f=w2852:T18)
                n933 = Select(t=w2852, s=w2850, f=State_Type_Definitions,_for_0.26g_versions_and_later_3."Task 9F: SCAN BOX" ("Enum")) -> (s? t:f=w2858:T18)
              }
              frame "Exit" {
                n934 = for {
                  shift-right: [w2876] -> w2873
                  shift-left: _ -> [w2877]
                  tunnel: string[] ["STOP", "RESET ENCODERS", "RESET YAW", ""] -> [w2875] mode=indexing
                  n935 = Enqueue Element(queue=w2877, element=w2875) -> (queue out=w2876:refnum<queue>)  [unwired: 2 in, 2 out]
                }
              }
            }
          }
          frame "Task 9G: MOVE RIGHT" {
            # ">>> Motor control cluster >>>"
            # ">>> yStepper command>>>"
            n936 = Dequeue Element(queue=w2889, timeout in ms (-1)=w2888, error in (no error)=w2887) -> (element=w2894:T10)  [unwired: 3 out]
            n937 = Greater?(x=w2879, y=50.0) -> (0:w2882:bool)
            n938 = And(x=w2880, y=w2882) -> (x .and. y?=w2878:bool)
            n939 = case shown="\"Start Task 1\", Default" w2894 {
              tunnel: w2878 -> [w2897 _]
              tunnel: [w2904 State_Type_Definitions,_for_0.26g_versions_and_later_3."True Stop" ("Enum")] -> w2893
              tunnel: w2886 -> [w2896 _]
              tunnel: w2890 -> [w2903 w2920]
              tunnel: [w2902 w2921] -> w2892
              tunnel: [State_Type_Definitions,_for_0.26g_versions_and_later_3."Idle" ("Enum") State_Type_Definitions,_for_0.26g_versions_and_later_3."Shutdown" ("Enum")] -> w2891
              frame "Start Task 1", Default {
                n940 = case shown="True" w2897 {
                  tunnel: w2903 -> [w2907 w2914]
                  tunnel: [w2908 w2913] -> w2902
                  frame False {
                    n941 = for {
                      tunnel: string[] ["READ LINE SENSOR", "READ NAVX", "RIGHT", "READ ENCODERS"] ("element") -> [w2909] mode=indexing
                      shift-right: [w2911] -> w2908
                      shift-left: w2907 -> [w2910]
                      n942 = Enqueue Element(queue=w2910, element=w2909) -> (queue out=w2911:refnum<queue>)  [unwired: 2 in, 2 out]
                    }
                  }
                  frame True {
                    n943 = for {
                      shift-right: [w2916] -> w2913
                      shift-left: w2914 -> [w2917]
                      tunnel: string[] ["RESET ENCODERS", "RESET YAW", "RESET FLAGS", "STOP", "BOX COLOUR"] -> [w2915] mode=indexing
                      n944 = Enqueue Element(queue=w2917, element=w2915) -> (queue out=w2916:refnum<queue>)  [unwired: 2 in, 2 out]
                    }
                  }
                }
                n945 = Or(x=w2897, y=w2896) -> (x .or. y?=w2895:bool)
                n946 = Select(t=State_Type_Definitions,_for_0.26g_versions_and_later_3."True Stop" ("Enum"), s=w2896, f=State_Type_Definitions,_for_0.26g_versions_and_later_3."Task 9H: SCAN BOX 2" ("Enum")) -> (s? t:f=w2898:T18)
                n947 = Select(t=w2898, s=w2895, f=State_Type_Definitions,_for_0.26g_versions_and_later_3."Task 9G: MOVE RIGHT" ("Enum")) -> (s? t:f=w2904:T18)
              }
              frame "Exit" {
                n948 = for {
                  shift-right: [w2924] -> w2921
                  shift-left: w2920 -> [w2925]
                  tunnel: string[] ["STOP", "RESET ENCODERS", "RESET YAW", "ARDUINO MODE 0"] -> [w2923] mode=indexing
                  n949 = Enqueue Element(queue=w2925, element=w2923) -> (queue out=w2924:refnum<queue>)  [unwired: 2 in, 2 out]
                }
              }
            }
          }
          frame "Task 9H: SCAN BOX 2" {
            # ">> Item Selection Bias >>"
            # ">>> Motor control cluster >>>"
            # ">>> yStepper command>>>"
            n950 = Dequeue Element(queue=w2935, timeout in ms (-1)=w2936, error in (no error)=w2937) -> (element=w2939:T10)  [unwired: 3 out]
            n951 = call "Box Colour FGV.vi"("Init/R/W State"=Box_Colour_FGV_States."Read") -> ("Colour to detect (output)"=w2929:T2)  [unwired: 9 in, 1 out]
            n952 = Equal?(x=w2928, y=w2929) -> (x = y?=w2927:bool)
            n953 = case shown="\"Start Task 1\", Default" w2939 {
              tunnel: w2926 -> [w2947 _]
              tunnel: [w2954 State_Type_Definitions,_for_0.26g_versions_and_later_3."True Stop" ("Enum")] -> w2932
              tunnel: w2938 -> [w2944 _]
              tunnel: w2934 -> [w2953 w2970]
              tunnel: [w2952 w2971] -> w2933
              tunnel: [State_Type_Definitions,_for_0.26g_versions_and_later_3."Idle" ("Enum") State_Type_Definitions,_for_0.26g_versions_and_later_3."Shutdown" ("Enum")] -> w2931
              tunnel: w2927 -> [w2945 _]
              frame "Start Task 1", Default {
                n954 = Or(x=w2947, y=w2944) -> (x .or. y?=w2946:bool)
                n955 = Or(x=w2945, y=w2944) -> (x .or. y?=w2943:bool)
                n956 = case shown="True" w2947 {
                  tunnel: w2953 -> [w2957 w2964]
                  tunnel: [w2958 w2963] -> w2952
                  frame False {
                    n957 = for {
                      tunnel: string[] ["", "", "", ""] ("element") -> [w2959] mode=indexing
                      shift-right: [w2961] -> w2958
                      shift-left: w2957 -> [w2960]
                      n958 = Enqueue Element(queue=w2960, element=w2959) -> (queue out=w2961:refnum<queue>)  [unwired: 2 in, 2 out]
                    }
                  }
                  frame True {
                    n959 = for {
                      shift-right: [w2966] -> w2963
                      shift-left: w2964 -> [w2967]
                      tunnel: string[] ["READ NAVX", "RESET FLAGS", "RESET ENCODERS", "", "", ""] -> [w2965] mode=indexing
                      n960 = Enqueue Element(queue=w2967, element=w2965) -> (queue out=w2966:refnum<queue>)  [unwired: 2 in, 2 out]
                    }
                  }
                }
                n961 = Select(t=State_Type_Definitions,_for_0.26g_versions_and_later_3."True Stop" ("Enum"), s=w2943, f=State_Type_Definitions,_for_0.26g_versions_and_later_3."Task 9I: ROTATE 90 CW" ("Enum")) -> (s? t:f=w2948:T18)
                n962 = Select(t=w2948, s=w2946, f=State_Type_Definitions,_for_0.26g_versions_and_later_3."Task 9H: SCAN BOX 2" ("Enum")) -> (s? t:f=w2954:T18)
              }
              frame "Exit" {
                n963 = for {
                  shift-right: [w2974] -> w2971
                  shift-left: w2970 -> [w2975]
                  tunnel: string[] ["STOP", "RESET ENCODERS", "RESET YAW", "ARDUINO MODE 0"] -> [w2973] mode=indexing
                  n964 = Enqueue Element(queue=w2975, element=w2973) -> (queue out=w2974:refnum<queue>)  [unwired: 2 in, 2 out]
                }
              }
            }
          }
          frame "Task 9I: ROTATE 90 CW" {
            # ">>> Motor control cluster >>>"
            # ">>> yStepper command>>>"
            # "High battery voltage: -36\nMid voltage: -38 \nLow voltage: -40"
            # ">> Item Selection Bias >>"
            n965 = Less Or Equal?(x=w2978, y=-38.0) -> (x <= y?=w2976:bool)
            n966 = Dequeue Element(queue=w2979, timeout in ms (-1)=w2980, error in (no error)=w2981) -> (element=w2987:T10)  [unwired: 3 out]
            n967 = case shown="\"Start Task 1\", Default" w2987 {
              tunnel: w2976 -> [w2993 _]
              tunnel: [w3000 State_Type_Definitions,_for_0.26g_versions_and_later_3."True Stop" ("Enum")] -> w2984
              tunnel: w2982 -> [w2992 _]
              tunnel: w2986 -> [w2999 w3016]
              tunnel: [w2998 w3017] -> w2985
              tunnel: [State_Type_Definitions,_for_0.26g_versions_and_later_3."Idle" ("Enum") State_Type_Definitions,_for_0.26g_versions_and_later_3."Shutdown" ("Enum")] -> w2983
              frame "Start Task 1", Default {
                n968 = case shown="False" w2993 {
                  tunnel: w2999 -> [w3003 w3010]
                  tunnel: [w3004 w3009] -> w2998
                  frame False {
                    n969 = for {
                      tunnel: string[] ["R-CW", "READ ENCODERS", "READ IR", "READ NAVX"] ("element") -> [w3005] mode=indexing
                      shift-right: [w3007] -> w3004
                      shift-left: w3003 -> [w3006]
                      n970 = Enqueue Element(queue=w3006, element=w3005) -> (queue out=w3007:refnum<queue>)  [unwired: 2 in, 2 out]
                    }
                  }
                  frame True {
                    n971 = for {
                      shift-right: [w3012] -> w3009
                      shift-left: w3010 -> [w3013]
                      tunnel: string[] ["STOP", "RESET ENCODERS", "RESET YAW", "RESET FLAGS", "READ IR", ""] -> [w3011] mode=indexing
                      n972 = Enqueue Element(queue=w3013, element=w3011) -> (queue out=w3012:refnum<queue>)  [unwired: 2 in, 2 out]
                    }
                  }
                }
                n973 = Or(x=w2993, y=w2992) -> (x .or. y?=w2991:bool)
                n974 = Select(t=State_Type_Definitions,_for_0.26g_versions_and_later_3."True Stop" ("Enum"), s=w2992, f=State_Type_Definitions,_for_0.26g_versions_and_later_3."Task 9J: FORWARD" ("Enum")) -> (s? t:f=w2994:T18)
                n975 = Select(t=w2994, s=w2991, f=State_Type_Definitions,_for_0.26g_versions_and_later_3."Task 9I: ROTATE 90 CW" ("Enum")) -> (s? t:f=w3000:T18)
              }
              frame "Exit" {
                n976 = for {
                  shift-right: [w3020] -> w3017
                  shift-left: w3016 -> [w3021]
                  tunnel: string[] ["STOP", "RESET ENCODERS", "RESET YAW", "ARDUINO MODE 0"] -> [w3019] mode=indexing
                  n977 = Enqueue Element(queue=w3021, element=w3019) -> (queue out=w3020:refnum<queue>)  [unwired: 2 in, 2 out]
                }
              }
            }
          }
          frame "Task 9J: FORWARD" {
            # "Tried values: 70, 150"
            # ">>Stops if either table or wall is obstructing >>"
            # ">> Item Selection Bias >>"
            n978 = Less?(x=w3024, y=150.0) -> (x < y?=w3027:bool)
            n979 = Greater Than 0?(x=w3024) -> (x > 0?=w3026:bool)
            n980 = Less Or Equal?(x=w3030, y=20.0) -> (x <= y?=w3028:bool)
            n981 = Greater Than 0?(x=w3030) -> (x > 0?=w3029:bool)
            n982 = And(x=w3026, y=w3027) -> ()  [unwired: 1 out]
            n983 = Dequeue Element(queue=w3036, timeout in ms (-1)=w3037, error in (no error)=w3038) -> (element=w3040:T10)  [unwired: 3 out]
            n984 = And(x=w3029, y=w3028) -> (x .and. y?=w3022:bool)
            n985 = Or(x=w3022, y=w3022) -> (x .or. y?=w3023:bool)
            n986 = case shown="\"Start Task 1\", Default" w3040 {
              tunnel: w3023 -> [w3046 _]
              tunnel: [w3053 State_Type_Definitions,_for_0.26g_versions_and_later_3."True Stop" ("Enum")] -> w3034
              tunnel: w3039 -> [w3045 _]
              tunnel: w3035 -> [w3052 w3069]
              tunnel: [w3051 w3070] -> w3033
              tunnel: [State_Type_Definitions,_for_0.26g_versions_and_later_3."Idle" ("Enum") State_Type_Definitions,_for_0.26g_versions_and_later_3."Shutdown" ("Enum")] -> w3032
              frame "Start Task 1", Default {
                n987 = case shown="True" w3046 {
                  tunnel: w3052 -> [w3056 w3063]
                  tunnel: [w3057 w3062] -> w3051
                  frame False {
                    n988 = for {
                      tunnel: string[] ["READ IR", "READ NAVX", "FORWARD"] ("element") -> [w3058] mode=indexing
                      shift-right: [w3060] -> w3057
                      shift-left: w3056 -> [w3059]
                      n989 = Enqueue Element(queue=w3059, element=w3058) -> (queue out=w3060:refnum<queue>)  [unwired: 2 in, 2 out]
                    }
                  }
                  frame True {
                    n990 = for {
                      shift-right: [w3065] -> w3062
                      shift-left: w3063 -> [w3066]
                      tunnel: string[] ["STOP", "RESET ENCODERS", "RESET YAW", "RESET FLAGS", "READ IR", ""] -> [w3064] mode=indexing
                      n991 = Enqueue Element(queue=w3066, element=w3064) -> (queue out=w3065:refnum<queue>)  [unwired: 2 in, 2 out]
                    }
                  }
                }
                n992 = Or(x=w3046, y=w3045) -> (x .or. y?=w3044:bool)
                n993 = Select(t=State_Type_Definitions,_for_0.26g_versions_and_later_3."True Stop" ("Enum"), s=w3045, f=State_Type_Definitions,_for_0.26g_versions_and_later_3."Task 9K: RAM WALL" ("Enum")) -> (s? t:f=w3047:T18)
                n994 = Select(t=w3047, s=w3044, f=State_Type_Definitions,_for_0.26g_versions_and_later_3."Task 9J: FORWARD" ("Enum")) -> (s? t:f=w3053:T18)
              }
              frame "Exit" {
                n995 = for {
                  shift-right: [w3073] -> w3070
                  shift-left: w3069 -> [w3074]
                  tunnel: string[] ["STOP", "RESET ENCODERS", "RESET YAW", "ARDUINO MODE 0"] -> [w3072] mode=indexing
                  n996 = Enqueue Element(queue=w3074, element=w3072) -> (queue out=w3073:refnum<queue>)  [unwired: 2 in, 2 out]
                }
              }
            }
          }
          frame "Task 9K: RAM WALL" {
            # "High battery voltage: 15"
            # ">> Item Selection Bias >>"
            # ">>Stops if either table or wall is obstructing >>"
            n997 = Less?(x=w3075, y=15.0) -> (x < y?=w3085:bool)
            n998 = Dequeue Element(queue=w3083, timeout in ms (-1)=w3082, error in (no error)=w3081) -> (element=w3087:T10)  [unwired: 3 out]
            n999 = case shown="\"Start Task 1\", Default" w3087 {
              tunnel: w3085 -> [w3092 _]
              tunnel: [w3099 State_Type_Definitions,_for_0.26g_versions_and_later_3."True Stop" ("Enum")] -> w3077
              tunnel: w3080 -> [w3091 _]
              tunnel: w3084 -> [w3098 w3115]
              tunnel: [w3097 w3116] -> w3078
              tunnel: [State_Type_Definitions,_for_0.26g_versions_and_later_3."Idle" ("Enum") State_Type_Definitions,_for_0.26g_versions_and_later_3."Shutdown" ("Enum")] -> w3076
              frame "Start Task 1", Default {
                n1000 = case shown="True" w3092 {
                  tunnel: w3098 -> [w3102 w3109]
                  tunnel: [w3103 w3108] -> w3097
                  frame False {
                    n1001 = for {
                      tunnel: string[] ["LEFT", "READ NAVX", "READ IR", ""] ("element") -> [w3104] mode=indexing
                      shift-right: [w3106] -> w3103
                      shift-left: w3102 -> [w3105]
                      n1002 = Enqueue Element(queue=w3105, element=w3104) -> (queue out=w3106:refnum<queue>)  [unwired: 2 in, 2 out]
                    }
                  }
                  frame True {
                    n1003 = for {
                      shift-right: [w3111] -> w3108
                      shift-left: w3109 -> [w3112]
                      tunnel: string[] ["STOP", "RESET ENCODERS", "RESET FLAGS", "RESET YAW", "READ IR", ""] -> [w3110] mode=indexing
                      n1004 = Enqueue Element(queue=w3112, element=w3110) -> (queue out=w3111:refnum<queue>)  [unwired: 2 in, 2 out]
                    }
                  }
                }
                n1005 = Or(x=w3092, y=w3091) -> (x .or. y?=w3090:bool)
                n1006 = Select(t=State_Type_Definitions,_for_0.26g_versions_and_later_3."True Stop" ("Enum"), s=w3091, f=State_Type_Definitions,_for_0.26g_versions_and_later_3."Task 9L: MOVE RIGHT" ("Enum")) -> (s? t:f=w3093:T18)
                n1007 = Select(t=w3093, s=w3090, f=State_Type_Definitions,_for_0.26g_versions_and_later_3."Task 9K: RAM WALL" ("Enum")) -> (s? t:f=w3099:T18)
              }
              frame "Exit" {
                n1008 = for {
                  shift-right: [w3119] -> w3116
                  shift-left: w3115 -> [w3120]
                  tunnel: string[] ["STOP", "RESET ENCODERS", "RESET YAW", "ARDUINO MODE 0"] -> [w3118] mode=indexing
                  n1009 = Enqueue Element(queue=w3120, element=w3118) -> (queue out=w3119:refnum<queue>)  [unwired: 2 in, 2 out]
                }
              }
            }
          }
          frame "Task 9L: MOVE RIGHT" {
            # "High battery voltage: 15"
            # ">>> Motor control cluster >>>"
            # ">>> yStepper command>>>"
            # ">> Item Selection Bias >>"
            n1010 = Dequeue Element(queue=w3128, timeout in ms (-1)=w3127, error in (no error)=w3126) -> (element=w3130:T10)  [unwired: 3 out]
            n1011 = case shown="\"Start Task 1\", Default" w3130 {
              tunnel: w3121 -> [w3136 _]
              tunnel: [w3143 State_Type_Definitions,_for_0.26g_versions_and_later_3."True Stop" ("Enum")] -> w3124
              tunnel: w3125 -> [w3135 _]
              tunnel: w3129 -> [w3142 w3159]
              tunnel: [w3141 w3160] -> w3122
              tunnel: [State_Type_Definitions,_for_0.26g_versions_and_later_3."Idle" ("Enum") State_Type_Definitions,_for_0.26g_versions_and_later_3."Shutdown" ("Enum")] -> w3123
              frame "Start Task 1", Default {
                n1012 = case shown="True" w3136 {
                  tunnel: w3142 -> [w3146 w3153]
                  tunnel: [w3147 w3152] -> w3141
                  frame False {
                    n1013 = for {
                      tunnel: string[] ["RIGHT", "READ NAVX", "READ LINE SENSOR", ""] ("element") -> [w3148] mode=indexing
                      shift-right: [w3150] -> w3147
                      shift-left: w3146 -> [w3149]
                      n1014 = Enqueue Element(queue=w3149, element=w3148) -> (queue out=w3150:refnum<queue>)  [unwired: 2 in, 2 out]
                    }
                  }
                  frame True {
                    n1015 = for {
                      shift-right: [w3155] -> w3152
                      shift-left: w3153 -> [w3156]
                      tunnel: string[] ["STOP", "RESET ENCODERS", "RESET FLAGS", "RESET YAW", "BOX COLOUR", ""] -> [w3154] mode=indexing
                      n1016 = Enqueue Element(queue=w3156, element=w3154) -> (queue out=w3155:refnum<queue>)  [unwired: 2 in, 2 out]
                    }
                  }
                }
                n1017 = Or(x=w3136, y=w3135) -> (x .or. y?=w3134:bool)
                n1018 = Select(t=State_Type_Definitions,_for_0.26g_versions_and_later_3."True Stop" ("Enum"), s=w3135, f=State_Type_Definitions,_for_0.26g_versions_and_later_3."Task 9M: SCAN BOX 3" ("Enum")) -> (s? t:f=w3137:T18)
                n1019 = Select(t=w3137, s=w3134, f=State_Type_Definitions,_for_0.26g_versions_and_later_3."Task 9L: MOVE RIGHT" ("Enum")) -> (s? t:f=w3143:T18)
              }
              frame "Exit" {
                n1020 = for {
                  shift-right: [w3163] -> w3160
                  shift-left: w3159 -> [w3164]
                  tunnel: string[] ["STOP", "RESET ENCODERS", "RESET YAW", "ARDUINO MODE 0"] -> [w3162] mode=indexing
                  n1021 = Enqueue Element(queue=w3164, element=w3162) -> (queue out=w3163:refnum<queue>)  [unwired: 2 in, 2 out]
                }
              }
            }
          }
          frame "Task 9M: SCAN BOX 3" {
            # ">>> Motor control cluster >>>"
            # ">>> yStepper command>>>"
            # ">> Item Selection Bias >>"
            n1022 = Dequeue Element(queue=w3174, timeout in ms (-1)=w3173, error in (no error)=w3172) -> (element=w3178:T10)  [unwired: 3 out]
            n1023 = call "Box Colour FGV.vi"("Init/R/W State"=Box_Colour_FGV_States."Read") -> ("Colour to detect (output)"=w3168:T2)  [unwired: 9 in, 1 out]
            n1024 = Equal?(x=w3167, y=w3168) -> (x = y?=w3166:bool)
            n1025 = case shown="\"Start Task 1\", Default" w3178 {
              tunnel: w3165 -> [w3186 _]
              tunnel: [w3193 State_Type_Definitions,_for_0.26g_versions_and_later_3."True Stop" ("Enum")] -> w3176
              tunnel: w3171 -> [w3182 _]
              tunnel: w3175 -> [w3192 w3209]
              tunnel: [w3191 w3210] -> w3170
              tunnel: [State_Type_Definitions,_for_0.26g_versions_and_later_3."Idle" ("Enum") State_Type_Definitions,_for_0.26g_versions_and_later_3."Shutdown" ("Enum")] -> w3177
              tunnel: w3166 -> [w3184 _]
              frame "Start Task 1", Default {
                n1026 = case shown="True" w3186 {
                  tunnel: w3192 -> [w3196 w3203]
                  tunnel: [w3197 w3202] -> w3191
                  frame False {
                    n1027 = for {
                      tunnel: string[] ["", "", "", ""] ("element") -> [w3198] mode=indexing
                      shift-right: [w3200] -> w3197
                      shift-left: w3196 -> [w3199]
                      n1028 = Enqueue Element(queue=w3199, element=w3198) -> (queue out=w3200:refnum<queue>)  [unwired: 2 in, 2 out]
                    }
                  }
                  frame True {
                    n1029 = for {
                      shift-right: [w3205] -> w3202
                      shift-left: w3203 -> [w3206]
                      tunnel: string[] ["STOP", "RESET ENCODERS", "RESET FLAGS", "RESET YAW", "", ""] -> [w3204] mode=indexing
                      n1030 = Enqueue Element(queue=w3206, element=w3204) -> (queue out=w3205:refnum<queue>)  [unwired: 2 in, 2 out]
                    }
                  }
                }
                n1031 = Or(x=w3186, y=w3182) -> (x .or. y?=w3185:bool)
                n1032 = Or(x=w3184, y=w3182) -> (x .or. y?=w3183:bool)
                n1033 = Select(t=State_Type_Definitions,_for_0.26g_versions_and_later_3."True Stop" ("Enum"), s=w3183, f=State_Type_Definitions,_for_0.26g_versions_and_later_3."Task 9N: MOVE RIGHT" ("Enum")) -> (s? t:f=w3187:T18)
                n1034 = Select(t=w3187, s=w3185, f=State_Type_Definitions,_for_0.26g_versions_and_later_3."Task 9M: SCAN BOX 3" ("Enum")) -> (s? t:f=w3193:T18)
              }
              frame "Exit" {
                n1035 = for {
                  shift-right: [w3213] -> w3210
                  shift-left: w3209 -> [w3214]
                  tunnel: string[] ["STOP", "RESET ENCODERS", "RESET YAW", "ARDUINO MODE 0"] -> [w3212] mode=indexing
                  n1036 = Enqueue Element(queue=w3214, element=w3212) -> (queue out=w3213:refnum<queue>)  [unwired: 2 in, 2 out]
                }
              }
            }
          }
          frame "Task 9N: MOVE RIGHT" {
            # ">> Item Selection Bias >>"
            n1037 = Dequeue Element(queue=w3219, timeout in ms (-1)=w3218, error in (no error)=w3217) -> (element=w3224:T10)  [unwired: 3 out]
            n1038 = case shown="\"Start Task 1\", Default" w3224 {
              tunnel: w3215 -> [w3230 _]
              tunnel: [w3237 State_Type_Definitions,_for_0.26g_versions_and_later_3."True Stop" ("Enum")] -> w3222
              tunnel: w3216 -> [w3229 _]
              tunnel: w3220 -> [w3236 w3253]
              tunnel: [w3235 w3254] -> w3221
              tunnel: [State_Type_Definitions,_for_0.26g_versions_and_later_3."Idle" ("Enum") State_Type_Definitions,_for_0.26g_versions_and_later_3."Shutdown" ("Enum")] -> w3223
              frame "Start Task 1", Default {
                n1039 = case shown="True" w3230 {
                  tunnel: w3236 -> [w3240 w3247]
                  tunnel: [w3241 w3246] -> w3235
                  frame False {
                    n1040 = for {
                      tunnel: string[] ["READ LINE SENSOR", "READ NAVX", "RIGHT", "READ ENCODERS"] ("element") -> [w3242] mode=indexing
                      shift-right: [w3244] -> w3241
                      shift-left: w3240 -> [w3243]
                      n1041 = Enqueue Element(queue=w3243, element=w3242) -> (queue out=w3244:refnum<queue>)  [unwired: 2 in, 2 out]
                    }
                  }
                  frame True {
                    n1042 = for {
                      shift-right: [w3249] -> w3246
                      shift-left: w3247 -> [w3250]
                      tunnel: string[] ["STOP", "RESET ENCODERS", "RESET YAW", "RESET FLAGS", "BOX COLOUR", ""] -> [w3248] mode=indexing
                      n1043 = Enqueue Element(queue=w3250, element=w3248) -> (queue out=w3249:refnum<queue>)  [unwired: 2 in, 2 out]
                    }
                  }
                }
                n1044 = Or(x=w3230, y=w3229) -> (x .or. y?=w3228:bool)
                n1045 = Select(t=State_Type_Definitions,_for_0.26g_versions_and_later_3."True Stop" ("Enum"), s=w3229, f=State_Type_Definitions,_for_0.26g_versions_and_later_3."Task 9O: SCAN BOX 4" ("Enum")) -> (s? t:f=w3231:T18)
                n1046 = Select(t=w3231, s=w3228, f=State_Type_Definitions,_for_0.26g_versions_and_later_3."Task 9N: MOVE RIGHT" ("Enum")) -> (s? t:f=w3237:T18)
              }
              frame "Exit" {
                n1047 = for {
                  shift-right: [w3257] -> w3254
                  shift-left: w3253 -> [w3258]
                  tunnel: string[] ["STOP", "RESET ENCODERS", "RESET YAW", "ARDUINO MODE 0"] -> [w3256] mode=indexing
                  n1048 = Enqueue Element(queue=w3258, element=w3256) -> (queue out=w3257:refnum<queue>)  [unwired: 2 in, 2 out]
                }
              }
            }
          }
          frame "Task 9O: SCAN BOX 4" {
            # ">>> Motor control cluster >>>"
            # ">>> yStepper command>>>"
            # ">> Item Selection Bias >>"
            n1049 = Dequeue Element(queue=w3269, timeout in ms (-1)=w3268, error in (no error)=w3267) -> (element=w3273:T10)  [unwired: 3 out]
            n1050 = call "Box Colour FGV.vi"("Init/R/W State"=Box_Colour_FGV_States."Read") -> ("Colour to detect (output)"=w3271:T2)  [unwired: 9 in, 1 out]
            n1051 = Equal?(x=w3261, y=w3271) -> (x = y?=w3270:bool)
            n1052 = case shown="\"Start Task 1\", Default" w3273 {
              tunnel: w3259 -> [w3280 _]
              tunnel: [w3287 State_Type_Definitions,_for_0.26g_versions_and_later_3."True Stop" ("Enum")] -> w3263
              tunnel: w3266 -> [w3276 _]
              tunnel: w3260 -> [w3286 w3303]
              tunnel: [w3285 w3304] -> w3264
              tunnel: [State_Type_Definitions,_for_0.26g_versions_and_later_3."Idle" ("Enum") State_Type_Definitions,_for_0.26g_versions_and_later_3."Shutdown" ("Enum")] -> w3262
              tunnel: w3270 -> [w3278 _]
              frame "Start Task 1", Default {
                n1053 = case shown="True" w3280 {
                  tunnel: w3286 -> [w3290 w3297]
                  tunnel: [w3291 w3296] -> w3285
                  frame False {
                    n1054 = for {
                      tunnel: string[] ["", "", "", ""] ("element") -> [w3292] mode=indexing
                      shift-right: [w3294] -> w3291
                      shift-left: w3290 -> [w3293]
                      n1055 = Enqueue Element(queue=w3293, element=w3292) -> (queue out=w3294:refnum<queue>)  [unwired: 2 in, 2 out]
                    }
                  }
                  frame True {
                    n1056 = for {
                      shift-right: [w3299] -> w3296
                      shift-left: w3297 -> [w3300]
                      tunnel: string[] ["STOP", "RESET ENCODERS", "RESET FLAGS", "RESET YAW", "", ""] -> [w3298] mode=indexing
                      n1057 = Enqueue Element(queue=w3300, element=w3298) -> (queue out=w3299:refnum<queue>)  [unwired: 2 in, 2 out]
                    }
                  }
                }
                n1058 = Or(x=w3280, y=w3276) -> (x .or. y?=w3279:bool)
                n1059 = Or(x=w3278, y=w3276) -> (x .or. y?=w3277:bool)
                n1060 = Select(t=State_Type_Definitions,_for_0.26g_versions_and_later_3."True Stop" ("Enum"), s=w3277, f=State_Type_Definitions,_for_0.26g_versions_and_later_3."True Stop" ("Enum")) -> (s? t:f=w3281:T18)
                n1061 = Select(t=w3281, s=w3279, f=State_Type_Definitions,_for_0.26g_versions_and_later_3."Task 9O: SCAN BOX 4" ("Enum")) -> (s? t:f=w3287:T18)
              }
              frame "Exit" {
                n1062 = for {
                  shift-right: [w3307] -> w3304
                  shift-left: w3303 -> [w3308]
                  tunnel: string[] ["STOP", "RESET ENCODERS", "RESET YAW", "ARDUINO MODE 0"] -> [w3306] mode=indexing
                  n1063 = Enqueue Element(queue=w3308, element=w3306) -> (queue out=w3307:refnum<queue>)  [unwired: 2 in, 2 out]
                }
              }
            }
          }
          frame "Task A1: RAISE ARM" {
            # ">>> Motor control cluster >>>"
            # ">> Stepper height reeached >>"
            # ">>> yStepper command>>>"
            # ">> Manual override >>"
            n1064 = Dequeue Element(queue=w3321, timeout in ms (-1)=w3316, error in (no error)=w3320) -> (element=w3323:T10)  [unwired: 3 out]
            n1065 = Equal?(x=w3318, y=u8 50) -> (x = y?=w3309:bool)
            n1066 = case shown="\"Start Task 1\", Default" w3323 {
              tunnel: [w3334 State_Type_Definitions,_for_0.26g_versions_and_later_3."True Stop" ("Enum")] -> w3314
              tunnel: [w3332 w3349] -> w3313
              tunnel: w3317 -> [w3331 _]
              tunnel: w3319 -> [w3325 _]
              tunnel: [State_Type_Definitions,_for_0.26g_versions_and_later_3."Idle" ("Enum") State_Type_Definitions,_for_0.26g_versions_and_later_3."Shutdown" ("Enum")] -> w3315
              tunnel: w3309 -> [w3324 _]
              frame "Start Task 1", Default {
                # ">> WIill proceed to part ii if not manual override >>"
                # ">>If ENABLE or Trigger is set to true>>"
                n1067 = Or(x=w3324, y=w3325) -> (x .or. y?=w3326:bool)
                n1068 = case shown="False" w3324 {
                  tunnel: [w3337 w3343] -> w3332
                  tunnel: w3331 -> [w3336 w3342]
                  frame False {
                    n1069 = for {
                      shift-right: [w3339] -> w3337
                      shift-left: w3336 -> [w3340]
                      tunnel: string[] ["Z STEPPER BOX HEIGHT", "READ STEPPER VALUES"] ("element") -> [w3338] mode=indexing
                      n1070 = Enqueue Element(queue=w3340, element=w3338) -> (queue out=w3339:refnum<queue>)  [unwired: 2 in, 2 out]
                    }
                  }
                  frame True {
                    n1071 = for {
                      shift-right: [w3345] -> w3343
                      shift-left: w3342 -> [w3346]
                      tunnel: string[] ["READ NAVX", "RESET FLAGS", "RESET YAW", "", "", ""] -> [w3344] mode=indexing
                      n1072 = Enqueue Element(queue=w3346, element=w3344) -> (queue out=w3345:refnum<queue>)  [unwired: 2 in, 2 out]
                    }
                  }
                }
                n1073 = Select(t=State_Type_Definitions,_for_0.26g_versions_and_later_3."True Stop" ("Enum"), s=w3325, f=State_Type_Definitions,_for_0.26g_versions_and_later_3."Task A2: ROTATE TO ANGLE" ("Enum")) -> (s? t:f=w3328:T18)
                n1074 = Select(t=w3328, s=w3326, f=State_Type_Definitions,_for_0.26g_versions_and_later_3."Task A1: RAISE ARM" ("Enum")) -> (s? t:f=w3334:T18)
              }
              frame "Exit" {
                n1075 = for {
                  shift-right: [w3352] -> w3349
                  shift-left: _ -> [w3353]
                  tunnel: string[] ["STOP", "RESET ENCODERS", "RESET YAW", ""] -> [w3351] mode=indexing
                  n1076 = Enqueue Element(queue=w3353, element=w3351) -> (queue out=w3352:refnum<queue>)  [unwired: 2 in, 2 out]
                }
              }
            }
          }
          frame "Task A2: ROTATE TO ANGLE" {
            # ">>> Motor control cluster >>>"
            # ">>> yStepper command>>>"
            n1077 = Dequeue Element(queue=w3367, timeout in ms (-1)=w3366, error in (no error)=w3365) -> (element=w3369:T10)  [unwired: 3 out]
            n1078 = In Range and Coerce(upper limit=65.0, x=w3359, lower limit=58.0) -> (In Range?=w3354:bool)  [unwired: 1 out]
            n1079 = case shown="\"Start Task 1\", Default" w3369 {
              tunnel: w3360 -> [w3372 _]
              tunnel: [w3380 State_Type_Definitions,_for_0.26g_versions_and_later_3."True Stop" ("Enum")] -> w3362
              tunnel: w3368 -> [w3378 w3396]
              tunnel: [w3377 w3395] -> w3361
              tunnel: [State_Type_Definitions,_for_0.26g_versions_and_later_3."Idle" ("Enum") State_Type_Definitions,_for_0.26g_versions_and_later_3."Shutdown" ("Enum")] -> w3363
              tunnel: w3354 -> [w3370 _]
              frame "Start Task 1", Default {
                n1080 = Or(x=w3370, y=w3372) -> (x .or. y?=w3371:bool)
                n1081 = case shown="False" w3370 {
                  tunnel: w3378 -> [w3383 w3389]
                  tunnel: [w3382 w3387] -> w3377
                  frame False {
                    n1082 = for {
                      shift-right: [w3385] -> w3382
                      shift-left: w3383 -> [w3386]
                      tunnel: string[] ["READ NAVX", "R-CW", ""] ("element") -> [w3384] mode=indexing
                      n1083 = Enqueue Element(queue=w3386, element=w3384) -> (queue out=w3385:refnum<queue>)  [unwired: 2 in, 2 out]
                    }
                  }
                  frame True {
                    n1084 = for {
                      shift-right: [w3391] -> w3387
                      shift-left: w3389 -> [w3392]
                      tunnel: string[] ["STOP", "RESET ENCODERS", "RESET YAW", "", ""] -> [w3390] mode=indexing
                      n1085 = Enqueue Element(queue=w3392, element=w3390) -> (queue out=w3391:refnum<queue>)  [unwired: 2 in, 2 out]
                    }
                  }
                }
                n1086 = Select(t=State_Type_Definitions,_for_0.26g_versions_and_later_3."True Stop" ("Enum"), s=w3372, f=State_Type_Definitions,_for_0.26g_versions_and_later_3."Task A3: MOVE TO BL BOX") -> (s? t:f=w3374:T18)
                n1087 = Select(t=w3374, s=w3371, f=State_Type_Definitions,_for_0.26g_versions_and_later_3."Task A2: ROTATE TO ANGLE" ("Enum")) -> (s? t:f=w3380:T18)
              }
              frame "Exit" {
                n1088 = for {
                  shift-right: [w3399] -> w3395
                  shift-left: w3396 -> [w3400]
                  tunnel: string[] ["STOP", "RESET ENCODERS", "RESET YAW", ""] -> [w3398] mode=indexing
                  n1089 = Enqueue Element(queue=w3400, element=w3398) -> (queue out=w3399:refnum<queue>)  [unwired: 2 in, 2 out]
                }
              }
            }
          }
          frame "Task A3: MOVE TO BL BOX" {
            # ">>> Motor control cluster >>>"
            # ">>Line Detected>>"
            # ">>Action Queue>>"
            # ">>> yStepper command>>>"
            n1090 = Dequeue Element(queue=w3412, timeout in ms (-1)=w3411, error in (no error)=w3410) -> (element=w3413:T10)  [unwired: 3 out]
            n1091 = case shown="\"Start Task 1\", Default" w3413 {
              tunnel: w3408 -> [w3414 _]
              tunnel: [w3424 State_Type_Definitions,_for_0.26g_versions_and_later_3."True Stop" ("Enum")] -> w3405
              tunnel: w3409 -> [w3422 w3440]
              tunnel: [w3421 w3439] -> w3404
              tunnel: [State_Type_Definitions,_for_0.26g_versions_and_later_3."Idle" ("Enum") State_Type_Definitions,_for_0.26g_versions_and_later_3."Shutdown" ("Enum")] -> w3407
              tunnel: w3401 -> [w3415 _]
              frame "Start Task 1", Default {
                n1092 = Or(x=w3414, y=w3415) -> (x .or. y?=w3416:bool)
                n1093 = case shown="True" w3415 {
                  tunnel: w3422 -> [w3427 w3433]
                  tunnel: [w3426 w3431] -> w3421
                  frame False {
                    n1094 = for {
                      shift-right: [w3429] -> w3426
                      shift-left: w3427 -> [w3430]
                      tunnel: string[] ["READ IR", "READ LINE SENSOR", "FORWARD - IR ASSIST"] ("element") -> [w3428] mode=indexing
                      n1095 = Enqueue Element(queue=w3430, element=w3428) -> (queue out=w3429:refnum<queue>)  [unwired: 2 in, 2 out]
                    }
                  }
                  frame True {
                    n1096 = for {
                      shift-right: [w3435] -> w3431
                      shift-left: w3433 -> [w3436]
                      tunnel: string[] ["STOP", "RESET ENCODERS", "RESET YAW", "RESET FLAGS"] -> [w3434] mode=indexing
                      n1097 = Enqueue Element(queue=w3436, element=w3434) -> (queue out=w3435:refnum<queue>)  [unwired: 2 in, 2 out]
                    }
                  }
                }
                n1098 = Select(t=State_Type_Definitions,_for_0.26g_versions_and_later_3."True Stop" ("Enum"), s=w3414, f=State_Type_Definitions,_for_0.26g_versions_and_later_3."Task A4: MOVE FORWARD") -> (s? t:f=w3418:T18)
                n1099 = Select(t=w3418, s=w3416, f=State_Type_Definitions,_for_0.26g_versions_and_later_3."Task A3: MOVE TO BL BOX" ("Enum")) -> (s? t:f=w3424:T18)
              }
              frame "Exit" {
                n1100 = for {
                  shift-right: [w3443] -> w3439
                  shift-left: w3440 -> [w3444]
                  tunnel: string[] ["STOP", "RESET ENCODERS", "RESET YAW", ""] -> [w3442] mode=indexing
                  n1101 = Enqueue Element(queue=w3444, element=w3442) -> (queue out=w3443:refnum<queue>)  [unwired: 2 in, 2 out]
                }
              }
            }
          }
          frame "Task A4: MOVE FORWARD" {
            # "Experiment and find proper value for this"
            # ">> Item Selection Bias >>"
            # ">> Manual override >>"
            # ">>> Motor control cluster >>>"
            # ">>Table or wall detectected>>"
            # ">>Action Queue>>"
            # ">>> yStepper command>>>"
            n1102 = Dequeue Element(queue=w3458, timeout in ms (-1)=w3457, error in (no error)=w3456) -> (element=w3459:T10)  [unwired: 3 out]
            n1103 = Greater Or Equal?(x=w3447, y=50.0) -> (x >= y?=w3445:bool)
            n1104 = case shown="\"Start Task 1\", Default" w3459 {
              tunnel: w3454 -> [w3462 _]
              tunnel: [w3470 State_Type_Definitions,_for_0.26g_versions_and_later_3."True Stop" ("Enum")] -> w3451
              tunnel: w3455 -> [w3468 w3486]
              tunnel: [w3467 w3485] -> w3450
              tunnel: [State_Type_Definitions,_for_0.26g_versions_and_later_3."Idle" ("Enum") State_Type_Definitions,_for_0.26g_versions_and_later_3."Shutdown" ("Enum")] -> w3453
              tunnel: w3445 -> [w3461 _]
              frame "Start Task 1", Default {
                n1105 = Or(x=w3462, y=w3461) -> (x .or. y?=w3460:bool)
                n1106 = case shown="False" w3460 {
                  tunnel: w3468 -> [w3473 w3479]
                  tunnel: [w3472 w3477] -> w3467
                  frame False {
                    n1107 = for {
                      shift-right: [w3475] -> w3472
                      shift-left: w3473 -> [w3476]
                      tunnel: string[] ["READ NAVX", "READ ENCODERS", "FORWARD"] ("element") -> [w3474] mode=indexing
                      n1108 = Enqueue Element(queue=w3476, element=w3474) -> (queue out=w3475:refnum<queue>)  [unwired: 2 in, 2 out]
                    }
                  }
                  frame True {
                    n1109 = for {
                      shift-right: [w3481] -> w3477
                      shift-left: w3479 -> [w3482]
                      tunnel: string[] ["STOP", "RESET ENCODERS", "RESET YAW", "RESET FLAGS"] -> [w3480] mode=indexing
                      n1110 = Enqueue Element(queue=w3482, element=w3480) -> (queue out=w3481:refnum<queue>)  [unwired: 2 in, 2 out]
                    }
                  }
                }
                n1111 = Select(t=State_Type_Definitions,_for_0.26g_versions_and_later_3."True Stop" ("Enum"), s=w3462, f=State_Type_Definitions,_for_0.26g_versions_and_later_3."Task A5: ROTATE CW 90") -> (s? t:f=w3464:T18)
                n1112 = Select(t=w3464, s=w3460, f=State_Type_Definitions,_for_0.26g_versions_and_later_3."Task A4: MOVE FORWARD" ("Enum")) -> (s? t:f=w3470:T18)
              }
              frame "Exit" {
                n1113 = for {
                  shift-right: [w3489] -> w3485
                  shift-left: w3486 -> [w3490]
                  tunnel: string[] ["STOP", "RESET ENCODERS", "RESET YAW", ""] -> [w3488] mode=indexing
                  n1114 = Enqueue Element(queue=w3490, element=w3488) -> (queue out=w3489:refnum<queue>)  [unwired: 2 in, 2 out]
                }
              }
            }
          }
          frame "Task A5: ROTATE CW 90" {
            # ">>> Motor control cluster >>>"
            # ">>> yStepper command>>>"
            # "High battery voltage: -36\nMid voltage: -38 \nLow voltage: -40"
            # ">> Item Selection Bias >>"
            n1115 = Less Or Equal?(x=w3493, y=-38.0) -> (x <= y?=w3491:bool)
            n1116 = Dequeue Element(queue=w3494, timeout in ms (-1)=w3495, error in (no error)=w3496) -> (element=w3502:T10)  [unwired: 3 out]
            n1117 = case shown="\"Start Task 1\", Default" w3502 {
              tunnel: w3491 -> [w3508 _]
              tunnel: [w3515 State_Type_Definitions,_for_0.26g_versions_and_later_3."True Stop" ("Enum")] -> w3499
              tunnel: w3497 -> [w3507 _]
              tunnel: w3501 -> [w3514 w3531]
              tunnel: [w3513 w3532] -> w3500
              tunnel: [State_Type_Definitions,_for_0.26g_versions_and_later_3."Idle" ("Enum") State_Type_Definitions,_for_0.26g_versions_and_later_3."Shutdown" ("Enum")] -> w3498
              frame "Start Task 1", Default {
                n1118 = case shown="True" w3508 {
                  tunnel: w3514 -> [w3518 w3525]
                  tunnel: [w3519 w3524] -> w3513
                  frame False {
                    n1119 = for {
                      tunnel: string[] ["R-CW", "READ ENCODERS", "READ IR", "READ NAVX"] ("element") -> [w3520] mode=indexing
                      shift-right: [w3522] -> w3519
                      shift-left: w3518 -> [w3521]
                      n1120 = Enqueue Element(queue=w3521, element=w3520) -> (queue out=w3522:refnum<queue>)  [unwired: 2 in, 2 out]
                    }
                  }
                  frame True {
                    n1121 = for {
                      shift-right: [w3527] -> w3524
                      shift-left: w3525 -> [w3528]
                      tunnel: string[] ["STOP", "RESET ENCODERS", "RESET YAW", "RESET FLAGS", "READ IR", ""] -> [w3526] mode=indexing
                      n1122 = Enqueue Element(queue=w3528, element=w3526) -> (queue out=w3527:refnum<queue>)  [unwired: 2 in, 2 out]
                    }
                  }
                }
                n1123 = Or(x=w3508, y=w3507) -> (x .or. y?=w3506:bool)
                n1124 = Select(t=State_Type_Definitions,_for_0.26g_versions_and_later_3."True Stop" ("Enum"), s=w3507, f=State_Type_Definitions,_for_0.26g_versions_and_later_3."True Stop" ("Enum")) -> (s? t:f=w3509:T18)
                n1125 = Select(t=w3509, s=w3506, f=State_Type_Definitions,_for_0.26g_versions_and_later_3."Task A5: ROTATE CW 90" ("Enum")) -> (s? t:f=w3515:T18)
              }
              frame "Exit" {
                n1126 = for {
                  shift-right: [w3535] -> w3532
                  shift-left: w3531 -> [w3536]
                  tunnel: string[] ["STOP", "RESET ENCODERS", "RESET YAW", "ARDUINO MODE 0"] -> [w3534] mode=indexing
                  n1127 = Enqueue Element(queue=w3536, element=w3534) -> (queue out=w3535:refnum<queue>)  [unwired: 2 in, 2 out]
                }
              }
            }
          }
        }
        "Object Detection" <- w324
        "Ultrasonic sensors" <- w347
        "Encoder values" <- w336
        "Stepper position values" <- w320
        "NAVX Values" <- w318
        "IR Sensors" <- w310
        "Line sensors" <- w305
        "Time cluster" <- w316
        "Box Colour Detection" <- w298
      }
    }
    "Object recognition mode" <- w222
    "Front Ultrasonic obstruct" <- w219
    "Front IR obstruct" <- w218
    "Table IR obstruct" <- w217
    "Same colour?" <- w212
    n1128 = local write "Green LED"(w232) -> ()
  }
  n1129 = while {
    tunnel: w47 -> [w4455]
    tunnel: w46 -> [w4452]
    stop <- w4449 stop-if-true
    # "Status Loop for Action Queues"
    n1130 = Get Queue Status(queue=w4455, return elements? (F)=TRUE) -> (error out=w4451:errorcluster, # elements in queue=→"Action Queue Items":i32, elements=→"Action Queues items":string[])  [unwired: 1 in, 5 out]
    n1131 = Get Queue Status(queue=w4452, return elements? (F)=TRUE) -> (# pending remove=→"State Logic Queue Items":i32, error out=w4450:errorcluster, elements=→"elements":T10[])  [unwired: 1 in, 5 out]
    n1132 = Merge Errors(w4451, w4450) -> (w4449:errorcluster)
    n1133 = Wait (ms)(milliseconds to wait=u32 500) -> ()  [unwired: 1 out]
  }
  n1134 = while {
    stop <- w4459 stop-if-true
    n1135 = call "MOTOR CONTROL WITH PID AE.vi"("AE Mode"=MOTOR_CONTROL_WITH_PID_AE_DATA_MODE_TYPE_DEF."Read from AE") -> ("Speed & distance"=→"Speed & distance":T15)  [unwired: 3 in]
    n1136 = call "FGV Bool.vi"("Init/Read/Write State"=States_for_Action_Engine."Read") -> ("Output node"=w4459:bool)  [unwired: 2 in, 1 out]
    n1137 = Wait (ms)(milliseconds to wait=u32 5) -> ()  [unwired: 1 out]
  }
  n1138 = call <vilib>:"DIO Close.vi"("error in (no error)"=w23, "DIO Info In"=w26) -> ()  [unwired: 9 in, 1 out]
  n1139 = call <vilib>:"DIO Close.vi"("error in (no error)"=w33, "DIO Info In"=w35) -> ()  [unwired: 9 in, 1 out]
  n1140 = call <vilib>:"NavX Close.vi"("error in (no error)"=w10, "NavX Info In"=w9) -> ()  [unwired: 9 in, 1 out]
  n1141 = call <vilib>:"DIO Close.vi"("error in (no error)"=w28, "DIO Info In"=w30) -> ()  [unwired: 9 in, 1 out]
  n1142 = call <vilib>:"DIO Close.vi"("error in (no error)"=w17, "DIO Info In"=w18) -> ()  [unwired: 9 in, 1 out]
  n1143 = call <vilib>:"DIO Close.vi"("error in (no error)"=w12, "DIO Info In"=w13) -> ()  [unwired: 9 in, 1 out]
  n1144 = Merge Errors "Merge Errors"(w63, w62) -> (w45:errorcluster)
  n1145 = Merge Errors(w49, w45) -> (w44:errorcluster)
  n1146 = Destroy User Event(user event=w67, error in=w44) -> ()  [unwired: 1 out]
  n1147 = Release Queue(queue=w40, error in (no error)=w44) -> (error out=→"Queue Errors":errorcluster)  [unwired: 1 in, 2 out]
  n1148 = Release Queue(queue=w57, error in (no error)=w44) -> ()  [unwired: 1 in, 3 out]
  n1149 = Destroy User Event(user event=w66, error in=w44) -> ()  [unwired: 1 out]
  n1150 = Unregister For Events(event registration refnum=w58, error in=w44) -> ()  [unwired: 1 out]
